vi "ActiView903-RealTime_CAS.vi"() -> ()   [LabVIEW 2022 SP3]
doc: "ActiView is based on a state machine (case structure inside while-loop) with six (orange) states:\n\nState 0: Wait for START, and read/write CFG files\nState 1: Start acquisition, determine speedmode and AD-box version, set panel controls accordingly, stop acquisition\nState 2: Reset panel indicators\nState 3: Initialize saving to BDF file\nState 4: Start acquisition, iterate while-loop to write data to screen and BDF flle (if selected) until STOP is pressed, or error occurs, stop acquisition\nState 5: Reset panel indicators, close BDF file\n\nThe while-loop in (orange) state 4 has five (green) cases.\n\nCase 0: Wait for new data\nCase 1: Read new data from ringbuffer, downsample data, write data to charts and in file array\nCase 2: Transfer block of 1 second of data from file array to BDF file\nCase 3: Close BDF file, and open new BDF file\nCase 4: Calculate average result, and write to ERP graphs \n\nAlso see the Light version of ActiView avalable from the www.biosemi.com"
uses:
  ActiView9-Subvi.llb/Data.glb
  ActiView9-Subvi.llb/CapsThread.glb
  ActiView9-Subvi.llb/PanelThread.glb
  <vilib>/Instr/_visa.llb/VISA Configure Serial Port (Instr).vi
  <vilib>/Utility/cursorutil.llb/Set Cursor (Icon Pict).vi
  <vilib>/Utility/config.llb/Read Key (String).vi
  <vilib>/Utility/config.llb/Write Key (String).vi
  ActiView9-Subvi.llb/StopJazzIni.glb
  ActiView9-Subvi.llb/TCPidentification.glb
  ActiView9-Subvi.llb/JazzLoBatWarning.glb
  ActiView9-Subvi.llb/LoBatWarning.glb
  ActiView9-Subvi.llb/StopThreads.glb
  <vilib>/httpClient/POSTBuffer.vi
  Instance          61 25Saved   ActiView606-Lores .vi
  <vilib>/Utility/config.llb/NI_LVConfig.lvlib
  <vilib>/httpClient/LabVIEWHTTPClient.lvlib
  <vilib>/Analysis/NI_AALBase.lvlib
panel:
  out "RemaingStim":i16
  in  "Task OFF/ON":bool
  in  "Condition":i8(ring) items=["Synch", "Asynch"]
  in  "Bloc":i8(ring) items=["1", "2", "3", "4"]
  in  "R-peak Threshold adjust":dbl=1.0 min=0.0 step=0.1 format="%#.6g"
  out "Trigger Bar":enum32{"Blank"}(tab)
  out "Dummy String":string
  out "Trigger Chart":i32[][](graph)
  out "Trigger Code":picture
  out "Battery":u8(slide) scale=0.0..100.0
  in  "Box":i32(ring) items=["AD-Box 1", "AD-Box 2", "AD-Box 3", "AD-Box 4"]
  out "Right Sidebar":enum32{"Blank"}(tab)
  out "Free HDD [sec]":i64=-1 caption="Free on Disc sec"
  out "Nr of Files":i32
  out "Total Saved [sec]":i32
  out "Current File [MB]":dbl format="%.1f"
  out "with Jazz or ABR":bool caption="with Jazz"
  out "Box4":bool caption="Box1"
  out "Box3":bool caption="Box1"
  out "Box2":bool caption="Box1"
  out "Box1":bool
  in  "FileAppend":bool=TRUE
  in  "RecTimeLimit":i32=9999999 caption="Time Limit [sec]" min=1 max=9999999 step=1
  out "Nr Chan Saved":string="0 + 0"
  out "with AIB":bool
  out "with Sens":bool
  out "with  8 EX":bool
  out "Bandwidth [Hz]":dbl
  in  "Decimation":i8(ring) items=["1", "1/2", "1/4", "1/8", "1/16", "1/32", "1/64"]
  out "Sample Rate [Hz]":dbl
  in  "FileLimit":i64=999999 caption="File Limit [MB]" min=1 max=999999 step=1
  out "Save Subset":string
  in  "Start Saving":bool
  in  "Pause Saving":bool
  out "Left Sidebar":T1(tab)
  in  "MonFree":i32[](listbox)=[0, 1, 2, 3, 4, 5, 6, 7, 8, 9, 10, 11, 12, 13, 14, 15, 16, 17, 18, 19, 20, 21, 22, 23, 24, 25, 26, 27, 28, 29, 30, 31, 32, 33, 34, 35, 36, 37, 38, 39, 40, 41, 42, 43, 44, 45, 46, 47, 48, 49, 50, 51, 52, 53, 54, 55, 56, 57, 58, 59, 60, 61, 62, 63, 64, 65, 66, 67, 68, 69, 70, 71, 72, 73, 74, 75, 76, 77, 78, 79, 80, 81, 82, 83, 84, 85, 86, 87, 88, 89, 90, 91, 92, 93, 94, 95, 96, 97, 98, 99, 100, 101, 102, 103, 104, 105, 106, 107, 108, 109, 110, 111, 112, 113, 114, 115, 116, 117, 118, 119, 120, 121, 122, 123, 124, 125, 126, 127, 128, 129, 130, 131, 132, 133, 134, 135, 136, 137, 138, 139, 140, 141, 142, 143, 144, 145, 146, 147, 148, 149, 150, 151, 152, 153, 154, 155, 156, 157, 158, 159, 160, 161, 162, 163, 164, 165, 166, 167, 168, 169, 170, 171, 172, 173, 174, 175, 176, 177, 178, 179, 180, 181, 182, 183, 184, 185, 186, 187, 188, 189, 190, 191, 192, 193, 194, 195, 196, 197, 198, 199, 200, 201, 202, 203, 204, 205, 206, 207, 208, 209, 210, 211, 212, 213, 214, 215, 216, 217, 218, 219, 220, 221, 222, 223, 224, 225, 226, 227, 228, 229, 230, 231, 232, 233, 234, 235, 236, 237, 238, 239, 240, 241, 242, 243, 244, 245, 246, 247, 248, 249, 250, 251, 252, 253, 254, 255]
  in  "Reference":i8(ring) items=["None (raw)", "Avg of 264", "Avg 1-256", "Avg 1-160", "Avg 1-128", "Avg 1-64", "Avg 1-32", "Avg of Displ", "Free Choice", "Ref (ABR)", "Mastoids (ABR)"]
  in  "Mon Filter Reset":bool
  in  "MonLP":bool=TRUE caption="Lowpass"
  in  "MonHP":bool=TRUE caption="Highpass"
  in  "RefFree":i32[](listbox)
  in  "Channels":i8(ring) items=["All 264 Chan ", "A-H (256)", "A-E (160)", "ABCD (128)", "A+B (64)", "A (32)", "B (32)", "C (32)", "D (32)", "E (32)", "F (32)", "G (32)", "H(32)", "EXG (8)", "Free Choice"]
  in  "MonHPfreq":dbl=0.16 caption="Cutoff Freq" min=0.01 max=9.99 step=0.1 format="%.2f"
  in  "MonScale":i8(ring)=4 caption="Y-scale V/div" items=["5 uV", "10 uV", "20 uV", "50 uV", "100 uV", "200 uV", "500 uV", "1 mV", "2 mV", "5 mV", "10 mV", "20 mV", "50 mV", "100 mV", "200 mV", "500 mV"]
  in  "MonLPfreq":dbl=100.0 caption="Cutoff Freq" min=1.0 max=8191.0 step=10.0
  out "NoRef Blinker":bool
  in  "AddTP":bool caption="Add  8 EXG"
  in  "BipFree":i32[](listbox)=[0, 2, 4, 6] caption="Bipolar\nLeads"
  in  "BipLP":bool=TRUE caption="Lowpass"
  in  "BipHP":bool=TRUE caption="Highpass"
  in  "BipHPfreq":dbl=0.16 caption="Cutoff Freq" min=0.01 max=99.9 step=1.0 format="%.2f"
  in  "BipScale":i8(ring)=7 caption="Y-scale V/div" items=["5 uV", "10 uV", "20 uV", "50 uV", "100 uV", "200 uV", "500 uV", "1 mV", "2 mV", "5 mV", "10 mV", "20 mV", "50 mV", "100 mV", "200 mV", "500 mV"]
  in  "BipLPfreq":dbl=100.0 caption="Cutoff Freq" min=1.0 max=8191.0 step=10.0
  in  "Bip Filter Reset":bool
  out "TP Offset Graph 2":dbl[](graph) caption="EX5 - EX8"
  out "TP Offset Graph 1":dbl[](graph) caption="EX1 - EX4"
  in  "Offset":i8(ring) caption="Channels" items=["All 256 Chan ", "A + B", "C + D", "E + F", "G + H"]
  out "Full Range":bool=TRUE
  in  "OffsetScale":i8(ring)=3 caption="Range" items=["20 mV", "50 mV", "100 mV", "262  mV", "1049 mV"]
  in  "HeadcapMaps":bool
  in  "UploadMaps":bool
  in  "ABR Filter Reset":bool
  in  "AbrLP":bool=TRUE caption="Lowpass"
  in  "AbrHP":bool=TRUE caption="Highpass"
  in  "AbrHPfreq":dbl=0.16 caption="Cutoff Freq" min=0.1 max=100.0 step=1.0 format="%.1f"
  in  "AbrScale":i8(ring)=4 caption="Y-scale V/div" items=["5 uV", "10 uV", "20 uV", "50 uV", "100 uV", "200 uV", "500 uV", "1 mV", "2 mV", "5 mV", "10 mV", "20 mV", "50 mV", "100 mV", "200 mV", "500 mV"]
  in  "AbrLPfreq":dbl=100.0 caption="Cutoff Freq" min=1.0 max=8191.0 step=10.0
  in  "AbrOn":bool caption="Enable ABR"
  in  "AbrChannels":i8(ring) caption="Channels" items=["Raw unreferenced", "LF referenced", "HF referenced"]
  out "ABR Offset Graph":dbl[](graph) caption="Offset"
  in  "AbrOffsetScale":i8(ring)=3 caption="Displayed \nRange" items=["20 mV", "50 mV", "100 mV", "262  mV"]
  out "ABR Full Range":bool=TRUE
  out "Rejected Sweeps":i32
  out "Valid Sweeps":i32
  in  "AvgLP":bool caption="Lowpass"
  in  "AvgLPfreq":dbl=100.0 caption="Cuttoff Freq" min=1.0 max=8191.0 step=10.0
  in  "AvgTrigLog":i8(ring) items=["AND trigs ", "OR trigs"]
  in  "AvgTrigSel":i32[](listbox)=[0]
  in  "AvgHP":bool=TRUE caption="Highpass"
  in  "AvgHPfreq":dbl=1.0 caption="Cutoff Freq" min=0.1 max=100.0 step=10.0 format="%.1f"
  out "RejDif":bool caption="Reject"
  out "RejAbs":bool caption="Reject"
  in  "AvgRelReject":dbl=50.0 caption="Difference with\navg more than:" min=0.0 step=1.0 format="%.1f"
  in  "AvgAbsReject":dbl=200.0 caption="All  sweeps\nlarger than:" min=0.0 step=10.0
  in  "AvgSweep":i32=500 caption="Sweep [msec]" min=1 max=9999 step=100
  in  "AvgAutoscale":bool=TRUE caption="Autoscale"
  in  "AvgScale":dbl=5.0 caption="Y-scale in uV" min=0.0 format="%.1f"
  in  "Averaging":bool
  in  "AuxReset":bool=TRUE caption="DC Reset at \nScreen Start"
  out "Unit":string="?"
  out "GSR2":dbl format="%_3f"
  out "GSR1":dbl format="%_3f"
  out "GSR2 pos":bool
  out "GSR2 neg":bool
  out "GSR1 pos":bool
  in  "GsrScale":i8(ring)=4 caption="GSR Y-scale" items=["1", "2", "5", "10", "20", "50", "100", "200", "500", "1k", "2k", "5k", "10k", "20k", "50k", "100k", "200k", "500k", "1M"]
  out "GSR1 neg":bool
  in  "ErgoLP":bool caption="Lowpass"
  in  "ErgoScale":i8(ring)=6 caption="Ergo Y-scale" items=["5 uV", "10 uV", "20 uV", "50 uV", "100 uV", "200 uV", "500 uV", "1 mV", "2 mV", "5 mV", "10 mV", "20 mV", "50 mV", "100 mV", "200 mV", "500 mV", "1V", "2V", "4V"]
  in  "AuxFree":i32[](listbox)=[0, 1, 2, 3, 4, 5, 6] caption="Sensors"
  in  "TempScale":i8(ring)=3 caption="Temp Y-scale" items=["0.01 C", "0.02 C", "0.05  C", "0.1 C", "0.2 C", "0.5 C", "1 C", "2 C", "5  C", "10 C"]
  in  "PletScale":i8(ring)=7 caption="Plet Y-scale" items=["5 uV", "10 uV", "20 uV", "50 uV", "100 uV", "200 uV", "500 uV", "1 mV", "2 mV", "5 mV", "10 mV", "20 mV", "50 mV", "100 mV", "200 mV", "500 mV"]
  in  "RespScale":i8(ring)=4 caption="Resp Y-scale" items=["0.1 mV", "0.2 mV", "0.5  mV", "1 mV", "2 mV", "5 mV", "10 mV", "20 mV", "50 mV", "100 mV", "200 mV", "500 mV"]
  out "Degrees Celcius":dbl caption="C" format="%.2f"
  in  "Aux DC Reset":bool
  in  "JazzOn":bool caption="Enable Jazz"
  in  "JazzReset":bool=TRUE caption="DC Reset at\nScreen Start"
  in  "JazzFree":i32[](listbox)=[0, 1, 2, 3, 4, 5, 6, 7, 8] caption="Jazz\nChannels"
  out "Jazz Batt Perc":string
  out "Jazz Batt Cap":u8(slide) caption="Jazz Batt" scale=0.0..100.0
  out "Jazz New\nFirmware":bool
  in  "Jazz Filter Reset":bool
  in  "AnaFree":i32[](listbox)=[0, 1, 2, 3, 4, 5, 6, 7, 8, 9, 10, 11, 12, 13, 14, 15] caption="Channels"
  in  "AnaReset":bool=TRUE caption="DC Reset at \nScreen Start"
  out "Ana Offset Graph":dbl[](graph)
  in  "AnaOffset":i32(ring) caption="AIB Channel" items=["Ana1", "Ana2", "Ana3", "Ana4", "Ana5", "Ana6", "Ana7", "Ana8", "Ana9", "Ana10", "Ana11", "Ana12", "Ana13", "Ana14", "Ana15", "Ana16", "Ana17", "Ana18", "Ana19", "Ana20", "Ana21", "Ana22", "Ana23", "Ana24", "Ana25", "Ana26", "Ana27", "Ana28", "Ana29", "Ana30", "Ana31", "Ana32"]
  in  "AnaLP":bool=TRUE caption="Lowpass"
  in  "AnaHP":bool=TRUE caption="Highpass"
  in  "AnaHPfreq":dbl=0.16 caption="Cutoff Freq" min=0.01 max=1023.0 step=1.0 format="%.2f"
  in  "AnaScale":i8(ring)=7 caption="Y-scale V/div" items=["5 uV", "10 uV", "20 uV", "50 uV", "100 uV", "200 uV", "500 uV", "1 mV", "2 mV", "5 mV", "10 mV", "20 mV", "50 mV", "100 mV", "200 mV", "500 mV", "1 V", "2 V", "4 V"]
  in  "AnaLPfreq":dbl=100.0 caption="Cutoff Freq" min=1.0 max=8191.0 step=10.0
  in  "Ana Filter Reset":bool
  in  "Buffer":i8(ring)=2 caption="Ringbuffer Size" items=["16 Mbyte", "32 Mbyte", "64 Mbyte", "128 Mbyte"]
  out "Pause Off/On":string="-1 / -1"
  out "Write CFG":bool
  in  "Save Configuration File":bool
  out "CFG Filepath":string
  in  "Load Configuration File":bool
  out "Errors:":i16
  in  "TrigCode":i8(ring) caption="Trigger Format" items=["Analog", "Decimal", "Hexa", "Binary", "Custom"]
  in  "ScreenLength":i32(ring)=3 caption="Screen Length" items=["1 sec", "2 sec", "4 sec", "8 sec", "16 sec", "32 sec", "64 sec"]
  out "Write BDF":bool
  out "BDF Filepath":string
  in  "Start":bool
  out "Low Batt":bool
  out "CM in Range":bool
  out "Ring Buffer":cluster{dbl, dbl}(knob)={0.0033134730043177896, 0.0033134730043177896} scale=0.0..64.0
  in  "Stop":bool
  in  "Charts/Graphs":T2(tab)
  out "MonLabels":picture
  out "Mon Chart":dbl[][](graph)
  out "BipLabels":picture
  out "Bip Chart":dbl[][](graph)
  out "DCLabels1 2":picture
  out "DCLabels1":picture
  out "Offset Graph First Half":dbl[](graph)
  out "Offset Graph  Second Half":dbl[](graph)
  out "ABR Labels":picture
  out "ABR Chart":dbl[][](graph)
  out "Avg2":dbl[][](graph) caption="Avg 2"
  out "Avg1":dbl[][](graph) caption="Avg 1"
  in  "RefFreeAvg2":i32[](listbox)=[3] caption="Versus"
  in  "MonFreeAvg2":i32(listbox)=2
  in  "RefFreeAvg1":i32[](listbox)=[1] caption="Versus"
  in  "MonFreeAvg1":i32(listbox)
  out "Sweeping":bool
  out "AuxLabels":picture
  out "Aux Chart":dbl[][](graph)
  out "JazzLabels":picture
  out "Jazz Chart":dbl[][](graph)
  out "AnaLabels":picture
  out "Ana Chart":dbl[][](graph)
  in  "TCPaddJazz":bool caption="Add 9 Jazz"
  in  "TCPaddTrig":bool caption="Add Trigger/Status Chan"
  out "Bytes in TCP Array":i32
  out "Bytes received by Client":i32
  out "TCP samples/channel":i32
  out "Channels sent by TCP":i32
  in  "TCPaddAnas":bool caption="Add 32 AIB Chan"
  in  "TCPaddSens":bool caption="Add 7 Sensors"
  in  "TCPaddTP":bool caption="Add  8 EX  electrodes"
  in  "TCPsubset":i8(ring)=7 caption="TCP subset:" items=["A1 - H32 (256)", "A1 - E32 (160)", "A1 - D32 (128)", "A1 - B32 (64)", "A1 - A32 (32)", "A1 - A16 (16)", "A1 -A8 (8)", "None (0) "]
  out "TCP Listening":bool
  out "TCP Connected":bool
  out "Remote Adress":string
  out "Receive Remote Port":u16
  out "Bytes sent by Server":i32
  in  "LocalPort":u16=778 caption="Sent Local Port"
  in  "Reset":bool
  out "Max RT Loop Block (ms)":i64
  in  "Set Stride in kByte\n(default 128 kByte)":i64=8
  out "USB-receiver firmware":string="?"
  out "USB-receiver model":string="?"
  out "Speed Mode":string="?"
  out "Server ID":string="?"
  out "Application:Kind":T3(ring)
  out "AD-box":string="?"
  in  "Edit":bool
  in  "Marker F8":bool
  in  "Marker F7":bool
  in  "Marker F6":bool
  in  "Marker F5":bool
  in  "Marker F4":bool
  in  "Marker F3":bool
  in  "Marker F2":bool
  in  "Marker F1":bool
  in  "Master Filter Reset":bool
  # "Trig 1-8"
  # "Trig 9-16"
  # "AD-Box"
  # "None = CMS"
  # "GSR\nIn Range"
  # "1"
  # "2"
  # "Range in mV"
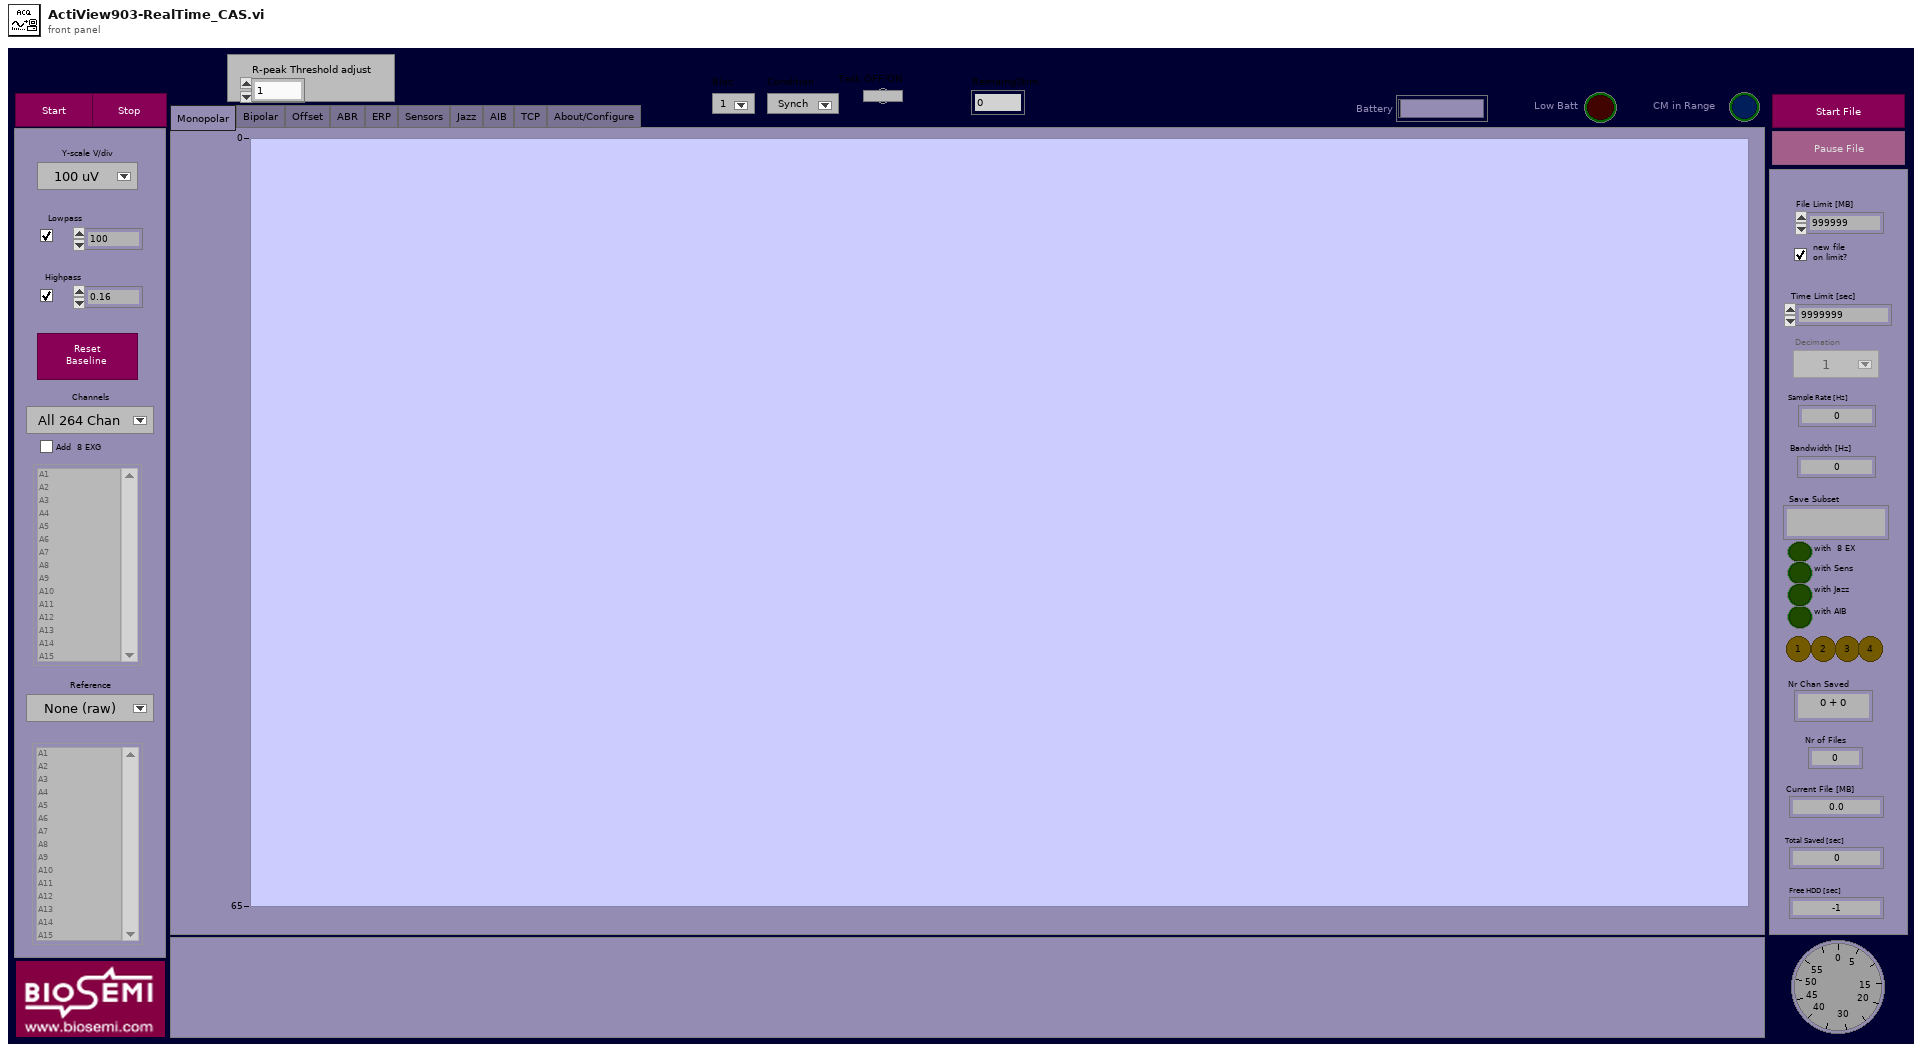
[diagram p1: front panel]
types:
  T1 = enum32{"Monopolar", "Bipolar", "Offset", "ABR", "Average", "Sensors", "Jazz", "Analog", "Initialization"}
  T2 = enum32{"Monopolar", "Bipolar", "Offset", "ABR", "ERP", "Sensors", "Jazz", "AIB", "TCP", "About/Configure"}
  T3 = enum32{"invalid app kind", "Development System", "Run Time System", "Student Edition", "Embedded LabVIEW", "Evaluation", "Custom"}
  T4 = cluster{"Font Name:":string, "Size":i16, "Strikeout?":bool, "Italic?":bool, "Underline?":bool, "Outline?":bool, "Shadow?":bool, "Bold?":bool}
  T5 = enum32{"Page Enabled", "Page Disabled", "Page Disabled & Grayed"}
  T6 = enum8{"Enabled", "Disabled", "Disabled and Grayed Out"}
  T7 = cluster{"AbrLP":bool, "AbrLPfreq":dbl, "AbrHP":bool, "AbrHPfreq":dbl}
  T8 = cluster{"Mark2":bool, "GSR16Hz":bool, "JazzRec":bool, "ABR Enabled":bool, "Speed Mode":i8, "ADC Rate":i32, "ADC Channels":i32, "Screen Ratio":i32, "Decimate Ratio":i32, "Mon Channels":i32, "Bip Channels":i32, "Aux Channels":i32, "Jazz Channels":i32, "Ana Channels":i32, "Save Subset":i8, "Add Touchproofs":bool, "Add Sensors":bool, "Add Jazz":bool, "Add Anas":bool, "Save Box":u32, "PauseOff":i32, "PauseOn":i32, "Save Path":path}
  T9 = cluster{"Warning":i8, "Motherboard":i8, "ElecGain":i8, "RespSwitch":i8, "LineWidth":u8, "Cursor":u16, "PopupKiller":i8, "BreathBelt":i8, "ABRlocation":i8, "SEMGswap":i8, "TrigLength":i32, "TrigLevel":i32, "TrigWindow":i8, "TrigPol":i8}
  T10 = cluster{"All Labels":string[], "Spec Labels":string[]}
  T11 = cluster{"connection ID":refnum<k5>, "remote address":string, "remote port":u16}
  T12 = enum16{"open", "replace", "create", "open or create", "replace or create", "replace or create with confirmation"}
  T13 = cluster{"Start Averaging":bool, "Busy Averaging":bool, "Sweep Lenght in Samples":i32, "Valid Sweeps":i32, "Rejected Sweeps":i32, "First Graph Update":bool}
  T14 = cluster{"Jazz No Data":bool, "Jazz Packet Loss":bool, "Jazz Batt":u8, "Jazz New Firmware":bool}
  T15 = cluster{"GSR1pos":bool, "GSR1neg":bool, "GSR2pos":bool, "GSR2neg":bool}
  T16 = cluster{"Sweeping":bool, "RejAbs":bool, "RejDif":bool}
  T17 = cluster{"ABR Enabled":bool, "Speed Mode":i8, "Save Subset":i8, "Initially Channel Selection":i32[], "Add Touchproofs":bool, "Mon Channels":i32, "Bip Channels":i32, "Add Sensors":bool, "Initially Channel Selection":i32[], "Add Jazz":bool, "Initially Channel Selection":i32[], "Add Anas":bool, "Initially Channel Selection":i32[], "Save Box":u32}
  T18 = typedef "LabVIEWHTTPClient.lvlib/ClientHandle.ctl" = refnum<k1>
  T19 = typedef "NI_LVConfig.lvlib/Config Data RefNum.ctl" = refnum<k1>
  T20 = cluster{"Save Subset":i8, "Add Touchproofs":bool, "Add Sensors":bool, "Add Jazz":bool, "Add Anas":bool, "Save Box":u32}
  T21 = cluster{"Local Patient Identification":string, "Local  Recording Identification":string}
  T22 = cluster{"Mark2":bool, "GSR16Hz":bool, bool, "Speed Mode":i8, "ABR Enabled":bool}
  T23 = cluster{"length":i32, "f":i32, "f":i32, "f":i32, "f":i32, "f":i32}
  T24 = cluster{bool, bool, bool, bool, bool, bool, bool, bool}
  T25 = cluster{"Clear Block":dbl, "Screen Ratio":dbl, "Y1":dbl, "Y2":dbl, "Y3":dbl, "Color":u32, "YT1":dbl, "YT2":dbl, "YT3":dbl}
  T26 = cluster{"Sync Errors":i16, "Recent Sync Error":bool}
  T27 = cluster{"LoBatChange":bool, "JazzLoBatChange":bool}
  T28 = typedef "LVRectTypeDef.ctl" = cluster{"Left":i16, "Top":i16, "Right":i16, "Bottom":i16}
  T29 = cluster{"GsrScale":i8, "ErgoScale":i8, "ErgoLP":bool, "RespScale":i8, "PletScale":i8, "TempScale":i8}
  T30 = cluster{"Mon Channels":i32, "Bip Channels":i32, "Aux Channels":i32, "Jazz Channels":i32}
  T31 = cluster{"End of Screen":bool, "Prop Screen Minimum":i64, "Screen Position":i32}
  T32 = cluster{"Ring Buffer Overflow":bool, "First Call":bool}
  T33 = cluster{"Xo":dbl, "Xmax":dbl, "Xmin":dbl, "Marker values":dbl[]}
  T34 = cluster{"AvgLP":bool, "AvgLPfreq ":dbl, "AvgHP":bool, "AvgHPfreq":dbl}
  T35 = cluster{"MonLP":bool, "MonLPfreq":dbl, "MonHP":bool, "MonHPfreq":dbl}
  T36 = cluster{"BipLP":bool, "BipLPfreq":dbl, "BipHP":bool, "BipHPfreq":dbl}
  T37 = cluster{"AnaLP":bool, "AnaLPfreq":dbl, "AnaHP":bool, "AnaHPfreq":dbl}
  T38 = cluster{"Marker F1":bool, "Marker F2":bool, "Marker F3":bool, "Marker F4":bool, "Marker F5":bool, "Marker F6":bool, "Marker F7":bool, "Marker F8":bool}
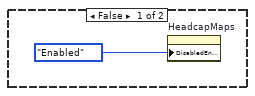
[diagram p2: hidden frame]
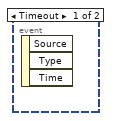
[diagram p3: hidden frame]
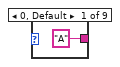
[diagram p6: hidden frame]
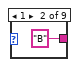
[diagram p7: hidden frame]
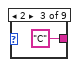
[diagram p8: hidden frame]
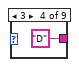
[diagram p9: hidden frame]
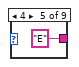
[diagram p10: hidden frame]
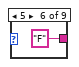
[diagram p11: hidden frame]
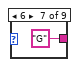
[diagram p12: hidden frame]
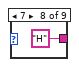
[diagram p13: hidden frame]
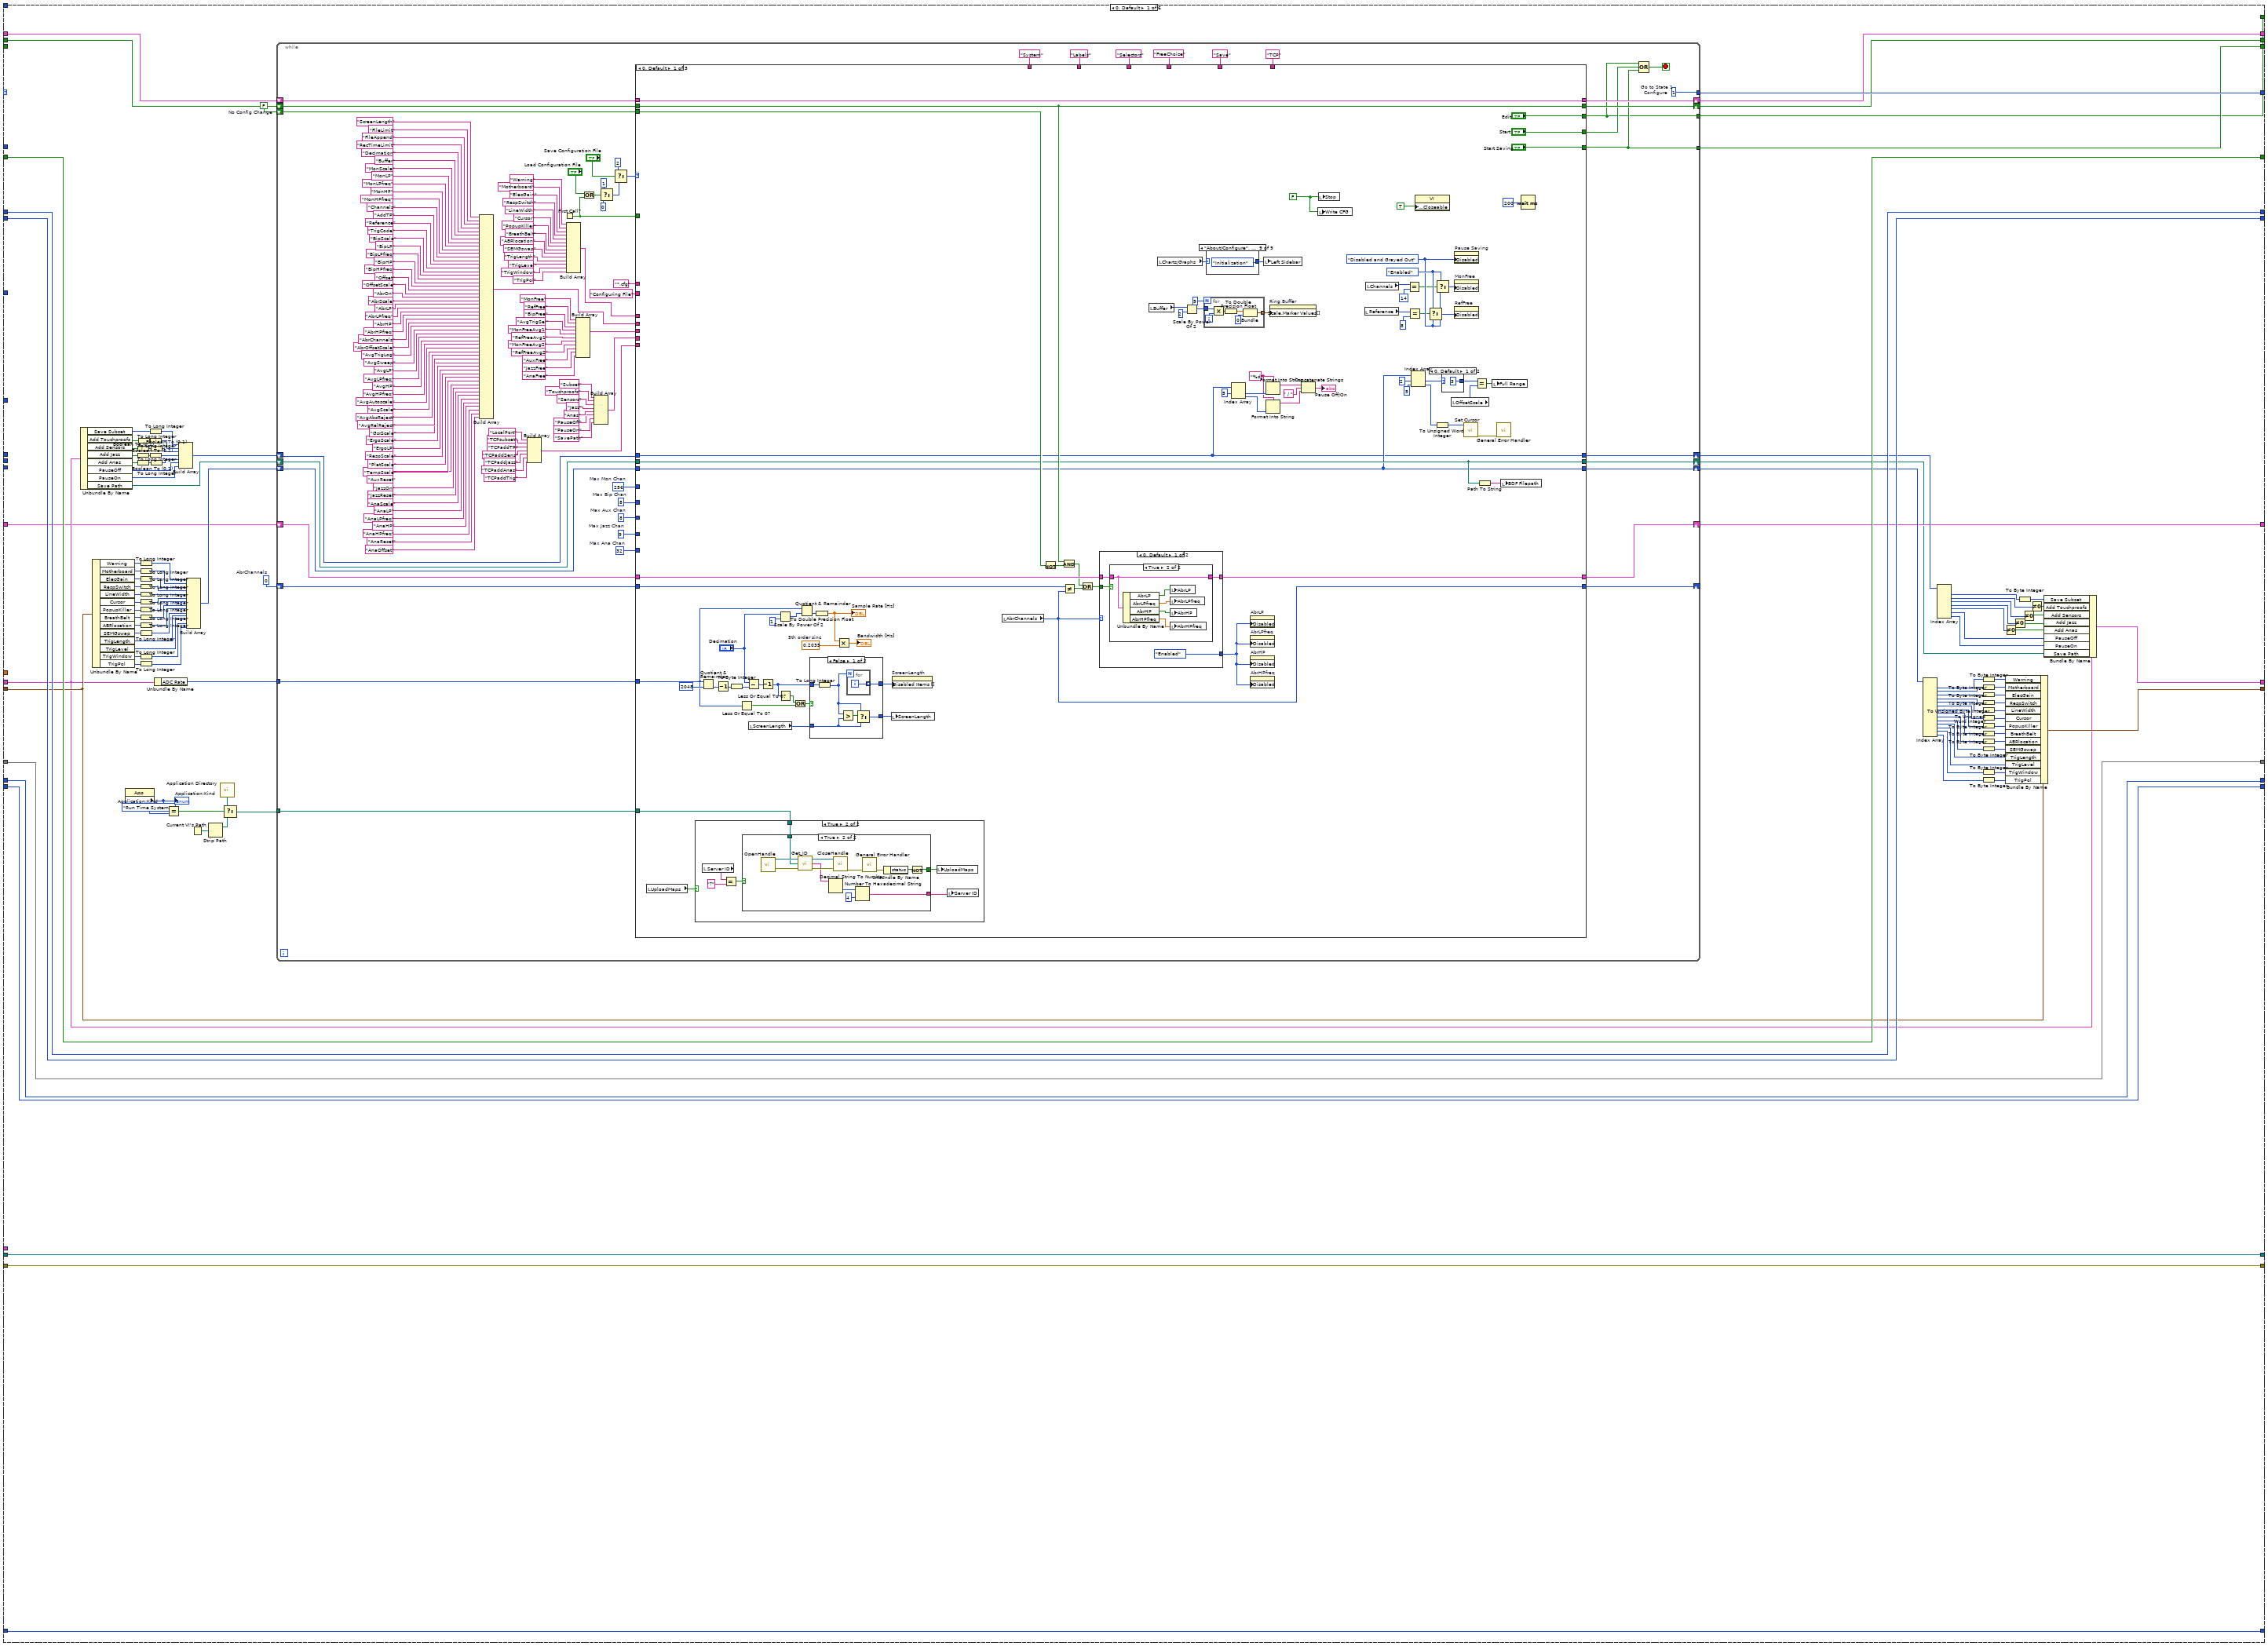
[diagram p14: hidden frame]
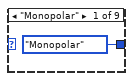
[diagram p15: hidden frame]
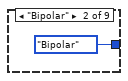
[diagram p16: hidden frame]
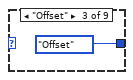
[diagram p17: hidden frame]
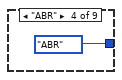
[diagram p18: hidden frame]
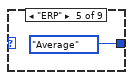
[diagram p19: hidden frame]
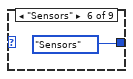
[diagram p20: hidden frame]
diagram:
  w20 = 44100.0
  w35 = i8 0  # TrigWindow
  w34 = i8 0  # TrigPol
  (unwired) i8 0  # TrigWindow
  w36 = 0  # TrigLevel
  w37 = 0  # TrigLength
  w38 = T4 {"Font Name:"="App Font", "Size"=12, "Strikeout?"=FALSE, "Italic?"=FALSE, "Underline?"=FALSE, "Outline?"=FALSE, "Shadow?"=FALSE, "Bold?"=FALSE}  # Channel and Trigger Font
  w39 = i8 0  # SEMGswap
  w42 = TRUE  # AbrHP
  w43 = 0.2  # AbrHPfreq
  w45 = 100.0  # AbrLPfreq
  w44 = TRUE  # AbrLP
  w46 = i8 0  # ABRlocation
  w51 = FALSE  # ABR Enabled
  w52 = i8 0  # BreathBelt
  w50 = FALSE  # JazzRec
  w54 = FALSE  # Add Anas
  w56 = 0  # Ana Channels
  w49 = FALSE  # GSR16Hz
  w61 = u32 0  # Save Box
  w48 = FALSE  # Mark2
  w64 = path ""  # Save Path
  w62 = 0  # PauseOff
  w63 = 0  # PauseOn
  w66 = 0  # ADC Rate
  w67 = 0  # ADC Channels
  w69 = 0  # Screen Ratio
  w55 = FALSE  # Add Jazz
  w57 = 0  # Jazz Channels
  w58 = FALSE  # Add Sensors
  w59 = FALSE  # Add Touchproofs
  w60 = i8 0  # Save Subset
  w65 = i8 -1  # Speed Mode
  w68 = 0  # Aux Channels
  w71 = 0  # Bip Channels
  w70 = 0  # Decimate Ratio
  w72 = 0  # Mon Channels
  w73 = i8 0  # PopupKiller
  w78 = FALSE  # Initially Not Start with Save
  w81 = refnum<file> refnum  # Dummy Refnum
  w74 = u16 0  # Cursor
  w75 = u8 0  # LineWidth
  w76 = i8 -1  # RespSwitch
  w83 = i8 -1  # Warning
  w85 = i8 -1  # Motherboard
  w84 = i8 -1  # ElecGain
  w86 = FALSE  # Initially Not Config Changed
  w87 = string[] []  # Spec Labels
  w88 = string[] []  # All Labels
  w77 = i32[] []  # Initially Channel Selection
  w79 = 0  # Initially  nothing saved
  w90 = FALSE  # Initially Not Busy Saving
  w89 = 0  # Initial State
  # "Load the CardiosynchExperimental generated by Matlab for experimental sucessions"
  # "Load the log file for r-peak threshold"
  # "Extract the R-peak threshold"
  # "loop start button"
  # "Initiate sound wave"
  # "Initiate trigger port"
  # "Initiate cooldown conter"
  # "Initialize Position_ECG_vector"
  # "Initialize ECG_vector"
  n1 = call "File Dialog2"("prompt"="Select CardioSynchExperimental of the participant" ("default name"), "pattern (all files)"="CardioSynchExperimental*.txt") -> ("selected path"=w6:path, "cancelled"=w7:bool)  [unwired: 10 in, 2 out]
  n2 = stacked-sequence {
    tunnel: [w129] -> w47
    frame #0 {
      w93 = FALSE ("PanelThread")
      w94 = T6."Enabled" ("Disabled")
      w103 = 0.5 ("X Scale.Range:Minimum")
      w104 = 128.5 ("X Scale.Range:Maximum")
      w99 = 8191.0 ("Data Range:Maximum")
      w129 = errorcluster {"status"=FALSE, "code"=0, "source"=""}  # Initially  No Error
      w130 = i32[] [] ("Disabled Items []")
      w127 = FALSE ("Visible")
      n3 = for {
        N: 264 -> [_]
        tunnel: [w147] -> w131 mode=indexing
        i -> [w152]
        n4 = Quotient & Remainder(x=w152, y=32) -> (x-y*floor(x/y)=w149:i32, floor(x/y)=w150:i32)
        n5 = case shown="8" w150 {
          tunnel: ["A" "B" "C" "D" "E" "F" "G" "H" "EX"] -> w148
          frame 0, Default {
          }
          frame 1 {
          }
          frame 2 {
          }
          frame 3 {
          }
          frame 4 {
          }
          frame 5 {
          }
          frame 6 {
          }
          frame 7 {
          }
          frame 8 {
          }
        }
        n6 = Increment(x=w149) -> (x+1=w146:i32)
        n7 = Format Into String(initial string=w148, w146) -> (resulting string=w147:string)  [unwired: 2 in, 1 out]
      }
      n8 = for {
        N: 128 -> [_]
        tunnel: [w136] -> w105 mode=indexing
        i -> [w138]
        n9 = Increment(x=w138) -> (x+1=w137:i32)
        n10 = To Double Precision Float(number=w137) -> (double precision float=w136:dbl)
      }
      n11 = Increment(x=3) -> (x+1=w95:i32)
      n12 = Increment(x=264) -> (x+1=w111:i32)
      n13 = Increment(x=8) -> (x+1=w110:i32)
      n14 = Increment(x=7) -> (x+1=w109:i32)
      n15 = Increment(x=9) -> (x+1=w108:i32)
      n16 = Increment(x=32) -> (x+1=w107:i32)
      n17 = property on="Charts/Graphs" class="TabCtl (strict)"() -> ("Pages"=w128:refnum<vi>[])  [unwired: 2 in, 2 out]
      n18 = property on="NoRef Blinker" class="Bool"("Visible"=w127) -> ()  [unwired: 2 in, 2 out]
      n19 = property on="Box" class="Ring (strict)"("Visible"=w127) -> ()  [unwired: 2 in, 2 out]
      n20 = for {
        N: w95 -> [_]
        tunnel: [w134] -> w97 mode=indexing
        i -> [w134]
      }
      n21 = for {
        N: w109 -> [_]
        tunnel: [w141] -> w119 mode=indexing
        i -> [w141]
      }
      n22 = for {
        N: w108 -> [_]
        tunnel: [w140] -> w116 mode=indexing
        i -> [w140]
      }
      n23 = for {
        N: w110 -> [_]
        tunnel: [w142] -> w122 mode=indexing
        i -> [w142]
      }
      n24 = for {
        N: w107 -> [_]
        tunnel: [w139] -> w113 mode=indexing
        i -> [w139]
      }
      n25 = for {
        N: w111 -> [_]
        tunnel: [w143] -> w125 mode=indexing
        i -> [w143]
      }
      n26 = for {
        N: 129 -> [_]
        tunnel: [0.0] -> w100 mode=indexing
      }
      n27 = for {
        tunnel: w128 -> [w145] mode=indexing
        n28 = property class="Page"(reference=w145, "Page Enabled State"=T5."Page Enabled") -> ()  [unwired: 1 in, 2 out]
      }
      n29 = global write "PanelThread.glb" "PanelThread"(w93) -> ()
      n30 = global write "CapsThread.glb" "CapsThread"(w93) -> ()
      n31 = local write "UploadMaps"(w93) -> ()
      n32 = property on="Ring Buffer" class="Knob (strict)"("Scale.Uniform Marker Spacing?"=FALSE) -> ()  [unwired: 2 in, 2 out]
      n33 = property on="AddTP" class="Bool (strict)"("Disabled"=w94) -> ()  [unwired: 2 in, 2 out]
      n34 = property on="TP Offset Graph 1" class="WFGraph (strict)"("Disabled"=w94) -> ()  [unwired: 2 in, 2 out]
      n35 = property on="TP Offset Graph 2" class="WFGraph (strict)"("Disabled"=w94) -> ()  [unwired: 2 in, 2 out]
      n36 = property on="AbrOn" class="Bool (strict)"("DisabledEnum"=w94) -> ()  [unwired: 2 in, 2 out]
      n37 = property on="AvgLP" class="Bool (strict)"("DisabledEnum"=w94) -> ()  [unwired: 2 in, 2 out]
      n38 = property on="AvgLPfreq" class="DigNum (strict)"("DisabledEnum"=w94) -> ()  [unwired: 2 in, 2 out]
      n39 = property on="AvgHP" class="Bool (strict)"("DisabledEnum"=w94) -> ()  [unwired: 2 in, 2 out]
      n40 = property on="AvgHPfreq" class="DigNum (strict)"("DisabledEnum"=w94) -> ()  [unwired: 2 in, 2 out]
      n41 = property on="MonFreeAvg1" class="LstBox (strict)"("DisabledEnum"=w94) -> ()  [unwired: 2 in, 2 out]
      n42 = property on="RefFreeAvg1" class="LstBox (strict)"("DisabledEnum"=w94) -> ()  [unwired: 2 in, 2 out]
      n43 = property on="MonFreeAvg2" class="LstBox (strict)"("DisabledEnum"=w94) -> ()  [unwired: 2 in, 2 out]
      n44 = property on="RefFreeAvg2" class="LstBox (strict)"("DisabledEnum"=w94) -> ()  [unwired: 2 in, 2 out]
      n45 = property on="GSR1 pos" class="Bool (strict)"("Disabled"=w94) -> ()  [unwired: 2 in, 2 out]
      n46 = property on="GSR1 neg" class="Bool (strict)"("Disabled"=w94) -> ()  [unwired: 2 in, 2 out]
      n47 = property on="GSR1" class="DigNum (strict)"("Disabled"=w94) -> ()  [unwired: 2 in, 2 out]
      n48 = property on="GSR2 neg" class="Bool (strict)"("Disabled"=w94) -> ()  [unwired: 2 in, 2 out]
      n49 = property on="GSR2 pos" class="Bool (strict)"("Disabled"=w94) -> ()  [unwired: 2 in, 2 out]
      n50 = property on="GsrScale" class="Ring (strict)"("Disabled"=w94) -> ()  [unwired: 2 in, 2 out]
      n51 = property on="Unit" class="Str"("Disabled"=w94) -> ()  [unwired: 2 in, 2 out]
      n52 = property on="ErgoScale" class="Ring (strict)"("Disabled"=w94) -> ()  [unwired: 2 in, 2 out]
      n53 = property on="ErgoLP" class="Bool (strict)"("Disabled"=w94) -> ()  [unwired: 2 in, 2 out]
      n54 = property on="RespScale" class="Ring (strict)"("Disabled"=w94) -> ()  [unwired: 2 in, 2 out]
      n55 = property on="PletScale" class="Ring (strict)"("Disabled"=w94) -> ()  [unwired: 2 in, 2 out]
      n56 = property on="TempScale" class="Ring (strict)"("Disabled"=w94) -> ()  [unwired: 2 in, 2 out]
      n57 = property on="Degrees Celcius" class="DigNum (strict)"("Disabled"=w94) -> ()  [unwired: 2 in, 2 out]
      n58 = property on="JazzOn" class="Bool (strict)"("Disabled"=w94) -> ()  [unwired: 2 in, 2 out]
      n59 = property on="HeadcapMaps" class="Bool (strict)"("DisabledEnum"=w94) -> ()  [unwired: 2 in, 2 out]
      n60 = property on="Decimation" class="Ring (strict)"("DisabledEnum"=w94) -> ()  [unwired: 2 in, 2 out]
      n61 = To Double Precision Float(number=w97) -> (double precision float=w96:dbl[])
      n62 = To Double Precision Float(number=w125) -> (double precision float=w124:dbl[])
      n63 = To Double Precision Float(number=w122) -> (double precision float=w121:dbl[])
      n64 = To Double Precision Float(number=w119) -> (double precision float=w118:dbl[])
      n65 = To Double Precision Float(number=w116) -> (double precision float=w115:dbl[])
      n66 = To Double Precision Float(number=w113) -> (double precision float=w112:dbl[])
      n67 = property on="Battery" class="Slide (strict)"("Visible"=TRUE) -> ()  [unwired: 2 in, 2 out]
      n68 = local write "Server ID"("?" ("Server ID")) -> ()
      n69 = property on="ScreenLength" class="Ring (strict)"("Disabled Items []"=w130) -> ()  [unwired: 2 in, 2 out]
      n70 = property on="Channels" class="Ring (strict)"("Disabled Items []"=w130) -> ()  [unwired: 2 in, 2 out]
      n71 = property on="Reference" class="Ring (strict)"("Disabled Items []"=w130) -> ()  [unwired: 2 in, 2 out]
      n72 = property on="Offset" class="Ring (strict)"("Disabled Items []"=w130) -> ()  [unwired: 2 in, 2 out]
      n73 = property on="TCPsubset" class="Ring (strict)"("Disabled Items []"=w130) -> ()  [unwired: 2 in, 2 out]
      n74 = global write "Data.glb" "Data"(w100) -> ()
      n75 = property on="Offset Graph First Half" class="WFGraph (strict)"("XScale.Maximum"=w104, "XScale.Minimum"=w103, "XScale.MarkerVals[]"=w105) -> ()  [unwired: 2 in, 2 out]
      n76 = property on="Offset Graph  Second Half" class="WFGraph (strict)"("XScale.Maximum"=w104, "XScale.Minimum"=w103, "XScale.MarkerVals[]"=w105) -> ()  [unwired: 2 in, 2 out]
      n77 = property on="ABR Chart" class="WFChart (strict)"("YScale.MarkerVals[]"=w96) -> ()  [unwired: 2 in, 2 out]
      n78 = property on="Mon Chart" class="WFChart (strict)"("YScale.MarkerVals[]"=w124, "YScale.Maximum"=65.0 ("Y Scale.Range:Maximum")) -> ()  [unwired: 2 in, 2 out]
      n79 = property on="Bip Chart" class="WFChart (strict)"("YScale.MarkerVals[]"=w121) -> ()  [unwired: 2 in, 2 out]
      n80 = property on="Aux Chart" class="WFChart (strict)"("YScale.MarkerVals[]"=w118) -> ()  [unwired: 2 in, 2 out]
      n81 = property on="Jazz Chart" class="WFChart (strict)"("YScale.MarkerVals[]"=w115) -> ()  [unwired: 2 in, 2 out]
      n82 = property on="Ana Chart" class="WFChart (strict)"("YScale.MarkerVals[]"=w112) -> ()  [unwired: 2 in, 2 out]
      n83 = property on="BipLPfreq" class="DigNum (strict)"("Data Range:Maximum"=w99) -> ()  [unwired: 2 in, 2 out]
      n84 = property on="AbrLPfreq" class="DigNum (strict)"("Data Range:Maximum"=w99) -> ()  [unwired: 2 in, 2 out]
      n85 = property on="AvgLPfreq" class="DigNum (strict)"("Data Range:Maximum"=w99) -> ()  [unwired: 2 in, 2 out]
      n86 = property on="AnaLPfreq" class="DigNum (strict)"("Data Range:Maximum"=w99) -> ()  [unwired: 2 in, 2 out]
      n87 = property on="MonLPfreq" class="DigNum (strict)"("Data Range:Maximum"=w99) -> ()  [unwired: 2 in, 2 out]
      n88 = property on="MonFree" class="LstBox (strict)"("Item Names"=w131) -> ()  [unwired: 2 in, 2 out]
      n89 = property on="RefFree" class="LstBox (strict)"("Item Names"=w131) -> ()  [unwired: 2 in, 2 out]
      n90 = property on="MonFreeAvg1" class="LstBox (strict)"("Item Names"=w131) -> ()  [unwired: 2 in, 2 out]
      n91 = property on="RefFreeAvg1" class="LstBox (strict)"("Item Names"=w131) -> ()  [unwired: 2 in, 2 out]
      n92 = property on="MonFreeAvg2" class="LstBox (strict)"("Item Names"=w131) -> ()  [unwired: 2 in, 2 out]
      n93 = property on="RefFreeAvg2" class="LstBox (strict)"("Item Names"=w131) -> ()  [unwired: 2 in, 2 out]
    }
  }
  n94 = call "File Dialog"("prompt"="Select logfile of the participant" ("default name"), "pattern (all files)"="logfile*.txt") -> ("selected path"=w14:path, "cancelled"=w11:bool)  [unwired: 10 in, 2 out]
  n95 = Stop(stop? (T)=w7) -> ()
  n96 = call "Read_text_file_mic.vi"("file path (dialog if empty)"=w6) -> ("Table"=w5:string[][])  [unwired: 10 in]
  n97 = Decimal String To Number(string=w5) -> (number=w4:i32[][])  [unwired: 2 in, 1 out]
  n98 = Stop(stop? (T)=w11) -> ()
  n99 = call "Read_text_file_mic.vi"("file path (dialog if empty)"=w14) -> ("Table"=w10:string[][])  [unwired: 10 in]
  n100 = Reciprocal(x=w20) -> (1/x=w23:dbl)
  n101 = Multiply(x=0.1, y=w20) -> (x*y=w26:dbl)
  n102 = Divide(x=1000.0, y=w20) -> (x/y=w24:dbl)
  n103 = call <vilib>:"Sine Wave.vi"("samples"=w26, "amplitude"=1.0, "frequency"=w24) -> ("sine wave"=w3:dbl[])  [unwired: 2 in, 2 out]
  n104 = Index Array(array=w10, index (row)=1, index (col)=1 ("disabled index (col)")) -> (element=w18:string)
  n105 = call "Normalized_sound.vi"("signal IN"=w3) -> ("signal OUT"=w2:dbl[])  [unwired: 10 in]
  n106 = Bundle By Name("Y"=w2, "dt"=w23) -> (w19:waveform(dbl))  [unwired: 1 in]
  n107 = Decimal String To Number(string=w18) -> (number=w15:i32)  [unwired: 2 in, 1 out]
  n108 = Bundle("AbrLP"=w44, "AbrLPfreq"=w45, "AbrHP"=w42, "AbrHPfreq"=w43) -> (w41:T7)  [unwired: 1 in]
  n109 = Bundle("Mark2"=w48, "GSR16Hz"=w49, "JazzRec"=w50, "ABR Enabled"=w51, "Speed Mode"=w65, "ADC Rate"=w66, "ADC Channels"=w67, "Screen Ratio"=w69, "Decimate Ratio"=w70, "Mon Channels"=w72, "Bip Channels"=w71, "Aux Channels"=w68, "Jazz Channels"=w57, "Ana Channels"=w56, "Save Subset"=w60, "Add Touchproofs"=w59, "Add Sensors"=w58, "Add Jazz"=w55, "Add Anas"=w54, "Save Box"=w61, "PauseOff"=w62, "PauseOn"=w63, "Save Path"=w64) -> (w53:T8)  [unwired: 1 out]
  n110 = Bundle("Warning"=w83, "Motherboard"=w85, "ElecGain"=w84, "RespSwitch"=w76, "LineWidth"=w75, "Cursor"=w74, "PopupKiller"=w73, "BreathBelt"=w52, "ABRlocation"=w46, "SEMGswap"=w39, "TrigLength"=w37, "TrigLevel"=w36, "TrigWindow"=w35, "TrigPol"=w34) -> (w82:T9)  [unwired: 1 out]
  n111 = Initialize Array(0.0 ("element"), 102 ("dimension size")) -> (w31:dbl[])
  n112 = Bundle("All Labels"=w88, "Spec Labels"=w87) -> (w40:T10)  [unwired: 1 out]
  n113 = To Quad Integer(1:w79) -> (0:w80:i64)
  n114 = call-poly "VISA Configure Serial Port"("VISA resource name"=refnum<visa-resource-name> "COM3", "baud rate (9600)"=u32 9600) -> ("VISA resource name out"=w27:refnum<visa-resource-name>)  [unwired: 12 in, 1 out]
  n115 = while {
    shift-left: w79 -> [w216]
    shift-right: [w215] -> _
    shift-left: w80 -> [w219]
    shift-right: [w220] -> _
    shift-left: w40 -> [w225]
    shift-right: [w226] -> _
    shift-left: w53 -> [w198]
    shift-right: [w227] -> _
    shift-left: w47 -> [w218]
    shift-right: [w228] -> _
    shift-left: w81 -> [w230]
    shift-right: [w229] -> _
    shift-left: w90 -> [w232]
    shift-right: [w231] -> _
    shift-left: w89 -> [w177]
    shift-right: [w233] -> _
    shift-right: [w212] -> _
    shift-left: w77 -> [w195]
    shift-right: [w207] -> _
    shift-left: w77 -> [w192]
    shift-right: [w205] -> _
    shift-left: w86 -> [w206]
    shift-right: [w204] -> _
    shift-left: w77 -> [w190]
    shift-right: [w200] -> _
    shift-left: w82 -> [w174]
    shift-right: [w188] -> _
    shift-left: w78 -> [w187]
    shift-right: [w186] -> _
    shift-left: w77 -> [w179]
    shift-right: [w171] -> _
    shift-left: w41 -> [w172]
    tunnel: w38 -> [w170]
    tunnel: w31 -> [w168]
    tunnel: 0 -> [w167]
    tunnel: i64 0 -> [w166]
    tunnel: w27 -> [w165]
    tunnel: w19 -> [w164]
    tunnel: w15 -> [w163]
    tunnel: w4 -> [w162]
    stop <- w169 stop-if-true
    w199 = 3  # Bytes per Word
    # "Sart with Save"
    # "Config Change"
    # "Current File in Byte"
    # "Header Lenght in Byte"
    # "Label Cluster"
    # "State machine with 6 states"
    # "Program runs continuously until\nEdit button is pressed in state 0"
    n116 = Unbundle By Name(w198) -> ("ABR Enabled"=w175:bool, "Speed Mode"=w176:i8, "Mon Channels"=w185:i32, "Bip Channels"=w184:i32, "Save Subset"=w183:i8, "Add Touchproofs"=w182:bool, "Add Sensors"=w181:bool, "Add Jazz"=w180:bool, "Add Anas"=w191:bool, "ADC Rate"=w194:i32, "Decimate Ratio"=w193:i32, "Save Box"=w189:u32)
    n117 = Unbundle By Name(w174) -> ("ABRlocation"=w173:i8)
    n118 = Wait (ms)(milliseconds to wait=u32 0) -> ()  [unwired: 1 out]
    n119 = Bundle("ABR Enabled"=w175, "Speed Mode"=w176, "Save Subset"=w183, "Initially Channel Selection"=w195, "Add Touchproofs"=w182, "Mon Channels"=w185, "Bip Channels"=w184, "Add Sensors"=w181, "Initially Channel Selection"=w192, "Add Jazz"=w180, "Initially Channel Selection"=w179, "Add Anas"=w191, "Initially Channel Selection"=w190, "Save Box"=w189) -> (w196:T17)  [unwired: 1 out]
    n120 = call "SaveSelect-ABR-EEG.vi"("Save Selection Cluster"=w196, "ABRlocation"=w173) -> ("ChanSelection"=w178:i32[], "Number of Save Channels"=w197:i32)
    n121 = Add(x="Buffer", y=i8 24) -> (x+y=w223:i8)
    n122 = Quotient & Remainder(x=w194, y=w193) -> (floor(x/y)=w211:i32)  [unwired: 1 out]
    n123 = Scale By Power Of 2(n="ScreenLength", x=1 ("X Scale.Range:Maximum")) -> (x*2^n=w201:i32)
    n124 = Scale By Power Of 2(n=w223, x=i64 1) -> (x*2^n=w221:i64)
    n125 = Scale By Power Of 2(n="Buffer", x=2) -> (x*2^n=w208:i32)
    n126 = To Double Precision Float(number=w211) -> (double precision float=w217:dbl)
    n127 = Compound Arithmetic op=MULTIPLY(w199, w197, w211) -> (w213:i32)
    n128 = case shown="4" w177 {
      tunnel: [w351 w1964 w2599 w2739 w3000 w5178] -> w233
      tunnel: w221 -> [_ w1776 _ _ w2860 _]
      tunnel: w217 -> [_ _ w2585 _ w2943 _]
      tunnel: w232 -> [w350 w1946 w2571 _ w2878 w5172]
      tunnel: [w350 w1946 w2571 w2730 w2877 w5151] -> w231
      tunnel: w230 -> [w349 w1961 w2613 _ w2996 w5176]
      tunnel: [w349 w1961 w2613 w2691 w2994 w5175] -> w229
      tunnel: [w348 w1779 w2573 w2736 w2926 w5162] -> w228
      tunnel: w213 -> [_ _ _ _ w2891 w5165]
      tunnel: [w343 w1711 w2576 w2725 w2982 w5146] -> w227
      tunnel: w198 -> [w297 w1812 w2576 w2724 w2931 w5146]
      tunnel: [w344 w1924 w2608 w2749 w2979 w5180] -> w226
      tunnel: w225 -> [w345 w1928 w2608 w2749 w2979 w5180]
      tunnel: [w347 w1962 w2612 w2693 w2998 w5150] -> w220
      tunnel: w219 -> [w347 w1962 w2612 _ w2993 w5177]
      tunnel: [w282 w1959 w2611 w2750 w2995 w5179] -> w169
      tunnel: w218 -> [w348 w1780 w2603 _ w2997 w5174]
      tunnel: w208 -> [_ _ w2605 _ _ _]
      tunnel: w216 -> [w346 w1963 w2610 _ w2992 w5173]
      tunnel: [w346 w1963 w2610 w2717 w2991 w5166] -> w215
      tunnel: w211 -> [_ _ _ _ w2945 _]
      tunnel: w195 -> [w309 w1960 w2609 w2714 w2984 w5171]
      tunnel: [w309 w1960 w2609 w2714 w2983 w5171] -> w212
      tunnel: w192 -> [w308 w1951 w2604 w2707 w2976 w5168]
      tunnel: [w308 w1951 w2604 w2707 w2975 w5168] -> w207
      tunnel: w206 -> [w329 w1950 w2588 w2734 w2974 w5170]
      tunnel: [w328 w1949 w2588 w2734 w2974 w5170] -> w205
      tunnel: w190 -> [w307 w1921 w2587 w2706 w2973 w5169]
      tunnel: [w307 w1921 w2587 w2706 w2972 w5169] -> w204
      tunnel: w201 -> [_ _ w2579 _ w2949 _]
      tunnel: w174 -> [w318 w1698 w2583 w2664 w2946 w5167]
      tunnel: [w317 w1698 w2583 w2664 w2948 w5167] -> w200
      tunnel: [w295 w1820 w2574 w2692 w2888 w5161] -> w188
      tunnel: w187 -> [_ w1820 w2574 w2692 w2887 w5161]
      tunnel: w179 -> [w288 w1796 w2572 w2684 w2885 w5152]
      tunnel: [w288 w1796 w2572 w2684 w2883 w5152] -> w186
      tunnel: w178 -> [_ _ _ _ w2857 _]
      tunnel: w172 -> [w271 w1682 w2566 w2662 w2842 w5119]
      tunnel: [w272 w1682 w2566 w2662 w2843 w5119] -> w171
      tunnel: w170 -> [_ _ _ _ w2841 _]
      tunnel: w168 -> [_ _ _ _ w2829 _]
      tunnel: w167 -> [_ _ _ _ w2828 _]
      tunnel: w166 -> [_ _ _ _ w2827 _]
      tunnel: w165 -> [_ _ _ _ w2826 _]
      tunnel: w164 -> [_ _ _ _ w2825 _]
      tunnel: w163 -> [_ _ _ _ w2824 _]
      tunnel: w162 -> [_ _ _ _ w2821 _]
      frame 0, Default {
        w269 = FALSE  # No Config Change
        w270 = i8 0  # AbrChannels
        n129 = Unbundle By Name(w297) -> ("Save Subset"=w333:i8, "Add Touchproofs"=w338:bool, "Add Sensors"=w337:bool, "Add Jazz"=w323:bool, "Add Anas"=w292:bool, "PauseOff"=w235:i32, "PauseOn"=w234:i32, "Save Path"=w236:path)
        n130 = Unbundle By Name(w318) -> ("Warning"=w322:i8, "Motherboard"=w321:i8, "ElecGain"=w320:i8, "RespSwitch"=w313:i8, "LineWidth"=w304:u8, "Cursor"=w306:u16, "PopupKiller"=w286:i8, "BreathBelt"=w283:i8, "ABRlocation"=w274:i8, "SEMGswap"=w268:i8, "TrigLength"=w240:i32, "TrigLevel"=w239:i32, "TrigWindow"=w246:i8, "TrigPol"=w245:i8)
        n131 = property class="App"() -> ("Application:Kind"=w277:T3)  [unwired: 2 in, 2 out]
        "Application:Kind" <- w277
        n132 = Boolean To (0,1)(Boolean=w323) -> (0, 1=w325:i16)
        n133 = Boolean To (0,1)(Boolean=w337) -> (0, 1=w336:i16)
        n134 = Boolean To (0,1)(Boolean=w292) -> (0, 1=w293:i16)
        n135 = Boolean To (0,1)(Boolean=w338) -> (0, 1=w335:i16)
        n136 = To Long Integer(number=w322) -> (32bit integer=w266:i32)
        n137 = To Long Integer(number=w321) -> (32bit integer=w265:i32)
        n138 = To Long Integer(number=w320) -> (32bit integer=w262:i32)
        n139 = To Long Integer(number=w313) -> (32bit integer=w261:i32)
        n140 = To Long Integer(number=w304) -> (32bit integer=w303:i32)
        n141 = To Long Integer(number=w306) -> (32bit integer=w305:i32)
        n142 = To Long Integer(number=w286) -> (32bit integer=w260:i32)
        n143 = To Long Integer(number=w283) -> (32bit integer=w259:i32)
        n144 = To Long Integer(number=w274) -> (32bit integer=w258:i32)
        n145 = To Long Integer(number=w268) -> (32bit integer=w257:i32)
        n146 = To Long Integer(number=w246) -> (32bit integer=w264:i32)
        n147 = To Long Integer(number=w245) -> (32bit integer=w263:i32)
        n148 = To Long Integer(number=w333) -> (32bit integer=w294:i32)
        n149 = To Long Integer(number=w335) -> (32bit integer=w332:i32)
        n150 = To Long Integer(number=w325) -> (32bit integer=w324:i32)
        n151 = To Long Integer(number=w336) -> (32bit integer=w331:i32)
        n152 = To Long Integer(number=w293) -> (32bit integer=w291:i32)
        n153 = Unbundle By Name(w297) -> ("ADC Rate"=w296:i32)
        n154 = Equal?(x=w277, y=T3."Run Time System") -> (x = y?=w281:bool)
        n155 = Build Array(w294, w332, w331, w324, w291, w235, w234) -> (w334:i32[])
        n156 = Build Array(w266, w265, w262, w261, w303, w305, w260, w259, w258, w257, w240, w239, w264, w263) -> (w319:i32[])
        n157 = Current VI's Path() -> (path=w280:path)
        n158 = Strip Path(path=w280) -> (stripped path=w278:path)  [unwired: 1 out]
        n159 = call <vilib>:"Application Directory.vi"() -> ("Application Directory"=w279:path)
        n160 = Select(t=w279, s=w281, f=w278) -> (s? t:f=w275:path)
        n161 = while {
          tunnel: [w359] -> w282
          tunnel: [w496] -> w351
          shift-right: [w493] -> w344
          shift-left: w345 -> [w494]
          shift-right: [w469] -> w311
          shift-left: w334 -> [w447]
          shift-right: [w491] -> w328
          shift-left: w329 -> [w492]
          shift-right: [w442] -> w310
          shift-left: w319 -> [w445]
          shift-right: [w466] -> w237
          shift-left: w236 -> [w446]
          tunnel: w296 -> [w362]
          tunnel: [w361] -> w295
          tunnel: w275 -> [w370]
          shift-right: [w367] -> w272
          shift-left: w271 -> [w368]
          shift-right: [w365] -> _
          shift-left: w270 -> [w366]
          shift-left: w269 -> [w364]
          stop <- w495 stop-if-true
          w427 = 9  # Max Jazz Chan
          w475 = 32  # Max Ana Chan
          w476 = 8  # Max Aux Chan
          w477 = 8  # Max Bip Chan
          w478 = 256  # Max Mon Chan
          w496 = 1  # Go to State 1   Configure
          n162 = Build Array("ScreenLength" ("key"), "FileLimit" ("key"), "FileAppend" ("key"), "RecTimeLimit" ("key"), "Decimation" ("key"), "Buffer" ("key"), "MonScale" ("key"), "MonLP" ("key"), "MonLPfreq" ("key"), "MonHP" ("key"), "MonHPfreq" ("key"), "Channels" ("key"), "AddTP" ("key"), "Reference" ("key"), "TrigCode" ("key"), "BipScale" ("key"), "BipLP" ("key"), "BipLPfreq" ("key"), "BipHP" ("key"), "BipHPfreq" ("key"), "Offset" ("key"), "OffsetScale" ("key"), "AbrOn" ("key"), "AbrScale" ("key"), "AbrLP" ("key"), "AbrLPfreq" ("key"), "AbrHP" ("key"), "AbrHPfreq" ("key"), "AbrChannels" ("key"), "AbrOffsetScale" ("key"), "AvgTrigLog" ("key"), "AvgSweep" ("key"), "AvgLP" ("key"), "AvgLPfreq" ("key"), "AvgHP" ("key"), "AvgHPfreq" ("key"), "AvgAutoscale" ("key"), "AvgScale" ("key"), "AvgAbsReject" ("key"), "AvgRelReject" ("key"), "GsrScale" ("key"), "ErgoScale" ("key"), "ErgoLP" ("key"), "RespScale" ("key"), "PletScale" ("key"), "TempScale" ("key"), "AuxReset" ("key"), "JazzOn" ("key"), "JazzReset" ("key"), "AnaScale" ("key"), "AnaLP" ("key"), "AnaLPfreq" ("key"), "AnaHP" ("key"), "AnaHPfreq" ("key"), "AnaReset" ("key"), "AnaOffset" ("key")) -> (w403:string[])
          n163 = Build Array("LocalPort" ("key"), "TCPsubset" ("key"), "TCPaddTP" ("key"), "TCPaddSens" ("key"), "TCPaddJazz" ("key"), "TCPaddAnas" ("key"), "TCPaddTrig" ("key")) -> (w437:string[])
          n164 = First Call?() -> (First Call?: T/F=w467:bool)
          n165 = Build Array("Warning" ("key"), "Motherboard" ("key"), "ElecGain" ("key"), "RespSwitch" ("key"), "LineWidth" ("key"), "Cursor" ("key"), "PopupKiller" ("key"), "BreathBelt" ("key"), "ABRlocation" ("key"), "SEMGswap" ("key"), "TrigLength" ("key"), "TrigLevel" ("key"), "TrigWindow" ("key"), "TrigPol" ("key")) -> (w428:string[])
          n166 = Build Array("MonFree" ("key"), "RefFree" ("key"), "BipFree" ("key"), "AvgTrigSel" ("key"), "MonFreeAvg1" ("key"), "RefFreeAvg1" ("key"), "MonFreeAvg2" ("key"), "RefFreeAvg2" ("key"), "AuxFree" ("key"), "JazzFree" ("key"), "AnaFree" ("key")) -> (w464:string[])
          n167 = Or(x="Load Configuration File", y=w467) -> (x .or. y?=w487:bool)
          n168 = Build Array("Subset" ("key"), "Touchproofs" ("key"), "Sensors" ("key"), "Jazz" ("key"), "Anas" ("key"), "PauseOff" ("key"), "PauseOn" ("key"), "SavePath" ("key")) -> (w473:string[])
          n169 = Select(t=i8 1, s=w487, f=i8 0 ("t")) -> (s? t:f=w489:i8)
          n170 = Select(t=i8 2, s="Save Configuration File", f=w489) -> (s? t:f=w490:i8)
          n171 = case shown="0, Default" w490 {
            tunnel: w494 -> [w574 w690 w1330]
            tunnel: w467 -> [_ w650 _]
            tunnel: [w574 w689 w1330] -> w493
            tunnel: [w515 w688 w1327] -> w469
            tunnel: w447 -> [w515 w687 w1327]
            tunnel: w492 -> [w565 w685 w1340]
            tunnel: [w565 w686 w1340] -> w491
            tunnel: w403 -> [_ w684 w1336]
            tunnel: "Labels" -> [_ w683 w1334]
            tunnel: "Selectors" ("section") -> [_ w682 w1335]
            tunnel: "FreeChoice" ("section") -> [_ w681 w1329]
            tunnel: "Save" ("section") -> [_ w680 w1328]
            tunnel: w478 -> [_ w679 w1333]
            tunnel: w477 -> [_ w678 w1332]
            tunnel: w476 -> [_ w677 w1331]
            tunnel: w475 -> [_ w676 w1315]
            tunnel: w473 -> [_ w675 w1326]
            tunnel: "System" -> [_ w674 w1324]
            tunnel: [w524 w673 w1325] -> w442
            tunnel: w445 -> [w524 w671 w1325]
            tunnel: w428 -> [_ w672 w1323]
            tunnel: w446 -> [w534 w670 w1322]
            tunnel: w437 -> [_ w669 w1321]
            tunnel: [w534 w668 w1322] -> w466
            tunnel: w464 -> [_ w667 w1320]
            tunnel: "TCP" ("section") -> [_ w651 w1319]
            tunnel: "*.cfg" ("pattern") -> [_ w649 w1317]
            tunnel: "Configuring File" ("pattern label") -> [_ w648 w1316]
            tunnel: w427 -> [_ w647 w1314]
            tunnel: w370 -> [w561 w646 w1313]
            tunnel: w368 -> [w572 w644 w1312]
            tunnel: [w571 w645 w1311] -> w367
            tunnel: w366 -> [w570 w643 w1310]
            tunnel: [w569 w643 w1310] -> w365
            tunnel: w364 -> [w566 _ _]
            tunnel: w362 -> [w536 _ _]
            tunnel: ["Start Saving" w642 w1309] -> w361
            tunnel: ["Start" w642 w1309] -> w360
            tunnel: ["Edit" w642 w1309] -> w359
            frame 0, Default {
              w513 = T6."Enabled" ("Disabled")
              w512 = T6."Disabled and Grayed Out" ("Disabled")
              w511 = FALSE ("Stop")
              w518 = "%d" ("Format String")
              w554 = 0.2035  # 5th order sinc
              n172 = local read "UploadMaps"() -> (w562:bool)
              n173 = case shown="True" w562 {
                tunnel: w561 -> [_ w602]
                frame False {
                }
                frame True {
                  n174 = local read "Server ID"() -> (w604:string)
                  n175 = Equal?(x=w604, y="?") -> (x = y?=w605:bool)
                  n176 = case shown="True" w605 {
                    tunnel: [w608 w615] -> w603
                    tunnel: w602 -> [_ w613]
                    tunnel: [TRUE w609] -> w601
                    frame False {
                      n177 = local read "Server ID"() -> (w608:string)
                    }
                    frame True {
                      n178 = call <vilib>:"OpenHandle.vi"() -> ("client handle out"=w619:T18, "error out"=w614:errorcluster)  [unwired: 14 in]
                      n179 = call "Get_ID.vi"("error in (no error)"=w614, "Filepath"=w613, "client handle in"=w619) -> ("error out"=w620:errorcluster, "ID (decimal)"=w616:string, "client handle out"=w621:T18)
                      n180 = Decimal String To Number(string=w616) -> (number=w618:i32)  [unwired: 2 in, 1 out]
                      n181 = call <vilib>:"CloseHandle.vi"("client handle"=w621, "error in (no error)"=w620) -> ("error out"=w612:errorcluster)  [unwired: 13 in]
                      n182 = Number To Hexadecimal String(1:i16 4 ("width (-)"), 2:w618) -> (0:w615:string)
                      n183 = call <vilib>:"General Error Handler.vi"("error in (no error)"=w612) -> ("error out"=w611:errorcluster)  [unwired: 4 in, 10 out]
                      n184 = Unbundle By Name(w611) -> ("status"=w610:bool)
                      n185 = Not(x=w610) -> (.not. x?=w609:bool)
                    }
                  }
                  n186 = local write "UploadMaps"(w601) -> ()
                  n187 = local write "Server ID"(w603) -> ()
                }
              }
              n188 = Quotient & Remainder(x=w536, y=2048) -> (floor(x/y)=w544:i32)  [unwired: 1 out]
              n189 = Decrement(x=w544) -> (x-1=w545:i32)
              n190 = To Byte Integer(number=w545) -> (8bit integer=w546:i8)
              n191 = Less Or Equal To 0?(x=w536) -> (x <= 0?=w552:bool)
              n192 = Subtract(x="Decimation", y=w546) -> (x-y=w550:i8)
              n193 = local read "ScreenLength"() -> (w548:i32)
              n194 = Decrement(x=w550) -> (x-1=w555:i8)
              n195 = Scale By Power Of 2(n="Decimation", x=1) -> (x*2^n=w541:i32)
              n196 = Less Or Equal To 0?(x=w555) -> (x <= 0?=w551:bool)
              n197 = Or(x=w551, y=w552) -> (x .or. y?=w553:bool)
              n198 = Quotient & Remainder(x=w536, y=w541) -> (floor(x/y)=w537:i32)  [unwired: 1 out]
              n199 = case shown="False" w553 {
                tunnel: [w588 i32[] [] ("Disabled Items []")] -> w547
                tunnel: [w589 w593] -> w549
                tunnel: w548 -> [w590 w593]
                tunnel: w555 -> [w587 _]
                frame False {
                  n200 = To Long Integer(number=w587) -> (32bit integer=w586:i32)
                  n201 = Greater?(x=w586, y=w590) -> (0:w591:bool)
                  n202 = for {
                    N: w586 -> [_]
                    tunnel: [w592] -> w588 mode=indexing
                    i -> [w592]
                  }
                  n203 = Select(t=w586, s=w591, f=w590) -> (s? t:f=w589:i32)
                }
                frame True {
                }
              }
              n204 = To Double Precision Float(number=w537) -> (double precision float=w539:dbl)
              "Sample Rate [Hz]" <- w539
              n205 = Multiply(x=w539, y=w554) -> (x*y=→"Bandwidth [Hz]":dbl)
              n206 = local write "ScreenLength"(w549) -> ()
              n207 = property on="ScreenLength" class="Ring (strict)"("Disabled Items []"=w547) -> ()  [unwired: 2 in, 2 out]
              n208 = local read "AbrChannels"() -> (w569:i8)
              n209 = Not(x=w566) -> (.not. x?=w563:bool)
              n210 = And(x=w565, y=w563) -> (x .and. y?=w564:bool)
              n211 = Not Equal?(x=w570, y=w569) -> (x != y?=w567:bool)
              n212 = Or(x=w564, y=w567) -> (x .or. y?=w568:bool)
              n213 = case shown="0, Default" w569 {
                tunnel: [T6."Enabled" ("Disabled") T6."Disabled and Grayed Out" ("Disabled")] -> w573
                tunnel: w572 -> [w624 w640]
                tunnel: [w623 w640] -> w571
                tunnel: w568 -> [w622 _]
                frame 0, Default {
                  n214 = case shown="True" w622 {
                    tunnel: w624 -> [w627 w636]
                    tunnel: [w626 w636] -> w623
                    frame False {
                      n215 = local read "AbrHPfreq"() -> (w628:dbl)
                      n216 = local read "AbrLPfreq"() -> (w630:dbl)
                      n217 = local read "AbrHP"() -> (w629:bool)
                      n218 = local read "AbrLP"() -> (w631:bool)
                      n219 = Bundle By Name(cluster=w627, "AbrLP"=w631, "AbrLPfreq"=w630, "AbrHP"=w629, "AbrHPfreq"=w628) -> (w626:T7)
                    }
                    frame True {
                      n220 = Unbundle By Name(w636) -> ("AbrLP"=w635:bool, "AbrLPfreq"=w634:dbl, "AbrHP"=w633:bool, "AbrHPfreq"=w632:dbl)
                      n221 = local write "AbrLP"(w635) -> ()
                      n222 = local write "AbrLPfreq"(w634) -> ()
                      n223 = local write "AbrHP"(w633) -> ()
                      n224 = local write "AbrHPfreq"(w632) -> ()
                    }
                  }
                }
                frame 2 {
                  w637 = TRUE ("AbrLP")
                  n225 = local write "AbrLP"(w637) -> ()
                  n226 = local write "AbrLPfreq"(3334.0 ("AbrLPfreq")) -> ()
                  n227 = local write "AbrHP"(w637) -> ()
                  n228 = local write "AbrHPfreq"(100.0 ("AbrHPfreq")) -> ()
                }
              }
              n229 = local read "Buffer"() -> (w560:i8)
              n230 = local read "Charts/Graphs"() -> (w502:T2)
              n231 = Scale By Power Of 2(n=w560, x=2) -> (x*2^n=w559:i32)
              n232 = for {
                N: 9 -> [_]
                tunnel: w559 -> [w599]
                tunnel: [w595] -> w557 mode=indexing
                i -> [w600]
                n233 = Multiply(x=w599, y=w600) -> (x*y=w598:i32)
                n234 = To Double Precision Float(number=w598) -> (double precision float=w597:dbl)
                n235 = Bundle(w597, u32 0) -> (w595:cluster{dbl, u32})  [unwired: 1 out]
              }
              n236 = case shown="\"About/Configure\", Default" w502 {
                tunnel: [T1."Monopolar" ("Left Sidebar") T1."Bipolar" ("Left Sidebar") T1."Offset" ("Left Sidebar") T1."ABR" ("Left Sidebar") T1."Average" ("Left Sidebar") T1."Sensors" ("Left Sidebar") T1."Jazz" ("Left Sidebar") T1."Analog" ("Left Sidebar") T1."Initialization" ("Left Sidebar")] -> w514
                frame "Monopolar" {
                }
                frame "Bipolar" {
                }
                frame "Offset" {
                }
                frame "ABR" {
                }
                frame "ERP" {
                }
                frame "Sensors" {
                }
                frame "Jazz" {
                }
                frame "AIB" {
                }
                frame "About/Configure", Default {
                }
              }
              n237 = Index Array(array=w515, index #1=5 ("index")) -> (element #1=w522:i32, element #2=w523:i32)  [unwired: 1 in]
              n238 = property on="AbrLP" class="Bool (strict)"("Disabled"=w573) -> ()  [unwired: 2 in, 2 out]
              n239 = property on="AbrLPfreq" class="DigNum (strict)"("Disabled"=w573) -> ()  [unwired: 2 in, 2 out]
              n240 = property on="AbrHP" class="Bool (strict)"("Disabled"=w573) -> ()  [unwired: 2 in, 2 out]
              n241 = property on="AbrHPfreq" class="DigNum (strict)"("Disabled"=w573) -> ()  [unwired: 2 in, 2 out]
              n242 = local write "Left Sidebar"(w514) -> ()
              n243 = Format Into String(format string=w518, w522) -> (resulting string=w520:string)  [unwired: 2 in, 1 out]
              n244 = Format Into String(format string=w518, w523) -> (resulting string=w516:string)  [unwired: 2 in, 1 out]
              n245 = property on="Ring Buffer" class="Knob (strict)"("Scale.Marker Values[]"=w557) -> ()  [unwired: 2 in, 2 out]
              n246 = Concatenate Strings(w520, " / " ("Substring"), w516) -> (→"Pause Off/On":string)
              n247 = local write "Write CFG"(w511) -> ()
              n248 = local write "Stop"(w511) -> ()
              n249 = local read "Reference"() -> (w508:i8)
              n250 = local read "Channels"() -> (w510:i8)
              n251 = Equal?(x=w510, y=i8 14 ("x")) -> (x = y?=w506:bool)
              n252 = Equal?(x=w508, y=i8 8) -> (x = y?=w507:bool)
              n253 = Index Array(array=w524, index #1=2 ("index"), index #2=5 ("index")) -> (element #1=w532:i32, element #2=w531:i32)
              n254 = property class="VI"("Front Panel Window:Closeable"=TRUE) -> ()  [unwired: 2 in, 2 out]
              n255 = Select(t=w513, s=w507, f=w512) -> (s? t:f=w503:T6)
              n256 = To Unsigned Word Integer(number=w531) -> (unsigned 16bit integer=w529:u16)
              n257 = Select(t=w513, s=w506, f=w512) -> (s? t:f=w504:T6)
              n258 = case shown="0, Default" w532 {
                tunnel: [i8 3 ("x") i8 4 ("x")] -> w533
                frame 0, Default {
                }
                frame 1 {
                }
              }
              n259 = local read "OffsetScale"() -> (w526:i8)
              n260 = property on="Pause Saving" class="Bool (strict)"("Disabled"=w512) -> ()  [unwired: 2 in, 2 out]
              n261 = property on="MonFree" class="LstBox (strict)"("Disabled"=w504) -> ()  [unwired: 2 in, 2 out]
              n262 = property on="RefFree" class="LstBox (strict)"("Disabled"=w503) -> ()  [unwired: 2 in, 2 out]
              n263 = call-poly <vilib>:"Set Cursor.vi"("icon"=w529) -> ("error out"=w528:errorcluster)  [unwired: 2 in, 8 out]
              n264 = Equal?(x=w533, y=w526) -> (x = y?=w525:bool)
              n265 = Path To String(path=w534) -> (string=w535:string)
              n266 = local write "Full Range"(w525) -> ()
              n267 = call <vilib>:"General Error Handler.vi"("error in (no error)"=w528) -> ()  [unwired: 2 in, 13 out]
              n268 = local write "BDF Filepath"(w535) -> ()
              n269 = Wait (ms)(milliseconds to wait=u32 200 ("millisecond timer value")) -> ()  [unwired: 1 out]
            }
            frame 1 {
              w642 = FALSE
              w660 = "Default.cfg"  # Default Configuration File
              # "Does File Exist?"
              n270 = property class="App"() -> (reference out=w666:refnum<vi>, "Application:Command Line Arguments"=w665:string[])  [unwired: 2 in, 1 out]
              n271 = Index Array(array=w665, index=1) -> (element=w661:string)
              n272 = Close Reference(reference=w666) -> (error out=w659:errorcluster)  [unwired: 1 in]
              n273 = Not Equal?(x=w661, y="") -> (x != y?=w662:bool)
              n274 = Select(t=w661, s=w662, f=w660) -> (s? t:f=w656:string)
              n275 = Build Path(base path=w646, name or relative path=w656) -> (appended path=w694:path)
              n276 = File/Directory Info(path=w694, error in=w659) -> (path out=w658:path, error out=w655:errorcluster)  [unwired: 5 out]
              n277 = Unbundle By Name(w655) -> ("code"=w693:i32)
              n278 = Not Equal?(x=w693, y=7 ("code")) -> (x != y?=w691:bool)
              n279 = And(x=w691, y=w650) -> (x .and. y?=w657:bool)
              n280 = case shown="False" w657 {
                tunnel: w646 -> [w701 _]
                tunnel: [w700 w705] -> w653
                tunnel: w658 -> [_ w705]
                tunnel: w656 -> [w698 _]
                tunnel: [w699 w704] -> w652
                tunnel: w655 -> [_ w703]
                tunnel: [w697 w703] -> w654
                tunnel: w649 -> [w696 _]
                tunnel: w648 -> [w695 _]
                frame False {
                  n281 = File Dialog(4:w695, 6:w696, 7:"Enter filename:" ("prompt"), 9:w698, 11:w701) -> (0:w697:errorcluster, 1:w699:bool, 3:w700:path)  [unwired: 1 in, 2 out]
                }
                frame True {
                  w704 = FALSE  # Cancelled
                }
              }
              n282 = case shown="False" w652 {
                tunnel: w690 -> [w749 w1308]
                tunnel: [w743 w1308] -> w689
                tunnel: w653 -> [w712 _]
                tunnel: [w744 w1307] -> w688
                tunnel: w687 -> [_ w1307]
                tunnel: [w745 w1306] -> w686
                tunnel: w685 -> [_ w1306]
                tunnel: w684 -> [w737 _]
                tunnel: w683 -> [w736 _]
                tunnel: w682 -> [w735 _]
                tunnel: w681 -> [w734 _]
                tunnel: w680 -> [w733 _]
                tunnel: w679 -> [w732 _]
                tunnel: w678 -> [w731 _]
                tunnel: w677 -> [w730 _]
                tunnel: w676 -> [w729 _]
                tunnel: w675 -> [w726 _]
                tunnel: w674 -> [w725 _]
                tunnel: [w724 w1305] -> w673
                tunnel: w672 -> [w723 _]
                tunnel: w671 -> [_ w1305]
                tunnel: w670 -> [_ w1304]
                tunnel: w669 -> [w721 _]
                tunnel: [w720 w1304] -> w668
                tunnel: w667 -> [w719 _]
                tunnel: w654 -> [w711 _]
                tunnel: w651 -> [w717 _]
                tunnel: w647 -> [w713 _]
                tunnel: [w707 w1303] -> w645
                tunnel: w644 -> [w706 w1303]
                frame False {
                  w745 = TRUE  # Config Changed
                  n283 = Path To String(path=w712) -> (string=→"CFG Filepath":string)
                  n284 = call <vilib>:"Open Config Data.vi"("error in (no error)"=w711, "configuration file path"=w712) -> ("error out"=w710:errorcluster, "refnum"=w709:T19)  [unwired: 7 in, 1 out]
                  n285 = stacked-sequence {
                    seq-local: [_ w841 _ _ _ _] -> [_ _ w1038 _ _ _]
                    seq-local: [_ w840 _ _ _ _] -> [_ _ w1037 _ _ _]
                    seq-local: [_ _ w1036 _ _ _] -> [_ _ _ w1190 _ _]
                    seq-local: [_ _ w1035 _ _ _] -> [_ _ _ w1189 _ _]
                    seq-local: [_ _ _ w1187 _ _] -> [_ _ _ _ w1252 _]
                    seq-local: [_ _ _ w1186 _ _] -> [_ _ _ _ w1251 _]
                    seq-local: [w758 _ _ _ _ _] -> [_ w843 _ _ _ _]
                    seq-local: [w759 _ _ _ _ _] -> [_ w844 _ _ _ _]
                    seq-local: [_ _ _ _ w1230 _] -> [_ _ _ _ _ w1274]
                    seq-local: [_ _ _ _ w1229 _] -> [_ _ _ _ _ w1273]
                    seq-local: [w752 _ _ _ _ _] -> [_ w831 _ _ _ _]
                    seq-local: [w750 _ _ _ _ _] -> [_ _ w1029 _ _ _]
                    tunnel: w749 -> [_ w868 _ _ _ _]
                    tunnel: w709 -> [w763 _ _ _ _ _]
                    tunnel: w710 -> [w762 _ _ _ _ _]
                    tunnel: [_ _ _ _ _ w1270] -> w746
                    tunnel: [_ _ _ _ _ w1269] -> w741
                    tunnel: [_ _ _ _ w1250 _] -> w744
                    tunnel: [_ w854 _ _ _ _] -> w743
                    tunnel: [_ w850 _ _ _ _] -> w716
                    tunnel: [_ _ w1032 _ _ _] -> w714
                    tunnel: [_ _ _ w1185 _ _] -> w728
                    tunnel: [_ _ _ _ w1243 _] -> w738
                    tunnel: w737 -> [_ _ w1031 _ _ _]
                    tunnel: w736 -> [_ w845 _ _ _ _]
                    tunnel: w735 -> [_ _ w1030 _ _ _]
                    tunnel: w734 -> [_ _ _ w1188 _ _]
                    tunnel: w733 -> [_ _ _ _ w1246 _]
                    tunnel: w732 -> [_ w839 _ _ _ _]
                    tunnel: w731 -> [_ w848 _ _ _ _]
                    tunnel: w730 -> [_ w853 _ _ _ _]
                    tunnel: w729 -> [_ w846 _ _ _ _]
                    tunnel: w726 -> [_ _ _ _ w1232 _]
                    tunnel: w725 -> [w760 _ _ _ _ _]
                    tunnel: [w764 _ _ _ _ _] -> w715
                    tunnel: [w753 _ _ _ _ _] -> w724
                    tunnel: w723 -> [w761 _ _ _ _ _]
                    tunnel: w712 -> [w756 _ _ _ _ _]
                    tunnel: w721 -> [_ _ _ _ _ w1272]
                    tunnel: [_ _ _ _ w1238 _] -> w720
                    tunnel: w719 -> [_ _ _ w1191 _ _]
                    tunnel: [_ _ _ _ _ w1266] -> w718
                    tunnel: w717 -> [_ _ _ _ _ w1271]
                    tunnel: w713 -> [_ w833 _ _ _ _]
                    tunnel: [_ _ w1028 _ _ _] -> w707
                    tunnel: w706 -> [_ _ w1027 _ _ _]
                    frame #0 {
                      # "ElecGain"
                      # "LineWidth"
                      # "Not Found"
                      n286 = for {
                        shift-right: [w771] -> w759
                        shift-left: w763 -> [w785]
                        shift-right: [w768] -> w758
                        shift-left: w762 -> [w784]
                        tunnel: [w767] -> w753 mode=indexing
                        tunnel: [w778] -> w757 mode=indexing
                        tunnel: w760 -> [w774]
                        tunnel: w761 -> [w769] mode=indexing
                        tunnel: w756 -> [w770]
                        i -> [w766]
                        n287 = call-poly <vilib>:"Read Key.vi"("section"=w774, "error in (no error)"=w784, "key"=w769, "refnum"=w785) -> ("error out"=w772:errorcluster, "value"=w780:string, "found?"=w779:bool, "refnum out"=w773:T19)  [unwired: 2 in, 2 out]
                        n288 = Decimal String To Number(string=w780) -> (number=w765:i32)  [unwired: 3 out]
                        n289 = Not(x=w779) -> (.not. x?=w782:bool)
                        n290 = Equal?(x="", y=w780) -> (x = y?=w781:bool)
                        n291 = Equal To 0?(x=w766) -> (x = 0?=w776:bool)
                        n292 = Or(x=w782, y=w781) -> (x .or. y?=w778:bool)
                        n293 = Not Equal To 0?(x=w765) -> (x != 0?=w777:bool)
                        n294 = And(x=w777, y=w776) -> (x .and. y?=w775:bool)
                        n295 = case shown="True" w775 {
                          tunnel: w769 -> [_ w804]
                          tunnel: w774 -> [_ w803]
                          tunnel: w773 -> [w795 w802]
                          tunnel: w772 -> [w796 w801]
                          tunnel: w770 -> [_ w800]
                          tunnel: [w796 w799] -> w768
                          tunnel: [w795 w798] -> w771
                          frame False {
                          }
                          frame True {
                            n296 = call "Act_Warning.vi"() -> ("Warning?"=w797:bool)  [unwired: 1 out]
                            n297 = case shown="False" w797 {
                              tunnel: w804 -> [w810 _]
                              tunnel: w803 -> [w812 _]
                              tunnel: w802 -> [w811 w827]
                              tunnel: w801 -> [w805 w828]
                              tunnel: w800 -> [w809 _]
                              tunnel: [w807 w828] -> w799
                              tunnel: [w806 w827] -> w798
                              frame False {
                                n298 = flat-sequence {
                                tunnel: w812 -> [w822]
                                tunnel: w805 -> [w821]
                                tunnel: w811 -> [w820]
                                tunnel: w810 -> [w819]
                                tunnel: [w814] -> w808
                                tunnel: w809 -> [w826]
                                tunnel: w808 -> [w825]
                                tunnel: [w823] -> w807
                                tunnel: [w824] -> w806
                                frame #0 {
                                w813 = "0"  # No Warning
                                w817 = TRUE  # write configuration file? (T)
                                n299 = call-poly <vilib>:"Write Key.vi"("section"=w822, "error in (no error)"=w821, "value"=w813, "key"=w819, "refnum"=w820) -> ("error out"=w815:errorcluster, "refnum out"=w816:T19)  [unwired: 1 in, 4 out]
                                n300 = call <vilib>:"Close Config Data.vi"("error in (no error)"=w815, "write file if changed (T)"=w817, "refnum"=w816) -> ("error out"=w818:errorcluster)  [unwired: 8 out]
                                n301 = call <vilib>:"General Error Handler.vi"("error in (no error)"=w818) -> ("error out"=w814:errorcluster)  [unwired: 2 in, 12 out]
                                }
                                frame #1 {
                                n302 = call <vilib>:"Open Config Data.vi"("error in (no error)"=w825, "configuration file path"=w826) -> ("error out"=w823:errorcluster, "refnum"=w824:T19)  [unwired: 7 in, 1 out]
                                }
                                }
                              }
                              frame True {
                              }
                            }
                          }
                        }
                        n303 = case shown="4" w766 {
                          tunnel: w765 -> [w786 w790 w794]
                          tunnel: [w786 w787 w791] -> w767
                          frame 0, Default {
                          }
                          frame 4 {
                            # "LineWidth"
                            n304 = In Range and Coerce(upper limit=1, x=w790, lower limit=5) -> (coerced(x)=w787:i32)  [unwired: 1 out]
                          }
                          frame 5 {
                            # "Cursor"
                            n305 = In Range and Coerce(upper limit=0, x=w794, lower limit=1) -> (coerced(x)=w791:i32)  [unwired: 1 out]
                          }
                        }
                      }
                      n306 = Index Array(array=w753, index #1=2 ("index"), index #2=4 ("index")) -> (element #1=w750:i32, element #2=w754:i32)
                      n307 = To Unsigned Byte Integer(number=w754) -> (unsigned 8bit integer=w752:u8)
                      n308 = Or Array Elements(Boolean array=w757) -> (logical OR=w764:bool)
                    }
                    frame #1 {
                      w830 = 3
                      # "Not Found"
                      # "Vbat is not a trace"
                      n309 = Decrement(x=w853) -> (x-1=w832:i32)
                      n310 = Add(x=w848, y=w839) -> (x+y=w838:i32)
                      n311 = Add(x=w848, y=w839) -> (x+y=w849:i32)
                      n312 = Add(x=w838, y=w853) -> (x+y=w837:i32)
                      n313 = Add(x=w837, y=w833) -> (x+y=w836:i32)
                      n314 = Add(x=w836, y=w846) -> (x+y=w851:i32)
                      n315 = for {
                        N: w849 -> [_]
                        tunnel: w831 -> [w950]
                        i -> [w949]
                        n316 = To Unsigned Long Integer(number=w949) -> (unsigned 32bit integer=w948:u32)
                        n317 = property on="Mon Chart" class="WFChart (strict)"("Active Plot"=w948, "Plot.Line Width"=w950) -> ()  [unwired: 2 in, 2 out]
                      }
                      n318 = for {
                        N: w848 -> [_]
                        tunnel: w831 -> [w947]
                        i -> [w946]
                        n319 = To Unsigned Long Integer(number=w946) -> (unsigned 32bit integer=w945:u32)
                        n320 = property on="Bip Chart" class="WFChart (strict)"("Active Plot"=w945, "Plot.Line Width"=w947) -> ()  [unwired: 2 in, 2 out]
                      }
                      n321 = To Unsigned Long Integer(number=w849) -> (unsigned 32bit integer=w867:u32)
                      n322 = To Unsigned Long Integer(number=w848) -> (unsigned 32bit integer=w856:u32)
                      n323 = To Unsigned Long Integer(number=w832) -> (unsigned 32bit integer=w855:u32)
                      n324 = To Unsigned Long Integer(number=w833) -> (unsigned 32bit integer=w847:u32)
                      n325 = To Unsigned Long Integer(number=w846) -> (unsigned 32bit integer=w852:u32)
                      n326 = To Unsigned Long Integer(number=w830) -> (unsigned 32bit integer=w829:u32)
                      n327 = Increment(x=w851) -> (x+1=w842:i32)
                      n328 = for {
                        N: w842 -> [w883]
                        shift-right: [w904] -> w841
                        shift-left: w844 -> [w906]
                        shift-right: [w903] -> w840
                        shift-left: w843 -> [w905]
                        tunnel: [w880] -> w834 mode=indexing
                        tunnel: [w892] -> w835 mode=indexing
                        tunnel: w839 -> [w884]
                        tunnel: w838 -> [w895]
                        tunnel: w845 -> [w879]
                        tunnel: w837 -> [w885]
                        tunnel: w836 -> [w872]
                        i -> [w874]
                        n329 = Increment(x=w874) -> (x+1=w882:i32)
                        n330 = Greater Or Equal?(x=w874, y=w895) -> (x >= y?=w900:bool)
                        n331 = Greater Or Equal?(x=w874, y=w884) -> (x >= y?=w902:bool)
                        n332 = Greater Or Equal?(x=w874, y=w885) -> (x >= y?=w886:bool)
                        n333 = Greater Or Equal?(x=w874, y=w872) -> (x >= y?=w873:bool)
                        n334 = Select(t=i8 1, s=w902, f=i8 0) -> (s? t:f=w901:i8)
                        n335 = Equal?(x=w883, y=w882) -> (x = y?=w875:bool)
                        n336 = Select(t=i8 2, s=w900, f=w901) -> (s? t:f=w889:i8)
                        n337 = Select(t=i8 3, s=w886, f=w889) -> (s? t:f=w888:i8)
                        n338 = Select(t=i8 4, s=w873, f=w888) -> (s? t:f=w877:i8)
                        n339 = Select(t=i8 5, s=w875, f=w877) -> (s? t:f=w878:i8)
                        n340 = case shown="5" w878 {
                          tunnel: [w910 w916 w922 w928 w934 "Trig" ("string")] -> w881
                          tunnel: w882 -> [w907 w914 w921 w925 w931 _]
                          tunnel: w884 -> [_ w913 _ _ _ _]
                          tunnel: w895 -> [_ _ w919 _ _ _]
                          tunnel: w885 -> [_ _ _ w923 _ _]
                          tunnel: w872 -> [_ _ _ _ w929 _]
                          frame 0, Default {
                            n341 = Number To Decimal String(number=w907) -> (decimal integer string=w908:string)  [unwired: 1 out]
                            n342 = Concatenate Strings("Chan" ("string"), w908) -> (w910:string)
                          }
                          frame 1 {
                            n343 = Subtract(x=w914, y=w913) -> (x-y=w911:i32)
                            n344 = Number To Decimal String(number=w911) -> (decimal integer string=w912:string)  [unwired: 1 out]
                            n345 = Concatenate Strings("Tou" ("string"), w912) -> (w916:string)
                          }
                          frame 2 {
                            n346 = Subtract(x=w921, y=w919) -> (x-y=w917:i32)
                            n347 = Number To Decimal String(number=w917) -> (decimal integer string=w918:string)  [unwired: 1 out]
                            n348 = Concatenate Strings("Aux" ("string"), w918) -> (w922:string)
                          }
                          frame 3 {
                            n349 = Subtract(x=w925, y=w923) -> (x-y=w924:i32)
                            n350 = Number To Decimal String(number=w924) -> (decimal integer string=w926:string)  [unwired: 1 out]
                            n351 = Concatenate Strings("Jazz" ("string"), w926) -> (w928:string)
                          }
                          frame 4 {
                            n352 = Subtract(x=w931, y=w929) -> (x-y=w930:i32)
                            n353 = Number To Decimal String(number=w930) -> (decimal integer string=w932:string)  [unwired: 1 out]
                            n354 = Concatenate Strings("Box" ("string"), w932) -> (w934:string)
                          }
                          frame 5 {
                          }
                        }
                        n355 = call-poly <vilib>:"Read Key.vi"("section"=w879, "error in (no error)"=w905, "key"=w881, "refnum"=w906) -> ("error out"=w903:errorcluster, "value"=w880:string, "found?"=w894:bool, "refnum out"=w904:T19)  [unwired: 2 in, 2 out]
                        n356 = Equal?(x="", y=w880) -> (x = y?=w890:bool)
                        n357 = Not(x=w894) -> (.not. x?=w893:bool)
                        n358 = Or(x=w890, y=w893) -> (x .or. y?=w892:bool)
                      }
                      n359 = property on="Mon Chart" class="WFChart (strict)"("Legend:Plots Shown"=w867) -> ()  [unwired: 2 in, 2 out]
                      n360 = property on="Bip Chart" class="WFChart (strict)"("Legend:Plots Shown"=w856) -> ()  [unwired: 2 in, 2 out]
                      n361 = property on="Aux Chart" class="WFChart (strict)"("Legend:Plots Shown"=w855) -> ()  [unwired: 2 in, 2 out]
                      n362 = property on="Jazz Chart" class="WFChart (strict)"("LegPlots"=w847) -> ()  [unwired: 2 in, 2 out]
                      n363 = property on="Ana Chart" class="WFChart (strict)"("Legend:Plots Shown"=w852) -> ()  [unwired: 2 in, 2 out]
                      n364 = property on="ABR Chart" class="WFChart (strict)"("Legend:Plots Shown"=w829) -> ()  [unwired: 2 in, 2 out]
                      n365 = Or Array Elements(Boolean array=w835) -> (logical OR=w850:bool)
                      n366 = Quotient & Remainder(x=w839, y=2) -> (floor(x/y)=w857:i32)  [unwired: 1 out]
                      n367 = case shown="False" w850 {
                        tunnel: w838 -> [w962 _]
                        tunnel: w848 -> [w961 _]
                        tunnel: w832 -> [w960 _]
                        tunnel: w839 -> [w959 _]
                        tunnel: w836 -> [w958 _]
                        tunnel: w846 -> [w957 _]
                        tunnel: w834 -> [w953 _]
                        tunnel: w833 -> [w955 _]
                        tunnel: w837 -> [w952 _]
                        frame False {
                          n368 = for {
                            N: w960 -> [_]
                            tunnel: w953 -> [w979]
                            tunnel: w962 -> [w980]
                            tunnel: [w978] -> w951 mode=indexing
                            i -> [w982]
                            n369 = Add(x=w980, y=w982) -> (x+y=w983:i32)
                            n370 = Index Array(array=w979, index=w983) -> (element=w984:string)
                            n371 = String Subset(string=w984, length (rest)=4 ("length (rest)")) -> (substring=w978:string)  [unwired: 1 out]
                          }
                          n372 = for {
                            N: w955 -> [_]
                            tunnel: w953 -> [w965]
                            tunnel: w952 -> [w966]
                            tunnel: [w964] -> w954 mode=indexing
                            i -> [w968]
                            n373 = Add(x=w966, y=w968) -> (x+y=w969:i32)
                            n374 = Index Array(array=w965, index=w969) -> (element=w970:string)
                            n375 = String Subset(string=w970, length (rest)=4 ("length (rest)")) -> (substring=w964:string)  [unwired: 1 out]
                          }
                          n376 = for {
                            N: w957 -> [_]
                            tunnel: w953 -> [w972]
                            tunnel: w958 -> [w973]
                            tunnel: [w971] -> w956 mode=indexing
                            i -> [w975]
                            n377 = Add(x=w973, y=w975) -> (x+y=w976:i32)
                            n378 = Index Array(array=w972, index=w976) -> (element=w977:string)
                            n379 = String Subset(string=w977, length (rest)=8 ("length (rest)")) -> (substring=w971:string)  [unwired: 1 out]
                          }
                          n380 = for {
                            N: w961 -> [w992]
                            tunnel: w953 -> [w997]
                            tunnel: w959 -> [w990]
                            tunnel: [w993] -> w963 mode=indexing
                            i -> [w988]
                            w985 = 4 ("length (rest)")
                            n381 = Increment(x=w988) -> (x+1=w987:i32)
                            n382 = Quotient & Remainder(x=w987, y=w992) -> (x-y*floor(x/y)=w986:i32)  [unwired: 1 out]
                            n383 = Add(x=w990, y=w988) -> (x+y=w991:i32)
                            n384 = Add(x=w990, y=w986) -> (x+y=w989:i32)
                            n385 = Index Array(array=w997, index=w991) -> (element=w999:string)
                            n386 = Index Array(array=w997, index=w989) -> (element=w998:string)
                            n387 = String Subset(string=w998, length (rest)=w985) -> (substring=w995:string)  [unwired: 1 out]
                            n388 = String Subset(string=w999, length (rest)=w985) -> (substring=w996:string)  [unwired: 1 out]
                            n389 = Concatenate Strings(w996, "-" ("string"), w995) -> (w993:string)
                          }
                          n390 = property on="AuxFree" class="LstBox (strict)"("Item Names"=w951) -> ()  [unwired: 2 in, 2 out]
                          n391 = property on="JazzFree" class="LstBox (strict)"("Item Names"=w954) -> ()  [unwired: 2 in, 2 out]
                          n392 = property on="AnaFree" class="LstBox (strict)"("Item Names"=w956) -> ()  [unwired: 2 in, 2 out]
                          n393 = property on="AnaOffset" class="Ring (strict)"("Strings []"=w956) -> ()  [unwired: 2 in, 2 out]
                          n394 = property on="BipFree" class="LstBox (strict)"("Item Names"=w963) -> ()  [unwired: 2 in, 2 out]
                        }
                        frame True {
                        }
                      }
                      n395 = Increment(x=w857) -> (x+1=w865:i32)
                      n396 = Increment(x=w857) -> (x+1=w860:i32)
                      n397 = for {
                        N: w830 -> [_]
                        tunnel: w831 -> [w871]
                        i -> [w870]
                        n398 = To Unsigned Long Integer(number=w870) -> (unsigned 32bit integer=w869:u32)
                        n399 = property on="ABR Chart" class="WFChart (strict)"("Active Plot"=w869, "Plot.Line Width"=w871) -> ()  [unwired: 2 in, 2 out]
                      }
                      n400 = for {
                        N: w833 -> [_]
                        tunnel: w831 -> [w938]
                        i -> [w937]
                        n401 = To Unsigned Long Integer(number=w937) -> (unsigned 32bit integer=w936:u32)
                        n402 = property on="Jazz Chart" class="WFChart (strict)"("Active Plot"=w936, "Plot.Line Width"=w938) -> ()  [unwired: 2 in, 2 out]
                      }
                      n403 = Increment(x=w860) -> (x+1=w866:i32)
                      n404 = Increment(x=w865) -> (x+1=w862:i32)
                      n405 = for {
                        N: w866 -> [w1006]
                        tunnel: [w1002] -> w859 mode=indexing
                        tunnel: [w1000] -> w861
                        i -> [w1009]
                        w1000 = 1.0 ("X Scale.Offset and Multiplier:Offset")
                        w1010 = 0.5 ("f")
                        n406 = Decrement(x=w1006) -> (x-1=w1005:i32)
                        n407 = Equal To 0?(x=w1009) -> (x = 0?=w1012:bool)
                        n408 = Equal?(x=w1005, y=w1009) -> (x = y?=w1008:bool)
                        n409 = To Double Precision Float(number=w1009) -> (double precision float=w1011:dbl)
                        n410 = To Double Precision Float(number=w1005) -> (double precision float=w1004:dbl)
                        n411 = Select(t=w1010, s=w1012, f=w1011) -> (s? t:f=w1007:dbl)
                        n412 = Subtract(x=w1004, y=w1010) -> (x-y=w1003:dbl)
                        n413 = Select(t=w1003, s=w1008, f=w1007) -> (s? t:f=w1001:dbl)
                        n414 = Subtract(x=w1001, y=w1000) -> (x-y=w1002:dbl)
                      }
                      n415 = for {
                        N: w862 -> [w1020]
                        tunnel: [w1013] -> w863 mode=indexing
                        tunnel: [w1015] -> w864
                        tunnel: w865 -> [w1016]
                        i -> [w1023]
                        w1024 = 0.5 ("f")
                        n416 = Decrement(x=w1020) -> (x-1=w1019:i32)
                        n417 = Equal To 0?(x=w1023) -> (x = 0?=w1026:bool)
                        n418 = Equal?(x=w1019, y=w1023) -> (x = y?=w1022:bool)
                        n419 = To Double Precision Float(number=w1023) -> (double precision float=w1025:dbl)
                        n420 = To Double Precision Float(number=w1019) -> (double precision float=w1018:dbl)
                        n421 = Select(t=w1024, s=w1026, f=w1025) -> (s? t:f=w1021:dbl)
                        n422 = Subtract(x=w1018, y=w1024) -> (x-y=w1017:dbl)
                        n423 = To Double Precision Float(number=w1016) -> (double precision float=w1015:dbl)
                        n424 = Select(t=w1017, s=w1022, f=w1021) -> (s? t:f=w1014:dbl)
                        n425 = Decrement(x=w1014) -> (x-1=w1013:dbl)
                      }
                      n426 = for {
                        N: w846 -> [_]
                        tunnel: w831 -> [w941]
                        i -> [w940]
                        n427 = To Unsigned Long Integer(number=w940) -> (unsigned 32bit integer=w939:u32)
                        n428 = property on="Ana Chart" class="WFChart (strict)"("Active Plot"=w939, "Plot.Line Width"=w941) -> ()  [unwired: 2 in, 2 out]
                      }
                      n429 = for {
                        N: w832 -> [_]
                        tunnel: w831 -> [w944]
                        i -> [w943]
                        n430 = To Unsigned Long Integer(number=w943) -> (unsigned 32bit integer=w942:u32)
                        n431 = property on="Aux Chart" class="WFChart (strict)"("Active Plot"=w942, "Plot.Line Width"=w944) -> ()  [unwired: 2 in, 2 out]
                      }
                      n432 = property on="Offset Graph First Half" class="WFGraph (strict)"("X Scale.Marker Values[]"=w859) -> ()  [unwired: 2 in, 2 out]
                      n433 = property on="Offset Graph  Second Half" class="WFGraph (strict)"("X Scale.Marker Values[]"=w863) -> ()  [unwired: 2 in, 2 out]
                      n434 = Bundle By Name(cluster=w868, "All Labels"=w834) -> (w854:T10)
                      n435 = property on="Offset Graph First Half" class="WFGraph (strict)"("X Scale.Offset and Multiplier:Offset"=w861) -> ()  [unwired: 2 in, 2 out]
                      n436 = property on="Offset Graph  Second Half" class="WFGraph (strict)"("X Scale.Offset and Multiplier:Offset"=w864) -> ()  [unwired: 2 in, 2 out]
                    }
                    frame #2 {
                      # "not found"
                      n437 = for {
                        shift-right: [w1183] -> w1036
                        shift-left: w1038 -> [w1181]
                        shift-right: [w1182] -> w1035
                        shift-left: w1037 -> [w1180]
                        tunnel: [w1179] -> w1034 mode=indexing
                        tunnel: w1031 -> [w1178] mode=indexing
                        tunnel: [w1172] -> w1033 mode=indexing
                        tunnel: w1030 -> [w1171]
                        n438 = call-poly <vilib>:"Read Key.vi"("section"=w1171, "error in (no error)"=w1180, "key"=w1178, "refnum"=w1181) -> ("error out"=w1182:errorcluster, "value"=w1176:string, "found?"=w1177:bool, "refnum out"=w1183:T19)  [unwired: 2 in, 2 out]
                        n439 = Not(x=w1177) -> (.not. x?=w1174:bool)
                        n440 = Equal?(x="", y=w1176) -> (x = y?=w1173:bool)
                        n441 = Decimal String To Number(string=w1176) -> (number=w1179:i32)  [unwired: 3 out]
                        n442 = Or(x=w1174, y=w1173) -> (x .or. y?=w1172:bool)
                      }
                      n443 = Or Array Elements(Boolean array=w1033) -> (logical OR=w1032:bool)
                      n444 = case shown="False" w1032 {
                        tunnel: w1034 -> [w1167 _]
                        tunnel: w1029 -> [w1084 _]
                        tunnel: [w1040 w1170] -> w1028
                        tunnel: w1027 -> [w1039 w1170]
                        frame False {
                          n445 = Index Array(array=w1167) -> (element #1=w1064:i32, element #2=w1063:i32, element #3=w1062:i32, element #4=w1061:i32, element #5=w1060:i32, element #6=w1059:i32, element #7=w1058:i32, element #8=w1057:i32, element #9=w1056:i32, element #10=w1055:i32, element #11=w1054:i32, element #12=w1053:i32, element #13=w1045:i32, element #14=w1046:i32, element #15=w1047:i32, element #16=w1048:i32, element #17=w1049:i32, element #18=w1050:i32, element #19=w1051:i32, element #20=w1052:i32, element #21=w1065:i32, element #22=w1066:i32, element #23=w1068:i32, element #24=w1070:i32, element #25=w1071:i32, element #26=w1072:i32, element #27=w1073:i32, element #28=w1074:i32, element #29=w1076:i32, element #30=w1078:i32, element #31=w1079:i32, element #32=w1131:i32, element #33=w1130:i32, element #34=w1127:i32, element #35=w1125:i32, element #36=w1112:i32, element #37=w1123:i32, element #38=w1119:i32, element #39=w1118:i32, element #40=w1117:i32, element #41=w1116:i32, element #42=w1115:i32, element #43=w1109:i32, element #44=w1108:i32, element #45=w1107:i32, element #46=w1106:i32, element #47=w1105:i32, element #48=w1095:i32, element #49=w1094:i32, element #50=w1096:i32, element #51=w1097:i32, element #52=w1098:i32, element #53=w1099:i32, element #54=w1100:i32, element #55=w1101:i32, element #56=w1102:i32)  [unwired: 56 in]
                          n446 = case shown="0, Default" w1084 {
                            tunnel: [i32[] [4] ("Disabled Items []") i32[] [] ("Disabled Items []")] -> w1083
                            frame 0, Default {
                            }
                            frame 1 {
                            }
                          }
                          n447 = Not Equal To 0?(x=w1123) -> (x != 0?=w1124:bool)
                          n448 = To Double Precision Float(number=w1100) -> (double precision float=w1147:dbl)
                          n449 = Not Equal To 0?(x=w1105) -> (x != 0?=w1151:bool)
                          n450 = Not Equal To 0?(x=w1125) -> (x != 0?=w1126:bool)
                          n451 = To Double Precision Float(number=w1119) -> (double precision float=w1122:dbl)
                          n452 = To Double Precision Float(number=w1118) -> (double precision float=w1121:dbl)
                          n453 = To Double Precision Float(number=w1117) -> (double precision float=w1120:dbl)
                          n454 = To Double Precision Float(number=w1052) -> (double precision float=w1157:dbl)
                          n455 = Not Equal To 0?(x=w1095) -> (x != 0?=w1093:bool)
                          n456 = To Byte Integer(number=w1106) -> (8bit integer=w1149:i8)
                          n457 = To Double Precision Float(number=w1098) -> (double precision float=w1144:dbl)
                          n458 = To Byte Integer(number=w1107) -> (8bit integer=w1150:i8)
                          n459 = To Byte Integer(number=w1115) -> (8bit integer=w1137:i8)
                          n460 = Not Equal To 0?(x=w1094) -> (x != 0?=w1092:bool)
                          n461 = Not Equal To 0?(x=w1097) -> (x != 0?=w1145:bool)
                          n462 = To Double Precision Float(number=w1074) -> (double precision float=w1081:dbl)
                          n463 = To Byte Integer(number=w1066) -> (8bit integer=w1086:i8)
                          n464 = To Long Integer(number=w1131) -> (32bit integer=w1132:i32)
                          n465 = To Byte Integer(number=w1046) -> (8bit integer=w1139:i8)
                          n466 = To Byte Integer(number=w1048) -> (8bit integer=w1158:i8)
                          n467 = To Byte Integer(number=w1079) -> (8bit integer=w1133:i8)
                          n468 = To Byte Integer(number=w1116) -> (8bit integer=w1103:i8)
                          n469 = To Double Precision Float(number=w1112) -> (double precision float=w1114:dbl)
                          n470 = To Byte Integer(number=w1078) -> (8bit integer=w1077:i8)
                          n471 = Not Equal To 0?(x=w1099) -> (x != 0?=w1143:bool)
                          n472 = To Byte Integer(number=w1096) -> (8bit integer=w1142:i8)
                          n473 = To Byte Integer(number=w1108) -> (8bit integer=w1136:i8)
                          n474 = To Double Precision Float(number=w1072) -> (double precision float=w1043:dbl)
                          n475 = To Double Precision Float(number=w1054) -> (double precision float=w1162:dbl)
                          n476 = Not Equal To 0?(x=w1055) -> (x != 0?=w1163:bool)
                          n477 = To Byte Integer(number=w1059) -> (8bit integer=w1159:i8)
                          n478 = Not Equal To 0?(x=w1051) -> (x != 0?=w1153:bool)
                          n479 = Divide(x=w1147, y=100.0) -> (x/y=w1146:dbl)
                          n480 = To Byte Integer(number=w1070) -> (8bit integer=w1069:i8)
                          n481 = To Quad Integer(1:w1063) -> (0:w1104:i64)
                          n482 = To Double Precision Float(number=w1050) -> (double precision float=w1154:dbl)
                          n483 = To Double Precision Float(number=w1127) -> (double precision float=w1128:dbl)
                          n484 = Not Equal To 0?(x=w1109) -> (x != 0?=w1110:bool)
                          n485 = Not Equal To 0?(x=w1062) -> (x != 0?=w1134:bool)
                          n486 = Not Equal To 0?(x=w1101) -> (x != 0?=w1135:bool)
                          n487 = To Double Precision Float(number=w1056) -> (double precision float=w1164:dbl)
                          n488 = To Byte Integer(number=w1060) -> (8bit integer=w1141:i8)
                          n489 = Not Equal To 0?(x=w1130) -> (x != 0?=w1129:bool)
                          n490 = To Byte Integer(number=w1058) -> (8bit integer=w1166:i8)
                          n491 = Not Equal To 0?(x=w1049) -> (x != 0?=w1155:bool)
                          n492 = To Byte Integer(number=w1047) -> (8bit integer=w1091:i8)
                          n493 = Divide(x=w1157, y=100.0) -> (x/y=w1152:dbl)
                          n494 = Not Equal To 0?(x=w1057) -> (x != 0?=w1165:bool)
                          n495 = To Byte Integer(number=w1065) -> (8bit integer=w1138:i8)
                          n496 = Not Equal To 0?(x=w1045) -> (x != 0?=w1082:bool)
                          n497 = Not Equal To 0?(x=w1071) -> (x != 0?=w1044:bool)
                          n498 = To Byte Integer(number=w1076) -> (8bit integer=w1075:i8)
                          n499 = Not Equal To 0?(x=w1068) -> (x != 0?=w1067:bool)
                          n500 = Divide(x=w1081, y=100.0) -> (x/y=w1041:dbl)
                          n501 = Divide(x=w1162, y=100.0) -> (x/y=w1160:dbl)
                          n502 = To Byte Integer(number=w1053) -> (8bit integer=w1140:i8)
                          n503 = Divide(x=w1114, y=100.0) -> (x/y=w1111:dbl)
                          n504 = Not Equal To 0?(x=w1073) -> (x != 0?=w1042:bool)
                          n505 = To Byte Integer(number=w1083) -> (8bit integer=w1087:i8[])
                          n506 = property on="OffsetScale" class="Ring (strict)"("Disabled Items []"=w1083) -> ()  [unwired: 2 in, 2 out]
                          n507 = local write "ScreenLength"(w1064) -> ()
                          n508 = local write "FileLimit"(w1104) -> ()
                          n509 = local write "FileAppend"(w1134) -> ()
                          n510 = local write "RecTimeLimit"(w1061) -> ()
                          n511 = local write "Decimation"(w1141) -> ()
                          n512 = local write "Buffer"(w1159) -> ()
                          n513 = local write "MonScale"(w1166) -> ()
                          n514 = local write "MonLP"(w1165) -> ()
                          n515 = local write "MonLPfreq"(w1164) -> ()
                          n516 = local write "MonHP"(w1163) -> ()
                          n517 = local write "MonHPfreq"(w1160) -> ()
                          n518 = local write "Channels"(w1140) -> ()
                          n519 = local write "AddTP"(w1082) -> ()
                          n520 = local write "Reference"(w1139) -> ()
                          n521 = local write "TrigCode"(w1091) -> ()
                          n522 = local write "BipScale"(w1158) -> ()
                          n523 = local write "BipLP"(w1155) -> ()
                          n524 = local write "BipLPfreq"(w1154) -> ()
                          n525 = local write "BipHP"(w1153) -> ()
                          n526 = local write "BipHPfreq"(w1152) -> ()
                          n527 = local write "Offset"(w1138) -> ()
                          n528 = local write "AbrOn"(w1067) -> ()
                          n529 = local write "AbrScale"(w1069) -> ()
                          n530 = local write "AbrChannels"(w1075) -> ()
                          n531 = local write "AbrOffsetScale"(w1077) -> ()
                          n532 = local write "AvgTrigLog"(w1133) -> ()
                          n533 = local write "AvgSweep"(w1132) -> ()
                          n534 = local write "AvgLP"(w1129) -> ()
                          n535 = local write "AvgLPfreq"(w1128) -> ()
                          n536 = local write "AvgHP"(w1126) -> ()
                          n537 = local write "AvgHPfreq"(w1111) -> ()
                          n538 = local write "AvgAutoscale"(w1124) -> ()
                          n539 = local write "AvgScale"(w1122) -> ()
                          n540 = local write "AvgAbsReject"(w1121) -> ()
                          n541 = local write "AvgRelReject"(w1120) -> ()
                          n542 = local write "GsrScale"(w1103) -> ()
                          n543 = local write "ErgoScale"(w1137) -> ()
                          n544 = local write "ErgoLP"(w1110) -> ()
                          n545 = local write "RespScale"(w1136) -> ()
                          n546 = local write "PletScale"(w1150) -> ()
                          n547 = local write "TempScale"(w1149) -> ()
                          n548 = local write "AuxReset"(w1151) -> ()
                          n549 = local write "JazzOn"(w1093) -> ()
                          n550 = local write "JazzReset"(w1092) -> ()
                          n551 = local write "AnaScale"(w1142) -> ()
                          n552 = local write "AnaLP"(w1145) -> ()
                          n553 = local write "AnaLPfreq"(w1144) -> ()
                          n554 = local write "AnaHP"(w1143) -> ()
                          n555 = local write "AnaHPfreq"(w1146) -> ()
                          n556 = local write "AnaReset"(w1135) -> ()
                          n557 = local write "AnaOffset"(w1102) -> ()
                          n558 = Search 1D Array(1D array=w1087, element=w1086) -> (index of element=w1088:i32)  [unwired: 1 out]
                          n559 = Less Than 0?(x=w1088) -> (x < 0?=w1089:bool)
                          n560 = Bundle By Name(cluster=w1039, "AbrLP"=w1044, "AbrLPfreq"=w1043, "AbrHP"=w1042, "AbrHPfreq"=w1041) -> (w1040:T7)
                          n561 = Select(t=w1086, s=w1089, f=i8 3) -> (s? t:f=w1085:i8)
                          n562 = local write "OffsetScale"(w1085) -> ()
                        }
                        frame True {
                        }
                      }
                    }
                    frame #3 {
                      w1184 = FALSE  # Not found
                      # "not found"
                      n563 = for {
                        tunnel: w1191 -> [w1199] mode=indexing
                        shift-right: [w1203] -> w1186
                        shift-left: w1189 -> [w1206]
                        shift-right: [w1204] -> w1187
                        shift-left: w1190 -> [w1207]
                        tunnel: w1188 -> [w1205]
                        shift-right: [w1192] -> w1185
                        shift-left: w1184 -> [w1194]
                        i -> [w1198]
                        n564 = call-poly <vilib>:"Read Key.vi"("section"=w1205, "error in (no error)"=w1206, "key"=w1199, "refnum"=w1207) -> ("error out"=w1203:errorcluster, "value"=w1200:string, "found?"=w1201:bool, "refnum out"=w1204:T19)  [unwired: 2 in, 2 out]
                        n565 = Not(x=w1201) -> (.not. x?=w1195:bool)
                        n566 = Equal?(x="", y=w1200) -> (x = y?=w1196:bool)
                        n567 = call "CFGtoArray.vi"("Cofiguration String"=w1200) -> ("Selector Array"=w1197:i32[])
                        n568 = Or(x=w1195, y=w1196) -> (x .or. y?=w1193:bool)
                        n569 = case shown="False" w1193 {
                          tunnel: w1198 -> [w1209 _]
                          tunnel: w1197 -> [w1208 _]
                          frame False {
                            n570 = case shown="8" w1209 {
                              tunnel: w1208 -> [w1210 w1211 w1212 w1213 w1215 w1218 w1221 w1223 w1226 w1227 w1228]
                              frame 0, Default {
                                n571 = local write "MonFree"(w1210) -> ()
                              }
                              frame 1 {
                                n572 = local write "RefFree"(w1211) -> ()
                              }
                              frame 2 {
                                n573 = local write "BipFree"(w1212) -> ()
                              }
                              frame 3 {
                                n574 = local write "AvgTrigSel"(w1213) -> ()
                              }
                              frame 4 {
                                n575 = Index Array(array=w1215) -> (element=w1214:i32)  [unwired: 1 in]
                                n576 = local write "MonFreeAvg1"(w1214) -> ()
                              }
                              frame 5 {
                                n577 = Array Size(array=w1218) -> (size(s)=w1217:i32)
                                n578 = Not Equal To 0?(x=w1217) -> (x != 0?=w1216:bool)
                                n579 = case shown="True" w1216 {
                                tunnel: w1218 -> [_ w1219]
                                frame False {
                                }
                                frame True {
                                n580 = local write "RefFreeAvg1"(w1219) -> ()
                                }
                                }
                              }
                              frame 6 {
                                n581 = Index Array(array=w1221) -> (element=w1220:i32)  [unwired: 1 in]
                                n582 = local write "MonFreeAvg2"(w1220) -> ()
                              }
                              frame 7 {
                                n583 = Array Size(array=w1223) -> (size(s)=w1224:i32)
                                n584 = Not Equal To 0?(x=w1224) -> (x != 0?=w1222:bool)
                                n585 = case shown="True" w1222 {
                                tunnel: w1223 -> [_ w1225]
                                frame False {
                                }
                                frame True {
                                n586 = local write "RefFreeAvg2"(w1225) -> ()
                                }
                                }
                              }
                              frame 8 {
                                n587 = local write "AuxFree"(w1226) -> ()
                              }
                              frame 9 {
                                n588 = local write "JazzFree"(w1227) -> ()
                              }
                              frame 10 {
                                n589 = local write "AnaFree"(w1228) -> ()
                              }
                            }
                          }
                          frame True {
                          }
                        }
                        n590 = Or(x=w1194, y=w1193) -> (x .or. y?=w1192:bool)
                      }
                    }
                    frame #4 {
                      w1236 = TRUE  # read raw string? (F)
                      # "Not Found"
                      n591 = Array Size(array=w1232) -> (size(s)=w1235:i32)
                      n592 = Decrement(x=w1235) -> (x-1=w1233:i32)
                      n593 = Decrement(x=w1235) -> (x-1=w1234:i32)
                      n594 = Index Array(array=w1232, index=w1234) -> (element=w1231:string)
                      n595 = for {
                        N: w1233 -> [_]
                        shift-right: [w1264] -> w1240
                        shift-left: w1252 -> [w1263]
                        shift-right: [w1265] -> w1239
                        shift-left: w1251 -> [w1262]
                        tunnel: [w1253] -> w1250 mode=indexing
                        tunnel: [w1256] -> w1249 mode=indexing
                        tunnel: w1246 -> [w1255]
                        tunnel: w1232 -> [w1254] mode=indexing
                        n596 = call-poly <vilib>:"Read Key.vi"("section"=w1255, "error in (no error)"=w1262, "key"=w1254, "refnum"=w1263) -> ("error out"=w1265:errorcluster, "value"=w1258:string, "found?"=w1257:bool, "refnum out"=w1264:T19)  [unwired: 2 in, 2 out]
                        n597 = Not(x=w1257) -> (.not. x?=w1260:bool)
                        n598 = Equal?(x="", y=w1258) -> (x = y?=w1259:bool)
                        n599 = Decimal String To Number(string=w1258) -> (number=w1253:i32)  [unwired: 3 out]
                        n600 = Or(x=w1260, y=w1259) -> (x .or. y?=w1256:bool)
                      }
                      n601 = call-poly <vilib>:"Read Key.vi"("read raw string? (F)"=w1236, "section"=w1246, "error in (no error)"=w1239, "key"=w1231, "refnum"=w1240) -> ("error out"=w1229:errorcluster, "value"=w1237:string, "found?"=w1245:bool, "refnum out"=w1230:T19)  [unwired: 1 in, 2 out]
                      n602 = Not(x=w1245) -> (.not. x?=w1244:bool)
                      n603 = Equal?(x="", y=w1237) -> (x = y?=w1247:bool)
                      n604 = String To Path(string=w1237) -> (path=w1238:path)
                      n605 = Or(x=w1244, y=w1247) -> (x .or. y?=w1241:bool)
                      n606 = Or Array Elements(Boolean array=w1249) -> (logical OR=w1242:bool)
                      n607 = Or(x=w1242, y=w1241) -> (x .or. y?=w1243:bool)
                    }
                    frame #5 {
                      # "Not Found"
                      n608 = for {
                        shift-right: [w1301] -> w1270
                        shift-left: w1274 -> [w1300]
                        shift-right: [w1302] -> w1269
                        shift-left: w1273 -> [w1299]
                        tunnel: [w1290] -> w1267 mode=indexing
                        tunnel: [w1293] -> w1268 mode=indexing
                        tunnel: w1271 -> [w1292]
                        tunnel: w1272 -> [w1291] mode=indexing
                        n609 = call-poly <vilib>:"Read Key.vi"("section"=w1292, "error in (no error)"=w1299, "key"=w1291, "refnum"=w1300) -> ("error out"=w1302:errorcluster, "value"=w1295:string, "found?"=w1294:bool, "refnum out"=w1301:T19)  [unwired: 2 in, 2 out]
                        n610 = Not(x=w1294) -> (.not. x?=w1297:bool)
                        n611 = Equal?(x="", y=w1295) -> (x = y?=w1296:bool)
                        n612 = Decimal String To Number(string=w1295) -> (number=w1290:i32)  [unwired: 3 out]
                        n613 = Or(x=w1297, y=w1296) -> (x .or. y?=w1293:bool)
                      }
                      n614 = Or Array Elements(Boolean array=w1268) -> (logical OR=w1266:bool)
                      n615 = case shown="False" w1266 {
                        tunnel: w1267 -> [w1289 _]
                        frame False {
                          n616 = Index Array(array=w1289) -> (element #1=w1288:i32, element #2=w1287:i32, element #3=w1286:i32, element #4=w1285:i32, element #5=w1276:i32, element #6=w1277:i32, element #7=w1278:i32)  [unwired: 7 in]
                          n617 = Not Equal To 0?(x=w1286) -> (x != 0?=w1282:bool)
                          n618 = Not Equal To 0?(x=w1276) -> (x != 0?=w1275:bool)
                          n619 = Not Equal To 0?(x=w1278) -> (x != 0?=w1279:bool)
                          n620 = To Byte Integer(number=w1287) -> (8bit integer=w1281:i8)
                          n621 = Not Equal To 0?(x=w1285) -> (x != 0?=w1283:bool)
                          n622 = Not Equal To 0?(x=w1277) -> (x != 0?=w1284:bool)
                          n623 = To Unsigned Word Integer(number=w1288) -> (unsigned 16bit integer=w1280:u16)
                          n624 = local write "LocalPort"(w1280) -> ()
                          n625 = local write "TCPaddTP"(w1282) -> ()
                          n626 = local write "TCPaddAnas"(w1284) -> ()
                          n627 = local write "TCPaddTrig"(w1279) -> ()
                          n628 = local write "TCPsubset"(w1281) -> ()
                          n629 = local write "TCPaddSens"(w1283) -> ()
                          n630 = local write "TCPaddJazz"(w1275) -> ()
                        }
                        frame True {
                        }
                      }
                    }
                  }
                  n631 = Compound Arithmetic op=OR(w715, w716, w714, w728, w738, w718) -> (w727:bool)
                  n632 = Build Array(w727) -> (w708:bool[])
                  n633 = call "Act_Error_7000.vi"("Error Code In"=w708, "error in (no error)"=w741) -> ("[user-defined descriptions]"=w739:string[], "[user-defined codes]"=w740:i32[], "error out"=w742:errorcluster)
                  n634 = call <vilib>:"Close Config Data.vi"("error in (no error)"=w742, "write file if changed (T)"=FALSE ("write configuration file? (T)"), "refnum"=w746) -> ("error out"=w748:errorcluster)  [unwired: 8 out]
                  n635 = call <vilib>:"General Error Handler.vi"("[user-defined codes]"=w740, "[user-defined descriptions]"=w739, "error in (no error)"=w748) -> ()  [unwired: 2 in, 11 out]
                }
                frame True {
                }
              }
            }
            frame 2 {
              w1309 = FALSE
              n636 = File Dialog(4:w1316, 6:w1317, 7:"Enter filename:" ("prompt"), 9:w1317, 11:w1313) -> (0:w1318:errorcluster, 1:w1337:bool, 3:w1338:path)  [unwired: 1 in, 2 out]
              n637 = case shown="False" w1337 {
                tunnel: w1338 -> [w1387 _]
                tunnel: w1336 -> [w1526 _]
                tunnel: w1335 -> [w1419 _]
                tunnel: w1334 -> [w1420 _]
                tunnel: w1333 -> [w1411 _]
                tunnel: w1332 -> [w1533 _]
                tunnel: w1331 -> [w1532 _]
                tunnel: w1330 -> [w1531 _]
                tunnel: w1329 -> [w1490 _]
                tunnel: w1328 -> [w1487 _]
                tunnel: w1327 -> [w1530 _]
                tunnel: w1326 -> [w1441 _]
                tunnel: w1325 -> [w1506 _]
                tunnel: w1324 -> [w1508 _]
                tunnel: w1323 -> [w1507 _]
                tunnel: w1322 -> [w1501 _]
                tunnel: w1321 -> [w1444 _]
                tunnel: w1320 -> [w1493 _]
                tunnel: w1319 -> [w1445 _]
                tunnel: w1318 -> [w1390 _]
                tunnel: w1315 -> [w1416 _]
                tunnel: w1314 -> [w1417 _]
                tunnel: w1312 -> [w1341 w1673]
                tunnel: [w1341 w1673] -> w1311
                frame False {
                  w1499 = TRUE  # write raw string? (F)
                  w1504 = i8 1  # New CFG has warning
                  w1534 = TRUE  # write configuration file?
                  n638 = call <vilib>:"Open Config Data.vi"("error in (no error)"=w1390, "configuration file path"=w1387) -> ("error out"=w1388:errorcluster, "refnum"=w1389:T19)  [unwired: 7 in, 1 out]
                  n639 = Replace Array Subset(array=w1506, new element=w1504) -> (w1505:i32[])  [unwired: 1 in]
                  n640 = Add(x=w1411, y=w1533) -> (x+y=w1412:i32)
                  n641 = Unbundle By Name(w1531) -> ("All Labels"=w1423:string[])
                  n642 = Add(x=w1412, y=w1532) -> (x+y=w1413:i32)
                  n643 = for {
                    shift-right: [w1651] -> w1422
                    shift-left: w1389 -> [w1654]
                    shift-right: [w1652] -> w1424
                    shift-left: w1388 -> [w1653]
                    tunnel: w1508 -> [w1650]
                    tunnel: w1505 -> [w1649] mode=indexing
                    tunnel: w1507 -> [w1647] mode=indexing
                    n644 = Number To Decimal String(number=w1649) -> (decimal integer string=w1648:string)  [unwired: 1 out]
                    n645 = call-poly <vilib>:"Write Key.vi"("section"=w1650, "error in (no error)"=w1653, "value"=w1648, "key"=w1647, "refnum"=w1654) -> ("error out"=w1652:errorcluster, "refnum out"=w1651:T19)  [unwired: 1 in, 4 out]
                  }
                  n646 = Add(x=w1413, y=w1417) -> (x+y=w1414:i32)
                  n647 = Add(x=w1414, y=w1416) -> (x+y=w1415:i32)
                  n648 = Increment(x=w1415) -> (x+1=w1421:i32)
                  n649 = for {
                    N: w1421 -> [w1573]
                    shift-right: [w1560] -> w1418
                    shift-left: w1422 -> [w1562]
                    shift-right: [w1559] -> w1425
                    shift-left: w1424 -> [w1563]
                    tunnel: w1411 -> [w1574]
                    tunnel: w1412 -> [w1580]
                    tunnel: w1420 -> [w1561]
                    tunnel: w1413 -> [w1575]
                    tunnel: w1414 -> [w1565]
                    tunnel: w1423 -> [w1558] mode=indexing
                    i -> [w1567]
                    n650 = Increment(x=w1567) -> (x+1=w1572:i32)
                    n651 = Greater Or Equal?(x=w1567, y=w1580) -> (x >= y?=w1585:bool)
                    n652 = Greater Or Equal?(x=w1567, y=w1574) -> (x >= y?=w1587:bool)
                    n653 = Greater Or Equal?(x=w1567, y=w1575) -> (x >= y?=w1576:bool)
                    n654 = Greater Or Equal?(x=w1567, y=w1565) -> (x >= y?=w1566:bool)
                    n655 = Select(t=i8 1, s=w1587, f=i8 0) -> (s? t:f=w1586:i8)
                    n656 = Equal?(x=w1573, y=w1572) -> (x = y?=w1568:bool)
                    n657 = Select(t=i8 2, s=w1585, f=w1586) -> (s? t:f=w1579:i8)
                    n658 = Select(t=i8 3, s=w1576, f=w1579) -> (s? t:f=w1578:i8)
                    n659 = Select(t=i8 4, s=w1566, f=w1578) -> (s? t:f=w1570:i8)
                    n660 = Select(t=i8 5, s=w1568, f=w1570) -> (s? t:f=w1571:i8)
                    n661 = case shown="5" w1571 {
                      tunnel: [w1591 w1597 w1603 w1609 w1615 "Trig" ("string")] -> w1564
                      tunnel: w1572 -> [w1588 w1595 w1602 w1606 w1612 _]
                      tunnel: w1574 -> [_ w1594 _ _ _ _]
                      tunnel: w1580 -> [_ _ w1600 _ _ _]
                      tunnel: w1575 -> [_ _ _ w1604 _ _]
                      tunnel: w1565 -> [_ _ _ _ w1610 _]
                      frame 0, Default {
                        n662 = Number To Decimal String(number=w1588) -> (decimal integer string=w1589:string)  [unwired: 1 out]
                        n663 = Concatenate Strings("Chan" ("string"), w1589) -> (w1591:string)
                      }
                      frame 1 {
                        n664 = Subtract(x=w1595, y=w1594) -> (x-y=w1592:i32)
                        n665 = Number To Decimal String(number=w1592) -> (decimal integer string=w1593:string)  [unwired: 1 out]
                        n666 = Concatenate Strings("Tou" ("string"), w1593) -> (w1597:string)
                      }
                      frame 2 {
                        n667 = Subtract(x=w1602, y=w1600) -> (x-y=w1598:i32)
                        n668 = Number To Decimal String(number=w1598) -> (decimal integer string=w1599:string)  [unwired: 1 out]
                        n669 = Concatenate Strings("Aux" ("string"), w1599) -> (w1603:string)
                      }
                      frame 3 {
                        n670 = Subtract(x=w1606, y=w1604) -> (x-y=w1605:i32)
                        n671 = Number To Decimal String(number=w1605) -> (decimal integer string=w1607:string)  [unwired: 1 out]
                        n672 = Concatenate Strings("Jazz" ("string"), w1607) -> (w1609:string)
                      }
                      frame 4 {
                        n673 = Subtract(x=w1612, y=w1610) -> (x-y=w1611:i32)
                        n674 = Number To Decimal String(number=w1611) -> (decimal integer string=w1613:string)  [unwired: 1 out]
                        n675 = Concatenate Strings("Box" ("string"), w1613) -> (w1615:string)
                      }
                      frame 5 {
                      }
                    }
                    n676 = call-poly <vilib>:"Write Key.vi"("section"=w1561, "error in (no error)"=w1563, "value"=w1558, "key"=w1564, "refnum"=w1562) -> ("error out"=w1559:errorcluster, "refnum out"=w1560:T19)  [unwired: 2 in, 3 out]
                  }
                  n677 = local read "AbrOffsetScale"() -> (w1359:i8)
                  n678 = local read "AvgAutoscale"() -> (w1482:bool)
                  n679 = local read "AvgAbsReject"() -> (w1480:dbl)
                  n680 = local read "ScreenLength"() -> (w1383:i32)
                  n681 = local read "RecTimeLimit"() -> (w1379:i32)
                  n682 = local read "AvgRelReject"() -> (w1481:dbl)
                  n683 = local read "AbrChannels"() -> (w1357:i8)
                  n684 = local read "MonHPfreq"() -> (w1551:dbl)
                  n685 = local read "Decimation"() -> (w1536:i8)
                  n686 = local read "AvgTrigLog"() -> (w1486:i8)
                  n687 = local read "FileAppend"() -> (w1495:bool)
                  n688 = local read "MonLPfreq"() -> (w1554:dbl)
                  n689 = local read "OffsetScale"() -> (w1525:i8)
                  n690 = local read "AvgLPfreq"() -> (w1474:dbl)
                  n691 = local read "AvgHPfreq"() -> (w1462:dbl)
                  n692 = local read "AnaHPfreq"() -> (w1512:dbl)
                  n693 = local read "TempScale"() -> (w1523:i8)
                  n694 = Unbundle By Name(w1341) -> ("AbrLP"=w1345:bool, "AbrLPfreq"=w1344:dbl, "AbrHP"=w1343:bool, "AbrHPfreq"=w1342:dbl)
                  n695 = local read "AvgSweep"() -> (w1485:i32)
                  n696 = local read "AnaLPfreq"() -> (w1519:dbl)
                  n697 = local read "BipHPfreq"() -> (w1542:dbl)
                  n698 = local read "AnaOffset"() -> (w1408:i32)
                  n699 = local read "MonScale"() -> (w1376:i8)
                  n700 = local read "Reference"() -> (w1547:i8)
                  n701 = local read "RespScale"() -> (w1509:i8)
                  n702 = local read "BipLPfreq"() -> (w1541:dbl)
                  n703 = local read "ErgoScale"() -> (w1510:i8)
                  n704 = local read "Channels"() -> (w1548:i8)
                  n705 = local read "AuxReset"() -> (w1522:bool)
                  n706 = local read "AnaReset"() -> (w1497:bool)
                  n707 = local read "TrigCode"() -> (w1511:i8)
                  n708 = local read "AvgScale"() -> (w1479:dbl)
                  n709 = local read "JazzReset"() -> (w1397:bool)
                  n710 = local read "AnaScale"() -> (w1520:i8)
                  n711 = local read "PletScale"() -> (w1524:i8)
                  n712 = local read "AbrScale"() -> (w1355:i8)
                  n713 = local read "FileLimit"() -> (w1494:i64)
                  n714 = local read "BipScale"() -> (w1546:i8)
                  n715 = local read "GsrScale"() -> (w1426:i8)
                  n716 = local read "MonHP"() -> (w1552:bool)
                  n717 = local read "MonLP"() -> (w1556:bool)
                  n718 = local read "AvgHP"() -> (w1483:bool)
                  n719 = local read "ErgoLP"() -> (w1434:bool)
                  n720 = local read "AnaHP"() -> (w1516:bool)
                  n721 = local read "JazzOn"() -> (w1399:bool)
                  n722 = local read "AddTP"() -> (w1391:bool)
                  n723 = local read "AbrOn"() -> (w1385:bool)
                  n724 = local read "AvgLP"() -> (w1484:bool)
                  n725 = local read "AnaLP"() -> (w1517:bool)
                  n726 = local read "BipHP"() -> (w1539:bool)
                  n727 = local read "Buffer"() -> (w1535:i8)
                  n728 = local read "Offset"() -> (w1537:i8)
                  n729 = local read "BipLP"() -> (w1544:bool)
                  n730 = Boolean To (0,1)(Boolean=w1391) -> (0, 1=w1392:i16)
                  n731 = Boolean To (0,1)(Boolean=w1495) -> (0, 1=w1496:i16)
                  n732 = Boolean To (0,1)(Boolean=w1544) -> (0, 1=w1545:i16)
                  n733 = Boolean To (0,1)(Boolean=w1556) -> (0, 1=w1555:i16)
                  n734 = Boolean To (0,1)(Boolean=w1539) -> (0, 1=w1540:i16)
                  n735 = Boolean To (0,1)(Boolean=w1345) -> (0, 1=w1353:i16)
                  n736 = Boolean To (0,1)(Boolean=w1343) -> (0, 1=w1351:i16)
                  n737 = Boolean To (0,1)(Boolean=w1522) -> (0, 1=w1521:i16)
                  n738 = To Long Integer(number=w1494) -> (32bit integer=w1381:i32)
                  n739 = To Long Integer(number=w1546) -> (32bit integer=w1366:i32)
                  n740 = Boolean To (0,1)(Boolean=w1434) -> (0, 1=w1435:i16)
                  n741 = To Long Integer(number=w1541) -> (32bit integer=w1364:i32)
                  n742 = Boolean To (0,1)(Boolean=w1385) -> (0, 1=w1386:i16)
                  n743 = To Long Integer(number=w1536) -> (32bit integer=w1378:i32)
                  n744 = To Long Integer(number=w1535) -> (32bit integer=w1377:i32)
                  n745 = Boolean To (0,1)(Boolean=w1552) -> (0, 1=w1553:i16)
                  n746 = Boolean To (0,1)(Boolean=w1399) -> (0, 1=w1400:i16)
                  n747 = To Long Integer(number=w1376) -> (32bit integer=w1375:i32)
                  n748 = To Long Integer(number=w1344) -> (32bit integer=w1347:i32)
                  n749 = Boolean To (0,1)(Boolean=w1397) -> (0, 1=w1401:i16)
                  n750 = To Long Integer(number=w1520) -> (32bit integer=w1402:i32)
                  n751 = To Long Integer(number=w1554) -> (32bit integer=w1373:i32)
                  n752 = Multiply(x=w1551, y=100.0) -> (x*y=w1549:dbl)
                  n753 = To Long Integer(number=w1547) -> (32bit integer=w1368:i32)
                  n754 = Multiply(x=w1542, y=100.0) -> (x*y=w1543:dbl)
                  n755 = To Long Integer(number=w1479) -> (32bit integer=w1470:i32)
                  n756 = Boolean To (0,1)(Boolean=w1517) -> (0, 1=w1518:i16)
                  n757 = To Long Integer(number=w1481) -> (32bit integer=w1468:i32)
                  n758 = To Long Integer(number=w1426) -> (32bit integer=w1467:i32)
                  n759 = Boolean To (0,1)(Boolean=w1516) -> (0, 1=w1515:i16)
                  n760 = To Long Integer(number=w1355) -> (32bit integer=w1354:i32)
                  n761 = Multiply(x=w1342, y=100.0) -> (x*y=w1352:dbl)
                  n762 = To Long Integer(number=w1480) -> (32bit integer=w1469:i32)
                  n763 = To Long Integer(number=w1486) -> (32bit integer=w1478:i32)
                  n764 = To Long Integer(number=w1485) -> (32bit integer=w1477:i32)
                  n765 = Boolean To (0,1)(Boolean=w1483) -> (0, 1=w1473:i16)
                  n766 = To Long Integer(number=w1496) -> (32bit integer=w1380:i32)
                  n767 = To Long Integer(number=w1392) -> (32bit integer=w1369:i32)
                  n768 = To Long Integer(number=w1540) -> (32bit integer=w1363:i32)
                  n769 = To Long Integer(number=w1474) -> (32bit integer=w1475:i32)
                  n770 = To Long Integer(number=w1555) -> (32bit integer=w1374:i32)
                  n771 = To Long Integer(number=w1525) -> (32bit integer=w1360:i32)
                  n772 = Multiply(x=w1462, y=100.0) -> (x*y=w1461:dbl)
                  n773 = To Long Integer(number=w1359) -> (32bit integer=w1358:i32)
                  n774 = Boolean To (0,1)(Boolean=w1484) -> (0, 1=w1476:i16)
                  n775 = To Long Integer(number=w1545) -> (32bit integer=w1365:i32)
                  n776 = To Long Integer(number=w1351) -> (32bit integer=w1348:i32)
                  n777 = To Long Integer(number=w1353) -> (32bit integer=w1346:i32)
                  n778 = To Long Integer(number=w1537) -> (32bit integer=w1361:i32)
                  n779 = To Long Integer(number=w1548) -> (32bit integer=w1370:i32)
                  n780 = To Long Integer(number=w1357) -> (32bit integer=w1356:i32)
                  n781 = Multiply(x=w1512, y=100.0) -> (x*y=w1514:dbl)
                  n782 = To Long Integer(number=w1386) -> (32bit integer=w1384:i32)
                  n783 = To Long Integer(number=w1549) -> (32bit integer=w1371:i32)
                  n784 = To Long Integer(number=w1511) -> (32bit integer=w1367:i32)
                  n785 = Boolean To (0,1)(Boolean=w1482) -> (0, 1=w1471:i16)
                  n786 = To Long Integer(number=w1435) -> (32bit integer=w1433:i32)
                  n787 = To Long Integer(number=w1553) -> (32bit integer=w1372:i32)
                  n788 = To Long Integer(number=w1510) -> (32bit integer=w1466:i32)
                  n789 = To Long Integer(number=w1509) -> (32bit integer=w1432:i32)
                  n790 = To Long Integer(number=w1400) -> (32bit integer=w1398:i32)
                  n791 = To Long Integer(number=w1473) -> (32bit integer=w1464:i32)
                  n792 = To Long Integer(number=w1524) -> (32bit integer=w1431:i32)
                  n793 = To Long Integer(number=w1401) -> (32bit integer=w1396:i32)
                  n794 = To Long Integer(number=w1543) -> (32bit integer=w1362:i32)
                  n795 = To Long Integer(number=w1523) -> (32bit integer=w1430:i32)
                  n796 = To Long Integer(number=w1476) -> (32bit integer=w1465:i32)
                  n797 = To Long Integer(number=w1515) -> (32bit integer=w1405:i32)
                  n798 = To Long Integer(number=w1352) -> (32bit integer=w1349:i32)
                  n799 = To Long Integer(number=w1521) -> (32bit integer=w1429:i32)
                  n800 = To Long Integer(number=w1519) -> (32bit integer=w1404:i32)
                  n801 = To Long Integer(number=w1518) -> (32bit integer=w1403:i32)
                  n802 = Boolean To (0,1)(Boolean=w1497) -> (0, 1=w1498:i16)
                  n803 = To Long Integer(number=w1514) -> (32bit integer=w1406:i32)
                  n804 = To Long Integer(number=w1471) -> (32bit integer=w1463:i32)
                  n805 = To Long Integer(number=w1461) -> (32bit integer=w1472:i32)
                  n806 = To Long Integer(number=w1498) -> (32bit integer=w1407:i32)
                  n807 = Build Array(w1383, w1381, w1380, w1379, w1378, w1377, w1375, w1374, w1373, w1372, w1371, w1370, w1369, w1368, w1367, w1366, w1365, w1364, w1363, w1362, w1361, w1360, w1384, w1354, w1346, w1347, w1348, w1349, w1356, w1358, w1478, w1477, w1465, w1475, w1464, w1472, w1463, w1470, w1469, w1468, w1467, w1466, w1433, w1432, w1431, w1430, w1429, w1398, w1396, w1402, w1403, w1404, w1405, w1406, w1407, w1408) -> (w1382:i32[])
                  n808 = for {
                    shift-right: [w1669] -> w1491
                    shift-left: w1425 -> [w1671]
                    shift-right: [w1670] -> w1492
                    shift-left: w1418 -> [w1672]
                    tunnel: w1526 -> [w1668] mode=indexing
                    tunnel: w1419 -> [w1667]
                    tunnel: w1382 -> [w1665] mode=indexing
                    n809 = Number To Decimal String(number=w1665) -> (decimal integer string=w1666:string)  [unwired: 1 out]
                    n810 = call-poly <vilib>:"Write Key.vi"("section"=w1667, "error in (no error)"=w1671, "value"=w1666, "key"=w1668, "refnum"=w1672) -> ("error out"=w1669:errorcluster, "refnum out"=w1670:T19)  [unwired: 1 in, 4 out]
                  }
                  n811 = Array Size(array=w1441) -> (size(s)=w1447:i32)
                  n812 = Decrement(x=w1447) -> (x-1=w1443:i32)
                  n813 = for {
                    tunnel: w1493 -> [w1628] mode=indexing
                    shift-right: [w1631] -> w1488
                    shift-left: w1491 -> [w1632]
                    shift-right: [w1630] -> w1489
                    shift-left: w1492 -> [w1633]
                    tunnel: w1490 -> [w1629]
                    i -> [w1627]
                    n814 = case shown="8" w1627 {
                      tunnel: [w1634 w1635 w1636 w1637 w1638 w1640 w1641 w1643 w1644 w1645 w1646] -> w1626
                      frame 0, Default {
                        n815 = local read "MonFree"() -> (w1634:i32[])
                      }
                      frame 1 {
                        n816 = local read "RefFree"() -> (w1635:i32[])
                      }
                      frame 2 {
                        n817 = local read "BipFree"() -> (w1636:i32[])
                      }
                      frame 3 {
                        n818 = local read "AvgTrigSel"() -> (w1637:i32[])
                      }
                      frame 4 {
                        n819 = local read "MonFreeAvg1"() -> (w1639:i32)
                        n820 = Build Array(w1639) -> (w1638:i32[])
                      }
                      frame 5 {
                        n821 = local read "RefFreeAvg1"() -> (w1640:i32[])
                      }
                      frame 6 {
                        n822 = local read "MonFreeAvg2"() -> (w1642:i32)
                        n823 = Build Array(w1642) -> (w1641:i32[])
                      }
                      frame 7 {
                        n824 = local read "RefFreeAvg2"() -> (w1643:i32[])
                      }
                      frame 8 {
                        n825 = local read "AuxFree"() -> (w1644:i32[])
                      }
                      frame 9 {
                        n826 = local read "JazzFree"() -> (w1645:i32[])
                      }
                      frame 10 {
                        n827 = local read "AnaFree"() -> (w1646:i32[])
                      }
                    }
                    n828 = call "ArrayToCFG.vi"("Selector Array"=w1626) -> ("Cofiguration String"=w1625:string)
                    n829 = call-poly <vilib>:"Write Key.vi"("section"=w1629, "error in (no error)"=w1632, "value"=w1625, "key"=w1628, "refnum"=w1633) -> ("error out"=w1631:errorcluster, "refnum out"=w1630:T19)  [unwired: 1 in, 4 out]
                  }
                  n830 = for {
                    N: w1443 -> [_]
                    shift-right: [w1661] -> w1503
                    shift-left: w1489 -> [w1664]
                    shift-right: [w1662] -> w1502
                    shift-left: w1488 -> [w1663]
                    tunnel: w1487 -> [w1660]
                    tunnel: w1530 -> [w1659] mode=indexing
                    tunnel: w1441 -> [w1657] mode=indexing
                    n831 = Number To Decimal String(number=w1659) -> (decimal integer string=w1658:string)  [unwired: 1 out]
                    n832 = call-poly <vilib>:"Write Key.vi"("section"=w1660, "error in (no error)"=w1663, "value"=w1658, "key"=w1657, "refnum"=w1664) -> ("error out"=w1662:errorcluster, "refnum out"=w1661:T19)  [unwired: 1 in, 4 out]
                  }
                  n833 = local read "TCPaddAnas"() -> (w1440:bool)
                  n834 = Decrement(x=w1447) -> (x-1=w1446:i32)
                  n835 = local read "TCPaddSens"() -> (w1439:bool)
                  n836 = local read "TCPaddJazz"() -> (w1394:bool)
                  n837 = local read "TCPaddTrig"() -> (w1427:bool)
                  n838 = local read "TCPsubset"() -> (w1437:i8)
                  n839 = local read "TCPaddTP"() -> (w1438:bool)
                  n840 = local read "LocalPort"() -> (w1436:u16)
                  n841 = Path To String(path=w1501) -> (string=w1500:string)
                  n842 = Index Array(array=w1441, index=w1446) -> (element=w1442:string)
                  n843 = Boolean To (0,1)(Boolean=w1439) -> (0, 1=w1455:i16)
                  n844 = Boolean To (0,1)(Boolean=w1438) -> (0, 1=w1456:i16)
                  n845 = Boolean To (0,1)(Boolean=w1394) -> (0, 1=w1395:i16)
                  n846 = Boolean To (0,1)(Boolean=w1440) -> (0, 1=w1454:i16)
                  n847 = Boolean To (0,1)(Boolean=w1427) -> (0, 1=w1428:i16)
                  n848 = To Long Integer(number=w1437) -> (32bit integer=w1457:i32)
                  n849 = To Long Integer(number=w1436) -> (32bit integer=w1458:i32)
                  n850 = To Long Integer(number=w1456) -> (32bit integer=w1453:i32)
                  n851 = To Long Integer(number=w1455) -> (32bit integer=w1452:i32)
                  n852 = To Long Integer(number=w1395) -> (32bit integer=w1393:i32)
                  n853 = To Long Integer(number=w1454) -> (32bit integer=w1409:i32)
                  n854 = To Long Integer(number=w1428) -> (32bit integer=w1410:i32)
                  n855 = call-poly <vilib>:"Write Key.vi"("write raw string? (F)"=w1499, "section"=w1487, "error in (no error)"=w1502, "value"=w1500, "key"=w1442, "refnum"=w1503) -> ("error out"=w1450:errorcluster, "refnum out"=w1451:T19)  [unwired: 4 out]
                  n856 = Build Array(w1458, w1457, w1453, w1452, w1393, w1409, w1410) -> (w1459:i32[])
                  n857 = Wait (ms)(milliseconds to wait=u32 300) -> ()  [unwired: 1 out]
                  n858 = for {
                    shift-right: [w1621] -> w1449
                    shift-left: w1451 -> [w1624]
                    shift-right: [w1622] -> w1448
                    shift-left: w1450 -> [w1623]
                    tunnel: w1445 -> [w1620]
                    tunnel: w1459 -> [w1619] mode=indexing
                    tunnel: w1444 -> [w1617] mode=indexing
                    n859 = Number To Decimal String(number=w1619) -> (decimal integer string=w1618:string)  [unwired: 1 out]
                    n860 = call-poly <vilib>:"Write Key.vi"("section"=w1620, "error in (no error)"=w1623, "value"=w1618, "key"=w1617, "refnum"=w1624) -> ("error out"=w1622:errorcluster, "refnum out"=w1621:T19)  [unwired: 1 in, 4 out]
                  }
                  n861 = call <vilib>:"Close Config Data.vi"("error in (no error)"=w1448, "write file if changed (T)"=w1534, "refnum"=w1449) -> ("error out"=w1528:errorcluster)  [unwired: 8 out]
                  n862 = call <vilib>:"General Error Handler.vi"("error in (no error)"=w1528) -> ("error out"=w1529:errorcluster)  [unwired: 2 in, 12 out]
                  n863 = Unbundle By Name(w1529) -> ("status"=w1527:bool)
                  n864 = case shown="False" w1527 {
                    tunnel: w1387 -> [w1655 _]
                    frame False {
                      n865 = Path To String(path=w1655) -> (string=w1656:string)
                      n866 = local write "CFG Filepath"(w1656) -> ()
                    }
                    frame True {
                    }
                  }
                  "Write CFG" <- w1534
                }
                frame True {
                }
              }
            }
          }
          n867 = Compound Arithmetic op=OR(w359, w360, w361) -> (w495:bool)
        }
        n868 = Index Array(array=w310) -> (element #1=w315:i32, element #2=w287:i32, element #3=w314:i32, element #4=w312:i32, element #5=w300:i32, element #6=w299:i32, element #7=w285:i32, element #8=w284:i32, element #9=w273:i32, element #10=w267:i32, element #11=w248:i32, element #12=w247:i32, element #13=w244:i32, element #14=w243:i32)  [unwired: 14 in]
        n869 = Index Array(array=w311) -> (element #1=w330:i32, element #2=w342:i32, element #3=w341:i32, element #4=w327:i32, element #5=w290:i32, element #6=w238:i32, element #7=w298:i32)  [unwired: 7 in]
        n870 = To Byte Integer(number=w315) -> (8bit integer=w256:i8)
        n871 = To Byte Integer(number=w287) -> (8bit integer=w255:i8)
        n872 = To Byte Integer(number=w314) -> (8bit integer=w254:i8)
        n873 = To Byte Integer(number=w312) -> (8bit integer=w253:i8)
        n874 = To Unsigned Byte Integer(number=w300) -> (unsigned 8bit integer=w302:u8)
        n875 = To Unsigned Word Integer(number=w299) -> (unsigned 16bit integer=w301:u16)
        n876 = To Byte Integer(number=w285) -> (8bit integer=w252:i8)
        n877 = To Byte Integer(number=w284) -> (8bit integer=w251:i8)
        n878 = To Byte Integer(number=w273) -> (8bit integer=w250:i8)
        n879 = To Byte Integer(number=w267) -> (8bit integer=w249:i8)
        n880 = To Byte Integer(number=w244) -> (8bit integer=w242:i8)
        n881 = To Byte Integer(number=w243) -> (8bit integer=w241:i8)
        n882 = Not Equal To 0?(x=w290) -> (x != 0?=w289:bool)
        n883 = Bundle By Name(cluster=w318, "Warning"=w256, "Motherboard"=w255, "ElecGain"=w254, "RespSwitch"=w253, "LineWidth"=w302, "Cursor"=w301, "PopupKiller"=w252, "BreathBelt"=w251, "ABRlocation"=w250, "SEMGswap"=w249, "TrigLength"=w248, "TrigLevel"=w247, "TrigWindow"=w242, "TrigPol"=w241) -> (w317:T9)
        n884 = Not Equal To 0?(x=w327) -> (x != 0?=w326:bool)
        n885 = To Byte Integer(number=w330) -> (8bit integer=w316:i8)
        n886 = Not Equal To 0?(x=w341) -> (x != 0?=w340:bool)
        n887 = Not Equal To 0?(x=w342) -> (x != 0?=w339:bool)
        n888 = Bundle By Name(cluster=w297, "Save Subset"=w316, "Add Touchproofs"=w339, "Add Sensors"=w340, "Add Jazz"=w326, "Add Anas"=w289, "PauseOff"=w238, "PauseOn"=w298, "Save Path"=w237) -> (w343:T8)
      }
      frame 1 {
        w1677 = 10  # Mastoids
        w1679 = 9  # Ref (ABR)
        w1727 = i8 7 items=["A1 - H32 (256)", "A1 - E32 (160)", "A1 - D32 (128)", "A1 - B32 (64)", "A1 - A32 (32)", "A1 - A16 (16)", "A1 -A8 (8)", "None (0) "] ("TCPsubset")
        w1734 = i8 13  # SimuABR
        w1756 = i8 9  # ABR
        w1818 = 0.2035  # 5th order sinc
        w1790 = i8 0 items=["All 256 Chan ", "A + B", "C + D", "E + F", "G + H"] ("Offset")
        w1933 = i8 0 items=["None (raw)", "Avg of 256", "Avg 1-224", "Avg 1-160", "Avg 1-128", "Avg 1-64", "Avg 1-32", "Avg of Displ", "Free Choice"] ("Reference")
        w1810 = 0 ("f")
        w1813 = 4  # Jazz Chan
        w1949 = FALSE  # Config Changed
        w1959 = FALSE  # Stop Running
        w1964 = 2  # Go to State 2 Initialize
        # "Jazz ?"
        # "Multibox?"
        # "Anabox?"
        # "Config Changed"
        # "Sensors?"
        n889 = flat-sequence {
          tunnel: w1776 -> [w2469]
          tunnel: [w2469] -> w1775
          tunnel: [w2488] -> w1909
          tunnel: [w2487] -> w1868
          tunnel: [w2486] -> w1867
          tunnel: [w2485] -> w1866
          tunnel: [w2483] -> w1833
          tunnel: [w2482] -> w1832
          tunnel: [w2481] -> w1817
          tunnel: "JazzOn" -> [w2477]
          tunnel: w1775 -> [w2473]
          tunnel: [w2472] -> w1675
          tunnel: [w2471] -> w1674
          tunnel: w1909 -> [w2537]
          tunnel: [w2536] -> w1706
          tunnel: w1868 -> [w2536]
          tunnel: w1867 -> [w2543]
          tunnel: w1866 -> [w2542]
          tunnel: [w2542] -> w1778
          tunnel: w1833 -> [w2541]
          tunnel: [w2541] -> w1785
          tunnel: w1832 -> [w2540]
          tunnel: w1817 -> [w2539]
          tunnel: [w2539] -> w1781
          tunnel: w1675 -> [w2534]
          tunnel: w1674 -> [w2533]
          frame #0 {
            n890 = global write "StopJazzIni.glb" "JazzIniStop"(FALSE) -> ()
          }
          frame #1 {
            w2479 = i64 1900544  # Max Samples in 2 sec
            w2484 = i64 0  # Integer 64
            n891 = call "Act_Open.vi"("Buffer Size in Byte"=w2473, "JazzOn"=w2477) -> ("Handle Out"=w2474:i64, "Buffer Size in Words"=w2475:i64, "RingBuffer"=w2476:i32[])
            n892 = Select(t=w2479, s=w2477, f=i64 256 ("Display Blocksize In")) -> (s? t:f=w2478:i64)
            n893 = while {
              tunnel: w2476 -> [w2515]
              tunnel: [w2514] -> w2487
              tunnel: w2475 -> [w2513]
              shift-right: [w2512] -> _
              shift-left: w2484 -> [w2506]
              tunnel: w2484 -> [w2511]
              tunnel: [w2497] -> w2488
              tunnel: [w2505] -> w2486
              tunnel: [w2504] -> w2485
              tunnel: [w2502] -> w2483
              tunnel: [w2501] -> w2482
              tunnel: [w2500] -> w2481
              tunnel: w2478 -> [w2499]
              tunnel: w2474 -> [w2496]
              i -> [w2508]
              stop <- w2498 stop-if-true
              n894 = Equal To 0?(x=w2508) -> (x = 0?=w2507:bool)
              n895 = call "Act_Pointer.vi"("First Iteration"=w2507, "Handle In"=w2496, "Display Blocksize In"=w2499, "Buffer Size"=w2513, "Old Total Displayed"=w2511, "Old Total Buffered"=w2506) -> ("Data Ready"=w2509:bool, "No Incoming Data"=w2503:bool, "New Total Buffered"=w2512:i64, "Handle Out"=w2497:i64)  [unwired: 1 out]
              n896 = case shown="True" w2509 {
                tunnel: w2515 -> [_ w2528]
                tunnel: [i8 -1 ("t") w2527] -> w2514
                tunnel: [FALSE TRUE] -> w2510
                tunnel: [w2517 w2529] -> w2505
                tunnel: [w2516 w2521] -> w2504
                tunnel: [w2516 w2524] -> w2502
                tunnel: [w2517 w2523] -> w2501
                tunnel: [w2516 w2522] -> w2500
                frame False {
                  w2516 = TRUE
                  w2517 = "?" ("f")
                  n897 = Wait (ms)(milliseconds to wait=u32 10) -> ()  [unwired: 1 out]
                }
                frame True {
                  n898 = call "Act_Mode.vi"("Serial Data"=w2528) -> ("SpeedMode"=w2527:i8, "Mk2 ?"=w2521:bool, "GSR16Hz ?"=w2524:bool, "Jazz ?"=w2522:bool)
                  n899 = property on="Battery" class="Slide (strict)"("Visible"=w2521) -> ()  [unwired: 2 in, 2 out]
                  n900 = Select(t="nanoS", s=w2524, f="Ohm") -> (s? t:f=w2523:string)
                  n901 = Select(t="Mk2", s=w2521, f="Mk1") -> (s? t:f=w2529:string)
                }
              }
              n902 = Or(x=w2503, y=w2510) -> (x .or. y?=w2498:bool)
              n903 = global write "StopJazzIni.glb" "JazzIniStop"(w2498) -> ()
            }
            n904 = case shown="True" w2477 {
              frame False {
              }
              frame True {
                n905 = while {
                  shift-left: TRUE ("NoRefWarning") -> [w2491]
                  shift-right: [w2490] -> _
                  stop <- w2490 stop-if-true
                  n906 = Wait (ms)(milliseconds to wait=u32 10) -> ()  [unwired: 1 out]
                  n907 = case shown="True" w2491 {
                    tunnel: [w2493 w2495] -> w2490
                    frame False {
                      n908 = global read "StopJazzIni.glb" "JazzIniStop"() -> (w2493:bool)
                    }
                    frame True {
                      n909 = call "JazzIni.vi"() -> ("Ready"=w2494:bool)  [unwired: 1 out]
                      n910 = Not(x=w2494) -> (.not. x?=w2495:bool)
                    }
                  }
                }
              }
            }
            n911 = call "Act_Info.vi"() -> ("FPGA firmware"=w2471:string, "USB chip"=w2472:string)  [unwired: 1 out]
          }
          frame #2 {
            # "JazzRec ?"
            # "GSR16Hz ?"
            # "Version Mk?"
            n912 = Number To Decimal String(number=w2536) -> (decimal integer string=→"Speed Mode":string)  [unwired: 1 in]
            n913 = global write "StopJazzIni.glb" "JazzIniStop"(FALSE) -> ()
            n914 = call "Act_Close.vi"("Handle In"=w2537) -> ()
            "AD-box" <- w2543
            "Unit" <- w2540
            "USB-receiver model" <- w2534
            "USB-receiver firmware" <- w2533
          }
        }
        n915 = Unbundle By Name(w1698) -> ("ABRlocation"=w1695:i8)
        n916 = Equal To 0?(x=w1695) -> (x = 0?=w1691:bool)
        n917 = local read "TCPsubset"() -> (w1879:i8)
        n918 = local read "Reference"() -> (w1919:i8)
        n919 = And(x="AbrOn", y=w1691) -> (x .and. y?=w1692:bool)
        n920 = local read "Channels"() -> (w1920:i8)
        n921 = local read "MonFree"() -> (w1917:i32[])
        n922 = local read "JazzFree"() -> (w1794:i32[])
        n923 = local read "AuxFree"() -> (w1697:i32[])
        n924 = local read "AnaFree"() -> (w1849:i32[])
        n925 = local read "RefFree"() -> (w1916:i32[])
        n926 = local read "BipFree"() -> (w1871:i32[])
        n927 = local read "Offset"() -> (w1918:i8)
        n928 = case shown="True" w1778 {
          tunnel: [w2051 w2224] -> w1878
          tunnel: [w2052 w2223] -> w1876
          tunnel: [w2050 w2222] -> w1680
          tunnel: [w2049 w2221] -> w1877
          tunnel: [w2046 w2220] -> w1815
          tunnel: [w2045 w2219] -> w1872
          tunnel: [w2047 w2218] -> w1736
          tunnel: [w2043 w2217] -> w1709
          tunnel: [w2042 w2216] -> w1707
          tunnel: [w2037 w2215] -> w1704
          tunnel: [w2044 w2214] -> w1705
          tunnel: w1706 -> [w2048 w2213]
          tunnel: [w2041 w2211] -> w1873
          tunnel: [w2040 w2212] -> w1875
          tunnel: w1780 -> [w2039 w2210]
          tunnel: [w2038 w2210] -> w1779
          tunnel: w1692 -> [_ w2209]
          frame False {
            # "Old Mk1 version"
            n929 = case shown="9" w2048 {
              tunnel: [232 ("Mon Channels") 256 ("Mon Channels") 128 ("Mon Channels") 64 ("Mon Channels") 32 ("Mon Channels") 232 ("Mon Channels") 104 ("Mon Channels") 40 ("Mon Channels") 8 ("Mon Channels") 232 ("Mon Channels") 232 ("Mon Channels")] -> w2037
              tunnel: [8 ("Bip Channels") 0 ("Bip Channels") 0 ("Bip Channels") 0 ("Bip Channels") 0 ("Bip Channels") 8 ("Bip Channels") 8 ("Bip Channels") 8 ("Bip Channels") 8 ("Bip Channels") 8 ("Bip Channels") 8 ("Bip Channels")] -> w2044
              tunnel: [8 ("Aux Channels") 0 ("Aux Channels") 0 ("Aux Channels") 0 ("Aux Channels") 0 ("Aux Channels") 8 ("Aux Channels") 8 ("Aux Channels") 8 ("Aux Channels") 8 ("Aux Channels") 8 ("Aux Channels") 8 ("Aux Channels")] -> w2043
              tunnel: [w2066 w2070 w2084 w2098 w2112 w2126 w2140 w2154 w2168 w2183 w2208] -> w2052
              tunnel: [i32[] [] ("Disabled Items []") i32[] [0, 13] ("Disabled Items []") i32[] [0, 1, 2, 9, 10, 11, 12, 13] ("Disabled Items []") i32[] [0, 1, 2, 3, 7, 8, 9, 10, 11, 12, 13] ("Disabled Items []") i32[] [0, 1, 2, 3, 4, 6, 7, 8, 9, 10, 11, 12, 13] ("Disabled Items []") i32[] [0, 1, 12] ("Disabled Items []") i32[] [0, 1, 2, 3, 8, 9, 10, 11, 12] ("Disabled Items []") i32[] [0, 1, 2, 3, 4, 6, 7, 8, 9, 10, 11, 12] ("Disabled Items []") i32[] [0, 1, 2, 3, 4, 5, 6, 7, 8, 9, 10, 11, 12] ("Disabled Items []") i32[] [0, 1, 12] ("Disabled Items []") i32[] [] ("Disabled Items []")] -> w2051
              tunnel: [i32[] [] ("Disabled Items []") i32[] [1] ("Disabled Items []") i32[] [1, 2, 3] ("Disabled Items []") i32[] [1, 2, 3, 4] ("Disabled Items []") i32[] [1, 2, 3, 4, 5] ("Disabled Items []") i32[] [1, 2] ("Disabled Items []") i32[] [1, 2, 3, 4] ("Disabled Items []") i32[] [1, 2, 3, 4, 5] ("Disabled Items []") i32[] [1, 2, 3, 4, 5, 6] ("Disabled Items []") i32[] [1] ("Disabled Items []") i32[] [] ("Disabled Items []")] -> w2050
              tunnel: [i32[] [] ("Disabled Items []") i32[] [] ("Disabled Items []") i32[] [3, 4] ("Disabled Items []") i32[] [2, 3, 4] ("Disabled Items []") i32[] [2, 3, 4] ("Disabled Items []") i32[] [] ("Disabled Items []") i32[] [3, 4] ("Disabled Items []") i32[] [2, 3, 4] ("Disabled Items []") i32[] [2, 3, 4] ("Disabled Items []") i32[] [] ("Disabled Items []") i32[] [] ("Disabled Items []")] -> w2049
              tunnel: [32 ("Aux Channels") 0 ("Aux Channels") 0 ("Aux Channels") 0 ("Aux Channels") 0 ("Aux Channels") 0 ("Aux Channels") 0 ("Aux Channels") 0 ("Aux Channels") 0 ("Aux Channels") 32 ("Aux Channels") 32 ("Aux Channels")] -> w2042
              tunnel: [0 ("ADC Rate") 2048 ("ADC Rate") 4096 ("ADC Rate") 8192 ("ADC Rate") 16384 ("ADC Rate") 2048 ("ADC Rate") 4096 ("ADC Rate") 8192 ("ADC Rate") 16384 ("ADC Rate") 2048 ("ADC Rate") 0 ("ADC Rate")] -> w2047
              tunnel: [0 ("Nr of Chan") 258 ("Nr of Chan") 130 ("Nr of Chan") 66 ("Nr of Chan") 34 ("Nr of Chan") 258 ("Nr of Chan") 130 ("Nr of Chan") 66 ("Nr of Chan") 34 ("Nr of Chan") 290 ("Nr of Chan") 0 ("Nr of Chan")] -> w2046
              tunnel: [0 ("Nr of Chan") 2 ("Nr of Chan") 4 ("Nr of Chan") 8 ("Nr of Chan") 16 ("Nr of Chan") 2 ("Nr of Chan") 4 ("Nr of Chan") 8 ("Nr of Chan") 16 ("Nr of Chan") 2 ("Nr of Chan") 0 ("Nr of Chan")] -> w2045
              tunnel: [i32[] [] ("Disabled Items []") i32[] [] ("Disabled Items []") i32[] [0, 1] ("Disabled Items []") i32[] [0, 1, 2] ("Disabled Items []") i32[] [0, 1, 2, 3] ("Disabled Items []") i32[] [0] ("Disabled Items []") i32[] [0, 1, 2] ("Disabled Items []") i32[] [0, 1, 2, 3] ("Disabled Items []") i32[] [0, 1, 2, 3, 4, 5] ("Disabled Items []") i32[] [0] ("Disabled Items []") i32[] [] ("Disabled Items []")] -> w2041
              tunnel: [w2054 w2069 w2083 w2097 w2111 w2125 w2138 w2153 w2167 w2182 w2196] -> w2040
              tunnel: w2039 -> [w2053 w2067 w2081 w2095 w2109 w2123 w2137 w2151 w2165 w2179 w2194]
              tunnel: [w2053 w2067 w2081 w2095 w2109 w2123 w2137 w2151 w2165 w2179 w2195] -> w2038
              frame -1, Default {
                w2054 = i8 0 items=["A1 - H32 (256)", "A1 - E32 (160)", "A1 - D32 (128)", "A1 - B32 (64)", "A1 - A32 (32)", "A1 - A16 (16)", "A1 -A8 (8)", "None (0) "] ("TCP subset:")
                w2066 = i8 0 items=["All 256 Chan ", "A-G (224)", "A-E (160)", "ABCD (128)", "A+B (64)", "A (32)", "B (32)", "C (32)", "D (32)", "E (32)", "F (32)", "G (32)", "H(32)", "EXG (8)", "Free Choice"] ("Channels")
              }
              frame 0 {
                w2069 = i8 0 items=["A1 - H32 (256)", "A1 - E32 (160)", "A1 - D32 (128)", "A1 - B32 (64)", "A1 - A32 (32)", "A1 - A16 (16)", "A1 -A8 (8)", "None (0) "] ("TCP subset:")
                w2070 = i8 1 items=["All 264 Chan ", "A-H (256)", "A-E (160)", "ABCD (128)", "A+B (64)", "A (32)", "B (32)", "C (32)", "D (32)", "E (32)", "F (32)", "G (32)", "H(32)", "EXG (8)", "Free Choice"] ("Channels")
              }
              frame 1 {
                w2083 = i8 2 items=["A1 - H32 (256)", "A1 - E32 (160)", "A1 - D32 (128)", "A1 - B32 (64)", "A1 - A32 (32)", "A1 - A16 (16)", "A1 -A8 (8)", "None (0) "] ("TCP subset:")
                w2084 = i8 3 items=["All 264 Chan ", "A-H (256)", "A-E (160)", "ABCD (128)", "A+B (64)", "A (32)", "B (32)", "C (32)", "D (32)", "E (32)", "F (32)", "G (32)", "H(32)", "EXG (8)", "Free Choice"] ("Channels")
              }
              frame 2 {
                w2097 = i8 3 items=["A1 - H32 (256)", "A1 - E32 (160)", "A1 - D32 (128)", "A1 - B32 (64)", "A1 - A32 (32)", "A1 - A16 (16)", "A1 -A8 (8)", "None (0) "] ("TCP subset:")
                w2098 = i8 4 items=["All 264 Chan ", "A-H (256)", "A-E (160)", "ABCD (128)", "A+B (64)", "A (32)", "B (32)", "C (32)", "D (32)", "E (32)", "F (32)", "G (32)", "H(32)", "EXG (8)", "Free Choice"] ("Channels")
              }
              frame 3 {
                w2111 = i8 4 items=["A1 - H32 (256)", "A1 - E32 (160)", "A1 - D32 (128)", "A1 - B32 (64)", "A1 - A32 (32)", "A1 - A16 (16)", "A1 -A8 (8)", "None (0) "] ("TCP subset:")
                w2112 = i8 5 items=["All 264 Chan ", "A-H (256)", "A-E (160)", "ABCD (128)", "A+B (64)", "A (32)", "B (32)", "C (32)", "D (32)", "E (32)", "F (32)", "G (32)", "H(32)", "EXG (8)", "Free Choice"] ("Channels")
              }
              frame 4 {
                w2125 = i8 1 items=["A1 - H32 (256)", "A1 - E32 (160)", "A1 - D32 (128)", "A1 - B32 (64)", "A1 - A32 (32)", "A1 - A16 (16)", "A1 -A8 (8)", "None (0) "] ("TCP subset:")
                w2126 = i8 2 items=["All 264 Chan ", "A-H (256)", "A-E (160)", "ABCD (128)", "A+B (64)", "A (32)", "B (32)", "C (32)", "D (32)", "E (32)", "F (32)", "G (32)", "H(32)", "EXG (8)", "Free Choice"] ("Channels")
              }
              frame 5 {
                w2138 = i8 3 items=["A1 - H32 (256)", "A1 - E32 (160)", "A1 - D32 (128)", "A1 - B32 (64)", "A1 - A32 (32)", "A1 - A16 (16)", "A1 -A8 (8)", "None (0) "] ("TCP subset:")
                w2140 = i8 4 items=["All 264 Chan ", "A-H (256)", "A-E (160)", "ABCD (128)", "A+B (64)", "A (32)", "B (32)", "C (32)", "D (32)", "E (32)", "F (32)", "G (32)", "H(32)", "EXG (8)", "Free Choice"] ("Channels")
              }
              frame 6 {
                w2153 = i8 4 items=["A1 - H32 (256)", "A1 - E32 (160)", "A1 - D32 (128)", "A1 - B32 (64)", "A1 - A32 (32)", "A1 - A16 (16)", "A1 -A8 (8)", "None (0) "] ("TCP subset:")
                w2154 = i8 5 items=["All 264 Chan ", "A-H (256)", "A-E (160)", "ABCD (128)", "A+B (64)", "A (32)", "B (32)", "C (32)", "D (32)", "E (32)", "F (32)", "G (32)", "H(32)", "EXG (8)", "Free Choice"] ("Channels")
              }
              frame 7 {
                w2167 = i8 6 items=["A1 - H32 (256)", "A1 - E32 (160)", "A1 - D32 (128)", "A1 - B32 (64)", "A1 - A32 (32)", "A1 - A16 (16)", "A1 -A8 (8)", "None (0) "] ("TCP subset:")
                w2168 = i8 14 items=["All 264 Chan ", "A-H (256)", "A-E (160)", "ABCD (128)", "A+B (64)", "A (32)", "B (32)", "C (32)", "D (32)", "E (32)", "F (32)", "G (32)", "H(32)", "EXG (8)", "Free Choice"] ("Channels")
              }
              frame 8 {
                w2182 = i8 1 items=["A1 - H32 (256)", "A1 - E32 (160)", "A1 - D32 (128)", "A1 - B32 (64)", "A1 - A32 (32)", "A1 - A16 (16)", "A1 -A8 (8)", "None (0) "] ("TCP subset:")
                w2183 = i8 2 items=["All 264 Chan ", "A-H (256)", "A-E (160)", "ABCD (128)", "A+B (64)", "A (32)", "B (32)", "C (32)", "D (32)", "E (32)", "F (32)", "G (32)", "H(32)", "EXG (8)", "Free Choice"] ("Channels")
              }
              frame 9 {
                w2193 = bool[] [FALSE, FALSE, TRUE]  # Error Code In
                w2196 = i8 0 items=["A1 - H32 (256)", "A1 - E32 (160)", "A1 - D32 (128)", "A1 - B32 (64)", "A1 - A32 (32)", "A1 - A16 (16)", "A1 -A8 (8)", "None (0) "] ("TCP subset:")
                w2208 = i8 0 items=["All 256 Chan ", "A-G (224)", "A-E (160)", "ABCD (128)", "A+B (64)", "A (32)", "B (32)", "C (32)", "D (32)", "E (32)", "F (32)", "G (32)", "H(32)", "EXG (8)", "Free Choice"] ("Channels")
                n930 = call "Act_Error_5000.vi"("Error Code In"=w2193, "error in (no error)"=w2194) -> ("error out"=w2195:errorcluster)  [unwired: 2 out]
              }
            }
          }
          frame True {
            # "New Mk2 version"
            n931 = case shown="13" w2213 {
              tunnel: [256 ("Mon Channels") 128 ("Mon Channels") 128 ("Mon Channels") 128 ("Mon Channels") 128 ("Mon Channels") 256 ("Mon Channels") 128 ("Mon Channels") 64 ("Mon Channels") 32 ("Mon Channels") 256 ("Mon Channels") 256 ("Mon Channels") 256 ("Mon Channels") 128 ("Mon Channels") 256 ("Mon Channels") 128 ("Mon Channels") 256 ("Mon Channels") 256 ("Mon Channels")] -> w2215
              tunnel: [8 ("Bip Channels") 8 ("Bip Channels") 8 ("Bip Channels") 8 ("Bip Channels") 8 ("Bip Channels") 8 ("Bip Channels") 8 ("Bip Channels") 8 ("Bip Channels") 8 ("Bip Channels") 8 ("Bip Channels") 8 ("Bip Channels") 8 ("Bip Channels") 8 ("Bip Channels") 8 ("Bip Channels") 8 ("Bip Channels") 8 ("Bip Channels") 8 ("Bip Channels")] -> w2214
              tunnel: [8 ("Aux Channels") 8 ("Aux Channels") 8 ("Aux Channels") 8 ("Aux Channels") 8 ("Aux Channels") 8 ("Aux Channels") 8 ("Aux Channels") 8 ("Aux Channels") 8 ("Aux Channels") 8 ("Aux Channels") 8 ("Aux Channels") 8 ("Aux Channels") 8 ("Aux Channels") 8 ("Aux Channels") 8 ("Aux Channels") 8 ("Aux Channels") 8 ("Aux Channels")] -> w2217
              tunnel: [w2228 w2241 w2254 w2267 w2280 w2293 w2306 w2320 w2333 w2345 w2364 w2371 w2384 w2397 w2412 w2432 w2445] -> w2223
              tunnel: [i32[] [] ("Disabled Items []") i32[] [0, 1, 2, 9, 10, 11, 12] ("Disabled Items []") i32[] [0, 1, 2, 9, 10, 11, 12] ("Disabled Items []") i32[] [0, 1, 2, 9, 10, 11, 12] ("Disabled Items []") i32[] [0, 1, 2, 9, 10, 11, 12] ("Disabled Items []") i32[] [] ("Disabled Items []") i32[] [0, 1, 2, 9, 10, 11, 12] ("Disabled Items []") i32[] [0, 1, 2, 3, 7, 8, 9, 10, 11, 12] ("Disabled Items []") i32[] [0, 1, 2, 3, 4, 6, 7, 8, 9, 10, 11, 12] ("Disabled Items []") i32[] [] ("Disabled Items []") i32[] [] ("Disabled Items []") i32[] [] ("Disabled Items []") i32[] [0, 1, 2, 9, 10, 11, 12] ("Disabled Items []") i32[] [] ("Disabled Items []") w2420 i32[] [] ("Disabled Items []") i32[] [] ("Disabled Items []")] -> w2224
              tunnel: [i32[] [] ("Disabled Items []") i32[] [1, 2, 3] ("Disabled Items []") i32[] [1, 2, 3] ("Disabled Items []") i32[] [1, 2, 3] ("Disabled Items []") i32[] [1, 2, 3] ("Disabled Items []") i32[] [] ("Disabled Items []") i32[] [1, 2, 3] ("Disabled Items []") i32[] [1, 2, 3, 4] ("Disabled Items []") i32[] [1, 2, 3, 4, 5] ("Disabled Items []") i32[] [] ("Disabled Items []") i32[] [] ("Disabled Items []") i32[] [] ("Disabled Items []") i32[] [1, 2, 3] ("Disabled Items []") i32[] [] ("Disabled Items []") w2419 i32[] [] ("Disabled Items []") i32[] [] ("Disabled Items []")] -> w2222
              tunnel: [i32[] [] ("Disabled Items []") i32[] [3, 4] ("Disabled Items []") i32[] [3, 4] ("Disabled Items []") i32[] [3, 4] ("Disabled Items []") i32[] [3, 4] ("Disabled Items []") i32[] [] ("Disabled Items []") i32[] [3, 4] ("Disabled Items []") i32[] [2, 3, 4] ("Disabled Items []") i32[] [2, 3, 4] ("Disabled Items []") i32[] [] ("Disabled Items []") i32[] [] ("Disabled Items []") i32[] [] ("Disabled Items []") i32[] [3, 4] ("Disabled Items []") i32[] [] ("Disabled Items []") w2416 i32[] [] ("Disabled Items []") i32[] [] ("Disabled Items []")] -> w2221
              tunnel: [32 ("Aux Channels") 0 ("Aux Channels") 0 ("Aux Channels") 0 ("Aux Channels") 0 ("Aux Channels") 0 ("Aux Channels") 0 ("Aux Channels") 0 ("Aux Channels") 0 ("Aux Channels") 32 ("Aux Channels") 32 ("Aux Channels") 0 ("Aux Channels") 0 ("Aux Channels") 0 ("Aux Channels") 0 ("Aux Channels") 0 ("Aux Channels") 0 ("Aux Channels")] -> w2216
              tunnel: [0 ("ADC Rate") 2048 ("ADC Rate") 2048 ("ADC Rate") 2048 ("ADC Rate") 2048 ("ADC Rate") 2048 ("ADC Rate") 4096 ("ADC Rate") 8192 ("ADC Rate") 16384 ("ADC Rate") 2048 ("ADC Rate") 16384 ("ADC Rate") 4096 ("ADC Rate") 8192 ("ADC Rate") 8192 ("ADC Rate") 16384 ("ADC Rate") 2048 ("ADC Rate") 2048 ("ADC Rate")] -> w2218
              tunnel: [0 ("Nr of Chan") 610 ("Nr of Chan") 610 ("Nr of Chan") 610 ("Nr of Chan") 610 ("Nr of Chan") 282 ("Nr of Chan") 154 ("Nr of Chan") 90 ("Nr of Chan") 58 ("Nr of Chan") 314 ("Nr of Chan") 10 ("Nr of Chan") 282 ("Nr of Chan") 154 ("Nr of Chan") 282 ("Nr of Chan") 154 ("Nr of Chan") 562 ("Nr of Chan") 562 ("Nr of Chan")] -> w2220
              tunnel: [0 ("Nr of Chan") 2 ("Nr of Chan") 2 ("Nr of Chan") 2 ("Nr of Chan") 2 ("Nr of Chan") 2 ("Nr of Chan") 4 ("Nr of Chan") 8 ("Nr of Chan") 16 ("Nr of Chan") 2 ("Nr of Chan") 16 ("Nr of Chan") 4 ("Nr of Chan") 8 ("Nr of Chan") 8 ("Nr of Chan") 16 ("Nr of Chan") 2 ("Nr of Chan") 2 ("Nr of Chan")] -> w2219
              tunnel: [w2227 w2240 w2253 w2266 w2279 w2292 w2305 w2317 w2331 w2344 w2360 w2370 w2383 w2396 w2408 w2431 w2444] -> w2212
              tunnel: [i32[] [] ("Disabled Items []") i32[] [0, 1] ("Disabled Items []") i32[] [0, 1] ("Disabled Items []") i32[] [0, 1] ("Disabled Items []") i32[] [0, 1] ("Disabled Items []") i32[] [] ("Disabled Items []") i32[] [0, 1] ("Disabled Items []") i32[] [0, 1, 2] ("Disabled Items []") i32[] [0, 1, 2, 3] ("Disabled Items []") i32[] [] ("Disabled Items []") i32[] [] ("Disabled Items []") i32[] [] ("Disabled Items []") i32[] [0, 1] ("Disabled Items []") i32[] [] ("Disabled Items []") i32[] [0, 1] ("Disabled Items []") i32[] [] ("Disabled Items []") i32[] [] ("Disabled Items []")] -> w2211
              tunnel: w2209 -> [_ _ _ _ _ _ _ _ _ _ _ _ _ _ w2410 _ _]
              frame -1, Default {
                w2227 = i8 0 items=["A1 - H32 (256)", "A1 - E32 (160)", "A1 - D32 (128)", "A1 - B32 (64)", "A1 - A32 (32)", "A1 - A16 (16)", "A1 -A8 (8)", "None (0) "] ("TCP subset:")
                w2228 = i8 0 items=["All 264 Chan ", "A-H (256)", "A-E (160)", "ABCD (128)", "A+B (64)", "A (32)", "B (32)", "C (32)", "D (32)", "E (32)", "F (32)", "G (32)", "H(32)", "EXG (8)", "Free Choice"] ("Channels")
              }
              frame 0 {
                w2240 = i8 2 items=["A1 - H32 (256)", "A1 - E32 (160)", "A1 - D32 (128)", "A1 - B32 (64)", "A1 - A32 (32)", "A1 - A16 (16)", "A1 -A8 (8)", "None (0) "] ("TCP subset:")
                w2241 = i8 3 items=["All 264 Chan ", "A-H (256)", "A-E (160)", "ABCD (128)", "A+B (64)", "A (32)", "B (32)", "C (32)", "D (32)", "E (32)", "F (32)", "G (32)", "H(32)", "EXG (8)", "Free Choice"] ("Channels")
              }
              frame 1 {
                w2253 = i8 2 items=["A1 - H32 (256)", "A1 - E32 (160)", "A1 - D32 (128)", "A1 - B32 (64)", "A1 - A32 (32)", "A1 - A16 (16)", "A1 -A8 (8)", "None (0) "] ("TCP subset:")
                w2254 = i8 3 items=["All 264 Chan ", "A-H (256)", "A-E (160)", "ABCD (128)", "A+B (64)", "A (32)", "B (32)", "C (32)", "D (32)", "E (32)", "F (32)", "G (32)", "H(32)", "EXG (8)", "Free Choice"] ("Channels")
              }
              frame 2 {
                w2266 = i8 2 items=["A1 - H32 (256)", "A1 - E32 (160)", "A1 - D32 (128)", "A1 - B32 (64)", "A1 - A32 (32)", "A1 - A16 (16)", "A1 -A8 (8)", "None (0) "] ("TCP subset:")
                w2267 = i8 3 items=["All 264 Chan ", "A-H (256)", "A-E (160)", "ABCD (128)", "A+B (64)", "A (32)", "B (32)", "C (32)", "D (32)", "E (32)", "F (32)", "G (32)", "H(32)", "EXG (8)", "Free Choice"] ("Channels")
              }
              frame 3 {
                w2279 = i8 2 items=["A1 - H32 (256)", "A1 - E32 (160)", "A1 - D32 (128)", "A1 - B32 (64)", "A1 - A32 (32)", "A1 - A16 (16)", "A1 -A8 (8)", "None (0) "] ("TCP subset:")
                w2280 = i8 3 items=["All 264 Chan ", "A-H (256)", "A-E (160)", "ABCD (128)", "A+B (64)", "A (32)", "B (32)", "C (32)", "D (32)", "E (32)", "F (32)", "G (32)", "H(32)", "EXG (8)", "Free Choice"] ("Channels")
              }
              frame 4 {
                w2292 = i8 0 items=["A1 - H32 (256)", "A1 - E32 (160)", "A1 - D32 (128)", "A1 - B32 (64)", "A1 - A32 (32)", "A1 - A16 (16)", "A1 -A8 (8)", "None (0) "] ("TCP subset:")
                w2293 = i8 1 items=["All 264 Chan ", "A-H (256)", "A-E (160)", "ABCD (128)", "A+B (64)", "A (32)", "B (32)", "C (32)", "D (32)", "E (32)", "F (32)", "G (32)", "H(32)", "EXG (8)", "Free Choice"] ("Channels")
              }
              frame 5 {
                w2305 = i8 2 items=["A1 - H32 (256)", "A1 - E32 (160)", "A1 - D32 (128)", "A1 - B32 (64)", "A1 - A32 (32)", "A1 - A16 (16)", "A1 -A8 (8)", "None (0) "] ("TCP subset:")
                w2306 = i8 3 items=["All 264 Chan ", "A-H (256)", "A-E (160)", "ABCD (128)", "A+B (64)", "A (32)", "B (32)", "C (32)", "D (32)", "E (32)", "F (32)", "G (32)", "H(32)", "EXG (8)", "Free Choice"] ("Channels")
              }
              frame 6 {
                w2317 = i8 3 items=["A1 - H32 (256)", "A1 - E32 (160)", "A1 - D32 (128)", "A1 - B32 (64)", "A1 - A32 (32)", "A1 - A16 (16)", "A1 -A8 (8)", "None (0) "] ("TCP subset:")
                w2320 = i8 4 items=["All 264 Chan ", "A-H (256)", "A-E (160)", "ABCD (128)", "A+B (64)", "A (32)", "B (32)", "C (32)", "D (32)", "E (32)", "F (32)", "G (32)", "H(32)", "EXG (8)", "Free Choice"] ("Channels")
              }
              frame 7 {
                w2331 = i8 4 items=["A1 - H32 (256)", "A1 - E32 (160)", "A1 - D32 (128)", "A1 - B32 (64)", "A1 - A32 (32)", "A1 - A16 (16)", "A1 -A8 (8)", "None (0) "] ("TCP subset:")
                w2333 = i8 5 items=["All 264 Chan ", "A-H (256)", "A-E (160)", "ABCD (128)", "A+B (64)", "A (32)", "B (32)", "C (32)", "D (32)", "E (32)", "F (32)", "G (32)", "H(32)", "EXG (8)", "Free Choice"] ("Channels")
              }
              frame 8 {
                w2344 = i8 0 items=["A1 - H32 (256)", "A1 - E32 (160)", "A1 - D32 (128)", "A1 - B32 (64)", "A1 - A32 (32)", "A1 - A16 (16)", "A1 -A8 (8)", "None (0) "] ("TCP subset:")
                w2345 = i8 1 items=["All 264 Chan ", "A-H (256)", "A-E (160)", "ABCD (128)", "A+B (64)", "A (32)", "B (32)", "C (32)", "D (32)", "E (32)", "F (32)", "G (32)", "H(32)", "EXG (8)", "Free Choice"] ("Channels")
              }
              frame 9 {
                w2360 = i8 0 items=["A1 - H32 (256)", "A1 - E32 (160)", "A1 - D32 (128)", "A1 - B32 (64)", "A1 - A32 (32)", "A1 - A16 (16)", "A1 -A8 (8)", "None (0) "] ("TCP subset:")
                w2364 = i8 0 items=["All 256 Chan ", "A-G (224)", "A-E (160)", "ABCD (128)", "A+B (64)", "A (32)", "B (32)", "C (32)", "D (32)", "E (32)", "F (32)", "G (32)", "H(32)", "EXG (8)", "Free Choice"] ("Channels")
              }
              frame 10 {
                w2370 = i8 0 items=["A1 - H32 (256)", "A1 - E32 (160)", "A1 - D32 (128)", "A1 - B32 (64)", "A1 - A32 (32)", "A1 - A16 (16)", "A1 -A8 (8)", "None (0) "] ("TCP subset:")
                w2371 = i8 1 items=["All 264 Chan ", "A-H (256)", "A-E (160)", "ABCD (128)", "A+B (64)", "A (32)", "B (32)", "C (32)", "D (32)", "E (32)", "F (32)", "G (32)", "H(32)", "EXG (8)", "Free Choice"] ("Channels")
              }
              frame 11 {
                w2383 = i8 2 items=["A1 - H32 (256)", "A1 - E32 (160)", "A1 - D32 (128)", "A1 - B32 (64)", "A1 - A32 (32)", "A1 - A16 (16)", "A1 -A8 (8)", "None (0) "] ("TCP subset:")
                w2384 = i8 3 items=["All 264 Chan ", "A-H (256)", "A-E (160)", "ABCD (128)", "A+B (64)", "A (32)", "B (32)", "C (32)", "D (32)", "E (32)", "F (32)", "G (32)", "H(32)", "EXG (8)", "Free Choice"] ("Channels")
              }
              frame 12 {
                w2396 = i8 0 items=["A1 - H32 (256)", "A1 - E32 (160)", "A1 - D32 (128)", "A1 - B32 (64)", "A1 - A32 (32)", "A1 - A16 (16)", "A1 -A8 (8)", "None (0) "] ("TCP subset:")
                w2397 = i8 1 items=["All 264 Chan ", "A-H (256)", "A-E (160)", "ABCD (128)", "A+B (64)", "A (32)", "B (32)", "C (32)", "D (32)", "E (32)", "F (32)", "G (32)", "H(32)", "EXG (8)", "Free Choice"] ("Channels")
              }
              frame 13 {
                w2408 = i8 2 items=["A1 - H32 (256)", "A1 - E32 (160)", "A1 - D32 (128)", "A1 - B32 (64)", "A1 - A32 (32)", "A1 - A16 (16)", "A1 -A8 (8)", "None (0) "] ("TCP subset:")
                n932 = case shown="True" w2410 {
                  tunnel: [i32[] [0, 1, 2, 9, 10, 11, 12] ("Disabled Items []") i32[] [0, 1, 2, 3, 7, 8, 9, 10, 11, 12] ("Disabled Items []")] -> w2420
                  tunnel: [i32[] [1, 2, 3] ("Disabled Items []") i32[] [1, 2, 3, 4] ("Disabled Items []")] -> w2419
                  tunnel: [i32[] [3, 4] ("Disabled Items []") i32[] [2, 3, 4] ("Disabled Items []")] -> w2416
                  tunnel: [w2421 w2428] -> w2412
                  frame False {
                    w2421 = i8 3 items=["All 264 Chan ", "A-H (256)", "A-E (160)", "ABCD (128)", "A+B (64)", "A (32)", "B (32)", "C (32)", "D (32)", "E (32)", "F (32)", "G (32)", "H(32)", "EXG (8)", "Free Choice"] ("Channels")
                  }
                  frame True {
                    w2428 = i8 4 items=["All 264 Chan ", "A-H (256)", "A-E (160)", "ABCD (128)", "A+B (64)", "A (32)", "B (32)", "C (32)", "D (32)", "E (32)", "F (32)", "G (32)", "H(32)", "EXG (8)", "Free Choice"] ("Channels")
                  }
                }
              }
              frame 14 {
                w2431 = i8 0 items=["A1 - H32 (256)", "A1 - E32 (160)", "A1 - D32 (128)", "A1 - B32 (64)", "A1 - A32 (32)", "A1 - A16 (16)", "A1 -A8 (8)", "None (0) "] ("TCP subset:")
                w2432 = i8 1 items=["All 264 Chan ", "A-H (256)", "A-E (160)", "ABCD (128)", "A+B (64)", "A (32)", "B (32)", "C (32)", "D (32)", "E (32)", "F (32)", "G (32)", "H(32)", "EXG (8)", "Free Choice"] ("Channels")
              }
              frame 15 {
                w2444 = i8 0 items=["A1 - H32 (256)", "A1 - E32 (160)", "A1 - D32 (128)", "A1 - B32 (64)", "A1 - A32 (32)", "A1 - A16 (16)", "A1 -A8 (8)", "None (0) "] ("TCP subset:")
                w2445 = i8 1 items=["All 264 Chan ", "A-H (256)", "A-E (160)", "ABCD (128)", "A+B (64)", "A (32)", "B (32)", "C (32)", "D (32)", "E (32)", "F (32)", "G (32)", "H(32)", "EXG (8)", "Free Choice"] ("Channels")
              }
            }
          }
        }
        n933 = In Range and Coerce(upper limit=i8 13 ("y"), x=w1706, lower limit=i8 4 ("y")) -> (In Range?=w1770:bool)  [unwired: 1 out]
        n934 = Build Array (concatenate)(w1680, w1679, w1677) -> (w1678:i32[])
        n935 = Compound Arithmetic op=AND(w1770, w1781, "JazzOn") -> (w1769:bool)
        n936 = Select(t=w1813, s=w1769, f=w1810) -> (s? t:f=w1814:i32)
        n937 = Select(t=9 ("Nr of Chan"), s=w1769, f=w1810) -> (s? t:f=w1708:i32)
        n938 = Add(x=w1815, y=w1814) -> (x+y=w1816:i32)
        n939 = To Byte Integer(number=w1873) -> (8bit integer=w1882:i8[])
        n940 = To Byte Integer(number=w1877) -> (8bit integer=w1937:i8[])
        n941 = local read "Charts/Graphs"() -> (w1732:T2)
        n942 = Search 1D Array(1D array=w1882, element=w1879) -> (index of element=w1881:i32)  [unwired: 1 out]
        n943 = Unbundle By Name(w1812) -> ("Speed Mode"=w1865:i8)
        n944 = Search 1D Array(1D array=w1937, element=w1918) -> (index of element=w1936:i32)  [unwired: 1 out]
        n945 = Less Than 0?(x=w1881) -> (x < 0?=w1880:bool)
        n946 = Less Than 0?(x=w1936) -> (x < 0?=w1935:bool)
        n947 = To Byte Integer(number=w1878) -> (8bit integer=w1945:i8[])
        n948 = Select(t=w1879, s=w1880, f=w1875) -> (s? t:f=w1874:i8)
        n949 = Add(x=w1705, y=w1704) -> (x+y=w1703:i32)
        n950 = Select(t=w1918, s=w1935, f=w1790) -> (s? t:f=w1934:i8)
        n951 = Search 1D Array(1D array=w1945, element=w1920) -> (index of element=w1944:i32)  [unwired: 1 out]
        n952 = Not Equal?(x=w1865, y=w1706) -> (x != y?=w1947:bool)
        n953 = Less Than 0?(x=w1944) -> (x < 0?=w1943:bool)
        n954 = Equal?(x=w1706, y=i8 8) -> (x = y?=w1914:bool)
        n955 = Less Than 0?(x=w1706) -> (x < 0?=w1777:bool)
        n956 = Select(t=w1920, s=w1943, f=w1876) -> (s? t:f=w1942:i8)
        n957 = Not(x=w1777) -> (.not. x?=w1805:bool)
        n958 = Or(x=w1914, y=w1777) -> (x .or. y?=w1806:bool)
        n959 = Equal?(x=w1732, y=T2."Jazz" ("Charts/Graphs")) -> (x = y?=w1784:bool)
        n960 = Equal?(x=T2."ABR" ("Charts/Graphs"), y=w1732) -> (x = y?=w1733:bool)
        n961 = Not(x=w1769) -> (.not. x?=w1783:bool)
        n962 = Not(x="AbrOn") -> (.not. x?=w1728:bool)
        n963 = Not(x=w1770) -> (.not. x?=w1847:bool)
        n964 = Compound Arithmetic op=OR(w1770, w1777, w1778) -> (w1789:bool)
        n965 = And(x=w1784, y=w1783) -> (x .and. y?=w1731:bool)
        n966 = And(x=w1733, y=w1728) -> (x .and. y?=w1730:bool)
        n967 = Compound Arithmetic op=AND(w1847, w1805, w1778) -> (w1765:bool)
        n968 = Compound Arithmetic op=OR(w1950, w1947, w1730, w1731) -> (w1714:bool)
        n969 = local write "Channels"(w1942) -> ()
        n970 = local write "Offset"(w1934) -> ()
        n971 = for {
          N: w1703 -> [_]
          tunnel: [w2547] -> w1699 mode=indexing
          i -> [w2547]
        }
        n972 = Bundle By Name(cluster=w1812, "Mark2"=w1778, "GSR16Hz"=w1785, "JazzRec"=w1781, "Speed Mode"=w1706, "ADC Rate"=w1736, "ADC Channels"=w1816, "Screen Ratio"=w1872, "Mon Channels"=w1704, "Bip Channels"=w1705, "Aux Channels"=w1709, "Jazz Channels"=w1708, "Ana Channels"=w1707) -> (w1767:T8)
        n973 = property on="Channels" class="Ring (strict)"("Disabled Items []"=w1878) -> ()  [unwired: 2 in, 2 out]
        n974 = property on="Offset" class="Ring (strict)"("Disabled Items []"=w1877) -> ()  [unwired: 2 in, 2 out]
        n975 = property on="TCPsubset" class="Ring (strict)"("Disabled Items []"=w1873) -> ()  [unwired: 2 in, 2 out]
        n976 = Or(x=w1769, y=w1777) -> (x .or. y?=w1786:bool)
        n977 = case shown="False" w1777 {
          tunnel: w1769 -> [w2027 _]
          frame False {
            n978 = local write "JazzOn"(w2027) -> ()
          }
          frame True {
          }
        }
        n979 = Select(t=w1727, s=w1765, f=w1874) -> (s? t:f=w1726:i8)
        n980 = local write "TCPsubset"(w1726) -> ()
        n981 = case shown="2" w1706 {
          tunnel: [i32[] [1, 2, 3] ("Disabled Items []") i32[] [2, 3] ("Disabled Items []") i32[] [3] ("Disabled Items []") i32[] [] ("Disabled Items []") i32[] [1, 2, 3] ("Disabled Items []") i32[] [2, 3] ("Disabled Items []")] -> w1768
          tunnel: [u32 1 u32 3 u32 7 u32 15 u32 1 u32 3] -> w1764
          frame 0, Default {
          }
          frame 1 {
          }
          frame 2 {
          }
          frame 3 {
          }
          frame 14 {
          }
          frame 15 {
          }
        }
        n982 = Not Equal?(x=w1706, y=w1734) -> (x != y?=w1729:bool)
        n983 = Or(x=w1728, y=w1729) -> (x .or. y?=w1687:bool)
        n984 = Not Equal?(x=w1756, y=w1706) -> (x != y?=w1713:bool)
        n985 = case shown="True" w1714 {
          tunnel: w1713 -> [_ w1996]
          frame False {
          }
          frame True {
            n986 = Select(t=T2."Monopolar" ("Charts/Graphs"), s=w1996, f=T2."ABR" ("Charts/Graphs")) -> (s? t:f=w1995:T2)
            n987 = local write "Charts/Graphs"(w1995) -> ()
          }
        }
        n988 = Not And(1:w1713, 2:w1687) -> (0:w1676:bool)
        n989 = Select(t=w1680, s=w1676, f=w1678) -> (s? t:f=w1681:i32[])
        n990 = To Byte Integer(number=w1681) -> (8bit integer=w1941:i8[])
        n991 = Search 1D Array(1D array=w1941, element=w1919) -> (index of element=w1940:i32)  [unwired: 1 out]
        n992 = Less Than 0?(x=w1940) -> (x < 0?=w1939:bool)
        n993 = Select(t=w1919, s=w1939, f=w1933) -> (s? t:f=w1938:i8)
        n994 = And(x=w1691, y=w1676) -> (x .and. y?=w1690:bool)
        n995 = local write "Reference"(w1938) -> ()
        n996 = case shown="True" w1690 {
          tunnel: w1699 -> [w1985 w1989]
          tunnel: [w1985 w1988] -> w1686
          tunnel: [i32[] [] w1986] -> w1685
          frame False {
          }
          frame True {
            w1987 = 64 ("length")
            n997 = Delete From Array(array=w1989, length=w1987, index=w1987) -> (array with subset deleted=w1988:i32[])  [unwired: 1 out]
            n998 = for {
              N: w1987 -> [_]
              tunnel: w1987 -> [w1992]
              tunnel: [w1990] -> w1986 mode=indexing
              i -> [w1991]
              n999 = Add(x=w1992, y=w1991) -> (x+y=w1990:i32)
            }
          }
        }
        n1000 = property on="Reference" class="Ring (strict)"("Disabled Items []"=w1681) -> ()  [unwired: 2 in, 2 out]
        n1001 = for {
          tunnel: w1686 -> [w2564]
          shift-right: [w2560] -> w1910
          shift-left: i32[] [] -> [w2562]
          tunnel: w1917 -> [w2558] mode=indexing
          n1002 = Search 1D Array(1D array=w2564, element=w2558) -> (index of element=w2563:i32)  [unwired: 1 out]
          n1003 = Greater Or Equal To 0?(x=w2563) -> (x >= 0?=w2561:bool)
          n1004 = Build Array (concatenate)(w2562, w2558) -> (w2559:i32[])
          n1005 = Select(t=w2559, s=w2561, f=w2562) -> (s? t:f=w2560:i32[])
        }
        n1006 = for {
          tunnel: w1686 -> [w2554]
          shift-right: [w2550] -> w1931
          shift-left: i32[] [] -> [w2552]
          tunnel: w1916 -> [w2548] mode=indexing
          n1007 = Search 1D Array(1D array=w2554, element=w2548) -> (index of element=w2553:i32)  [unwired: 1 out]
          n1008 = Greater Or Equal To 0?(x=w2553) -> (x >= 0?=w2551:bool)
          n1009 = Build Array (concatenate)(w2552, w2548) -> (w2549:i32[])
          n1010 = Select(t=w2549, s=w2551, f=w2552) -> (s? t:f=w2550:i32[])
        }
        n1011 = property on="MonFree" class="LstBox (strict)"("Disabled Items"=w1685) -> ()  [unwired: 2 in, 2 out]
        n1012 = property on="RefFree" class="LstBox (strict)"("Disabled Items"=w1685) -> ()  [unwired: 2 in, 2 out]
        n1013 = Array Size(array=w1910) -> (size(s)=w1913:i32)
        n1014 = Equal To 0?(x=w1913) -> (x = 0?=w1912:bool)
        n1015 = Select(t=w1764, s=w1765, f=u32 1) -> (s? t:f=w1766:u32)
        n1016 = local write "RefFree"(w1931) -> ()
        n1017 = Select(t=i32[] [0], s=w1912, f=w1910) -> (s? t:f=w1700:i32[])
        n1018 = local write "MonFree"(w1700) -> ()
        n1019 = case shown="1" w1695 {
          tunnel: [w1966 w1970] -> w1696
          tunnel: w1697 -> [w1966 w1971]
          tunnel: [i32[] [] ("Disabled Items") w1968] -> w1694
          tunnel: w1676 -> [_ w1967]
          frame 0, Default {
          }
          frame 1 {
            n1020 = case shown="False" w1967 {
              tunnel: [i32[] [0, 1, 2, 3] i32[] [2, 3]] -> w1969
              tunnel: [i32[] [4, 5, 6] i32[] [0, 1, 4, 5, 6]] -> w1968
              frame False {
              }
              frame True {
              }
            }
            n1021 = for {
              tunnel: w1969 -> [w1983]
              shift-right: [w1979] -> w1970
              shift-left: i32[] [] -> [w1981]
              tunnel: w1971 -> [w1977] mode=indexing
              n1022 = Search 1D Array(1D array=w1983, element=w1977) -> (index of element=w1982:i32)  [unwired: 1 out]
              n1023 = Greater Or Equal To 0?(x=w1982) -> (x >= 0?=w1980:bool)
              n1024 = Build Array (concatenate)(w1981, w1977) -> (w1978:i32[])
              n1025 = Select(t=w1978, s=w1980, f=w1981) -> (s? t:f=w1979:i32[])
            }
          }
        }
        n1026 = property on="Box" class="Ring (strict)"("Visible"=w1765, "Disabled Items []"=w1768) -> ()  [unwired: 2 in, 2 out]
        n1027 = local read "RefFreeAvg1"() -> (w1906:i32[])
        n1028 = local read "MonFreeAvg2"() -> (w1900:i32)
        n1029 = local read "RefFreeAvg2"() -> (w1905:i32[])
        n1030 = local read "MonFreeAvg1"() -> (w1895:i32)
        n1031 = for {
          tunnel: w1686 -> [w2468]
          shift-right: [w2464] -> w1890
          shift-left: i32[] [] -> [w2466]
          tunnel: w1906 -> [w2462] mode=indexing
          n1032 = Search 1D Array(1D array=w2468, element=w2462) -> (index of element=w2467:i32)  [unwired: 1 out]
          n1033 = Greater Or Equal To 0?(x=w2467) -> (x >= 0?=w2465:bool)
          n1034 = Build Array (concatenate)(w2466, w2462) -> (w2463:i32[])
          n1035 = Select(t=w2463, s=w2465, f=w2466) -> (s? t:f=w2464:i32[])
        }
        n1036 = for {
          tunnel: w1686 -> [w2461]
          shift-right: [w2457] -> w1884
          shift-left: i32[] [] -> [w2459]
          tunnel: w1905 -> [w2455] mode=indexing
          n1037 = Search 1D Array(1D array=w2461, element=w2455) -> (index of element=w2460:i32)  [unwired: 1 out]
          n1038 = Greater Or Equal To 0?(x=w2460) -> (x >= 0?=w2458:bool)
          n1039 = Build Array (concatenate)(w2459, w2455) -> (w2456:i32[])
          n1040 = Select(t=w2456, s=w2458, f=w2459) -> (s? t:f=w2457:i32[])
        }
        n1041 = Search 1D Array(1D array=w1686, element=w1900) -> (index of element=w1902:i32)  [unwired: 1 out]
        n1042 = Search 1D Array(1D array=w1686, element=w1895) -> (index of element=w1898:i32)  [unwired: 1 out]
        n1043 = Greater Or Equal To 0?(x=w1902) -> (x >= 0?=w1901:bool)
        n1044 = Greater Or Equal To 0?(x=w1898) -> (x >= 0?=w1897:bool)
        n1045 = Quotient & Remainder(x=w1736, y=2048) -> (floor(x/y)=w1830:i32)  [unwired: 1 out]
        n1046 = Select(t=w1900, s=w1901, f=0) -> (s? t:f=w1893:i32)
        n1047 = Select(t=w1895, s=w1897, f=0) -> (s? t:f=w1894:i32)
        n1048 = Decrement(x=w1830) -> (x-1=w1829:i32)
        n1049 = property on="AuxFree" class="LstBox (strict)"("Disabled Items"=w1694) -> ()  [unwired: 2 in, 2 out]
        n1050 = local write "AuxFree"(w1696) -> ()
        n1051 = To Byte Integer(number=w1829) -> (8bit integer=w1828:i8)
        n1052 = Array Size(array=w1890) -> (size(s)=w1892:i32)
        n1053 = local read "TCPaddAnas"() -> (w1839:bool)
        n1054 = local read "TCPaddSens"() -> (w1841:bool)
        n1055 = Less Or Equal To 0?(x=w1736) -> (x <= 0?=w1825:bool)
        n1056 = local read "TCPaddJazz"() -> (w1788:bool)
        n1057 = local read "TCPaddTrig"() -> (w1835:bool)
        n1058 = Array Size(array=w1884) -> (size(s)=w1887:i32)
        n1059 = local read "TCPaddTP"() -> (w1843:bool)
        n1060 = local read "Averaging"() -> (w1837:bool)
        n1061 = local read "ScreenLength"() -> (w1823:i32)
        n1062 = Equal To 0?(x=w1892) -> (x = 0?=w1891:bool)
        n1063 = local read "AddTP"() -> (w1724:bool)
        n1064 = Equal To 0?(x=w1887) -> (x = 0?=w1886:bool)
        n1065 = Not(x=w1765) -> (.not. x?=w1738:bool)
        n1066 = Select(t=i32[] [0], s=w1891, f=w1890) -> (s? t:f=w1889:i32[])
        n1067 = Select(t=i32[] [0], s=w1886, f=w1884) -> (s? t:f=w1883:i32[])
        n1068 = case shown="True" w1676 {
          selector: w1676 -> [_ w2004]
          tunnel: w1894 -> [w2003 _]
          tunnel: w1889 -> [w2002 _]
          tunnel: w1893 -> [w2001 _]
          tunnel: w1883 -> [w2000 _]
          tunnel: [w2003 0 ("f")] -> w1723
          tunnel: [w2002 w2013] -> w1722
          tunnel: [w2001 2 ("f")] -> w1721
          tunnel: [w2000 w2013] -> w1720
          tunnel: [w1999 w2011] -> w1718
          tunnel: [w1999 w2011] -> w1715
          tunnel: [w1999 w2011] -> w1716
          tunnel: [w1999 w2011] -> w1717
          tunnel: ["with Jazz" ("Boolean Text.Text") "with ABR" ("Boolean Text.Text")] -> w1719
          tunnel: [w1997 w2006] -> w1712
          frame False {
            w1999 = T6."Enabled" ("Disabled")
            n1069 = local read "Decimation"() -> (w1997:i8)
          }
          frame True {
            w2006 = i8 0 items=["1", "1/2", "1/4", "1/8", "1/16", "1/32", "1/64"] ("Decimation")
            w2007 = TRUE
            w2011 = T6."Disabled and Grayed Out" ("Disabled")
            w2013 = i32[] [1] ("t")
            n1070 = local write "AbrOn"(w2004) -> ()
            n1071 = local write "Decimation"(w2006) -> ()
            n1072 = property on="AbrOn" class="Bool (strict)"("DisabledEnum"=T6."Disabled and Grayed Out" ("Disabled")) -> ()  [unwired: 2 in, 2 out]
            n1073 = local write "AvgLPfreq"(3334.0 ("AvgLPfreq")) -> ()
            n1074 = local write "AvgLP"(w2007) -> ()
            n1075 = local write "AvgHP"(w2007) -> ()
            n1076 = local write "AvgHPfreq"(100.0 ("AvgLPfreq")) -> ()
          }
        }
        n1077 = Scale By Power Of 2(n=w1712, x=1) -> (x*2^n=w1710:i32)
        n1078 = Bundle By Name(cluster=w1767, "ABR Enabled"=w1676, "Save Box"=w1766, "Decimate Ratio"=w1710) -> (w1711:T8)
        n1079 = Quotient & Remainder(x=w1736, y=w1710) -> (floor(x/y)=w1907:i32)  [unwired: 1 out]
        n1080 = To Double Precision Float(number=w1907) -> (double precision float=w1819:dbl)
        n1081 = Multiply(x=w1818, y=w1819) -> (x*y=w1908:dbl)
        n1082 = local write "MonFreeAvg1"(w1723) -> ()
        n1083 = local write "RefFreeAvg1"(w1722) -> ()
        n1084 = local write "MonFreeAvg2"(w1721) -> ()
        n1085 = local write "RefFreeAvg2"(w1720) -> ()
        n1086 = property on="MonFreeAvg1" class="LstBox (strict)"("DisabledEnum"=w1718) -> ()  [unwired: 2 in, 2 out]
        n1087 = property on="RefFreeAvg1" class="LstBox (strict)"("DisabledEnum"=w1715) -> ()  [unwired: 2 in, 2 out]
        n1088 = property on="MonFreeAvg2" class="LstBox (strict)"("DisabledEnum"=w1716) -> ()  [unwired: 2 in, 2 out]
        n1089 = property on="RefFreeAvg2" class="LstBox (strict)"("DisabledEnum"=w1717) -> ()  [unwired: 2 in, 2 out]
        n1090 = property on="with Jazz or ABR" class="Bool (strict)"("Caption.Text"=w1719) -> ()  [unwired: 2 in, 2 out]
        n1091 = local write "Bandwidth [Hz]"(w1908) -> ()
        n1092 = local write "Sample Rate [Hz]"(w1819) -> ()
        n1093 = Subtract(x=w1712, y=w1828) -> (x-y=w1827:i8)
        n1094 = Decrement(x=w1827) -> (x-1=w1791:i8)
        n1095 = Less Or Equal To 0?(x=w1791) -> (x <= 0?=w1826:bool)
        n1096 = Or(x=w1826, y=w1825) -> (x .or. y?=w1824:bool)
        n1097 = property on="AvgLP" class="Bool (strict)"("DisabledEnum"=w1718) -> ()  [unwired: 2 in, 2 out]
        n1098 = property on="AvgLPfreq" class="DigNum (strict)"("DisabledEnum"=w1715) -> ()  [unwired: 2 in, 2 out]
        n1099 = property on="AvgHP" class="Bool (strict)"("DisabledEnum"=w1716) -> ()  [unwired: 2 in, 2 out]
        n1100 = property on="AvgHPfreq" class="DigNum (strict)"("DisabledEnum"=w1717) -> ()  [unwired: 2 in, 2 out]
        n1101 = case shown="False" w1824 {
          tunnel: [w2030 i32[] [] ("Disabled Items []")] -> w1821
          tunnel: [w2031 w2035] -> w1822
          tunnel: w1823 -> [w2032 w2035]
          tunnel: w1791 -> [w2029 _]
          frame False {
            n1102 = To Long Integer(number=w2029) -> (32bit integer=w2028:i32)
            n1103 = Greater?(x=w2028, y=w2032) -> (0:w2033:bool)
            n1104 = for {
              N: w2028 -> [_]
              tunnel: [w2034] -> w2030 mode=indexing
              i -> [w2034]
            }
            n1105 = Select(t=w2028, s=w2033, f=w2032) -> (s? t:f=w2031:i32)
          }
          frame True {
          }
        }
        n1106 = And(x=w1738, y=w1837) -> (x .and. y?=w1836:bool)
        n1107 = And(x=w1724, y=w1789) -> (x .and. y?=w1725:bool)
        n1108 = And(x=w1835, y=w1738) -> (x .and. y?=w1834:bool)
        n1109 = Compound Arithmetic op=AND(w1843, w1789, w1738) -> (w1842:bool)
        n1110 = Compound Arithmetic op=AND(w1841, w1789, w1738) -> (w1840:bool)
        n1111 = Compound Arithmetic op=AND(w1839, w1806, w1738) -> (w1838:bool)
        n1112 = Compound Arithmetic op=AND(w1788, w1786, w1738) -> (w1787:bool)
        n1113 = local write "AddTP"(w1725) -> ()
        n1114 = local write "TCPaddTP"(w1842) -> ()
        n1115 = local write "TCPaddSens"(w1840) -> ()
        n1116 = local write "TCPaddAnas"(w1838) -> ()
        n1117 = local write "TCPaddJazz"(w1787) -> ()
        n1118 = local write "TCPaddTrig"(w1834) -> ()
        n1119 = local write "Averaging"(w1836) -> ()
        n1120 = property on="ScreenLength" class="Ring (strict)"("Disabled Items []"=w1821) -> ()  [unwired: 2 in, 2 out]
        n1121 = local write "ScreenLength"(w1822) -> ()
        n1122 = Array Size(array=w1696) -> (size(s)=w1863:i32)
        n1123 = property on="Charts/Graphs" class="TabCtl (strict)"() -> ("Pages"=w1861:refnum<vi>[])  [unwired: 2 in, 2 out]
        n1124 = Array Size(array=w1794) -> (size(s)=w1795:i32)
        n1125 = Array Size(array=w1849) -> (size(s)=w1864:i32)
        n1126 = Array Size(array=w1871) -> (size(s)=w1930:i32)
        n1127 = Not Equal To 0?(x=w1795) -> (x != 0?=w1792:bool)
        n1128 = Not Equal To 0?(x=w1864) -> (x != 0?=w1741:bool)
        n1129 = Not Equal To 0?(x=w1863) -> (x != 0?=w1862:bool)
        n1130 = Not Equal To 0?(x=w1930) -> (x != 0?=w1929:bool)
        n1131 = Index Array(array=w1861) -> (element #1=w1752:refnum<vi>, element #2=w1762:refnum<vi>, element #3=w1747:refnum<vi>, element #4=w1745:refnum<vi>, element #5=w1757:refnum<vi>, element #6=w1761:refnum<vi>, element #7=w1760:refnum<vi>, element #8=w1759:refnum<vi>, element #9=w1758:refnum<vi>)  [unwired: 10 in, 1 out]
        n1132 = Compound Arithmetic op=AND(w1862, w1789, w1713) -> (w1855:bool)
        n1133 = Compound Arithmetic op=AND(w1741, w1806, w1713) -> (w1851:bool)
        n1134 = Compound Arithmetic op=AND(w1792, w1786, w1713) -> (w1793:bool)
        n1135 = And(x=w1929, y=w1789) -> (x .and. y?=w1848:bool)
        n1136 = Unbundle By Name(w1928) -> ("All Labels"=w1800:string[])
        n1137 = Unbundle By Name(w1711) -> ("Mon Channels"=w1953:i32, "Bip Channels"=w1952:i32, "Aux Channels"=w1869:i32, "Jazz Channels"=w1799:i32, "Ana Channels"=w1804:i32)
        n1138 = Not(x=w1713) -> (.not. x?=w1740:bool)
        n1139 = And(x=w1848, y=w1713) -> (x .and. y?=w1751:bool)
        n1140 = And(x=w1713, y=w1738) -> (x .and. y?=w1737:bool)
        n1141 = Or(x=w1740, y=w1738) -> (x .or. y?=w1739:bool)
        n1142 = Select(t=T5."Page Enabled" ("Page Enabled State"), s=w1751, f=T5."Page Disabled & Grayed" ("Page Enabled State")) -> (s? t:f=w1859:T5)
        n1143 = Select(t=T5."Page Enabled" ("Page Enabled State"), s=w1793, f=T5."Page Disabled & Grayed" ("Page Enabled State")) -> (s? t:f=w1807:T5)
        n1144 = Array Size(array=w1800) -> (size(s)=w1927:i32)
        n1145 = Select(t=T5."Page Enabled" ("Page Enabled State"), s=w1851, f=T5."Page Disabled & Grayed" ("Page Enabled State")) -> (s? t:f=w1852:T5)
        n1146 = Select(t=T5."Page Enabled" ("Page Enabled State"), s=w1737, f=T5."Page Disabled & Grayed" ("Page Enabled State")) -> (s? t:f=w1844:T5)
        n1147 = Select(t=T5."Page Enabled" ("Page Enabled State"), s=w1855, f=T5."Page Disabled & Grayed" ("Page Enabled State")) -> (s? t:f=w1854:T5)
        n1148 = Select(t=T6."Enabled" ("Disabled"), s=w1848, f=T6."Disabled and Grayed Out" ("Disabled")) -> (s? t:f=w1870:T6)
        n1149 = Select(t=T5."Page Enabled" ("Page Enabled State"), s=w1739, f=T5."Page Disabled & Grayed" ("Page Enabled State")) -> (s? t:f=w1742:T5)
        n1150 = Decrement(x=w1927) -> (x-1=w1926:i32)
        n1151 = property on="Bipolar" class="Page"(reference=w1762, "Page Enabled State"=w1859) -> ()  [unwired: 1 in, 2 out]
        n1152 = property on="Sensors" class="Page"(reference=w1761, "Page Enabled State"=w1854) -> ()  [unwired: 1 in, 2 out]
        n1153 = property on="Jazz" class="Page"(reference=w1760, "Page Enabled State"=w1807) -> ()  [unwired: 1 in, 2 out]
        n1154 = property on="AIB" class="Page"(reference=w1759, "Page Enabled State"=w1852) -> ()  [unwired: 1 in, 2 out]
        n1155 = property on="TCP" class="Page"(reference=w1758, "Page Enabled State"=w1844) -> ()  [unwired: 1 in, 2 out]
        n1156 = property on="Average" class="Page"(reference=w1757, "Page Enabled State"=w1742) -> ()  [unwired: 1 in, 2 out]
        n1157 = property on="TP Offset Graph 1" class="WFGraph (strict)"("Disabled"=w1870) -> ()  [unwired: 2 in, 2 out]
        n1158 = property on="TP Offset Graph 2" class="WFGraph (strict)"("Disabled"=w1870) -> ()  [unwired: 2 in, 2 out]
        n1159 = Index Array(array=w1800, index=w1926) -> (element=w1803:string)
        n1160 = Array Subset(array=w1800, length=w1953) -> (w1958:string[])  [unwired: 1 in]
        n1161 = Array Subset(array=w1800, index=256, length=w1952) -> (w1957:string[])
        n1162 = Array Subset(array=w1800, index=264, length=w1869) -> (w1954:string[])
        n1163 = Array Subset(array=w1800, index=272, length=w1799) -> (w1801:string[])
        n1164 = Array Subset(array=w1800, index=281, length=w1804) -> (w1802:string[])
        n1165 = Build Array (concatenate)(w1958, w1957, w1954, w1801, w1802, w1803) -> (w1925:string[])
        n1166 = Select(t=T5."Page Enabled" ("Page Enabled State"), s=w1713, f=T5."Page Disabled & Grayed" ("Page Enabled State")) -> (s? t:f=w1754:T5)
        n1167 = Select(t=T5."Page Enabled" ("Page Enabled State"), s=w1713, f=T5."Page Disabled & Grayed" ("Page Enabled State")) -> (s? t:f=w1749:T5)
        n1168 = Select(t=T5."Page Enabled" ("Page Enabled State"), s=w1676, f=T5."Page Disabled & Grayed" ("Page Enabled State")) -> (s? t:f=w1746:T5)
        n1169 = property on="Monopolar" class="Page"(reference=w1752, "Page Enabled State"=w1754) -> ()  [unwired: 1 in, 2 out]
        n1170 = property on="Offset" class="Page"(reference=w1747, "Page Enabled State"=w1749) -> ()  [unwired: 1 in, 2 out]
        n1171 = property on="ABR" class="Page"(reference=w1745, "Page Enabled State"=w1746) -> ()  [unwired: 1 in, 2 out]
        n1172 = for {
          N: w1703 -> [_]
          tunnel: w1925 -> [w2556] mode=indexing
          tunnel: [w2555] -> w1702 mode=indexing
          n1173 = String Subset(string=w2556, length (rest)=5 ("length (rest)")) -> (substring=w2555:string)  [unwired: 1 out]
        }
        n1174 = for {
          tunnel: w1925 -> [w2545] mode=indexing
          tunnel: [w2544] -> w1923 mode=indexing
          n1175 = Format Into String(format string="%-16.16s", w2545) -> (resulting string=w2544:string)  [unwired: 2 in, 1 out]
        }
        n1176 = Bundle By Name(cluster=w1928, "Spec Labels"=w1923) -> (w1924:T10)
        n1177 = Select(t=string[] ["Left", "Ref", "Right"], s=w1676, f=w1702) -> (s? t:f=w1735:string[])
        n1178 = property on="MonFree" class="LstBox (strict)"("Item Names"=w1702) -> ()  [unwired: 2 in, 2 out]
        n1179 = property on="RefFree" class="LstBox (strict)"("Item Names"=w1702) -> ()  [unwired: 2 in, 2 out]
        n1180 = property on="RefFreeAvg1" class="LstBox (strict)"("Item Names"=w1735) -> ()  [unwired: 2 in, 2 out]
        n1181 = property on="MonFreeAvg1" class="LstBox (strict)"("Item Names"=w1735) -> ()  [unwired: 2 in, 2 out]
        n1182 = property on="RefFreeAvg2" class="LstBox (strict)"("Item Names"=w1735) -> ()  [unwired: 2 in, 2 out]
        n1183 = property on="MonFreeAvg2" class="LstBox (strict)"("Item Names"=w1735) -> ()  [unwired: 2 in, 2 out]
      }
      frame 2 {
        w2565 = T6."Disabled and Grayed Out" ("Disabled")
        w2600 = 5  # Go to State 5:    stop running
        w2575 = FALSE
        w2570 = FALSE
        w2586 = 0 ("Dimension Size")
        w2611 = FALSE  # Stop Running
        w2614 = 4  # Go to State 4    Displaying
        w2615 = 3  # Go to State 3     Saving
        # "Screen Duration"
        # "Sample Rate"
        # "Busy Saving"
        n1184 = flat-sequence {
          tunnel: w2581 -> [w2622]
          tunnel: w2579 -> [w2621]
          tunnel: w2580 -> [w2620]
          tunnel: w2579 -> [w2627]
          tunnel: w2579 -> [w2632]
          frame #0 {
            w2618 = 0 ("Dimension Size")
            # "Cear the Charts"
            n1185 = Initialize Array(w2618, w2618, w2618) -> (w2617:i32[][])
            n1186 = To Double Precision Float(number=w2617) -> (double precision float=w2616:dbl[][])
            n1187 = property on="Trigger Chart" class="WFChart (strict)"("History Data"=w2617) -> ()  [unwired: 2 in, 2 out]
            n1188 = property on="Mon Chart" class="WFChart (strict)"("History Data"=w2616) -> ()  [unwired: 2 in, 2 out]
            n1189 = property on="Bip Chart" class="WFChart (strict)"("History Data"=w2616) -> ()  [unwired: 2 in, 2 out]
            n1190 = property on="ABR Chart" class="WFChart (strict)"("History Data"=w2616) -> ()  [unwired: 2 in, 2 out]
            n1191 = property on="Aux Chart" class="WFChart (strict)"("History Data"=w2616) -> ()  [unwired: 2 in, 2 out]
            n1192 = property on="Jazz Chart" class="WFChart (strict)"("History Data"=w2616) -> ()  [unwired: 2 in, 2 out]
            n1193 = property on="Ana Chart" class="WFChart (strict)"("History Data"=w2616) -> ()  [unwired: 2 in, 2 out]
          }
          frame #1 {
            # "Scale the Charts"
            # "Set \"Chart History Lenght\" at:\n(x-scale lenghts in s) * (sample rate) + 1"
            # "Sample Rate on screen"
            n1194 = Multiply(x=w2620, y=w2621) -> (x*y=w2625:i32)
            n1195 = Quotient & Remainder(x=w2622, y=w2625) -> (floor(x/y)=w2624:i32)  [unwired: 1 out]
            n1196 = To Double Precision Float(number=w2624) -> (double precision float=w2623:dbl)
            n1197 = Reciprocal(x=w2623) -> (1/x=w2619:dbl)
            n1198 = property on="Mon Chart" class="WFChart (strict)"("X Scale.Offset and Multiplier:Multiplier"=w2619) -> ()  [unwired: 2 in, 2 out]
            n1199 = property on="Trigger Chart" class="WFChart (strict)"("X Scale.Offset and Multiplier:Multiplier"=w2619) -> ()  [unwired: 2 in, 2 out]
            n1200 = property on="Bip Chart" class="WFChart (strict)"("X Scale.Offset and Multiplier:Multiplier"=w2619) -> ()  [unwired: 2 in, 2 out]
            n1201 = property on="ABR Chart" class="WFChart (strict)"("X Scale.Offset and Multiplier:Multiplier"=w2619) -> ()  [unwired: 2 in, 2 out]
            n1202 = property on="Aux Chart" class="WFChart (strict)"("X Scale.Offset and Multiplier:Multiplier"=w2619) -> ()  [unwired: 2 in, 2 out]
            n1203 = property on="Jazz Chart" class="WFChart (strict)"("X Scale.Offset and Multiplier:Multiplier"=w2619) -> ()  [unwired: 2 in, 2 out]
            n1204 = property on="Ana Chart" class="WFChart (strict)"("X Scale.Offset and Multiplier:Multiplier"=w2619) -> ()  [unwired: 2 in, 2 out]
          }
          frame #2 {
            n1205 = To Double Precision Float(number=w2627) -> (double precision float=w2626:dbl)
            n1206 = property on="Mon Chart" class="WFChart (strict)"("X Scale.Range:Maximum"=w2626) -> ()  [unwired: 2 in, 2 out]
            n1207 = property on="Trigger Chart" class="WFChart (strict)"("X Scale.Range:Maximum"=w2626) -> ()  [unwired: 2 in, 2 out]
            n1208 = property on="Bip Chart" class="WFChart (strict)"("X Scale.Range:Maximum"=w2626) -> ()  [unwired: 2 in, 2 out]
            n1209 = property on="ABR Chart" class="WFChart (strict)"("X Scale.Range:Maximum"=w2626) -> ()  [unwired: 2 in, 2 out]
            n1210 = property on="Aux Chart" class="WFChart (strict)"("X Scale.Range:Maximum"=w2626) -> ()  [unwired: 2 in, 2 out]
            n1211 = property on="Jazz Chart" class="WFChart (strict)"("X Scale.Range:Maximum"=w2626) -> ()  [unwired: 2 in, 2 out]
            n1212 = property on="Ana Chart" class="WFChart (strict)"("X Scale.Range:Maximum"=w2626) -> ()  [unwired: 2 in, 2 out]
          }
          frame #3 {
            n1213 = Greater Or Equal?(x=1, y=w2632) -> (x >= y?=w2631:bool)
            n1214 = Select(t=u8 1, s=w2631, f=u8 0) -> (s? t:f=w2628:u8)
            n1215 = property on="Mon Chart" class="WFChart (strict)"("X Scale.Format & Precision:Precision"=w2628) -> ()  [unwired: 2 in, 2 out]
            n1216 = property on="Bip Chart" class="WFChart (strict)"("X Scale.Format & Precision:Precision"=w2628) -> ()  [unwired: 2 in, 2 out]
            n1217 = property on="ABR Chart" class="WFChart (strict)"("X Scale.Format & Precision:Precision"=w2628) -> ()  [unwired: 2 in, 2 out]
            n1218 = property on="Aux Chart" class="WFChart (strict)"("X Scale.Format & Precision:Precision"=w2628) -> ()  [unwired: 2 in, 2 out]
            n1219 = property on="Jazz Chart" class="WFChart (strict)"("X Scale.Format & Precision:Precision"=w2628) -> ()  [unwired: 2 in, 2 out]
            n1220 = property on="Ana Chart" class="WFChart (strict)"("X Scale.Format & Precision:Precision"=w2628) -> ()  [unwired: 2 in, 2 out]
          }
        }
        n1221 = Unbundle By Name(w2576) -> ("ADC Rate"=w2581:i32, "Screen Ratio"=w2580:i32)
        n1222 = for {
          N: 9 -> [_]
          tunnel: w2605 -> [w2660]
          tunnel: [w2656] -> w2606 mode=indexing
          i -> [w2661]
          n1223 = Multiply(x=w2660, y=w2661) -> (x*y=w2659:i32)
          n1224 = To Double Precision Float(number=w2659) -> (double precision float=w2658:dbl)
          n1225 = Bundle(w2658, u32 0) -> (w2656:cluster{dbl, u32})  [unwired: 1 out]
        }
        n1226 = property on="Ring Buffer" class="Knob (strict)"("Scale.Marker Values[]"=w2606) -> ()  [unwired: 2 in, 2 out]
        n1227 = property on="ScreenLength" class="Ring (strict)"("Disabled"=w2565) -> ()  [unwired: 2 in, 2 out]
        n1228 = property on="Decimation" class="Ring (strict)"("Disabled"=w2565) -> ()  [unwired: 2 in, 2 out]
        n1229 = property on="Buffer" class="Ring (strict)"("Disabled"=w2565) -> ()  [unwired: 2 in, 2 out]
        n1230 = property on="Load Configuration File" class="Bool"("Disabled"=w2565) -> ()  [unwired: 2 in, 2 out]
        n1231 = property on="Save Configuration File" class="Bool"("Disabled"=w2565) -> ()  [unwired: 2 in, 2 out]
        n1232 = property on="Edit" class="Bool"("Disabled"=w2565) -> ()  [unwired: 2 in, 2 out]
        n1233 = property on="LocalPort" class="DigNum (strict)"("Disabled"=w2565) -> ()  [unwired: 2 in, 2 out]
        n1234 = property on="TCPsubset" class="Ring (strict)"("Disabled"=w2565) -> ()  [unwired: 2 in, 2 out]
        n1235 = property on="TCPaddTP" class="Bool (strict)"("Disabled"=w2565) -> ()  [unwired: 2 in, 2 out]
        n1236 = property on="TCPaddSens" class="Bool (strict)"("Disabled"=w2565) -> ()  [unwired: 2 in, 2 out]
        n1237 = property on="TCPaddAnas" class="Bool (strict)"("Disabled"=w2565) -> ()  [unwired: 2 in, 2 out]
        n1238 = property on="TCPaddJazz" class="Bool (strict)"("Disabled"=w2565) -> ()  [unwired: 2 in, 2 out]
        n1239 = property on="TCPaddTrig" class="Bool (strict)"("Disabled"=w2565) -> ()  [unwired: 2 in, 2 out]
        n1240 = property on="JazzOn" class="Bool (strict)"("Disabled"=w2565) -> ()  [unwired: 2 in, 2 out]
        n1241 = property on="AbrOn" class="Bool (strict)"("DisabledEnum"=w2565) -> ()  [unwired: 2 in, 2 out]
        n1242 = global write "TCPidentification.glb" "TCP cluster"(T11 {"connection ID"=refnum, "remote address"="", "remote port"=0} ("TCP cluster")) -> ()
        n1243 = property on="Set Stride in kByte\n(default 128 kByte)" class="DigNum (strict)"("DisabledEnum"=w2565) -> ()  [unwired: 2 in, 2 out]
        n1244 = local write "Save Subset"("" ("Local Patient Identification")) -> ()
        n1245 = local write "with  8 EX"(w2575) -> ()
        n1246 = local write "with Sens"(w2575) -> ()
        n1247 = local write "with AIB"(w2575) -> ()
        n1248 = local write "RejAbs"(w2575) -> ()
        n1249 = local write "RejDif"(w2575) -> ()
        n1250 = local write "Box1"(w2575) -> ()
        n1251 = local write "Box2"(w2575) -> ()
        n1252 = local write "Box3"(w2575) -> ()
        n1253 = local write "Box4"(w2575) -> ()
        n1254 = Greater Than 0?(x=w2585) -> (x > 0?=w2584:bool)
        n1255 = To Double Precision Float(number=w2586) -> (double precision float=w2589:dbl)
        n1256 = case shown="True" w2584 {
          tunnel: w2585 -> [_ w2649]
          frame False {
          }
          frame True {
            n1257 = Divide(x=w2649, y=2.0) -> (x/y=w2651:dbl)
            n1258 = Decrement(x=w2651) -> (x-1=w2635:dbl)
            n1259 = property on="MonLPfreq" class="DigNum (strict)"("Data Range:Maximum"=w2635) -> ()  [unwired: 2 in, 2 out]
            n1260 = property on="BipLPfreq" class="DigNum (strict)"("Data Range:Maximum"=w2635) -> ()  [unwired: 2 in, 2 out]
            n1261 = property on="AbrLPfreq" class="DigNum (strict)"("Data Range:Maximum"=w2635) -> ()  [unwired: 2 in, 2 out]
            n1262 = property on="AvgLPfreq" class="DigNum (strict)"("Data Range:Maximum"=w2635) -> ()  [unwired: 2 in, 2 out]
            n1263 = property on="AnaHPfreq" class="DigNum (strict)"("Data Range:Maximum"=w2635) -> ()  [unwired: 2 in, 2 out]
            n1264 = local read "MonLPfreq"() -> (w2648:dbl)
            n1265 = local read "AvgLPfreq"() -> (w2642:dbl)
            n1266 = local read "AbrLPfreq"() -> (w2636:dbl)
            n1267 = local read "AnaLPfreq"() -> (w2639:dbl)
            n1268 = local read "BipLPfreq"() -> (w2645:dbl)
            n1269 = Less Or Equal?(x=w2645, y=w2635) -> (x <= y?=w2646:bool)
            n1270 = Less Or Equal?(x=w2648, y=w2635) -> (x <= y?=w2652:bool)
            n1271 = Less Or Equal?(x=w2642, y=w2635) -> (x <= y?=w2643:bool)
            n1272 = Less Or Equal?(x=w2639, y=w2635) -> (x <= y?=w2640:bool)
            n1273 = Less Or Equal?(x=w2636, y=w2635) -> (x <= y?=w2637:bool)
            n1274 = Select(t=w2645, s=w2646, f=w2635) -> (s? t:f=w2644:dbl)
            n1275 = Select(t=w2648, s=w2652, f=w2635) -> (s? t:f=w2647:dbl)
            n1276 = Select(t=w2642, s=w2643, f=w2635) -> (s? t:f=w2641:dbl)
            n1277 = Select(t=w2639, s=w2640, f=w2635) -> (s? t:f=w2638:dbl)
            n1278 = Select(t=w2636, s=w2637, f=w2635) -> (s? t:f=w2634:dbl)
            n1279 = local write "MonLPfreq"(w2647) -> ()
            n1280 = local write "BipLPfreq"(w2644) -> ()
            n1281 = local write "AbrLPfreq"(w2634) -> ()
            n1282 = local write "AnaLPfreq"(w2638) -> ()
            n1283 = local write "AvgLPfreq"(w2641) -> ()
          }
        }
        n1284 = global write "LoBatWarning.glb" "LoBatWarning"(w2570) -> ()
        n1285 = global write "JazzLoBatWarning.glb" "JazzLoBatWarning"(w2570) -> ()
        n1286 = global write "StopThreads.glb" "StopThreads"(w2570) -> ()
        n1287 = local write "Total Saved [sec]"(w2586) -> ()
        n1288 = property class="VI"("Front Panel Window:Closeable"=FALSE) -> ()  [unwired: 2 in, 2 out]
        n1289 = local write "Current File [MB]"(w2589) -> ()
        n1290 = property on="MonFree" class="LstBox (strict)"() -> ("Item Names"=w2590:string[])  [unwired: 2 in, 2 out]
        n1291 = Unbundle By Name(w2576) -> ("Mon Channels"=w2569:i32, "Bip Channels"=w2598:i32)
        n1292 = Format Into String(format string="%-4.4s", "" ("input 1")) -> (resulting string=w2592:string)  [unwired: 2 in, 1 out]
        n1293 = Build Array (concatenate)(w2590, w2592) -> (w2595:string[])
        n1294 = Add(x=w2569, y=w2598) -> (x+y=w2597:i32)
        n1295 = Match First String(2:w2595, 3:w2592) -> (0:w2596:i32)  [unwired: 1 out]
        n1296 = Not Equal?(x=w2596, y=w2597) -> (x != y?=w2591:bool)
        n1297 = Build Array(FALSE ("element"), w2591) -> (w2567:bool[])
        n1298 = case shown="True" w2571 {
          selector: w2571 -> [_ w2653]
          frame False {
          }
          frame True {
            n1299 = flat-sequence {
              tunnel: w2653 -> [w2654]
              frame #0 {
                n1300 = local write "Start Saving"(w2654) -> ()
              }
              frame #1 {
                n1301 = property on="Start Saving" class="Bool (strict)"("Boolean Text.Text"="Initializing") -> ()  [unwired: 2 in, 2 out]
              }
            }
          }
        }
        n1302 = call "Act_Error_7000.vi"("Error Code In"=w2567, "error in (no error)"=w2603) -> ("error out"=w2573:errorcluster)  [unwired: 2 out]
        n1303 = Unbundle By Name(w2573) -> ("status"=w2602:bool)
        n1304 = Select(t=w2615, s=w2571, f=w2614) -> (s? t:f=w2601:i32)
        n1305 = Select(t=w2600, s=w2602, f=w2601) -> (s? t:f=w2599:i32)
      }
      frame 3 {
        w2721 = 43 items=["No Error", "Manager Argument Error", "Memory Full", "Out of Zone", "End of File", "File Already Open", "Generic File IO Error", "File Not Found", "File Permission Error", "Disk Full", "Duplicate Path", "Too Many Files Open", "Not Enabled", "Resource File Not Found", "Cannot Add Resource", "Resource Not Found", "Image Not Found", "Image Memory Error", "Pen Does Not Exist", "Config Bad Type", "Config Token Not Found", "Config Parse Error", "Config Memory Error", "Bad External Code Format", "Bad External Code Offset", "External Code Not Present", "Null Window", "Destroy Window Mixup", "Null Menu", "Print Aborted", "Bad Print Record", "Print Driver Error", "Windows Error During Print", "Memory Error During Print", "Print Dialog Error", "Generic Print Error", "Invalid Device Refnum", "Device Not Found", "Device Parameter Error", "Device Unit Error", "Can't Open Device", "Device Call Aborted", "Generic Error", "Cancelled By User"]
        w2735 = 43 items=["No Error", "Manager Argument Error", "Memory Full", "Out of Zone", "End of File", "File Already Open", "Generic File IO Error", "File Not Found", "File Permission Error", "Disk Full", "Duplicate Path", "Too Many Files Open", "Not Enabled", "Resource File Not Found", "Cannot Add Resource", "Resource Not Found", "Image Not Found", "Image Memory Error", "Pen Does Not Exist", "Config Bad Type", "Config Token Not Found", "Config Parse Error", "Config Memory Error", "Bad External Code Format", "Bad External Code Offset", "External Code Not Present", "Null Window", "Destroy Window Mixup", "Null Menu", "Print Aborted", "Bad Print Record", "Print Driver Error", "Windows Error During Print", "Memory Error During Print", "Print Dialog Error", "Generic Print Error", "Invalid Device Refnum", "Device Not Found", "Device Parameter Error", "Device Unit Error", "Can't Open Device", "Device Call Aborted", "Generic Error", "Cancelled By User"]
        w2750 = FALSE  # Stop Running
        # "Jazz Chan Selection"
        # "Ana Chan Selection"
        # "Aux Chan Selection"
        # "Mon Chan Selection"
        # "path does exist"
        # "Current File in Byte"
        # "Header Lenght in Byte"
        n1306 = Unbundle By Name(w2724) -> ("Save Path"=w2673:path, "Mark2"=w2672:bool, "GSR16Hz"=w2671:bool, "ABR Enabled"=w2667:bool, "Jazz Channels"=w2683:i32, "Speed Mode"=w2675:i8, "ADC Rate"=w2727:i32, "Decimate Ratio"=w2728:i32, "Mon Channels"=w2712:i32, "Bip Channels"=w2711:i32, "Save Subset"=w2710:i8, "Add Touchproofs"=w2709:bool, "Add Sensors"=w2705:bool, "Add Jazz"=w2688:bool, "Add Anas"=w2689:bool, "Save Box"=w2690:u32)
        n1307 = Not Equal To 0?(x=w2683) -> (x != 0?=w2678:bool)
        n1308 = Unbundle By Name(w2664) -> ("ABRlocation"=w2663:i8)
        n1309 = Bundle("Save Subset"=w2710, "Add Touchproofs"=w2709, "Add Sensors"=w2705, "Add Jazz"=w2688, "Add Anas"=w2689, "Save Box"=w2690) -> (w2733:T20)  [unwired: 1 out]
        n1310 = call "BDFlocal-ABR-EEG.vi"("ABR Enabled"=w2667, "ABRlocation"=w2663, "Default Save Cluster"=w2733, "Speedmode"=w2675, "JazzOn"=w2678, "Mark2"=w2672) -> ("error out"=w2679:errorcluster, "Save Cluster"=w2723:T20, "Local ID"=w2746:T21, "Save Subset"=w2666:string)
        n1311 = Strip Path(path=w2673) -> (stripped path=w2681:path, name=w2697:string)
        n1312 = Bundle("Mark2"=w2672, "GSR16Hz"=w2671, w2678, "Speed Mode"=w2675, "ABR Enabled"=w2667) -> (w2716:T22)  [unwired: 1 out]
        n1313 = Unbundle By Name(w2679) -> ("code"=w2722:i32)
        n1314 = File/Directory Info(path=w2681, error in=w2679) -> (directory=w2680:bool)  [unwired: 6 out]
        n1315 = Unbundle By Name(w2723) -> ("Save Subset"=w2715:i8, "Add Touchproofs"=w2713:bool, "Add Sensors"=w2708:bool, "Add Jazz"=w2685:bool, "Add Anas"=w2686:bool, "Save Box"=w2687:u32)
        n1316 = Equal?(x=w2722, y=w2721) -> (x = y?=w2719:bool)
        n1317 = Or(x=w2680, y=w2719) -> (x .or. y?=w2720:bool)
        n1318 = case shown="False" w2720 {
          tunnel: [w2753 w2761] -> w2700
          tunnel: w2679 -> [w2755 w2760]
          tunnel: w2681 -> [_ w2761]
          tunnel: [w2757 w2760] -> w2698
          frame False {
            w2753 = path ""  # Empty Path
            w2757 = errorcluster {"status"=FALSE, "code"=0, "source"=""}  # No Error
            w2752 = FALSE ("element")
            n1319 = Build Array(w2752, w2752, w2752, TRUE ("element")) -> (w2751:bool[])
            n1320 = call "Act_Error_7000.vi"("Error Code In"=w2751, "error in (no error)"=w2755) -> ("[user-defined descriptions]"=w2758:string[], "[user-defined codes]"=w2759:i32[], "error out"=w2754:errorcluster)
            n1321 = call <vilib>:"General Error Handler.vi"("[user-defined codes]"=w2759, "[user-defined descriptions]"=w2758, "error in (no error)"=w2754) -> ()  [unwired: 2 in, 11 out]
          }
          frame True {
          }
        }
        n1322 = File Dialog(4:"BioSemi Data Format" ("pattern label"), 6:"*.bdf" ("pattern (all files)"), 7:"Enter filename:" ("prompt"), 8:w2698, 9:w2697, 11:w2700) -> (0:w2699:errorcluster, 3:w2701:path)  [unwired: 3 out]
        n1323 = Unbundle By Name(w2664) -> ("ElecGain"=w2682:i8, "BreathBelt"=w2677:i8, "ABRlocation"=w2665:i8)
        n1324 = Open/Create/Replace File(file path (use dialog)=w2701, error in=w2699, operation (0:open)=T12."replace or create with confirmation") -> (refnum out=w2703:refnum<file>, error out=w2702:errorcluster)  [unwired: 4 out]
        n1325 = Bundle("ABR Enabled"=w2667, "Speed Mode"=w2675, "Save Subset"=w2715, "Initially Channel Selection"=w2714, "Add Touchproofs"=w2713, "Mon Channels"=w2712, "Bip Channels"=w2711, "Add Sensors"=w2708, "Initially Channel Selection"=w2707, "Add Jazz"=w2685, "Initially Channel Selection"=w2684, "Add Anas"=w2686, "Initially Channel Selection"=w2706, "Save Box"=w2687) -> (w2670:T17)  [unwired: 1 out]
        n1326 = Initialize Array(u8 255, 1) -> (w2742:u8[])
        n1327 = call "Write File+ [U8].vi"("1D array"=w2742, "error in (no error)"=w2702, "refnum"=w2703) -> ("error out"=w2747:errorcluster, "dup refnum"=w2748:refnum<file>)  [unwired: 2 in, 2 out]
        n1328 = Unbundle By Name(w2749) -> ("Spec Labels"=w2745:string[])
        n1329 = call "SaveSelect-ABR-EEG.vi"("Save Selection Cluster"=w2670, "ABRlocation"=w2665) -> ("ChanSelection"=w2669:i32[])  [unwired: 1 out]
        n1330 = Array Size(array=w2742) -> (size(s)=w2732:i32)
        n1331 = call "BDFheader-ABR-EEG.vi"("ElecGain"=w2682, "BreathBelt"=w2677, "ABRlocation"=w2665, "ChanSelection"=w2669, "Configuration"=w2716, "BDF Label Array"=w2745, "Decimate Ratio"=w2728, "ADC Sample Rate"=w2727, "Local ID"=w2746, "PreHeader Lenght"=w2732) -> ("BDF header Out"=w2731:string, "Total Header Lenght Out"=w2718:i32)
        n1332 = call "Write File+ [String].vi"("String"=w2731, "error in (no error)"=w2747, "refnum"=w2748) -> ("error out"=w2737:errorcluster, "dup refnum"=w2726:refnum<file>)  [unwired: 2 in, 2 out]
        n1333 = Equal?(x=w2675, y=i8 9) -> (x = y?=w2674:bool)
        n1334 = Or(x=w2667, y=w2674) -> (x .or. y?=w2668:bool)
        n1335 = Unbundle By Name(w2737) -> ("status"=w2740:bool, "code"=w2741:i32)
        n1336 = Equal?(x=w2741, y=w2735) -> (x = y?=w2738:bool)
        n1337 = case shown="True" w2740 {
          tunnel: [w2785 w2795] -> w2730
          tunnel: [w2784 w2796] -> w2739
          tunnel: w2738 -> [_ w2797]
          tunnel: w2737 -> [w2783 w2794]
          tunnel: [w2783 w2793] -> w2736
          tunnel: w2718 -> [w2782 w2792]
          tunnel: [w2782 w2791] -> w2717
          tunnel: w2726 -> [w2779 w2790]
          tunnel: [w2779 w2789] -> w2691
          tunnel: w2666 -> [w2773 _]
          tunnel: w2713 -> [w2776 _]
          tunnel: w2708 -> [w2777 _]
          tunnel: w2735 -> [_ w2788]
          tunnel: [T6."Enabled" ("Disabled") T6."Disabled and Grayed Out" ("Disabled")] -> w2729
          tunnel: w2724 -> [w2781 w2787]
          tunnel: [w2780 w2787] -> w2725
          tunnel: w2715 -> [w2778 _]
          tunnel: w2687 -> [w2767 _]
          tunnel: w2686 -> [w2766 _]
          tunnel: w2685 -> [w2763 _]
          tunnel: w2668 -> [w2762 _]
          frame False {
            w2785 = TRUE  # Busy Saving
            w2784 = 4  # Go to State 4: Display with Save
            n1338 = Number To Boolean Array(number=w2767) -> (Boolean array=w2772:bool[])
            n1339 = Index Array(array=w2772) -> (element #1=→"Box1":bool, element #2=→"Box2":bool, element #3=→"Box3":bool, element #4=→"Box4":bool)  [unwired: 4 in]
            n1340 = Or(x=w2763, y=w2762) -> (x .or. y?=→"with Jazz or ABR":bool)
            n1341 = Refnum to Path(1:w2779) -> (0:w2774:path)
            n1342 = Bundle By Name(cluster=w2781, "Save Path"=w2774, "Save Subset"=w2778, "Add Touchproofs"=w2776, "Add Sensors"=w2777, "Add Jazz"=w2763, "Add Anas"=w2766, "Save Box"=w2767) -> (w2780:T8)
            n1343 = Path To String(path=w2774) -> (string=→"BDF Filepath":string)
            "with  8 EX" <- w2776
            "with Sens" <- w2777
            "with AIB" <- w2766
            "Save Subset" <- w2773
          }
          frame True {
            n1344 = case shown="True" w2797 {
              tunnel: [w2802 w2814] -> w2796
              tunnel: [w2801 w2805] -> w2795
              tunnel: w2794 -> [w2800 w2811]
              tunnel: [w2800 w2812] -> w2793
              tunnel: w2792 -> [w2799 _]
              tunnel: [w2799 0 ("Total Header Lenght Out")] -> w2791
              tunnel: w2790 -> [w2798 w2807]
              tunnel: [w2798 w2803] -> w2789
              tunnel: w2788 -> [_ w2810]
              frame False {
                w2801 = TRUE  # Busy Saving
                w2802 = 5  # Go to State 5: Stop
              }
              frame True {
                w2803 = refnum<file> refnum  # Dummy Refnum
                w2804 = FALSE  # Start Saving
                w2805 = FALSE  # Busy Saving
                n1345 = Close File(refnum=w2807, error in=w2811) -> (error out=w2813:errorcluster)  [unwired: 1 out]
                n1346 = Unbundle By Name(w2813) -> ("code"=w2809:i32)
                n1347 = Equal?(x=w2810, y=w2809) -> (x = y?=w2808:bool)
                n1348 = case shown="True" w2808 {
                  tunnel: [w2816 w2818] -> w2814
                  tunnel: w2813 -> [w2815 _]
                  tunnel: [w2815 w2817] -> w2812
                  frame False {
                    w2816 = 5  # Go to State 5: Stop
                  }
                  frame True {
                    w2817 = errorcluster {"status"=FALSE, "code"=0, "source"=""}  # no error
                    w2818 = 4  # Go to State 4: Display  without Save
                  }
                }
                n1349 = local write "Start Saving"(w2804) -> ()
              }
            }
          }
        }
        n1350 = property on="Pause Saving" class="Bool (strict)"("Disabled"=w2729) -> ()  [unwired: 2 in, 2 out]
        n1351 = To Quad Integer(1:w2717) -> (0:w2693:i64)
        n1352 = local write "Pause Saving"(w2730) -> ()
      }
      frame 4 {
        w2840 = TRUE  # Paused
        w2845 = i8 0 items=["Raw unreferenced", "LF referenced", "HF referenced"] ("AbrChannels")
        w2848 = i16 650  # MinPanelHeight
        w2852 = 23.0  # YT2
        w2853 = 9.0  # YT1
        w2851 = 32.0  # YT3
        w2858 = bool[] [FALSE, FALSE, FALSE, FALSE, FALSE, FALSE, FALSE, FALSE, FALSE, FALSE, FALSE, FALSE, FALSE, FALSE, FALSE]  # 15 Triggers Out
        w2936 = 0.3 ("y")
        w2950 = 1.089  # Screen Ratio
        w2977 = i32[] [] ("Initially Empty Save Array")
        w2866 = 512  # GSR/Jazz sample rate
        w2871 = FALSE  # JazzLoBatChange
        w2884 = TRUE  # Initially Filter Reset
        w2888 = FALSE  # Not Start with Save
        w2889 = FALSE  # Initialy Not Start Saving
        w2893 = 0  # Box
        w2897 = 0 ("f")
        w2919 = 3  # 3 Bytes per Sample
        w2933 = 16  # Nr of Displayed Triggers
        w2942 = FALSE
        w2968 = 24.0  # Y2
        w2967 = 22.0  # Y1
        w2969 = 45.0  # Y3
        w2876 = i16 0  # Sync Errors
        w2952 = 44.0  # Clear Block
        w2962 = FALSE  # Initialy Not Last Call
        w2965 = 0 ("dimension size")
        w2970 = u32 13421823  # Color
        w2981 = FALSE  # LoBatChange
        w2986 = FALSE  # Second Half
        w2846 = TRUE  # Initially Filter Reset
        w2990 = i8 2  # Intiallly Screen Reset
        w2947 = 0  # Index
        w2988 = u8 0  # U8
        w2833 = i64 0  # Integer 64
        w2995 = FALSE  # Stop Running
        w3001 = 2  # Go to State 2:  Start Saving
        w2875 = FALSE  # Recent Sync Error
        w2837 = 0
        w2999 = 5  # Go to State 5: Close
        # "AsynchTime"
        # "variable Coen"
        # "StimIndice"
        # "Close triggerPort"
        # "SaveChanSelect"
        # "JazzOn"
        # "Sart with Save"
        # "Ringbuffer"
        # "Screen Duration"
        # "Config Changed"
        # "Busy Saving"
        # "Save Buffer"
        # "Busy Saving"
        # "Samples per Record"
        # "Label Cluster"
        # "Save Blocksize in Bytes"
        # "Busy Saving"
        n1353 = Unbundle By Name(w2931) -> ("Jazz Channels"=w2862:i32, "GSR16Hz"=w2869:bool, "ADC Rate"=w2867:i32, "ADC Channels"=w2873:i32, "Screen Ratio"=w2863:i32, "Decimate Ratio"=w2882:i32)
        n1354 = To Double Precision Float(number=w2949) -> (double precision float=w2850:dbl)
        n1355 = To Quad Integer(1:w2949) -> (0:w2892:i64)
        n1356 = To Double Precision Float(number=w2863) -> (double precision float=w2951:dbl)
        n1357 = To Double Precision Float(number=w2863) -> (double precision float=w2849:dbl)
        n1358 = Select(t=8 ("length"), s="TCPaddTP", f=w2897) -> (s? t:f=w2907:i32)
        n1359 = To Double Precision Float(number=w2949) -> (double precision float=w2954:dbl)
        n1360 = case shown="0, Default" "TCPsubset" {
          tunnel: [256 ("length") 160 ("length") 128 ("length") 64 ("length") 32 ("length") 16 ("length") 8 ("length") 0 ("length")] -> w2908
          frame 0, Default {
          }
          frame 1 {
          }
          frame 2 {
          }
          frame 3 {
          }
          frame 4 {
          }
          frame 5 {
          }
          frame 6 {
          }
          frame 7 {
          }
        }
        n1361 = Select(t=7, s="TCPaddSens", f=w2897) -> (s? t:f=w2906:i32)
        n1362 = Compound Arithmetic op=MULTIPLY(w2952, w2850, w2849) -> (w2953:dbl)
        n1363 = Select(t=9, s="TCPaddJazz", f=w2897) -> (s? t:f=w2905:i32)
        n1364 = Not Equal To 0?(x=w2862) -> (x != 0?=w2859:bool)
        n1365 = property on="Charts/Graphs" class="TabCtl (strict)"() -> ("Pages"=w2901:refnum<vi>[])  [unwired: 2 in, 2 out]
        n1366 = Not(x=w2869) -> (.not. x?=w2864:bool)
        n1367 = Select(t=32, s="TCPaddAnas", f=w2897) -> (s? t:f=w2904:i32)
        n1368 = Select(t=1, s="TCPaddTrig", f=w2897) -> (s? t:f=w2895:i32)
        n1369 = Multiply(x=w2949, y=w2863) -> (x*y=w2932:i32)
        n1370 = Or(x=w2859, y=w2864) -> (x .or. y?=w2868:bool)
        n1371 = Quotient & Remainder(x=w2867, y=w2866) -> (floor(x/y)=w2865:i32)  [unwired: 1 out]
        n1372 = for {
          tunnel: w2901 -> [w3238] mode=indexing
          shift-right: [w3232] -> w2899
          shift-left: i32[] [] ("Disabled Items []") -> [w3234]
          i -> [w3233]
          n1373 = property class="Page"(reference=w3238) -> ("Page Enabled State"=w3237:T5)  [unwired: 1 in, 2 out]
          n1374 = Equal?(x=T5."Page Enabled" ("Page Enabled State"), y=w3237) -> (x = y?=w3235:bool)
          n1375 = case shown="False" w3235 {
            tunnel: w3234 -> [w3241 w3242]
            tunnel: w3233 -> [w3239 _]
            tunnel: [w3240 w3242] -> w3232
            frame False {
              n1376 = Build Array (concatenate)(w3241, w3239) -> (w3240:i32[])
            }
            frame True {
            }
          }
        }
        n1377 = Compound Arithmetic op=MULTIPLY(w2950, w2954, w2951) -> (w2856:dbl)
        n1378 = Select(t=w2865, s=w2868, f=w2863) -> (s? t:f=w2870:i32)
        n1379 = Quotient & Remainder(x=w2932, y=w2882) -> (floor(x/y)=w2894:i32)  [unwired: 1 out]
        n1380 = call "Act_Stride.vi"("JazzOn"=w2859, "Stride in kByte"="Set Stride in kByte\n(default 128 kByte)", "Buffer Size in Byte"=w2860) -> ("RingBuffer"=w2838:i32[], "Buffer Size in Words"=w2836:i64, "Handle Out"=w2835:i64)
        n1381 = Compound Arithmetic op=ADD(w2908, w2907, w2906, w2905, w2904, w2895) -> (w2909:i32)
        "Channels sent by TCP" <- w2909
        n1382 = Bundle("length"=w2908, "f"=w2907, "f"=w2906, "f"=w2905, "f"=w2904, "f"=w2895) -> (w2903:T23)  [unwired: 1 out]
        n1383 = Multiply(x=w2873, y=w2867) -> (x*y=w2881:i32)
        n1384 = Multiply(x=w2873, y=w2932) -> (x*y=w2922:i32)
        n1385 = Multiply(x=w2873, y=w2870) -> (x*y=w2921:i32)
        n1386 = Multiply(x=w2891, y=2) -> (x*y=w2987:i32)
        n1387 = Bundle(w2942, w2942, w2942, w2942, w2942, w2942, w2942, w2942) -> (w2941:T24)  [unwired: 1 out]
        n1388 = Bundle By Name(cluster=T13 {"Start Averaging"=FALSE, "Busy Averaging"=FALSE, "Sweep Lenght in Samples"=0, "Valid Sweeps"=0, "Rejected Sweeps"=0, "First Graph Update"=FALSE} ("Avg Cluster In"), "Sweep Lenght in Samples"=w2945) -> (w2963:T13)
        n1389 = Multiply(x=w2919, y=w2909) -> (x*y=w2918:i32)
        n1390 = Bundle("Clear Block"=w2952, "Screen Ratio"=w2950, "Y1"=w2967, "Y2"=w2968, "Y3"=w2969, "Color"=w2970, "YT1"=w2853, "YT2"=w2852, "YT3"=w2851) -> (w2955:T25)  [unwired: 1 out]
        n1391 = Bundle By Name(cluster=w2955, "Clear Block"=w2953, "Screen Ratio"=w2856) -> (w2855:T25)
        n1392 = Initialize Array(w2988, w2987) -> (w2985:u8[])
        n1393 = Greater?(x=w2922, y=w2921) -> (0:w2923:bool)
        n1394 = To Double Precision Float(number=w2933) -> (double precision float=w2934:dbl)
        n1395 = Decrement(x=w2936) -> (x-1=w2935:dbl)
        n1396 = Select(t=w2922, s=w2923, f=w2921) -> (s? t:f=w2920:i32)
        n1397 = Negate(x=w2935) -> (-x=w2938:dbl)
        n1398 = Add(x=w2934, y=w2936) -> (x+y=w2937:dbl)
        n1399 = Bundle("Sync Errors"=w2876, "Recent Sync Error"=w2875) -> (w2874:T26)  [unwired: 1 out]
        n1400 = Initialize Array(0.0 ("element"), w2965, w2965) -> (w2964:dbl[][])
        n1401 = To Quad Integer(1:w2881) -> (0:w2831:i64)
        n1402 = Bundle(w2831, "64bit integer"=i64 282) -> (w2832:cluster{i64, "64bit integer":i64})  [unwired: 1 in]
        n1403 = Quotient & Remainder(x=w2920, y=w2873) -> (floor(x/y)=w2930:i32)  [unwired: 1 out]
        n1404 = To Quad Integer(1:w2920) -> (0:w2834:i64)
        n1405 = property on="Trigger Chart" class="WFChart (strict)"("Y Scale.Range:Maximum"=w2937) -> ()  [unwired: 2 in, 2 out]
        n1406 = property on="Trigger Chart" class="WFChart (strict)"("Y Scale.Range:Minimum"=w2938) -> ()  [unwired: 2 in, 2 out]
        n1407 = call "Empty Picture"() -> ("empty picture"=w2854:picture)
        n1408 = Select(t=1, s=w2878, f=w2837) -> (s? t:f=w2940:i32)
        n1409 = Quotient & Remainder(x=w2930, y=w2882) -> (floor(x/y)=w2902:i32)  [unwired: 1 out]
        "TCP samples/channel" <- w2902
        n1410 = Multiply(x=w2902, y=w2918) -> (x*y=→"Bytes in TCP Array":i32)
        n1411 = Bundle("LoBatChange"=w2981, "JazzLoBatChange"=w2871) -> (w2944:T27)  [unwired: 1 out]
        n1412 = To Quad Integer(1:w2891) -> (0:w2890:i64)
        n1413 = Scale By Power Of 2(n=20, x=i64 1) -> (x*2^n=w2959:i64)
        n1414 = To Quad Integer(1:w2837) -> (0:w2847:i64)
        n1415 = while {
          tunnel: w2838 -> [w3027]
          shift-right: [w3032] -> _
          shift-left: w2833 -> [w3039]
          shift-right: [w3034] -> _
          shift-left: w2833 -> [w3035]
          tunnel: w2836 -> [w3033]
          shift-right: [w3030] -> _
          shift-left: _ -> [w3036]
          tunnel: w2835 -> [w3038]
          tunnel: w2832 -> [w3031]
          shift-right: [w3025] -> _
          shift-left: w2833 -> [w3026]
          shift-right: [w3017] -> _
          shift-left: i64 0 ("New Display Blocksize") -> [w3023]
          shift-right: [w3013] -> _
          shift-left: w2828 -> [w3016]
          shift-right: [w3014] -> _
          shift-left: w2829 -> [w3015]
          shift-right: [w3011] -> _
          shift-left: w2827 -> [w3012]
          tunnel: w2826 -> [w3010]
          tunnel: [w3009] -> w2822
          tunnel: w2825 -> [w3008]
          tunnel: w2824 -> [w3007]
          tunnel: w2821 -> [w3006]
          shift-right: [w3002] -> _
          shift-left: i16 0 ("StimIndice_Next") -> [w3005]
          shift-right: [w3003] -> _
          shift-left: 0 -> [w3004]
          i -> [w3024]
          stop <- w3040 stop-if-true
          n1416 = Equal To 0?(x=w3024) -> (x = 0?=w3028:bool)
          n1417 = Wait (ms)(milliseconds to wait=u32 0) -> ()  [unwired: 1 out]
          n1418 = call "Act_Pointer_RT.vi"("First Iteration"=w3028, "Handle In"=w3038, "Display Blocksize In"=w3036, "Buffer Size"=w3033, "Old Total Displayed"=w3035, "Old Total Buffered"=w3039) -> ("Data Ready"=w3037:bool, "New Total Buffered"=w3032:i64)  [unwired: 1 in, 2 out]
          n1419 = case shown="True" w3037 {
            tunnel: w3036 -> [w3049 w3084]
            tunnel: w3035 -> [w3050 w3104]
            tunnel: [w3050 w3103] -> w3034
            tunnel: w3033 -> [_ w3097]
            tunnel: w3032 -> [_ w3102]
            tunnel: w3031 -> [_ w3101]
            tunnel: [w3049 w3100] -> w3030
            tunnel: w3027 -> [_ w3099]
            tunnel: w3026 -> [w3048 w3098]
            tunnel: [w3048 w3083] -> w3025
            tunnel: w3023 -> [w3043 w3092]
            tunnel: [w3043 w3091] -> w3018
            tunnel: w3016 -> [w3046 w3082]
            tunnel: w3015 -> [w3047 w3081]
            tunnel: [w3047 w3078] -> w3014
            tunnel: [w3046 w3080] -> w3013
            tunnel: w3012 -> [w3045 w3076]
            tunnel: [w3045 w3075] -> w3011
            tunnel: w3010 -> [w3044 w3074]
            tunnel: [w3044 w3073] -> w3009
            tunnel: w3008 -> [_ w3069]
            tunnel: w3007 -> [_ w3070]
            tunnel: w3006 -> [_ w3065]
            tunnel: [w3041 w3064] -> w3002
            tunnel: w3005 -> [w3041 w3059]
            tunnel: w3004 -> [w3042 w3063]
            tunnel: [w3042 w3062] -> w3003
            frame False {
              n1420 = Wait (ms)(milliseconds to wait=u32 1) -> ()  [unwired: 1 out]
            }
            frame True {
              # "Reset switch"
              # "Max number of stim"
              # "EXG1-EXG2"
              # "R-peak detector"
              # "Generate ECG vector"
              # "Contert to uV"
              # "Only for MK2 Speedmode 4"
              n1421 = Greater?(x=w3084, y=w3092) -> (0:w3093:bool)
              n1422 = call "Act_Ring_RT.vi"("Old Display Index"=w3098, "Buffer Size"=w3097, "Display Blocksize"=w3084, "Nr of Channels"=282, "Serial Data"=w3099) -> ("New Display Index"=w3083:i64, "2D Chan Array"=w3096:i32[][])  [unwired: 1 in, 1 out]
              n1423 = Select(t=w3084, s=w3093, f=w3092) -> (s? t:f=w3091:i64)
              n1424 = Index Array(array=w3096, index (row) #1=256 ("index (row)"), index (row) #2=257 ("index (row)")) -> (element #1=w3090:i32[], element #2=w3089:i32[])  [unwired: 2 in]
              n1425 = To Double Precision Float(number=w3090) -> (double precision float=w3088:dbl[])
              n1426 = To Double Precision Float(number=w3089) -> (double precision float=w3087:dbl[])
              n1427 = Subtract(x=i16 300, y=w3059) -> (x-y=w3057:i16)
              "RemaingStim" <- w3057
              n1428 = Subtract(x=w3088, y=w3087) -> (x-y=w3086:dbl[])
              n1429 = Divide(x=w3086, y=8192.0) -> (x/y=w3061:dbl[])
              n1430 = call "Act_Screen_RT.vi"("Max/Min Display Blocksize"=w3101, "New Total Buffered"=w3102, "Old Display Blocksize"=w3084, "Old Total Displayed"=w3104) -> ("New Display Blocksize"=w3100:i64, "New Total Displayed"=w3103:i64)  [unwired: 3 in, 3 out]
              n1431 = Greater?(x=w3057, y=i16 0) -> (0:w3052:bool)
              n1432 = Not(x=w3052) -> (.not. x?=w3053:bool)
              n1433 = case shown="True" w3053 {
                frame False {
                }
                frame True {
                  n1434 = property on="Task OFF/ON" class="Bool (strict)"("Value"=FALSE ("Task OFF/ON")) -> ()  [unwired: 2 in, 2 out]
                }
              }
              n1435 = Array Size(array=w3061) -> (size(s)=w3060:i32)
              n1436 = call "GenerateECGvector_V2.vi"("Position_ECG_vector"=w3082, "ECG_vector"=w3081, "cooldown In"=w3076, "EXG1-EXG2 current block"=w3061) -> ("Position_ECG_vector_OUT"=w3080:i32, "ECG_vector_OUT"=w3078:dbl[], "cooldown out"=w3077:i64)  [unwired: 5 in]
              n1437 = Multiply(x=w3070, y="R-peak Threshold adjust") -> (x*y=w3072:dbl)
              n1438 = And(x="Task OFF/ON", y=w3052) -> (x .and. y?=w3054:bool)
              n1439 = call "R-peak_detection_V2.vi"("Cooldown in"=w3077, "Threshold"=w3072, "ECG_vector"=w3078) -> ("Cooldown out"=w3075:i64, "Rpeak_detected"=w3068:bool)  [unwired: 7 in]
              n1440 = case shown="True" w3054 {
                tunnel: w3068 -> [_ w3119]
                tunnel: w3074 -> [w3108 w3118]
                tunnel: [w3108 w3116] -> w3073
                tunnel: w3069 -> [_ w3115]
                tunnel: "Condition" -> [_ w3120]
                tunnel: "Bloc" -> [_ w3117]
                tunnel: w3065 -> [_ w3114]
                tunnel: [w3106 w3113] -> w3064
                tunnel: w3059 -> [w3106 w3112]
                tunnel: w3063 -> [w3107 w3111]
                tunnel: [w3107 w3110] -> w3062
                tunnel: w3060 -> [_ w3109]
                frame False {
                }
                frame True {
                  n1441 = case shown="0, Default" w3120 {
                    tunnel: w3119 -> [w3129 _]
                    tunnel: w3118 -> [w3128 w3139]
                    tunnel: w3117 -> [w3126 w3138]
                    tunnel: [w3123 w3137] -> w3116
                    tunnel: w3115 -> [w3125 w3136]
                    tunnel: w3114 -> [w3124 w3135]
                    tunnel: [w3122 w3134] -> w3113
                    tunnel: w3112 -> [w3127 w3133]
                    tunnel: w3111 -> [w3121 w3132]
                    tunnel: [w3121 w3130] -> w3110
                    tunnel: w3109 -> [_ w3131]
                    frame 0, Default {
                      # "Synch"
                      n1442 = call "Task_code_SYNCH.vi"("SoundWave"=w3125, "CardioSynchExperimentalMatrix"=w3124, "StimIndice"=w3127, "Bloc"=w3126, "TriggerPort"=w3128, "Rpeak_detected"=w3129) -> ("StimIndice_Next"=w3122:i16, "TriggerPort"=w3123:refnum<visa-resource-name>)  [unwired: 4 in]
                    }
                    frame 1 {
                      # "Asynch"
                      n1443 = call "Task_code_ASYNCH.vi"("CurrentBufferSize"=w3131, "SoundWave"=w3136, "CardioSynchExperimentalMatrix"=w3135, "StimIndice"=w3133, "Bloc"=w3138, "TriggerPort"=w3139, "AsynchTimeIN"=w3132) -> ("StimIndice_Next"=w3134:i16, "TriggerPort"=w3137:refnum<visa-resource-name>, "AsynchTimeOUT"=w3130:i32)  [unwired: 2 in]
                    }
                  }
                }
              }
            }
          }
          n1444 = Select(t=i64 0, s="Reset", f=w3018) -> (s? t:f=w3017:i64)
          n1445 = Quotient & Remainder(x=w3017, y=i64 577) -> (floor(x/y)=→"Max RT Loop Block (ms)":i64)  [unwired: 1 out]
          n1446 = global read "StopThreads.glb" "StopThreads"() -> (w3040:bool)
        }
        n1447 = while {
          shift-left: FALSE ("LoBatWarning") -> [w3269]
          shift-right: [w3268] -> _
          stop <- w3267 stop-if-true
          n1448 = Wait (ms)(milliseconds to wait=u32 300) -> ()  [unwired: 1 out]
          n1449 = case shown="True" w3269 {
            tunnel: [w3271 w3272] -> w3268
            frame False {
              n1450 = global read "LoBatWarning.glb" "LoBatWarning"() -> (w3271:bool)
            }
            frame True {
              n1451 = call "LoBatWarning.vi"() -> ("Ready"=w3273:bool)  [unwired: 1 out]
              n1452 = Not(x=w3273) -> (.not. x?=w3272:bool)
            }
          }
          n1453 = global read "StopThreads.glb" "StopThreads"() -> (w3267:bool)
        }
        n1454 = while {
          shift-left: FALSE ("LoBatWarning") -> [w3227]
          shift-right: [w3226] -> _
          stop <- w3225 stop-if-true
          n1455 = Wait (ms)(milliseconds to wait=u32 300) -> ()  [unwired: 1 out]
          n1456 = case shown="True" w3227 {
            tunnel: [w3229 w3230] -> w3226
            frame False {
              n1457 = global read "JazzLoBatWarning.glb" "JazzLoBatWarning"() -> (w3229:bool)
            }
            frame True {
              n1458 = call "JazzLoBatWarning.vi"() -> ("Ready"=w3231:bool)  [unwired: 1 out]
              n1459 = Not(x=w3231) -> (.not. x?=w3230:bool)
            }
          }
          n1460 = global read "StopThreads.glb" "StopThreads"() -> (w3225:bool)
        }
        n1461 = while {
          tunnel: "LocalPort" -> [w3249]
          stop <- w3247 stop-if-true
          n1462 = global read "TCPidentification.glb" "TCP cluster"() -> (w3252:T11)
          n1463 = Wait (ms)(milliseconds to wait=u32 100) -> ()  [unwired: 1 out]
          n1464 = Unbundle By Name(w3252) -> ("remote port"=w3251:u16)
          n1465 = Equal To 0?(x=w3251) -> (x = 0?=w3248:bool)
          "TCP Listening" <- w3248
          n1466 = case shown="True" w3248 {
            tunnel: w3249 -> [_ w3253]
            frame False {
            }
            frame True {
              w3254 = 1000  # timeout ms
              n1467 = call <vilib>:"TCP Listen.vi"("timeout ms (wait forever: -1)"=w3254, "port"=w3253) -> ("remote port"=w3255:u16, "remote address"=w3257:string, "connection ID"=w3258:refnum<k5>)  [unwired: 2 in, 5 out]
              n1468 = Bundle("connection ID"=w3258, "remote address"=w3257, "remote port"=w3255) -> (w3256:T11)  [unwired: 1 out]
              n1469 = global write "TCPidentification.glb" "TCP cluster"(w3256) -> ()
            }
          }
          n1470 = global read "StopThreads.glb" "StopThreads"() -> (w3247:bool)
        }
        n1471 = while {
          stop <- w3140 stop-if-true
          n1472 = case shown="True" "UploadMaps" {
            tunnel: [w3142 w3145] -> w3140
            frame False {
              n1473 = Wait (ms)(milliseconds to wait=u32 300) -> ()  [unwired: 1 out]
              n1474 = global read "StopThreads.glb" "StopThreads"() -> (w3142:bool)
            }
            frame True {
              n1475 = local read "Server ID"() -> (w3144:string)
              n1476 = Hexadecimal String To Number(string=w3144) -> (number=w3147:u32)  [unwired: 2 in, 1 out]
              n1477 = call <vilib>:"OpenHandle.vi"() -> ("client handle out"=w3151:T18, "error out"=w3150:errorcluster)  [unwired: 14 in]
              n1478 = Number To Decimal String(number=w3147) -> (decimal integer string=w3146:string)  [unwired: 1 in]
              n1479 = while {
                shift-right: [w3185] -> w3148
                shift-left: w3151 -> [w3187]
                shift-right: [w3154] -> w3149
                shift-left: w3150 -> [w3186]
                shift-right: [w3184] -> _
                shift-left: w3146 -> [w3183]
                tunnel: [w3156] -> w3145
                tunnel: w3144 -> [w3160]
                stop <- w3157 stop-if-true
                w3171 = FALSE ("element")
                w3176 = "https://biosemi.nl/offsetmonitor/input.php"  # url
                n1480 = Equal?(x=w3160, y="?") -> (x = y?=w3166:bool)
                n1481 = Wait (ms)(milliseconds to wait=u32 1000) -> ()  [unwired: 1 out]
                n1482 = case shown="True" w3166 {
                  tunnel: w3186 -> [w3200 w3211]
                  tunnel: [w3200 w3209] -> w3165
                  tunnel: [w3199 w3208] -> w3184
                  tunnel: w3183 -> [w3199 _]
                  tunnel: w3187 -> [w3198 w3207]
                  tunnel: [w3198 w3206] -> w3161
                  frame False {
                  }
                  frame True {
                    n1483 = property class="App"(error in=w3211) -> (error out=w3210:errorcluster, "Application:Kind"=w3212:T3)  [unwired: 1 in, 1 out]
                    n1484 = Current VI's Path() -> (path=w3204:path)
                    n1485 = Equal?(x=w3212, y=T3."Run Time System") -> (x = y?=w3202:bool)
                    n1486 = Strip Path(path=w3204) -> (stripped path=w3203:path)  [unwired: 1 out]
                    n1487 = call <vilib>:"Application Directory.vi"() -> ("Application Directory"=w3205:path)
                    n1488 = Select(t=w3205, s=w3202, f=w3203) -> (s? t:f=w3201:path)
                    n1489 = call "Get_ID.vi"("error in (no error)"=w3210, "Filepath"=w3201, "client handle in"=w3207) -> ("error out"=w3209:errorcluster, "ID (decimal)"=w3208:string, "client handle out"=w3206:T18)
                  }
                }
                n1490 = global read "Data.glb" "Data"() -> (w3177:dbl[])
                n1491 = for {
                  N: 129 -> [_]
                  shift-right: [w3222] -> w3182
                  shift-left: "" -> [w3214]
                  tunnel: w3177 -> [w3217] mode=indexing
                  i -> [w3218]
                  n1492 = Absolute Value(x=w3217) -> (abs(x)=w3215:dbl)
                  n1493 = To Unsigned Byte Integer(number=w3215) -> (unsigned 8bit integer=w3216:u8)
                  n1494 = Number To Decimal String(number=w3218) -> (decimal integer string=w3220:string)  [unwired: 1 in]
                  n1495 = Number To Decimal String(number=w3216) -> (decimal integer string=w3224:string)  [unwired: 1 in]
                  n1496 = Concatenate Strings(w3214, "c" ("string"), w3220, "=" ("string"), w3224, "&" ("string")) -> (w3222:string)
                }
                n1497 = Decimal String To Number(string=w3184) -> (number=w3164:i32)  [unwired: 2 in, 1 out]
                n1498 = Concatenate Strings("id=" ("string"), w3184, "&" ("string"), w3182) -> (w3175:string)
                n1499 = Number To Hexadecimal String(1:i16 4 ("width (-)"), 2:w3164) -> (0:→"Server ID":string)
                n1500 = call-poly <vilib>:"POST.vi"("client handle"=w3161, "url"=w3176, "buffer"=w3175, "error in (no error)"=w3165) -> ("client handle out"=w3185:T18, "body"=w3172:string, "error out"=w3170:errorcluster)  [unwired: 8 in, 1 out]
                n1501 = Match Pattern(string=w3172, regular expression="Database updated.") -> (offset past match=w3173:i32)  [unwired: 1 in, 3 out]
                n1502 = Less Than 0?(x=w3173) -> (x < 0?=w3169:bool)
                n1503 = Build Array(w3171, w3171, w3171, w3171, w3169) -> (w3168:bool[])
                n1504 = call "Act_Error_7000.vi"("Error Code In"=w3168, "error in (no error)"=w3170) -> ("[user-defined descriptions]"=w3152:string[], "[user-defined codes]"=w3153:i32[], "error out"=w3155:errorcluster)
                n1505 = Unbundle By Name(w3155) -> ("status"=w3159:bool)
                n1506 = case shown="True" w3159 {
                  selector: w3159 -> [_ w3196]
                  tunnel: [w3190 w3196] -> w3158
                  tunnel: w3155 -> [w3189 w3195]
                  tunnel: [w3189 w3194] -> w3154
                  tunnel: w3153 -> [_ w3193]
                  tunnel: w3152 -> [_ w3192]
                  frame False {
                    n1507 = local read "UploadMaps"() -> (w3191:bool)
                    n1508 = Not(x=w3191) -> (.not. x?=w3190:bool)
                  }
                  frame True {
                    n1509 = Not(x=w3196) -> (.not. x?=w3197:bool)
                    n1510 = local write "UploadMaps"(w3197) -> ()
                    n1511 = call <vilib>:"General Error Handler.vi"("[user-defined codes]"=w3193, "[user-defined descriptions]"=w3192, "error in (no error)"=w3195) -> ("error out"=w3194:errorcluster)  [unwired: 2 in, 10 out]
                  }
                }
                n1512 = global read "StopThreads.glb" "StopThreads"() -> (w3156:bool)
                n1513 = Or(x=w3158, y=w3156) -> (x .or. y?=w3157:bool)
              }
              n1514 = call <vilib>:"CloseHandle.vi"("client handle"=w3148, "error in (no error)"=w3149) -> ()  [unwired: 13 in, 1 out]
            }
          }
        }
        n1515 = VISA Close(VISA resource name=w2822) -> ()  [unwired: 1 in, 1 out]
        n1516 = Unbundle By Name(w2979) -> ("Spec Labels"=w2978:string[])
        n1517 = Scale By Power Of 2(n=i16 20, x=1.0) -> (x*2^n=w2956:dbl)
        n1518 = while {
          shift-left: w2846 -> [w3467]
          shift-right: [w3466] -> _
          shift-left: w2944 -> [w3470]
          shift-right: [w3469] -> _
          shift-left: w2992 -> [w3435]
          shift-right: [w3476] -> w2991
          shift-left: w2874 -> [w3482]
          shift-right: [w3481] -> _
          shift-left: w2977 -> [w3485]
          shift-right: [w3486] -> _
          tunnel: w2978 -> [w3487]
          tunnel: w2931 -> [w3289]
          tunnel: w2891 -> [w3342]
          shift-left: w2985 -> [w3458]
          shift-right: [w3488] -> _
          shift-left: w2990 -> [w3405]
          shift-right: [w3472] -> _
          tunnel: w2878 -> [w3287]
          shift-left: w2996 -> [w3480]
          shift-right: [w3489] -> w2994
          shift-left: w2997 -> [w3490]
          shift-right: [w3491] -> w2927
          shift-left: w2993 -> [w3434]
          shift-right: [w3477] -> w2998
          tunnel: w2943 -> [w3465]
          tunnel: w2831 -> [w3475]
          shift-left: w2831 -> [w3392]
          shift-right: [w3373] -> _
          shift-left: w2847 -> [w3377]
          shift-right: [w3382] -> _
          shift-left: w2833 -> [w3483]
          shift-right: [w3495] -> _
          shift-left: w2833 -> [w3484]
          shift-right: [w3381] -> _
          tunnel: w2836 -> [w3376]
          tunnel: w2838 -> [w3374]
          shift-right: [w3464] -> _
          shift-left: w2846 -> [w3463]
          shift-right: [w3461] -> w2983
          shift-left: w2984 -> [w3462]
          tunnel: w2945 -> [w3412]
          shift-right: [w3460] -> _
          shift-left: w2947 -> [w3457]
          shift-right: [w3459] -> _
          shift-left: w2986 -> [w3360]
          tunnel: [w3307] -> w2982
          shift-right: [w3455] -> _
          shift-left: w2977 -> [w3456]
          shift-right: [w3452] -> _
          shift-left: w2846 -> [w3453]
          shift-right: [w3450] -> w2975
          shift-left: w2976 -> [w3451]
          tunnel: w2831 -> [w3387]
          tunnel: w2834 -> [w3386]
          tunnel: w2878 -> [w3346]
          shift-right: [w3438] -> w2972
          shift-left: w2973 -> [w3439]
          shift-right: [w3436] -> _
          shift-left: w2846 -> [w3437]
          shift-right: [w3429] -> _
          shift-left: w2854 -> [w3431]
          shift-right: [w3428] -> _
          shift-left: w2854 -> [w3430]
          shift-right: [w3427] -> _
          shift-left: FALSE ("fill?(F)") -> [w3424]
          shift-right: [w3415] -> _
          shift-left: w2964 -> [w3410]
          shift-right: [w3414] -> _
          shift-left: w2964 -> [w3411]
          shift-right: [w3413] -> _
          shift-left: w2963 -> [w3404]
          shift-right: [w3408] -> _
          shift-left: w2962 -> [w3303]
          tunnel: w2959 -> [w3391]
          tunnel: w2956 -> [w3390]
          tunnel: w2892 -> [w3388]
          tunnel: w2946 -> [w3372]
          tunnel: [w3385] -> w2948
          shift-right: [w3370] -> _
          shift-left: w2941 -> [w3371]
          shift-right: [w3369] -> _
          shift-left: w2837 -> [w3368]
          shift-right: [w3366] -> _
          shift-left: w2940 -> [w3367]
          tunnel: w2933 -> [w3358]
          tunnel: w2918 -> [w3357]
          tunnel: w2902 -> [w3356]
          tunnel: [w3350] -> w2925
          tunnel: [w3352] -> w2924
          tunnel: w2903 -> [w3351]
          tunnel: w2899 -> [_]
          tunnel: w2894 -> [w3349]
          shift-right: [w3347] -> _
          shift-left: w2893 -> [w3348]
          tunnel: w2890 -> [w3341]
          shift-right: [w3345] -> w2879
          shift-left: w2889 -> [w3337]
          tunnel: w2887 -> [w3336]
          shift-right: [w3331] -> w2883
          shift-left: w2885 -> [w3332]
          shift-right: [w3329] -> _
          shift-left: w2884 -> [w3330]
          shift-right: [w3313] -> _
          shift-left: w2858 -> [w3278]
          tunnel: [w3314] -> w2861
          tunnel: w2835 -> [w3312]
          tunnel: w2857 -> [w3304]
          shift-right: [w3302] -> _
          shift-left: T2."Monopolar" ("Charts/Graphs") -> [w3282]
          shift-right: [w3300] -> _
          shift-left: w2855 -> [w3301]
          tunnel: w2855 -> [w3299]
          shift-right: [w3298] -> _
          shift-left: w2848 -> [w3297]
          shift-right: [w3293] -> _
          shift-left: w2846 -> [w3294]
          shift-right: [w3291] -> _
          shift-left: w2845 -> [w3292]
          shift-right: [w3285] -> w2843
          shift-left: w2842 -> [w3284]
          tunnel: w2841 -> [w3283]
          shift-right: [w3275] -> _
          shift-left: w2840 -> [w3276]
          i -> [w3274]
          stop <- w3303 stop-if-true
          w3286 = T2."ERP" ("Charts/Graphs")
          w3409 = i8 4  # Avg
          w3478 = i8 3  # EOF
          w3492 = i8 2  # Save
          w3493 = i8 1  # Display
          w3494 = i8 0  # Wait
          (unwired) 32
          # "Start Output Trigger 13"
          # "Do not overwrite output trigger 16\n(used to switch receiver to Jazz)"
          # "Charts/Graphs"
          # "ABR Filter Cluster"
          # "ABR Filter Cluster"
          # "ABR Channel Selection"
          # "ABR Channel Selection"
          # "ABR Filter Reset"
          # "ABR Filter Reset"
          # "Speed/Save Cluster"
          # "Average Total"
          # "Noise Total"
          # "Total ADC Sample/s"
          # "Jazz Channel Selection"
          # "Jazz Filter Reset"
          # "Jazz Channel Selection"
          # "Jazz Filter Reset"
          # "Box"
          # "Box"
          # "File Limit in Byte"
          # "Time Limit"
          # "Number of Files"
          # "Number of Files"
          # "Total Saved in Sec"
          # "Total Saved in Sec"
          # "Markers"
          # "Driver Handle"
          # "Handle"
          # "System Cluster"
          # "Extra Blocksize Check"
          # "Buffer pointer in Byte"
          # "in Mbyte"
          # "Average Cluster"
          # "Tab Control"
          # "Last Call"
          # "Stop next call"
          # "Update Avg"
          # "Average Cluster"
          # "Average Total"
          # "Noise Total"
          # "Decimation Factor"
          # "Ana Filter Reset"
          # "Ana Filter Reset"
          # "Ana Channel Selection"
          # "Charts/Graphs"
          # "Ana Channel Selection"
          # "Acquisition Error"
          # "Second Half"
          # "Aux Channel Selection"
          # "Aux Channel Selection"
          # "Aux DC Reset"
          # "Aux DC Reset"
          # "Save Index"
          # "Bip Channel Selection"
          # "Bip Channel Selection"
          # "Sample Rate"
          # "Mon Channel selection"
          # "Mon Ref Selection"
          # "Mon Channel selection"
          # "Mon Ref Selection"
          # "Bip Filter Reset"
          # "Bip Filter Reset"
          # "Mon Filter Reset"
          # "Mon Filter Reset"
          # "Max/Min Display Blocksize"
          # "Popup Change"
          # "Popups Change"
          # "Max/Min Display Blocksize"
          # "Screen Reset"
          # "Current File in Byte"
          # "Header Lenght in Byte"
          # "Header Lenght in Byte"
          # "Current File in Byte"
          # "Screen Reset"
          # "Sync Error Cluster"
          # "Sync Error Cluster"
          # "Display/Save data until an error occurs,\nor Stop or Start-File button is pressed"
          # "No Incoming Data"
          # "Buffer Pointer"
          # "Buffer pointer"
          # "Speed/Save Cluster"
          # "Start Saving"
          # "New Total Buffered"
          # "Save Array"
          # "Diplay Blocksize"
          # "Display Index"
          # "Display Blocksize"
          # "New Total Displayed"
          # "Total ADC Samples/s"
          # "New Total Buffered"
          # "Buffer Size in I32"
          # "Old Total Displayed"
          # "New Total Buffered"
          # "Display Index"
          # "Old total buffered"
          n1519 = global write "StopThreads.glb" "StopThreads"(w3303) -> ()
          n1520 = Wait (ms)(milliseconds to wait=u32 0) -> ()  [unwired: 1 out]
          n1521 = Less Or Equal?(x=w3392, y=w3387) -> (x <= y?=w3398:bool)
          n1522 = Select(t=w3392, s=w3398, f=w3387) -> (s? t:f=w3393:i64)
          n1523 = Unbundle By Name(w3404) -> ("Valid Sweeps"=w3327:i32, "Rejected Sweeps"=w3325:i32)
          n1524 = Greater Or Equal?(x=w3368, y="RecTimeLimit") -> (x >= y?=w3340:bool)
          n1525 = Multiply(x=w3391, y="FileLimit") -> (x*y=w3343:i64)
          n1526 = global read "TCPidentification.glb" "TCP cluster"() -> (w3355:T11)
          n1527 = Quotient & Remainder(x=w3393, y=w3386) -> (floor(x/y)=w3396:i64)  [unwired: 1 out]
          n1528 = Select(t=T6."Disabled and Grayed Out" ("Disabled"), s="Averaging", f=T6."Enabled" ("Disabled")) -> (s? t:f=w3290:T6)
          n1529 = Bundle(w3387, w3386) -> (w3335:cluster{i64, i64})  [unwired: 1 out]
          n1530 = Less Or Equal To 0?(x=w3396) -> (x <= 0?=w3397:bool)
          n1531 = Unbundle By Name(w3289) -> ("ABR Enabled"=w3288:bool)
          n1532 = Not(x="Pause Saving") -> (.not. x?=w3281:bool)
          n1533 = Select(t=i64 1, s=w3397, f=w3396) -> (s? t:f=w3394:i64)
          n1534 = property on="AvgTrigSel" class="LstBox (strict)"("Disabled"=w3290) -> ()  [unwired: 2 in, 2 out]
          n1535 = property on="AvgTrigLog" class="Ring (strict)"("Disabled"=w3290) -> ()  [unwired: 2 in, 2 out]
          n1536 = property on="AvgSweep" class="DigNum (strict)"("Disabled"=w3290) -> ()  [unwired: 2 in, 2 out]
          n1537 = Unbundle By Name(w3355) -> ("connection ID"=w3350:refnum<k5>, "remote address"=→"Remote Adress":string, "remote port"=w3353:u16)
          "Receive Remote Port" <- w3353
          n1538 = Multiply(x=w3394, y=w3386) -> (x*y=w3375:i64)
          n1539 = local read "Valid Sweeps"() -> (w3326:i32)
          n1540 = Replace Array Subset(array=w3278, new element=w3281, index=12) -> (w3277:bool[])
          n1541 = case shown="False" w3288 {
            tunnel: w3290 -> [w3496 _]
            frame False {
              n1542 = property on="AvgLP" class="Bool (strict)"("Disabled"=w3496) -> ()  [unwired: 2 in, 2 out]
              n1543 = property on="AvgLPfreq" class="DigNum (strict)"("Disabled"=w3496) -> ()  [unwired: 2 in, 2 out]
              n1544 = property on="AvgHP" class="Bool (strict)"("Disabled"=w3496) -> ()  [unwired: 2 in, 2 out]
              n1545 = property on="AvgHPfreq" class="DigNum (strict)"("Disabled"=w3496) -> ()  [unwired: 2 in, 2 out]
              n1546 = property on="MonFreeAvg1" class="LstBox (strict)"("Disabled"=w3496) -> ()  [unwired: 2 in, 2 out]
              n1547 = property on="RefFreeAvg1" class="LstBox (strict)"("Disabled"=w3496) -> ()  [unwired: 2 in, 2 out]
              n1548 = property on="MonFreeAvg2" class="LstBox (strict)"("Disabled"=w3496) -> ()  [unwired: 2 in, 2 out]
              n1549 = property on="RefFreeAvg2" class="LstBox (strict)"("Disabled"=w3496) -> ()  [unwired: 2 in, 2 out]
            }
            frame True {
            }
          }
          n1550 = Add(x=w3434, y=w3341) -> (x+y=w3379:i64)
          n1551 = Equal To 0?(x=w3274) -> (x = 0?=w3378:bool)
          n1552 = local read "Charts/Graphs"() -> (w3406:T2)
          n1553 = Greater?(x=w3327, y=w3326) -> (0:w3323:bool)
          n1554 = Not Equal To 0?(x=w3353) -> (x != 0?=w3352:bool)
          "TCP Connected" <- w3352
          n1555 = local read "Rejected Sweeps"() -> (w3324:i32)
          n1556 = call "Act_Pointer.vi"("First Iteration"=w3378, "Handle In"=w3312, "Display Blocksize In"=w3375, "Buffer Size"=w3376, "Old Total Displayed"=w3483, "Old Total Buffered"=w3484) -> ("Data Ready"=w3444:bool, "No Incoming Data"=w3380:bool, "Buffer Pointer"=w3310:i64, "New Total Buffered"=w3381:i64, "Handle Out"=w3311:i64)
          n1557 = Greater?(x=w3379, y=w3343) -> (0:w3339:bool)
          n1558 = Greater?(x=w3325, y=w3324) -> (0:w3322:bool)
          n1559 = Not Equal?(x=w3282, y=w3286) -> (x != y?=w3407:bool)
          n1560 = Greater Or Equal?(x=w3457, y=w3342) -> (x >= y?=w3361:bool)
          n1561 = case shown="True" w3287 {
            tunnel: "Pause Saving" -> [_ w3506]
            frame False {
            }
            frame True {
              n1562 = property on="Start Saving" class="Bool (strict)"() -> ("Colors [4]"=w3515:cluster{u32, u32}[])  [unwired: 2 in, 2 out]
              n1563 = Select(t=u32 16711680, s=w3506, f=u32 6618880) -> (s? t:f=w3510:u32)
              n1564 = Select(t="Not Saving" ("f"), s=w3506, f="Saving" ("Boolean Text.Text")) -> (s? t:f=w3518:string)
              n1565 = Select(t=u32 16777215, s=w3506, f=u32 0) -> (s? t:f=w3505:u32)
              n1566 = Index Array(array=w3515) -> (element #1=w3509:cluster{u32, u32}, element #2=w3512:cluster{u32, u32})  [unwired: 2 in]
              n1567 = Unbundle(w3512) -> (w3511:u32)  [unwired: 1 out]
              n1568 = Bundle(w3510, w3511) -> (w3513:cluster{u32, u32})  [unwired: 1 out]
              n1569 = Build Array(w3509, w3513) -> (w3514:cluster{u32, u32}[])
              n1570 = property on="Start Saving" class="Bool (strict)"("Boolean Text.Text"=w3518, "Colors [4]"=w3514, "Boolean Text.Text Colors:Text Color"=w3505) -> ()  [unwired: 2 in, 2 out]
            }
          }
          n1571 = Equal?(x=w3286, y=w3406) -> (x = y?=w3320:bool)
          n1572 = Or(x=w3323, y=w3322) -> (x .or. y?=w3321:bool)
          n1573 = Or(x=w3340, y=w3339) -> (x .or. y?=w3338:bool)
          n1574 = Exclusive Or(1:w3360, 2:w3361) -> (0:w3359:bool)
          n1575 = And(x=w3321, y=w3320) -> (x .and. y?=w3319:bool)
          n1576 = And(x=w3407, y=w3320) -> (x .and. y?=w3315:bool)
          n1577 = Not And(1:w3359, 2:w3287) -> (0:w3362:bool)
          n1578 = Not And(1:w3287, 2:w3338) -> (0:w3449:bool)
          n1579 = local write "Start"(TRUE ("Start")) -> ()
          n1580 = Select(t=w3493, s=w3444, f=w3494) -> (s? t:f=w3364:i8)
          n1581 = Compound Arithmetic op=OR(w3319, w3303, w3315) -> (w3318:bool)
          n1582 = Not Or(1:"Pause Saving", 2:w3362) -> (0:→"Write BDF":bool)
          n1583 = Not And(1:"Averaging", 2:w3318) -> (0:w3317:bool)
          n1584 = Select(t=w3364, s=w3317, f=w3409) -> (s? t:f=w3363:i8)
          n1585 = Select(t=w3363, s=w3362, f=w3492) -> (s? t:f=w3474:i8)
          n1586 = Select(t=w3474, s=w3449, f=w3478) -> (s? t:f=w3365:i8)
          n1587 = property on="Trigger Chart" class="WFChart (strict)"() -> ("X Scale.Range:Maximum"=w3416:dbl)  [unwired: 2 in, 2 out]
          n1588 = property on="Mon Chart" class="WFChart (strict)"() -> ("X Scale.Range:Maximum"=w3473:dbl)  [unwired: 2 in, 2 out]
          n1589 = property on="Bip Chart" class="WFChart (strict)"() -> ("X Scale.Range:Maximum"=w3471:dbl)  [unwired: 2 in, 2 out]
          n1590 = property on="ABR Chart" class="WFChart (strict)"() -> ("XScale.Maximum"=w3296:dbl)  [unwired: 2 in, 2 out]
          n1591 = property on="Aux Chart" class="WFChart (strict)"() -> ("X Scale.Range:Maximum"=w3454:dbl)  [unwired: 2 in, 2 out]
          n1592 = property on="Jazz Chart" class="WFChart (strict)"() -> ("XScale.Maximum"=w3334:dbl)  [unwired: 2 in, 2 out]
          n1593 = property on="Ana Chart" class="WFChart (strict)"() -> ("X Scale.Range:Maximum"=w3441:dbl)  [unwired: 2 in, 2 out]
          n1594 = case shown="1" w3365 {
            tunnel: [w3675 w4161 w4786 w4938 w5068] -> w3495
            tunnel: [w3641 w3764 w4754 w4911 w5031] -> w3382
            tunnel: w3376 -> [_ w4048 _ _ _]
            tunnel: w3483 -> [w3675 w4159 w4786 w4938 w5068]
            tunnel: w3375 -> [w3673 w4047 w4714 w4937 w5067]
            tunnel: w3381 -> [_ w4167 _ _ _]
            tunnel: [w3673 w3735 w4714 w4937 w5067] -> w3373
            tunnel: w3342 -> [_ _ w4728 w4888 _]
            tunnel: [w3653 w4099 w4782 w4904 w5035] -> w3491
            tunnel: w3490 -> [w3652 w4009 w4744 w4908 w5035]
            tunnel: [w3672 w4002 w4730 w4906 w5034] -> w3489
            tunnel: w3480 -> [w3672 w4002 w4747 w4907 w5034]
            tunnel: [w3671 w4163 w4785 w4936 w5066] -> w3472
            tunnel: w3405 -> [w3671 w3786 w4785 w4936 w5066]
            tunnel: "Pause Saving" -> [_ w3984 w4694 _ _]
            tunnel: [w3670 w4128 w4742 w4935 w5065] -> w3488
            tunnel: w3458 -> [w3670 w3943 w4742 w4935 w5065]
            tunnel: w3475 -> [_ w4160 _ _ _]
            tunnel: w3289 -> [w3654 w3986 w4712 w4926 w5054]
            tunnel: w3487 -> [_ w3766 _ _ _]
            tunnel: [w3669 w3684 w4784 w4934 w5064] -> w3486
            tunnel: w3485 -> [w3669 w4140 w4784 w4934 w5064]
            tunnel: w3482 -> [w3668 w3889 w4783 w4933 w5063]
            tunnel: [w3668 w3887 w4783 w4933 w5063] -> w3481
            tunnel: [w3642 w3939 w4749 w4905 FALSE] -> w3442
            tunnel: w3435 -> [w3666 w4166 w4760 w4892 w5061]
            tunnel: w3434 -> [w3667 w4165 w4775 w4902 w5062]
            tunnel: [w3667 w4165 w4761 w4901 w5062] -> w3477
            tunnel: [w3666 w4166 w4760 w4892 w5061] -> w3476
            tunnel: w3473 -> [_ w3789 _ _ _]
            tunnel: w3335 -> [_ w4158 _ _ _]
            tunnel: w3471 -> [_ w4102 _ _ _]
            tunnel: w3470 -> [w3665 w4061 w4774 w4932 w5060]
            tunnel: [w3665 w4136 w4774 w4932 w5060] -> w3469
            tunnel: w3467 -> [w3664 w4143 w4773 w4931 w5059]
            tunnel: [w3664 w4038 w4773 w4931 w5059] -> w3466
            tunnel: w3465 -> [_ w3681 _ _ w5038]
            tunnel: [w3663 w4034 w4772 w4930 w5058] -> w3464
            tunnel: w3463 -> [w3663 w4115 w4772 w4930 w5058]
            tunnel: w3462 -> [w3662 w4139 w4771 w4929 w5057]
            tunnel: [w3662 w3895 w4771 w4929 w5057] -> w3461
            tunnel: w3412 -> [_ w3944 w4707 _ _]
            tunnel: w3457 -> [w3660 w3942 w4770 w4927 w5055]
            tunnel: w3360 -> [w3661 w4138 w4741 w4928 w5056]
            tunnel: [w3660 w4129 w4770 w4927 w5055] -> w3460
            tunnel: [w3661 w4138 w4743 w4928 w5056] -> w3459
            tunnel: [w3654 w3986 w4712 w4926 w5054] -> w3307
            tunnel: w3287 -> [_ w3919 _ _ _]
            tunnel: w3456 -> [w3659 w4125 w4769 w4925 w5053]
            tunnel: [w3659 w3916 w4769 w4925 w5053] -> w3455
            tunnel: w3454 -> [_ w4103 _ _ _]
            tunnel: [w3658 w4032 w4768 w4924 w5052] -> w3452
            tunnel: w3453 -> [w3658 w4114 w4768 w4924 w5052]
            tunnel: w3451 -> [w3657 w4105 w4767 w4923 w5051]
            tunnel: [w3657 w3914 w4767 w4923 w5051] -> w3450
            tunnel: [w3630 w4103 w4721 w4880 w5007] -> w3448
            tunnel: [w3630 w4102 w4721 w4880 w5007] -> w3447
            tunnel: [w3630 w3789 w4721 w4880 w5007] -> w3446
            tunnel: [FALSE w3775 FALSE FALSE FALSE] -> w3432
            tunnel: [w3655 w4101 w4765 w4922 w5050] -> w3445
            tunnel: [w3655 w3868 w4765 w4922 w5050] -> w3389
            tunnel: w3380 -> [w3642 _ _ _ _]
            tunnel: w3441 -> [_ w4096 _ _ _]
            tunnel: [w3630 w4096 w4721 w4880 w5007] -> w3440
            tunnel: w3439 -> [w3651 w4091 w4764 w4920 w5048]
            tunnel: w3282 -> [w3650 _ w4763 w4919 _]
            tunnel: [w3651 w3816 w4764 w4920 w5048] -> w3438
            tunnel: [w3650 "Charts/Graphs" w4763 w4919 T2."ERP" ("Charts/Graphs")] -> w3302
            tunnel: w3437 -> [w3649 w4030 w4762 w4918 w5047]
            tunnel: [w3649 w4033 w4762 w4918 w5047] -> w3436
            tunnel: w3431 -> [w3648 w3913 w4759 w4917 w5046]
            tunnel: w3430 -> [w3647 w3912 w4758 w4916 w5045]
            tunnel: [w3648 w3977 w4759 w4917 w5046] -> w3425
            tunnel: [w3647 w3976 w4758 w4916 w5045] -> w3426
            tunnel: w3424 -> [_ w4013 _ _ _]
            tunnel: [w3630 w3790 w4721 w4880 w5007] -> w3417
            tunnel: w3416 -> [_ w3790 _ _ _]
            tunnel: w3410 -> [w3645 w4083 w4756 w4914 w5023]
            tunnel: w3411 -> [w3644 w4082 w4755 w4915 w5022]
            tunnel: [w3645 w4081 w4756 w4914 w5023] -> w3415
            tunnel: [w3644 w3906 w4755 w4915 w5022] -> w3414
            tunnel: [w3646 w4079 w4757 w4913 w5016] -> w3413
            tunnel: w3404 -> [w3646 w4075 w4757 w4913 w5017]
            tunnel: "Averaging" -> [_ w4074 _ _ _]
            tunnel: w3388 -> [_ w3868 _ _ _]
            tunnel: w3349 -> [_ w3686 _ _ _]
            tunnel: w3372 -> [w3643 w3707 w4717 w4912 w5032]
            tunnel: [w3643 w3707 w4717 w4912 w5032] -> w3385
            tunnel: w3377 -> [w3641 w4049 w4754 w4911 w5031]
            tunnel: w3374 -> [_ w4046 _ _ _]
            tunnel: w3371 -> [w3640 w4023 w4753 w4910 w5030]
            tunnel: [w3640 w4022 w4753 w4910 w5030] -> w3370
            tunnel: w3368 -> [w3639 w4021 w4746 w4909 w5029]
            tunnel: [w3639 w4021 w4750 w4909 w5029] -> w3369
            tunnel: w3367 -> [w3638 w4020 w4748 w4895 w5028]
            tunnel: [w3638 w4020 w4748 w4903 w5028] -> w3366
            tunnel: w3340 -> [_ _ _ w4900 _]
            tunnel: w3343 -> [_ _ _ w4890 _]
            tunnel: w3358 -> [_ w3980 _ _ _]
            tunnel: w3357 -> [_ w4004 _ _ _]
            tunnel: w3356 -> [_ w4003 _ _ _]
            tunnel: w3352 -> [_ w4006 _ _ _]
            tunnel: w3351 -> [_ w3804 _ _ _]
            tunnel: w3350 -> [_ w4005 _ _ _]
            tunnel: w3348 -> [w3637 w3969 w4734 w4889 w5027]
            tunnel: [w3637 "Box" w4734 w4889 w5027] -> w3347
            tunnel: w3346 -> [_ w3963 _ _ _]
            tunnel: [w3636 w3949 w4732 w4886 w5026] -> w3345
            tunnel: w3337 -> [w3636 _ w4732 w4886 w5026]
            tunnel: w3336 -> [_ w3950 _ _ _]
            tunnel: [w3630 w3947 w4721 w4880 w5007] -> w3333
            tunnel: w3334 -> [_ w3947 _ _ _]
            tunnel: w3332 -> [w3634 w3933 w4724 w4884 w5024]
            tunnel: [w3634 w3811 w4724 w4884 w5024] -> w3331
            tunnel: w3330 -> [w3635 w3922 w4725 w4885 w5025]
            tunnel: [w3635 w3930 w4725 w4885 w5025] -> w3329
            tunnel: [w3633 w3678 w4711 w4883 w5010] -> w3313
            tunnel: w3277 -> [w3633 w3867 w4711 w4883 w5010]
            tunnel: w3304 -> [_ w3854 w4695 _ _]
            tunnel: w3301 -> [w3632 w3849 w4723 w4882 w5009]
            tunnel: [w3632 w3846 w4723 w4882 w5009] -> w3300
            tunnel: w3299 -> [_ w3845 _ _ _]
            tunnel: [w3631 w3819 w4722 w4881 w5008] -> w3298
            tunnel: w3297 -> [w3631 w3820 w4722 w4881 w5008]
            tunnel: [w3629 w3791 w4720 w4879 w5006] -> w3293
            tunnel: w3296 -> [_ w3788 _ _ _]
            tunnel: [w3630 w3788 w4721 w4880 w5007] -> w3295
            tunnel: w3294 -> [w3629 w3784 w4720 w4879 w5006]
            tunnel: w3292 -> [w3628 w3782 w4719 w4878 w5005]
            tunnel: [w3628 "AbrChannels" w4719 w4878 w5005] -> w3291
            tunnel: [w3626 w3737 w4718 w4877 w5003] -> w3285
            tunnel: w3284 -> [w3626 w3695 w4718 w4877 w5003]
            tunnel: w3283 -> [_ w3708 _ _ _]
            tunnel: w3276 -> [w3625 w3677 w4706 w4876 w5002]
            tunnel: [w3625 w3677 w4694 w4876 w5002] -> w3275
            frame 0, Default {
              w3630 = 0.0 ("XScale.Maximum")
              w3655 = i64 0 ("Prop Screen Minimum")
              # "Wait"
              n1595 = Wait (ms)(milliseconds to wait=u32 10) -> ()  [unwired: 1 out]
              n1596 = Build Array(w3642) -> (w3627:bool[])
              n1597 = call "Act_Error_5000.vi"("Error Code In"=w3627, "error in (no error)"=w3652) -> ("error out"=w3653:errorcluster)  [unwired: 2 out]
            }
            frame 1 {
              w3742 = u32 16711718
              w3750 = i8 9  # ABR
              w3839 = 12.0  # FontSize
              w3859 = T6."Disabled and Grayed Out" ("Disabled")
              w3871 = TRUE  # Aquiring?
              w3941 = FALSE  # No Error
              w4162 = i8 1  # End of Screen
              # "Speedmode"
              # "Reset ABR Labels"
              # "ABR Filter Reset"
              # "Screen X-axis reset"
              # "Screen Duration"
              # "RespSwitch"
              # "Jazz LoBatt"
              # "Reset Jazz Labels"
              # "JazzOn"
              # "<-- Mark2"
              # "First Call"
              # "<-- ADC Rate"
              # "<-- ADC Channels"
              # "Markers"
              # "Reset Aux Labels"
              # "Reset Aux Labels"
              # "Screen Duration"
              # "Busy Averaging"
              # "Start Averaging"
              # "Downsample Correction"
              # "Ana Filter Reset"
              # "Reset Ana Labels"
              # "Error Code"
              # "<-- Speed Mode"
              # "8 Aux Channels"
              # "First Call"
              # "<-- Center Traces"
              # "<-- Charts Tab"
              # "Decimation Factor"
              # "First Call"
              # "Reset Bip Labels"
              # "Reset Bip Labels"
              # "Busy Saving"
              # "Low Batt"
              # "Second Half"
              # "New Save Buffer"
              # "New Index"
              # "<-- First Call"
              # "Bip Filter Reset"
              # "First Call"
              # "Reset Mon Labels"
              # "Reset Mon Filter"
              # "Sample Rate"
              # "Mon Filter Reset"
              # "Screen X-axis reset"
              # "Popup Change"
              # "Screen DC Reset"
              # "Display"
              # "Status Channel"
              # "Sync Errors"
              # "Buffer Size"
              # "Display Blocksize"
              # "New Display Index"
              # "Old Total Displayed"
              n1598 = property class="VI"() -> ("Front Panel.PanelBounds"=w3851:T28)  [unwired: 2 in, 2 out]
              n1599 = Unbundle By Name(w3707) -> ("ElecGain"=w3869:i8, "RespSwitch"=w3739:i8, "PopupKiller"=w3891:i8, "BreathBelt"=w3691:i8, "ABRlocation"=w3709:i8, "SEMGswap"=w3724:i8)
              n1600 = Unbundle By Name(w3986) -> ("PauseOff"=w3988:i32, "PauseOn"=w3987:i32)
              n1601 = Unbundle By Name(w3851) -> ("Left"=w3847:i16, "Top"=w3848:i16, "Right"=w3853:i16, "Bottom"=w3852:i16)
              n1602 = property on="GSR1 pos" class="Bool (strict)"() -> ("Disabled"=w3956:u8)  [unwired: 2 in, 2 out]
              n1603 = property on="GSR2 pos" class="Bool (strict)"() -> ("Disabled"=w3957:u8)  [unwired: 2 in, 2 out]
              n1604 = Bundle("PauseOff"=w3988, "PauseOn"=w3987) -> (w3985:cluster{"PauseOff":i32, "PauseOn":i32})  [unwired: 1 out]
              n1605 = Subtract(x=w3853, y=w3847) -> (x-y=w3850:i16)
              n1606 = Subtract(x=w3852, y=w3848) -> (x-y=w3819:i16)
              n1607 = Not Equal?(x=w3819, y=w3820) -> (x != y?=w3777:bool)
              n1608 = Unbundle By Name(w3845) -> ("Clear Block"=w3823:dbl, "Screen Ratio"=w3842:dbl, "Y1"=w3835:dbl, "Y2"=w3834:dbl, "Y3"=w3833:dbl, "YT1"=w3832:dbl, "YT2"=w3831:dbl, "YT3"=w3830:dbl)
              n1609 = Equal To 0?(x=w3956) -> (x = 0?=w3711:bool)
              n1610 = Equal To 0?(x=w3957) -> (x = 0?=w3710:bool)
              n1611 = To Double Precision Float(number=w3850) -> (double precision float=w3843:dbl)
              n1612 = To Double Precision Float(number=w3819) -> (double precision float=w3841:dbl)
              n1613 = Divide(x=1200.0 ("y"), y=w3843) -> (x/y=w3806:dbl)
              n1614 = Unbundle By Name(w4075) -> ("Busy Averaging"=w4071:bool)
              n1615 = Divide(x=w3841, y=650.0) -> (x/y=w3821:dbl)
              n1616 = Unbundle By Name(w3986) -> ("Mark2"=w3946:bool, "GSR16Hz"=w3945:bool, "Speed Mode"=w3706:i8, "ADC Rate"=w3937:i32, "ADC Channels"=w3763:i32, "Decimate Ratio"=w3774:i32, "Mon Channels"=w3722:i32, "Bip Channels"=w3698:i32, "Aux Channels"=w3923:i32, "Jazz Channels"=w3679:i32, "Ana Channels"=w3680:i32, "Save Subset"=w3997:i8, "Add Sensors"=w3769:bool, "Add Jazz"=w3768:bool, "Add Anas"=w3767:bool, "ABR Enabled"=w3728:bool)
              n1617 = call "Act_Ring_X.vi"("Old Display Index"=w4049, "Buffer Size"=w4048, "Display Blocksize"=w4047, "Nr of Channels"=w3763, "Serial Data"=w4046) -> ("New Display Index"=w3764:i64, "Sync Channnel"=w3761:i32[], "Status Channnel"=w3760:i32[], "2D Chan Array"=w3762:i32[][])
              n1618 = In Range and Coerce(upper limit=i8 13 ("y"), x=w3706, lower limit=i8 4 ("y")) -> (In Range?=w3855:bool)  [unwired: 1 out]
              n1619 = Equal?(x=w3706, y=i8 8) -> (x = y?=w4018:bool)
              n1620 = Not(x=w3855) -> (.not. x?=w3954:bool)
              n1621 = call "SyncCheck.vi"("Speedmode"=w3706, "Satus Chan In"=w3760, "Sync Chan In"=w3761) -> ("Number of Sync Errors"=w3765:i16)
              n1622 = And(x=w3946, y=w3954) -> (x .and. y?=w3953:bool)
              n1623 = Multiply(x=w3839, y=w3821) -> (x*y=w3837:dbl)
              n1624 = Bundle("GsrScale"="GsrScale", "ErgoScale"="ErgoScale", "ErgoLP"="ErgoLP", "RespScale"="RespScale", "PletScale"="PletScale", "TempScale"="TempScale") -> (w4086:T29)  [unwired: 1 out]
              n1625 = Multiply(x=w3806, y=w3842) -> (x*y=w3807:dbl)
              n1626 = Unbundle By Name(w3986) -> ("Mon Channels"=w4012:i32, "Bip Channels"=w4011:i32, "Aux Channels"=w4010:i32, "Jazz Channels"=w3936:i32)
              n1627 = To Word Integer(number=w3837) -> (16bit integer=w3836:i16)
              n1628 = Not Equal?(x=w3706, y=w3750) -> (x != y?=w3749:bool)
              n1629 = Multiply(x=w3823, y=w3821) -> (x*y=w3822:dbl)
              n1630 = Array Size(array=w4105) -> (size(s)=w4109:i32)
              n1631 = Not(x=w4071) -> (.not. x?=w4080:bool)
              n1632 = Not Equal To 0?(x=w3679) -> (x != 0?=w3773:bool)
              n1633 = Multiply(x=w3821, y=w3835) -> (x*y=w3829:dbl)
              n1634 = Multiply(x=w3821, y=w3834) -> (x*y=w3828:dbl)
              n1635 = Multiply(x=w3821, y=w3833) -> (x*y=w3827:dbl)
              n1636 = Multiply(x=w3821, y=w3832) -> (x*y=w3826:dbl)
              n1637 = Multiply(x=w3821, y=w3831) -> (x*y=w3825:dbl)
              n1638 = Multiply(x=w3821, y=w3830) -> (x*y=w3824:dbl)
              n1639 = And(x=w4074, y=w4080) -> (x .and. y?=w4077:bool)
              n1640 = Bundle("Mon Channels"=w4012, "Bip Channels"=w4011, "Aux Channels"=w4010, "Jazz Channels"=w3936) -> (w4007:T30)  [unwired: 1 out]
              n1641 = And(x=w3919, y=w3769) -> (x .and. y?=w3951:bool)
              n1642 = Select(t=T6."Disabled and Grayed Out" ("Disabled"), s=w3951, f=T6."Enabled" ("Disabled")) -> (s? t:f=w4100:T6)
              n1643 = And(x=w3919, y=w3768) -> (x .and. y?=w3910:bool)
              n1644 = And(x=w3919, y=w3767) -> (x .and. y?=w3952:bool)
              n1645 = Bundle By Name(cluster=w3849, "Clear Block"=w3822, "Screen Ratio"=w3807, "Y1"=w3829, "Y2"=w3828, "Y3"=w3827, "YT1"=w3826, "YT2"=w3825, "YT3"=w3824) -> (w3846:T25)
              n1646 = property on="AuxFree" class="LstBox (strict)"("Disabled"=w4100) -> ()  [unwired: 2 in, 2 out]
              n1647 = Add(x=w3722, y=w3698) -> (x+y=w3699:i32)
              n1648 = Add(x=w3699, y="AuxFree") -> (x+y=w3914:i32[])
              n1649 = Array Size(array=w3914) -> (size(s)=w4059:i32)
              n1650 = Not Equal?(x=w4059, y=w4109) -> (x != y?=w4106:bool)
              n1651 = Not Equal?(x=w3914, y=w4105) -> (x != y?=w4108:bool[])
              n1652 = Or Array Elements(Boolean array=w4108) -> (logical OR=w4107:bool)
              n1653 = Bundle By Name(cluster=w3708, "Size"=w3836) -> (w3838:T4)
              n1654 = call "Act_Screen.vi"("Screen Reset Interval"=w3868, "Max/Min Display Blocksize"=w4158, "Nr of Channels"=w3763, "New Total Buffered"=w4167, "Buffer Size"=w4048, "ADC samples/s"=w4160, "Old Display Blocksize"=w4047, "Old Total Displayed"=w4159) -> ("Screen Reset Parameters"=w4156:T31, "New Display Blocksize"=w3735:i64, "New Total Displayed"=w4161:i64, "Errors Out"=w4085:T32)
              n1655 = Unbundle By Name(w4085) -> ("Ring Buffer Overflow"=w3940:bool, "First Call"=w3723:bool)
              n1656 = case shown="False" w3855 {
                tunnel: [w4282 w4307] -> w4019
                tunnel: [w4280 w4314] -> w3716
                tunnel: [w4281 w4311] -> w3726
                tunnel: w4018 -> [_ w4305]
                tunnel: w3707 -> [w4278 w4313]
                tunnel: w3937 -> [w4276 w4312]
                tunnel: [w4279 w4309] -> w3971
                tunnel: w3946 -> [w4279 _]
                tunnel: "Box" -> [w4277 _]
                tunnel: w3945 -> [w4275 w4310]
                tunnel: [w4274 w4309] -> w3870
                tunnel: w3723 -> [w4273 w4308]
                tunnel: [T14 {"Jazz No Data"=FALSE, "Jazz Packet Loss"=FALSE, "Jazz Batt"=0, "Jazz New Firmware"=FALSE} ("Jazz Cluster") w4304] -> w3721
                tunnel: w3773 -> [_ w4306]
                tunnel: w3706 -> [w4272 w4303]
                tunnel: [u8 0 ("Battery Voltage") w4302] -> w3770
                tunnel: w3762 -> [w4269 w4300]
                tunnel: w3760 -> [w4270 w4301]
                tunnel: w3728 -> [_ w4299]
                frame False {
                  n1657 = case shown="True" w4279 {
                    tunnel: [w4284 w4289] -> w4282
                    tunnel: [w4285 w4288] -> w4281
                    tunnel: [T15 {"GSR1pos"=FALSE, "GSR1neg"=FALSE, "GSR2pos"=FALSE, "GSR2neg"=FALSE} ("GSR in Range") w4290] -> w4280
                    tunnel: w4278 -> [_ w4293]
                    tunnel: w4277 -> [_ w4295]
                    tunnel: w4276 -> [_ w4292]
                    tunnel: [FALSE ("CM in Range") w4287] -> w4274
                    tunnel: w4275 -> [_ w4291]
                    tunnel: w4273 -> [_ w4294]
                    tunnel: w4272 -> [_ w4296]
                    tunnel: w4270 -> [w4284 w4298]
                    tunnel: w4269 -> [w4285 w4297]
                    frame False {
                    }
                    frame True {
                      n1658 = call "Convert_Daisy_Tr.vi"("Status Channel  In"=w4298, "GSR16Hz"=w4291, "N Chan Array In"=w4297, "Speedmode"=w4296, "Box"=w4295, "First Call"=w4294, "Sytem Cluster"=w4293, "ADC Rate"=w4292) -> ("GSR in Range"=w4290:T15, "Status Channnel"=w4289:i32[], "576 or 544 Chan Array"=w4288:i32[][], "CM in Range"=w4287:bool)  [unwired: 1 in, 3 out]
                    }
                  }
                }
                frame True {
                  w4309 = FALSE
                  n1659 = case shown="0, Default" w4303 {
                    tunnel: [w4320 T15 {"GSR1pos"=FALSE, "GSR1neg"=FALSE, "GSR2pos"=FALSE, "GSR2neg"=FALSE} ("GSR in Range")] -> w4314
                    tunnel: w4313 -> [w4323 _]
                    tunnel: w4312 -> [w4322 w4331]
                    tunnel: [w4316 w4333] -> w4311
                    tunnel: w4310 -> [w4319 _]
                    tunnel: w4308 -> [w4324 w4334]
                    tunnel: [w4317 w4336] -> w4307
                    tunnel: w4306 -> [w4318 _]
                    tunnel: w4305 -> [w4325 _]
                    tunnel: [w4321 T14 {"Jazz No Data"=FALSE, "Jazz Packet Loss"=FALSE, "Jazz Batt"=0, "Jazz New Firmware"=FALSE} ("Jazz Cluster")] -> w4304
                    tunnel: [u8 0 ("Battery Voltage") w4332] -> w4302
                    tunnel: w4301 -> [w4327 w4336]
                    tunnel: w4300 -> [w4326 w4335]
                    tunnel: w4299 -> [w4315 _]
                    frame 0, Default {
                      n1660 = call "Convert_4-13_Tr.vi"("Status Channel  In"=w4327, "Jazz On"=w4318, "GSR16Hz"=w4319, "N Chan Array In"=w4326, "AIB"=w4325, "First Call"=w4324, "Sytem Cluster"=w4323, "ADC Rate"=w4322, "ABR Enabled"=w4315) -> ("GSR in Range"=w4320:T15, "Jazz Cluster"=w4321:T14, "Status Channnel"=w4317:i32[], "N Chan Array Out"=w4316:i32[][])  [unwired: 3 in]
                    }
                    frame 9 {
                      n1661 = call "Convert_9_X.vi"("Initialize Filters"=w4334, "ADC Rate"=w4331, "8 Chan Array In"=w4335) -> ("Battery Voltage"=w4332:u8, "8 Chan Array Out"=w4333:i32[][])
                    }
                  }
                }
              }
              n1662 = Unbundle By Name(w3716) -> ("GSR1pos"=w3715:bool, "GSR1neg"=w3714:bool, "GSR2pos"=w3713:bool, "GSR2neg"=w3712:bool)
              n1663 = And(x=w3711, y=w3715) -> (x .and. y?=→"GSR1 pos":bool)
              n1664 = And(x=w3711, y=w3714) -> (x .and. y?=→"GSR1 neg":bool)
              n1665 = And(x=w3710, y=w3713) -> (x .and. y?=→"GSR2 pos":bool)
              n1666 = And(x=w3710, y=w3712) -> (x .and. y?=→"GSR2 neg":bool)
              n1667 = call "sEMG-ChanSwap.vi"("First Call"=w3723, "MonChannels"=w3722, "SMEGswap"=w3724, "Array In"=w3726) -> ("Array Out"=w3725:i32[][])
              n1668 = call "Downsample.vi"("Status Channel  In"=w4019, "Acquiring?"=w3871, "N Channel Array In"=w3725, "First Call"=w3723, "Marker Cluster"=w4023, "Decimate Ratio"=w3774) -> ("N-1 Channel Array Out"=w3915:i32[][], "Status Channel Out"=w3911:i32[])
              n1669 = call "TrigProcess.vi"("PopupKiller"=w3891, "Pause Cluster"=w3985, "First Call"=w3723, "Pause Saving"=w3984, "Decimation Factor"=w3686, "Status Channel  In"=w3911, "Nr of Displayed Triggers"=w3980) -> ("Pause"=w3983:bool, "Lamps Cluster"=w3982:cluster{"CM in Range":bool, "Low Batt":bool}, "Triggers Boolean"=w3704:bool[][], "Triggers Chart Signals"=→"Trigger Chart":i32[][])
              n1670 = Exclusive Or(1:w3984, 2:w3983) -> (0:w4028:bool)
              n1671 = case shown="True" w4028 {
                tunnel: w3983 -> [_ w4337]
                frame False {
                }
                frame True {
                  n1672 = local write "Pause Saving"(w4337) -> ()
                }
              }
              n1673 = Unbundle By Name(w3982) -> ("CM in Range"=w3955:bool, "Low Batt"=w3981:bool)
              n1674 = Select(t=w3870, s=w3953, f=w3955) -> (s? t:f=w3803:bool)
              "CM in Range" <- w3803
              n1675 = Compound Arithmetic op=OR(w3723, w4107, w4106) -> (w3781:bool)
              n1676 = Unbundle By Name(w3721) -> ("Jazz No Data"=w3720:bool, "Jazz Packet Loss"=w3719:bool, "Jazz Batt"=w3718:u8, "Jazz New Firmware"=→"Jazz New\nFirmware":bool)
              "Jazz Batt Cap" <- w3718
              n1677 = Add(x=w3699, y=w3923) -> (x+y=w3917:i32)
              n1678 = case shown="True" w3971 {
                tunnel: w3917 -> [_ w4266]
                tunnel: w3915 -> [w4262 w4265]
                tunnel: [w4262 w4264] -> w3730
                tunnel: "Box" -> [_ w4263]
                frame False {
                }
                frame True {
                  n1679 = Multiply(x=w4263, y=w4266) -> (x*y=w4267:i32)
                  n1680 = Array Subset(array=w4265, index (row)=w4267, length (row)=w4266) -> (w4264:i32[][])  [unwired: 2 in]
                }
              }
              n1681 = Array Subset(array=w3730, index (row)=w3699, length (row)=w3923) -> (w4110:i32[][])  [unwired: 2 in]
              n1682 = call "TCP-Jazz.vi"("Status Channel  In"=w3911, "connection ID"=w4005, "TCP Connected"=w4006, "TCP Add Cluster"=w3804, "Chan Number Cluster"=w4007, "error in (no error)"=w4009, "TCP Samples/Chan"=w4003, "TCP total Bytes"=w4004, "N Channel Array In"=w3730) -> ("error out"=w4008:errorcluster, "Bytes Received by Client"=→"Bytes received by Client":i32, "Bytes Sent by Server"=→"Bytes sent by Server":i32)
              n1683 = Format Into String(format string="%d", w3718) -> (resulting string=w3884:string)  [unwired: 2 in, 1 out]
              n1684 = Equal?(x=w3997, y=i8 8) -> (x = y?=w3996:bool)
              n1685 = case shown="\"Offset\"" "Charts/Graphs" {
                tunnel: w3730 -> [w4523 w4548 _]
                tunnel: w3722 -> [w4507 _ _]
                tunnel: w3706 -> [w4506 w4547 _]
                tunnel: w3869 -> [w4519 _ _]
                tunnel: w3766 -> [w4504 _ _]
                tunnel: w3946 -> [w4508 _ _]
                tunnel: w3709 -> [_ w4542 _]
                tunnel: w3708 -> [w4493 _ _]
                frame "Offset" {
                  n1686 = case shown="0, Default" w4519 {
                    tunnel: [i8 3 ("x") i8 4 ("x")] -> w4527
                    frame 0, Default {
                    }
                    frame 1 {
                    }
                  }
                  n1687 = Equal?(x="OffsetScale", y=w4527) -> (x = y?=w4531:bool)
                  "Full Range" <- w4531
                  n1688 = call "DCviewer-Mon.vi"("N Chan In"=w4523, "Speedmode"=w4506, "Mark2"=w4508, "Channels"="Offset", "ElecGain"=w4519) -> ("First Trace"=w4500:i32, "First Half array out"=→"Offset Graph First Half":dbl[], "First Half Graph Scaling"=w4518:T33, "Second Half array out"=→"Offset Graph  Second Half":dbl[], "Second Half Graph Scaling"=w4524:T33)
                  n1689 = property on="Offset Graph First Half" class="WFGraph (strict)"() -> ("Width"=w4497:u32)  [unwired: 2 in, 2 out]
                  n1690 = case shown="0" "OffsetScale" {
                    tunnel: [20.0 50.0 100.0 262.0 1049.0] -> w4511
                    frame 0 {
                    }
                    frame 1 {
                    }
                    frame 2 {
                    }
                    frame 3, Default {
                    }
                    frame 4 {
                    }
                  }
                  n1691 = call "DCviewer-TP.vi"("ElecGain"=w4519, "Mark2"=w4508, "Speedmode"=w4506, "N Chan In"=w4523) -> ("Second Half array out"=→"TP Offset Graph 2":dbl[], "First Half array out"=→"TP Offset Graph 1":dbl[])
                  n1692 = Add(x=w4500, y=32) -> (x+y=w4499:i32)
                  n1693 = Select(t=u32 16711680, s=w4531, f=u32 255) -> (s? t:f=w4509:u32)
                  n1694 = To Double Precision Float(number=w4497) -> (double precision float=w4496:dbl)
                  n1695 = Unbundle(w4518) -> ("Xo"=w4526:dbl, "Xmax"=w4514:dbl, "Xmin"=w4513:dbl, "Marker values"=w4512:dbl[])
                  n1696 = Divide(x=w4496, y=932.0) -> (x/y=w4494:dbl)
                  n1697 = Negate(x=w4511) -> (-x=w4510:dbl)
                  n1698 = property on="Offset Graph First Half" class="WFGraph (strict)"("Plot.Fill/Pt. Color"=w4509, "X Scale.Offset and Multiplier:Offset"=w4526, "XScale.Maximum"=w4514, "XScale.Minimum"=w4513, "XScale.MarkerVals[]"=w4512) -> ()  [unwired: 2 in, 2 out]
                  n1699 = Unbundle(w4524) -> ("Xo"=w4525:dbl, "Xmax"=w4517:dbl, "Xmin"=w4516:dbl, "Marker values"=w4515:dbl[])
                  n1700 = property on="Offset Graph First Half" class="WFGraph (strict)"("Y Scale.Range:Maximum"=w4511, "YScale.Minimum"=w4510) -> ()  [unwired: 2 in, 2 out]
                  n1701 = property on="Offset Graph  Second Half" class="WFGraph (strict)"("Y Scale.Range:Maximum"=w4511, "YScale.Minimum"=w4510) -> ()  [unwired: 2 in, 2 out]
                  n1702 = call "DClabels.vi"("Offset"="Offset", "Mark2"=w4508, "Speedmode"=w4506, "Mon Channels"=w4507, "Spec Labels"=w4504) -> ("DC Labels"=w4502:string[])
                  n1703 = call "Write_Labels.vi"("[user-specified font]"=w4493, "Spec Labels"=w4502, "Ratio"=w4494, "First Trace"=w4499) -> ("DC Labels"=→"DCLabels1 2":picture)
                  n1704 = call "Write_Labels.vi"("[user-specified font]"=w4493, "Spec Labels"=w4502, "Ratio"=w4494, "First Trace"=w4500) -> ("DC Labels"=→"DCLabels1":picture)
                  n1705 = property on="Offset Graph  Second Half" class="WFGraph (strict)"("Plot.Fill/Pt. Color"=w4509, "X Scale.Offset and Multiplier:Offset"=w4525, "XScale.Maximum"=w4517, "XScale.Minimum"=w4516, "XScale.MarkerVals[]"=w4515) -> ()  [unwired: 2 in, 2 out]
                  n1706 = property on="TP Offset Graph 1" class="WFGraph (strict)"("YScale.Maximum"=w4511, "YScale.Minimum"=w4510, "Plot.Fill/Pt. Color"=w4509) -> ()  [unwired: 2 in, 2 out]
                  n1707 = property on="TP Offset Graph 2" class="WFGraph (strict)"("YScale.Maximum"=w4511, "YScale.Minimum"=w4510, "Plot.Fill/Pt. Color"=w4509) -> ()  [unwired: 2 in, 2 out]
                }
                frame "ABR" {
                  w4553 = 8192.0  # Convert to uV
                  w4556 = 1000.0  # uV/mV
                  n1708 = Not Equal?(x=w4547, y=i8 9) -> (x != y?=w4545:bool)
                  n1709 = case shown="1" w4542 {
                    tunnel: [120 ("f") 140 ("f")] -> w4540
                    frame 0, Default {
                    }
                    frame 1 {
                    }
                  }
                  n1710 = Select(t=w4540, s=w4545, f=0 ("t")) -> (s? t:f=w4543:i32)
                  n1711 = Equal?(x="AbrOffsetScale", y=i8 3 ("x")) -> (x = y?=w4549:bool)
                  "ABR Full Range" <- w4549
                  n1712 = Array Size(array=w4548) -> (size(s)=w4558:i32[])
                  n1713 = Array Subset(array=w4548, index (row)=w4543, length (row)=3 ("length")) -> (w4559:i32[][])  [unwired: 2 in]
                  n1714 = case shown="3, Default" "AbrOffsetScale" {
                    tunnel: [20.0 50.0 100.0 262.0] -> w4562
                    frame 0 {
                    }
                    frame 1 {
                    }
                    frame 2 {
                    }
                    frame 3, Default {
                    }
                  }
                  n1715 = Index Array(array=w4558) -> (element #2=w4555:i32)  [unwired: 2 in, 1 out]
                  n1716 = Select(t=u32 16711680, s=w4549, f=u32 255) -> (s? t:f=w4560:u32)
                  n1717 = To Double Precision Float(number=w4555) -> (double precision float=w4557:dbl)
                  n1718 = Negate(x=w4562) -> (-x=w4561:dbl)
                  n1719 = Multiply(x=w4557, y=w4556) -> (x*y=w4554:dbl)
                  n1720 = for {
                    tunnel: w4559 -> [w4573] mode=indexing
                    tunnel: [w4569] -> w4550 mode=indexing
                    tunnel: w4554 -> [w4568]
                    tunnel: w4553 -> [w4567]
                    n1721 = To Double Precision Float(number=w4573) -> (double precision float=w4570:dbl[])
                    n1722 = Divide(x=w4570, y=w4567) -> (x/y=w4571:dbl[])
                    n1723 = Add Array Elements(numeric array=w4571) -> (sum=w4572:dbl)
                    n1724 = Divide(x=w4572, y=w4568) -> (x/y=w4569:dbl)
                  }
                  "ABR Offset Graph" <- w4550
                  n1725 = property on="ABR Offset Graph" class="WFGraph (strict)"("YScale.Maximum"=w4562, "YScale.Minimum"=w4561, "Plot.Fill/Pt. Color"=w4560) -> ()  [unwired: 2 in, 2 out]
                }
                frame "About/Configure", Default {
                }
              }
              n1726 = call "Act_Save.vi"("ChanSelection"=w3854, "Status Channel  In"=w3911, "Data In"=w3915, "Samples per Record"=w3944, "BDF Buffer In"=w3943, "Index in Byte In"=w3942) -> ("Nr of Chan Saved"=w4063:i32, "BDF Buffer Out"=w4128:u8[], "Index in Byte Out"=w4129:i32)
              n1727 = Add(x=w3679, y=w3917) -> (x+y=w3925:i32)
              n1728 = Concatenate Strings(w3884, " %" ("string")) -> (→"Jazz Batt Perc":string)
              n1729 = case shown="1" w3786 {
                tunnel: [FALSE FALSE TRUE] -> w3779
                tunnel: [i8 0 i8 2 i8 0] -> w4120
                tunnel: [FALSE TRUE FALSE] -> w3775
                frame 0, Default {
                }
                frame 1 {
                }
                frame 2 {
                }
              }
              n1730 = Compound Arithmetic op=OR(w3775, w3781, w3777) -> (w3812:bool)
              n1731 = case shown="True" w3812 {
                tunnel: "AuxFree" -> [_ w4442]
                tunnel: w3766 -> [_ w4437]
                tunnel: w3914 -> [_ w4440]
                tunnel: w3708 -> [_ w4435]
                frame False {
                }
                frame True {
                  w4441 = 8  # Max Nr of Aux Labels
                  n1732 = stacked-sequence {
                    tunnel: w4442 -> [w4452 w4463 w4473 w4481 w4487]
                    frame #0 {
                      w4443 = T6."Disabled and Grayed Out" ("Disabled")
                      w4444 = T6."Enabled" ("Disabled")
                      w4449 = -1 ("y")
                      n1733 = Search 1D Array(1D array=w4452, element=0) -> (index of element=w4456:i32)  [unwired: 1 out]
                      n1734 = Search 1D Array(1D array=w4452, element=1) -> (index of element=w4455:i32)  [unwired: 1 out]
                      n1735 = Not Equal?(x=w4456, y=w4449) -> (x != y?=w4454:bool)
                      n1736 = Not Equal?(x=w4455, y=w4449) -> (x != y?=w4448:bool)
                      n1737 = Or(x=w4454, y=w4448) -> (x .or. y?=w4453:bool)
                      n1738 = Select(t=w4444, s=w4448, f=w4443) -> (s? t:f=w4445:T6)
                      n1739 = Select(t=w4444, s=w4454, f=w4443) -> (s? t:f=w4447:T6)
                      n1740 = Select(t=w4444, s=w4453, f=w4443) -> (s? t:f=w4446:T6)
                      n1741 = property on="GSR1 pos" class="Bool (strict)"("Disabled"=w4447) -> ()  [unwired: 2 in, 2 out]
                      n1742 = property on="GSR1 neg" class="Bool (strict)"("Disabled"=w4447) -> ()  [unwired: 2 in, 2 out]
                      n1743 = property on="GSR1" class="DigNum (strict)"("Disabled"=w4447) -> ()  [unwired: 2 in, 2 out]
                      n1744 = property on="GSR2 pos" class="Bool (strict)"("Disabled"=w4445) -> ()  [unwired: 2 in, 2 out]
                      n1745 = property on="GSR2 neg" class="Bool (strict)"("Disabled"=w4445) -> ()  [unwired: 2 in, 2 out]
                      n1746 = property on="GSR2" class="DigNum (strict)"("Disabled"=w4445) -> ()  [unwired: 2 in, 2 out]
                      n1747 = property on="GsrScale" class="Ring (strict)"("Disabled"=w4446) -> ()  [unwired: 2 in, 2 out]
                      n1748 = property on="Unit" class="Str"("Disabled"=w4446) -> ()  [unwired: 2 in, 2 out]
                    }
                    frame #1 {
                      w4459 = -1 ("y")
                      n1749 = Search 1D Array(1D array=w4463, element=2) -> (index of element=w4468:i32)  [unwired: 1 out]
                      n1750 = Search 1D Array(1D array=w4463, element=3) -> (index of element=w4467:i32)  [unwired: 1 out]
                      n1751 = Not Equal?(x=w4468, y=w4459) -> (x != y?=w4466:bool)
                      n1752 = Not Equal?(x=w4467, y=w4459) -> (x != y?=w4465:bool)
                      n1753 = Or(x=w4466, y=w4465) -> (x .or. y?=w4464:bool)
                      n1754 = Select(t=T6."Enabled" ("Disabled"), s=w4464, f=T6."Disabled and Grayed Out" ("Disabled")) -> (s? t:f=w4460:T6)
                      n1755 = property on="ErgoScale" class="Ring (strict)"("Disabled"=w4460) -> ()  [unwired: 2 in, 2 out]
                    }
                    frame #2 {
                      n1756 = Search 1D Array(1D array=w4473, element=4) -> (index of element=w4475:i32)  [unwired: 1 out]
                      n1757 = Not Equal?(x=w4475, y=-1) -> (x != y?=w4470:bool)
                      n1758 = Select(t=T6."Enabled" ("Disabled"), s=w4470, f=T6."Disabled and Grayed Out" ("Disabled")) -> (s? t:f=w4472:T6)
                      n1759 = property on="RespScale" class="Ring (strict)"("Disabled"=w4472) -> ()  [unwired: 2 in, 2 out]
                    }
                    frame #3 {
                      n1760 = Search 1D Array(1D array=w4481, element=5) -> (index of element=w4484:i32)  [unwired: 1 out]
                      n1761 = Not Equal?(x=w4484, y=-1) -> (x != y?=w4480:bool)
                      n1762 = Select(t=T6."Enabled" ("Disabled"), s=w4480, f=T6."Disabled and Grayed Out" ("Disabled")) -> (s? t:f=w4479:T6)
                      n1763 = property on="PletScale" class="Ring (strict)"("Disabled"=w4479) -> ()  [unwired: 2 in, 2 out]
                    }
                    frame #4 {
                      n1764 = Search 1D Array(1D array=w4487, element=6) -> (index of element=w4492:i32)  [unwired: 1 out]
                      n1765 = Not Equal?(x=w4492, y=-1) -> (x != y?=w4489:bool)
                      n1766 = Select(t=T6."Enabled" ("Disabled"), s=w4489, f=T6."Disabled and Grayed Out" ("Disabled")) -> (s? t:f=w4488:T6)
                      n1767 = property on="TempScale" class="Ring (strict)"("Disabled"=w4488) -> ()  [unwired: 2 in, 2 out]
                      n1768 = property on="Degrees Celcius" class="DigNum (strict)"("Disabled"=w4488) -> ()  [unwired: 2 in, 2 out]
                    }
                  }
                  n1769 = property on="Aux Chart" class="WFChart (strict)"() -> ("Height"=w4439:u32)  [unwired: 2 in, 2 out]
                  n1770 = call "LabelsMon.vi"("Max Nr of Labels"=w4441, "Spec Labels"=w4437, "Channel Selection"=w4440, "Height"=w4439, "[user-specified font]"=w4435) -> ("Mon Labels"=→"AuxLabels":picture, "Y-Max"=w4438:dbl)
                  n1771 = property on="Aux Chart" class="WFChart (strict)"("YScale.Maximum"=w4438) -> ()  [unwired: 2 in, 2 out]
                }
              }
              n1772 = And(x=w3779, y="AuxReset") -> (x .and. y?=w4111:bool)
              n1773 = Or(x=w4111, y=w4114) -> (x .or. y?=w4113:bool)
              n1774 = call "Ref-Sens-Deci.vi"("First Call"=w3723, "Decimating factor"=w3686, "BreathBelt"=w3691, "Gain Cluster"=w4086, "Reset Traces"=w4113, "Sample Rate"=w3681, "Sensor Selection"="AuxFree", "8 Channel Aux Array In"=w4110) -> ("Battery Voltage"=w3772:u8, "Temperature"=→"Degrees Celcius":dbl, "Chart Array"=→"Aux Chart":dbl[][], "GSR Cluster"=w3694:cluster{"GSR1":dbl, "GSR2":dbl})
              n1775 = Unbundle By Name(w3694) -> ("GSR1"=→"GSR1":dbl, "GSR1"=→"GSR2":dbl)
              n1776 = Select(t=w3772, s=w3749, f=w3770) -> (s? t:f=→"Battery":u8)
              n1777 = And(x=w3919, y=w3996) -> (x .and. y?=w4098:bool)
              n1778 = call "DCviewer-Maps.vi"("N Chan In"=w3730, "CM in Range"=w3803) -> ("129 Chan DC Out"=w3805:dbl[])
              n1779 = Unbundle By Name(w3889) -> ("Sync Errors"=w3890:i16, "Recent Sync Error"=w3886:bool)
              n1780 = Add(x="AnaFree", y=w3925) -> (x+y=w3816:i32[])
              n1781 = Add(x="BipFree", y=w3722) -> (x+y=w3916:i32[])
              n1782 = And(x="AnaReset", y=w3779) -> (x .and. y?=w4029:bool)
              n1783 = global write "Data.glb" "Data"(w3805) -> ()
              n1784 = Not(x=w3720) -> (.not. x?=w3874:bool)
              n1785 = Less Or Equal?(x=w3718, y=u8 5) -> (x <= y?=w3873:bool)
              n1786 = Bundle("AvgLP"="AvgLP", "AvgLPfreq"="AvgLPfreq", "AvgHP"="AvgHP", "AvgHPfreq"="AvgHPfreq") -> (w3755:T34)  [unwired: 1 out]
              n1787 = call "Ref-Avg-ABR.vi"("HP Cluster"=w3755, "ABR Enabled"=w3728, "Initialize Filters"=w3723, "ABRlocation"=w3709, "Speedmode"=w3706, "Sample Rate"=w3681, "N Channel Array In"=w3730, "RefFreeAvg2"="RefFreeAvg2", "MonFreeAvg2"="MonFreeAvg2", "RefFreeAvg1"="RefFreeAvg1", "MonFreeAvg1"="MonFreeAvg1") -> ("2 Avg Chan Out"=w4062:dbl[][])
              n1788 = Equal To 0?(x="TrigCode") -> (x = 0?=w3974:bool)
              n1789 = Compound Arithmetic op=AND(w3874, w3873, w3773) -> (w3872:bool)
              n1790 = Not Equal To 0?(x=w3679) -> (x != 0?=w3924:bool)
              n1791 = Decrement(x=w4063) -> (x-1=w4070:i32)
              n1792 = Add(x=w3890, y=w3765) -> (x+y=w3888:i16)
              "Errors:" <- w3888
              n1793 = Not Equal To 0?(x=w3765) -> (x != 0?=w3885:bool)
              n1794 = case shown="14" "Channels" {
                tunnel: [i32[] [0, 1, 2, 3, 4, 5, 6, 7, 8, 9, 10, 11, 12, 13, 14, 15, 16, 17, 18, 19, 20, 21, 22, 23, 24, 25, 26, 27, 28, 29, 30, 31, 32, 33, 34, 35, 36, 37, 38, 39, 40, 41, 42, 43, 44, 45, 46, 47, 48, 49, 50, 51, 52, 53, 54, 55, 56, 57, 58, 59, 60, 61, 62, 63, 64, 65, 66, 67, 68, 69, 70, 71, 72, 73, 74, 75, 76, 77, 78, 79, 80, 81, 82, 83, 84, 85, 86, 87, 88, 89, 90, 91, 92, 93, 94, 95, 96, 97, 98, 99, 100, 101, 102, 103, 104, 105, 106, 107, 108, 109, 110, 111, 112, 113, 114, 115, 116, 117, 118, 119, 120, 121, 122, 123, 124, 125, 126, 127, 128, 129, 130, 131, 132, 133, 134, 135, 136, 137, 138, 139, 140, 141, 142, 143, 144, 145, 146, 147, 148, 149, 150, 151, 152, 153, 154, 155, 156, 157, 158, 159, 160, 161, 162, 163, 164, 165, 166, 167, 168, 169, 170, 171, 172, 173, 174, 175, 176, 177, 178, 179, 180, 181, 182, 183, 184, 185, 186, 187, 188, 189, 190, 191, 192, 193, 194, 195, 196, 197, 198, 199, 200, 201, 202, 203, 204, 205, 206, 207, 208, 209, 210, 211, 212, 213, 214, 215, 216, 217, 218, 219, 220, 221, 222, 223, 224, 225, 226, 227, 228, 229, 230, 231, 232, 233, 234, 235, 236, 237, 238, 239, 240, 241, 242, 243, 244, 245, 246, 247, 248, 249, 250, 251, 252, 253, 254, 255, 256, 257, 258, 259, 260, 261, 262, 263] ("Array") i32[] [0, 1, 2, 3, 4, 5, 6, 7, 8, 9, 10, 11, 12, 13, 14, 15, 16, 17, 18, 19, 20, 21, 22, 23, 24, 25, 26, 27, 28, 29, 30, 31, 32, 33, 34, 35, 36, 37, 38, 39, 40, 41, 42, 43, 44, 45, 46, 47, 48, 49, 50, 51, 52, 53, 54, 55, 56, 57, 58, 59, 60, 61, 62, 63, 64, 65, 66, 67, 68, 69, 70, 71, 72, 73, 74, 75, 76, 77, 78, 79, 80, 81, 82, 83, 84, 85, 86, 87, 88, 89, 90, 91, 92, 93, 94, 95, 96, 97, 98, 99, 100, 101, 102, 103, 104, 105, 106, 107, 108, 109, 110, 111, 112, 113, 114, 115, 116, 117, 118, 119, 120, 121, 122, 123, 124, 125, 126, 127, 128, 129, 130, 131, 132, 133, 134, 135, 136, 137, 138, 139, 140, 141, 142, 143, 144, 145, 146, 147, 148, 149, 150, 151, 152, 153, 154, 155, 156, 157, 158, 159, 160, 161, 162, 163, 164, 165, 166, 167, 168, 169, 170, 171, 172, 173, 174, 175, 176, 177, 178, 179, 180, 181, 182, 183, 184, 185, 186, 187, 188, 189, 190, 191, 192, 193, 194, 195, 196, 197, 198, 199, 200, 201, 202, 203, 204, 205, 206, 207, 208, 209, 210, 211, 212, 213, 214, 215, 216, 217, 218, 219, 220, 221, 222, 223, 224, 225, 226, 227, 228, 229, 230, 231, 232, 233, 234, 235, 236, 237, 238, 239, 240, 241, 242, 243, 244, 245, 246, 247, 248, 249, 250, 251, 252, 253, 254, 255] ("All Channels") i32[] [0, 1, 2, 3, 4, 5, 6, 7, 8, 9, 10, 11, 12, 13, 14, 15, 16, 17, 18, 19, 20, 21, 22, 23, 24, 25, 26, 27, 28, 29, 30, 31, 32, 33, 34, 35, 36, 37, 38, 39, 40, 41, 42, 43, 44, 45, 46, 47, 48, 49, 50, 51, 52, 53, 54, 55, 56, 57, 58, 59, 60, 61, 62, 63, 64, 65, 66, 67, 68, 69, 70, 71, 72, 73, 74, 75, 76, 77, 78, 79, 80, 81, 82, 83, 84, 85, 86, 87, 88, 89, 90, 91, 92, 93, 94, 95, 96, 97, 98, 99, 100, 101, 102, 103, 104, 105, 106, 107, 108, 109, 110, 111, 112, 113, 114, 115, 116, 117, 118, 119, 120, 121, 122, 123, 124, 125, 126, 127, 128, 129, 130, 131, 132, 133, 134, 135, 136, 137, 138, 139, 140, 141, 142, 143, 144, 145, 146, 147, 148, 149, 150, 151, 152, 153, 154, 155, 156, 157, 158, 159] ("Array") i32[] [0, 1, 2, 3, 4, 5, 6, 7, 8, 9, 10, 11, 12, 13, 14, 15, 16, 17, 18, 19, 20, 21, 22, 23, 24, 25, 26, 27, 28, 29, 30, 31, 32, 33, 34, 35, 36, 37, 38, 39, 40, 41, 42, 43, 44, 45, 46, 47, 48, 49, 50, 51, 52, 53, 54, 55, 56, 57, 58, 59, 60, 61, 62, 63, 64, 65, 66, 67, 68, 69, 70, 71, 72, 73, 74, 75, 76, 77, 78, 79, 80, 81, 82, 83, 84, 85, 86, 87, 88, 89, 90, 91, 92, 93, 94, 95, 96, 97, 98, 99, 100, 101, 102, 103, 104, 105, 106, 107, 108, 109, 110, 111, 112, 113, 114, 115, 116, 117, 118, 119, 120, 121, 122, 123, 124, 125, 126, 127] ("Array") i32[] [0, 1, 2, 3, 4, 5, 6, 7, 8, 9, 10, 11, 12, 13, 14, 15, 16, 17, 18, 19, 20, 21, 22, 23, 24, 25, 26, 27, 28, 29, 30, 31, 32, 33, 34, 35, 36, 37, 38, 39, 40, 41, 42, 43, 44, 45, 46, 47, 48, 49, 50, 51, 52, 53, 54, 55, 56, 57, 58, 59, 60, 61, 62, 63] ("Array") i32[] [0, 1, 2, 3, 4, 5, 6, 7, 8, 9, 10, 11, 12, 13, 14, 15, 16, 17, 18, 19, 20, 21, 22, 23, 24, 25, 26, 27, 28, 29, 30, 31] ("Array") i32[] [32, 33, 34, 35, 36, 37, 38, 39, 40, 41, 42, 43, 44, 45, 46, 47, 48, 49, 50, 51, 52, 53, 54, 55, 56, 57, 58, 59, 60, 61, 62, 63] ("Array") i32[] [64, 65, 66, 67, 68, 69, 70, 71, 72, 73, 74, 75, 76, 77, 78, 79, 80, 81, 82, 83, 84, 85, 86, 87, 88, 89, 90, 91, 92, 93, 94, 95] ("Array") i32[] [96, 97, 98, 99, 100, 101, 102, 103, 104, 105, 106, 107, 108, 109, 110, 111, 112, 113, 114, 115, 116, 117, 118, 119, 120, 121, 122, 123, 124, 125, 126, 127] ("Array") i32[] [128, 129, 130, 131, 132, 133, 134, 135, 136, 137, 138, 139, 140, 141, 142, 143, 144, 145, 146, 147, 148, 149, 150, 151, 152, 153, 154, 155, 156, 157, 158, 159] ("Array") i32[] [160, 161, 162, 163, 164, 165, 166, 167, 168, 169, 170, 171, 172, 173, 174, 175, 176, 177, 178, 179, 180, 181, 182, 183, 184, 185, 186, 187, 188, 189, 190, 191] ("Array") i32[] [192, 193, 194, 195, 196, 197, 198, 199, 200, 201, 202, 203, 204, 205, 206, 207, 208, 209, 210, 211, 212, 213, 214, 215, 216, 217, 218, 219, 220, 221, 222, 223] ("Array") i32[] [224, 225, 226, 227, 228, 229, 230, 231, 232, 233, 234, 235, 236, 237, 238, 239, 240, 241, 242, 243, 244, 245, 246, 247, 248, 249, 250, 251, 252, 253, 254, 255] ("Array") w4657 w4660] -> w3897
                tunnel: [w4629 w4631 w4633 w4635 w4637 w4639 w4641 w4643 w4645 w4647 w4649 w4651 w4653 w4655 T6."Enabled" ("Disabled")] -> w3898
                tunnel: w3722 -> [_ _ _ _ _ _ _ _ _ _ _ _ _ w4656 _]
                tunnel: "MonFree" -> [_ _ _ _ _ _ _ _ _ _ _ _ _ _ w4660]
                tunnel: T6."Disabled and Grayed Out" ("Disabled") -> [w4629 w4631 w4633 w4635 w4637 w4639 w4641 w4643 w4645 w4647 w4649 w4651 w4653 w4655 _]
                frame 0, Default {
                }
                frame 1 {
                }
                frame 2 {
                }
                frame 3 {
                }
                frame 4 {
                }
                frame 5 {
                }
                frame 6 {
                }
                frame 7 {
                }
                frame 8 {
                }
                frame 9 {
                }
                frame 10 {
                }
                frame 11 {
                }
                frame 12 {
                }
                frame 13 {
                  n1795 = Add(x=i32[] [0, 1, 2, 3, 4, 5, 6, 7] ("Array"), y=w4656) -> (x+y=w4657:i32[])
                }
                frame 14 {
                }
              }
              n1796 = Not Equal To 0?(x=w3698) -> (x != 0?=w3778:bool)
              n1797 = Add(x="JazzFree", y=w3917) -> (x+y=w3909:i32[])
              n1798 = Not Equal To 0?(x=w3680) -> (x != 0?=w3991:bool)
              n1799 = Not(x=w3974) -> (.not. x?=w4084:bool)
              n1800 = Format Into String(format string="%d" ("Format String"), w4070) -> (resulting string=w4068:string)  [unwired: 2 in, 1 out]
              n1801 = And(x="JazzReset", y=w3779) -> (x .and. y?=w3921:bool)
              n1802 = Select(t=w3909, s=w3924, f=i32[] []) -> (s? t:f=w3811:i32[])
              n1803 = Select(t=w3916, s=w3778, f=i32[] []) -> (s? t:f=w3999:i32[])
              n1804 = Select(t=w3816, s=w3991, f=i32[] []) -> (s? t:f=w3992:i32[])
              n1805 = And(x=w3886, y=w3885) -> (x .and. y?=w3938:bool)
              n1806 = property on="Trigger Code" class="Pict"("Visible"=w4084) -> ()  [unwired: 2 in, 2 out]
              n1807 = Array Size(array=w4062) -> (size(s)=w4073:i32[])
              n1808 = Concatenate Strings(w4068, " + 1" ("Substring")) -> (w4066:string)
              n1809 = call "Ref-Jazz-Deci.vi"("Decimating factor"=w3686, "Max Nr of Traces"=w3679, "Initialize Filters"=w3922, "Center Traces"=w3921, "Channels"=w3811, "Channel Array In"=w3730) -> ("Screen signals Out"=→"Jazz Chart":dbl[][])  [unwired: 3 in]
              n1810 = property on="Trigger Chart" class="WFChart (strict)"("Visible"=w3974) -> ()  [unwired: 2 in, 2 out]
              n1811 = Select(t=T6."Disabled and Grayed Out" ("Disabled"), s=w3910, f=T6."Enabled" ("Disabled")) -> (s? t:f=w3918:T6)
              n1812 = Select(t=w4066, s=w3919, f="0 + 0") -> (s? t:f=→"Nr Chan Saved":string)
              n1813 = Index Array(array=w4073) -> (element=w4072:i32)  [unwired: 1 in]
              n1814 = case shown="True" w4077 {
                selector: w4077 -> [_ w4391]
                tunnel: w4082 -> [w4388 _]
                tunnel: w4083 -> [w4389 _]
                tunnel: [w4389 w4402] -> w3908
                tunnel: [w4388 w4402] -> w3907
                tunnel: w4072 -> [_ w4401]
                tunnel: w4075 -> [w4387 w4390]
                tunnel: [w4387 w4400] -> w4076
                tunnel: w3944 -> [_ w4395]
                frame False {
                }
                frame True {
                  w4392 = 0 ("Rejected Sweeps")
                  # "Initilaize Buffers"
                  n1815 = Multiply(x="AvgSweep", y=w4395) -> (x*y=w4399:i32)
                  n1816 = To Double Precision Float(number=w4399) -> (double precision float=w4398:dbl)
                  n1817 = Divide(x=w4398, y=1000.0) -> (x/y=w4396:dbl)
                  n1818 = To Long Integer(number=w4396) -> (32bit integer=w4393:i32)
                  n1819 = local write "Valid Sweeps"(w4392) -> ()
                  n1820 = Bundle By Name(cluster=w4390, "Start Averaging"=w4391, "Busy Averaging"=w4391, "Sweep Lenght in Samples"=w4393, "Valid Sweeps"=w4392, "Rejected Sweeps"=w4392, "First Graph Update"=w4391) -> (w4400:T13)
                  n1821 = Initialize Array(0.0 ("element"), w4401, w4393) -> (w4402:dbl[][])
                  n1822 = local write "Rejected Sweeps"(w4392) -> ()
                }
              }
              n1823 = Array Size(array=w3811) -> (size(s)=w3810:i32)
              n1824 = case shown="True" "AddTP" {
                tunnel: w3897 -> [w4253 w4255]
                tunnel: [w4253 w4254] -> w3896
                tunnel: w3722 -> [_ w4257]
                frame False {
                }
                frame True {
                  n1825 = Add(x=i32[] [0, 1, 2, 3, 4, 5, 6, 7] ("Array"), y=w4257) -> (x+y=w4256:i32[])
                  n1826 = Build Array (concatenate)(w4255, w4256) -> (w4254:i32[])
                }
              }
              n1827 = Array Size(array=w3933) -> (size(s)=w3935:i32)
              n1828 = property on="JazzFree" class="LstBox (strict)"("Disabled"=w3918) -> ()  [unwired: 2 in, 2 out]
              n1829 = Not Equal?(x="AbrChannels", y=w3782) -> (x != y?=w3783:bool)
              n1830 = Not Equal?(x=w3810, y=w3935) -> (x != y?=w3926:bool)
              n1831 = Not Equal?(x=w3811, y=w3933) -> (x != y?=w3934:bool[])
              n1832 = property on="Dummy String" class="Str"("Visible"=w3974) -> ()  [unwired: 2 in, 2 out]
              n1833 = Or(x=w3783, y=w3723) -> (x .or. y?=w3733:bool)
              n1834 = Bundle("MonLP"="MonLP", "MonLPfreq"="MonLPfreq", "MonHP"="MonHP", "MonHPfreq"="MonHPfreq") -> (w3685:T35)  [unwired: 1 out]
              n1835 = Or Array Elements(Boolean array=w3934) -> (logical OR=w3927:bool)
              n1836 = Bundle("BipLP"="BipLP", "BipLPfreq"="BipLPfreq", "BipHP"="BipHP", "BipHPfreq"="BipHPfreq") -> (w3683:T36)  [unwired: 1 out]
              n1837 = Bundle By Name(cluster=w3889, "Sync Errors"=w3888, "Recent Sync Error"=w3885) -> (w3887:T26)
              n1838 = Bundle("AnaLP"="AnaLP", "AnaLPfreq"="AnaLPfreq", "AnaHP"="AnaHP", "AnaHPfreq"="AnaHPfreq") -> (w3682:T37)  [unwired: 1 out]
              n1839 = Compound Arithmetic op=OR(w3927, w3926, w3723) -> (w3809:bool)
              n1840 = Array Subset(array=w3896, length=w3699) -> (w3895:i32[])  [unwired: 1 in]
              n1841 = Select(t=w3859, s=w4098, f=w3898) -> (s? t:f=w4137:T6)
              n1842 = Select(t=w3859, s=w4098, f=T6."Enabled" ("Disabled")) -> (s? t:f=w3893:T6)
              n1843 = Select(t=w3730, s=w3728, f=i32[][] []) -> (s? t:f=w3729:i32[][])
              n1844 = Select(t=w3893, s=w3778, f=w3859) -> (s? t:f=w3892:T6)
              n1845 = property on="MonFree" class="LstBox (strict)"("Disabled"=w4137) -> ()  [unwired: 2 in, 2 out]
              n1846 = Equal?(x=T2."AIB" ("Charts/Graphs"), y="Charts/Graphs") -> (x = y?=w4088:bool)
              n1847 = property on="Channels" class="Ring (strict)"("Disabled"=w3893) -> ()  [unwired: 2 in, 2 out]
              n1848 = property on="AddTP" class="Bool (strict)"("Disabled"=w3892) -> ()  [unwired: 2 in, 2 out]
              n1849 = case shown="True" w4088 {
                tunnel: w3730 -> [_ w4408]
                tunnel: w3925 -> [_ w4406]
                frame False {
                }
                frame True {
                  n1850 = Add(x=w4406, y="AnaOffset") -> (x+y=w4404:i32)
                  n1851 = call "DCviewer-Ana.vi"("Ana Channels"=w4404, "N Chan In"=w4408) -> ("1 Chan array out"=→"Ana Offset Graph":dbl[])
                }
              }
              n1852 = Unbundle By Name(w4156) -> ("End of Screen"=w4104:bool, "Prop Screen Minimum"=w4101:i64, "Screen Position"=w3978:i32)
              n1853 = call "TriggerScreenVari.vi"("Screen Position"=w3978, "Downsample Correction"=w3774, "Block Cluster"=w3846, "[user-specified font]"=w3838, "Old picture 2"=w3912, "Old picture 1"=w3913, "Status Channel  In"=w3911, "TrigCode"="TrigCode") -> ("New picture 2"=w3976:picture, "New picture 1"=w3977:picture)
              n1854 = case shown="18" "AnaScale" {
                tunnel: [5.0 10.0 20.0 50.0 100.0 200.0 500.0 1000.0 2000.0 5000.0 10000.0 20000.0 50000.0 100000.0 200000.0 500000.0 1000000.0 2000000.0 4000000.0] -> w3687
                frame 0, Default {
                }
                frame 1 {
                }
                frame 2 {
                }
                frame 3 {
                }
                frame 4 {
                }
                frame 5 {
                }
                frame 6 {
                }
                frame 7 {
                }
                frame 8 {
                }
                frame 9 {
                }
                frame 10 {
                }
                frame 11 {
                }
                frame 12 {
                }
                frame 13 {
                }
                frame 14 {
                }
                frame 15 {
                }
                frame 16 {
                }
                frame 17 {
                }
                frame 18 {
                }
              }
              n1855 = call "Ref-Ana-Deci.vi"("Filter Cluster"=w3682, "Decimating factor"=w3686, "uV/div"=w3687, "Max Nr of Traces"=w3680, "Sample Rate"=w3681, "Initialize Filters"=w4030, "Center Traces"=w4029, "Channels"=w3992, "Channel Array In"=w3730) -> ("Screen signals Out"=→"Ana Chart":dbl[][])  [unwired: 2 in]
              n1856 = case shown="\"Monopolar\"" "Charts/Graphs" {
                tunnel: [T1."Monopolar" ("Left Sidebar") T1."Bipolar" ("Left Sidebar") T1."Offset" ("Left Sidebar") T1."ABR" ("Left Sidebar") T1."Average" ("Left Sidebar") T1."Sensors" ("Left Sidebar") T1."Jazz" ("Left Sidebar") T1."Analog" ("Left Sidebar") T1."Initialization" ("Left Sidebar")] -> w3793
                frame "Monopolar" {
                }
                frame "Bipolar" {
                }
                frame "Offset" {
                }
                frame "ABR" {
                }
                frame "ERP" {
                }
                frame "Sensors" {
                }
                frame "Jazz" {
                }
                frame "AIB" {
                }
                frame "About/Configure", Default {
                }
              }
              "Left Sidebar" <- w3793
              n1857 = case shown="15" "AbrScale" {
                tunnel: [5.0 10.0 20.0 50.0 100.0 200.0 500.0 1000.0 2000.0 5000.0 10000.0 20000.0 50000.0 100000.0 200000.0 500000.0] -> w3696
                frame 0, Default {
                }
                frame 1 {
                }
                frame 2 {
                }
                frame 3 {
                }
                frame 4 {
                }
                frame 5 {
                }
                frame 6 {
                }
                frame 7 {
                }
                frame 8 {
                }
                frame 9 {
                }
                frame 10 {
                }
                frame 11 {
                }
                frame 12 {
                }
                frame 13 {
                }
                frame 14 {
                }
                frame 15 {
                }
              }
              n1858 = call "Ref-ABR-Deci.vi"("Speedmode"=w3706, "Filter Cluster"=w3695, "Decimating factor"=w3686, "uV/div"=w3696, "ABRlocation"=w3709, "Sample Rate"=w3681, "Initialize Filters"=w3784, "Center Traces"=w3779, "Channels"="AbrChannels", "N Channel Array In"=w3729) -> ("Screen signals Out"=→"ABR Chart":dbl[][])  [unwired: 1 in]
              n1859 = Select(t=w3977, s=w4013, f=w3976) -> (s? t:f=→"Trigger Code":picture)
              n1860 = case shown="15" "MonScale" {
                tunnel: [5.0 10.0 20.0 50.0 100.0 200.0 500.0 1000.0 2000.0 5000.0 10000.0 20000.0 50000.0 100000.0 200000.0 500000.0] -> w3702
                frame 0, Default {
                }
                frame 1 {
                }
                frame 2 {
                }
                frame 3 {
                }
                frame 4 {
                }
                frame 5 {
                }
                frame 6 {
                }
                frame 7 {
                }
                frame 8 {
                }
                frame 9 {
                }
                frame 10 {
                }
                frame 11 {
                }
                frame 12 {
                }
                frame 13 {
                }
                frame 14 {
                }
                frame 15 {
                }
              }
              n1861 = case shown="15" "BipScale" {
                tunnel: [5.0 10.0 20.0 50.0 100.0 200.0 500.0 1000.0 2000.0 5000.0 10000.0 20000.0 50000.0 100000.0 200000.0 500000.0] -> w3700
                frame 0, Default {
                }
                frame 1 {
                }
                frame 2 {
                }
                frame 3 {
                }
                frame 4 {
                }
                frame 5 {
                }
                frame 6 {
                }
                frame 7 {
                }
                frame 8 {
                }
                frame 9 {
                }
                frame 10 {
                }
                frame 11 {
                }
                frame 12 {
                }
                frame 13 {
                }
                frame 14 {
                }
                frame 15 {
                }
              }
              n1862 = call "Ref-Bip-Deci.vi"("ElecGain"=w3869, "Filter Cluster"=w3683, "Decimating factor"=w3686, "uV/div"=w3700, "Max Nr of Traces"=w3698, "Sample Rate"=w3681, "Initialize Filter"=w4115, "Center Traces"=w3779, "Channels"=w3999, "Channel Array In"=w3730) -> ("Screen signals Out"=→"Bip Chart":dbl[][])  [unwired: 1 in]
              n1863 = Build Array(w3941, w3940, w3938, w3941, w3720, w3719) -> (w3740:bool[])
              n1864 = Compound Arithmetic op=OR(w3940, w3938, w3720, w3719) -> (w3939:bool)
              n1865 = Compound Arithmetic op=OR(w3775, w3809, w3777) -> (w3808:bool)
              n1866 = Array Size(array=w3895) -> (size(s)=w3970:i32)
              n1867 = Array Size(array=w4139) -> (size(s)=w4153:i32)
              n1868 = Bundle("AvgAbsReject"="AvgAbsReject", "AvgRelReject"="AvgRelReject") -> (w3904:cluster{"AvgAbsReject":dbl, "AvgRelReject":dbl})  [unwired: 1 out]
              n1869 = case shown="True" w4074 {
                selector: w4074 -> [w4374 _]
                tunnel: w4076 -> [w4373 w4378]
                tunnel: w4062 -> [_ w4386]
                tunnel: [w4372 w4377] -> w4079
                tunnel: [w4371 w4381] -> w4081
                tunnel: "AvgTrigLog" -> [_ w4385]
                tunnel: "AvgTrigSel" -> [_ w4384]
                tunnel: w3908 -> [w4371 w4383]
                tunnel: w3907 -> [w4370 w4382]
                tunnel: [w4370 w4380] -> w3906
                tunnel: w3704 -> [_ w4379]
                tunnel: w3904 -> [_ w4376]
                tunnel: [T16 {"Sweeping"=FALSE, "RejAbs"=FALSE, "RejDif"=FALSE} ("Sweep/Reject Cluster Out") w4375] -> w3902
                frame False {
                  n1870 = Bundle By Name(cluster=w4373, "Busy Averaging"=w4374) -> (w4372:T13)
                }
                frame True {
                  n1871 = call "Avg-Sweep-Rev.vi"("Triggers Boolean"=w4379, "Reject Cluster In"=w4376, "AvgTrigLog"=w4385, "AvgTrigSel"=w4384, "Noise Total"=w4382, "Average Total"=w4383, "Processed signals In"=w4386, "Avg Cluster In"=w4378) -> ("Noise Total Out"=w4380:dbl[][], "Average Total Out"=w4381:dbl[][], "Avg Cluster Out"=w4377:T13, "Sweep/Reject Cluster Out"=w4375:T16)
                }
              }
              n1872 = case shown="True" w3808 {
                tunnel: w3766 -> [_ w4230]
                tunnel: w3811 -> [_ w4232]
                tunnel: w3708 -> [_ w4229]
                frame False {
                }
                frame True {
                  w4231 = 9  # Max Nr of Jazz Labels
                  n1873 = property on="Jazz Chart" class="WFChart (strict)"() -> ("Height"=w4233:u32)  [unwired: 2 in, 2 out]
                  n1874 = call "LabelsMon.vi"("Max Nr of Labels"=w4231, "Spec Labels"=w4230, "Channel Selection"=w4232, "Height"=w4233, "[user-specified font]"=w4229) -> ("Mon Labels"=→"JazzLabels":picture, "Y-Max"=w4234:dbl)
                  n1875 = property on="Jazz Chart" class="WFChart (strict)"("YScale.Maximum"=w4234) -> ()  [unwired: 2 in, 2 out]
                }
              }
              n1876 = Not Equal?(x=w3970, y=w4153) -> (x != y?=w4123:bool)
              n1877 = case shown="10" "Reference" {
                tunnel: [i32[] [] i32[] [0, 1, 2, 3, 4, 5, 6, 7, 8, 9, 10, 11, 12, 13, 14, 15, 16, 17, 18, 19, 20, 21, 22, 23, 24, 25, 26, 27, 28, 29, 30, 31, 32, 33, 34, 35, 36, 37, 38, 39, 40, 41, 42, 43, 44, 45, 46, 47, 48, 49, 50, 51, 52, 53, 54, 55, 56, 57, 58, 59, 60, 61, 62, 63, 64, 65, 66, 67, 68, 69, 70, 71, 72, 73, 74, 75, 76, 77, 78, 79, 80, 81, 82, 83, 84, 85, 86, 87, 88, 89, 90, 91, 92, 93, 94, 95, 96, 97, 98, 99, 100, 101, 102, 103, 104, 105, 106, 107, 108, 109, 110, 111, 112, 113, 114, 115, 116, 117, 118, 119, 120, 121, 122, 123, 124, 125, 126, 127, 128, 129, 130, 131, 132, 133, 134, 135, 136, 137, 138, 139, 140, 141, 142, 143, 144, 145, 146, 147, 148, 149, 150, 151, 152, 153, 154, 155, 156, 157, 158, 159, 160, 161, 162, 163, 164, 165, 166, 167, 168, 169, 170, 171, 172, 173, 174, 175, 176, 177, 178, 179, 180, 181, 182, 183, 184, 185, 186, 187, 188, 189, 190, 191, 192, 193, 194, 195, 196, 197, 198, 199, 200, 201, 202, 203, 204, 205, 206, 207, 208, 209, 210, 211, 212, 213, 214, 215, 216, 217, 218, 219, 220, 221, 222, 223, 224, 225, 226, 227, 228, 229, 230, 231, 232, 233, 234, 235, 236, 237, 238, 239, 240, 241, 242, 243, 244, 245, 246, 247, 248, 249, 250, 251, 252, 253, 254, 255, 256, 257, 258, 259, 260, 261, 262, 263] ("Array") i32[] [0, 1, 2, 3, 4, 5, 6, 7, 8, 9, 10, 11, 12, 13, 14, 15, 16, 17, 18, 19, 20, 21, 22, 23, 24, 25, 26, 27, 28, 29, 30, 31, 32, 33, 34, 35, 36, 37, 38, 39, 40, 41, 42, 43, 44, 45, 46, 47, 48, 49, 50, 51, 52, 53, 54, 55, 56, 57, 58, 59, 60, 61, 62, 63, 64, 65, 66, 67, 68, 69, 70, 71, 72, 73, 74, 75, 76, 77, 78, 79, 80, 81, 82, 83, 84, 85, 86, 87, 88, 89, 90, 91, 92, 93, 94, 95, 96, 97, 98, 99, 100, 101, 102, 103, 104, 105, 106, 107, 108, 109, 110, 111, 112, 113, 114, 115, 116, 117, 118, 119, 120, 121, 122, 123, 124, 125, 126, 127, 128, 129, 130, 131, 132, 133, 134, 135, 136, 137, 138, 139, 140, 141, 142, 143, 144, 145, 146, 147, 148, 149, 150, 151, 152, 153, 154, 155, 156, 157, 158, 159, 160, 161, 162, 163, 164, 165, 166, 167, 168, 169, 170, 171, 172, 173, 174, 175, 176, 177, 178, 179, 180, 181, 182, 183, 184, 185, 186, 187, 188, 189, 190, 191, 192, 193, 194, 195, 196, 197, 198, 199, 200, 201, 202, 203, 204, 205, 206, 207, 208, 209, 210, 211, 212, 213, 214, 215, 216, 217, 218, 219, 220, 221, 222, 223, 224, 225, 226, 227, 228, 229, 230, 231, 232, 233, 234, 235, 236, 237, 238, 239, 240, 241, 242, 243, 244, 245, 246, 247, 248, 249, 250, 251, 252, 253, 254, 255] ("All Channels") i32[] [0, 1, 2, 3, 4, 5, 6, 7, 8, 9, 10, 11, 12, 13, 14, 15, 16, 17, 18, 19, 20, 21, 22, 23, 24, 25, 26, 27, 28, 29, 30, 31, 32, 33, 34, 35, 36, 37, 38, 39, 40, 41, 42, 43, 44, 45, 46, 47, 48, 49, 50, 51, 52, 53, 54, 55, 56, 57, 58, 59, 60, 61, 62, 63, 64, 65, 66, 67, 68, 69, 70, 71, 72, 73, 74, 75, 76, 77, 78, 79, 80, 81, 82, 83, 84, 85, 86, 87, 88, 89, 90, 91, 92, 93, 94, 95, 96, 97, 98, 99, 100, 101, 102, 103, 104, 105, 106, 107, 108, 109, 110, 111, 112, 113, 114, 115, 116, 117, 118, 119, 120, 121, 122, 123, 124, 125, 126, 127, 128, 129, 130, 131, 132, 133, 134, 135, 136, 137, 138, 139, 140, 141, 142, 143, 144, 145, 146, 147, 148, 149, 150, 151, 152, 153, 154, 155, 156, 157, 158, 159] ("Array") i32[] [0, 1, 2, 3, 4, 5, 6, 7, 8, 9, 10, 11, 12, 13, 14, 15, 16, 17, 18, 19, 20, 21, 22, 23, 24, 25, 26, 27, 28, 29, 30, 31, 32, 33, 34, 35, 36, 37, 38, 39, 40, 41, 42, 43, 44, 45, 46, 47, 48, 49, 50, 51, 52, 53, 54, 55, 56, 57, 58, 59, 60, 61, 62, 63, 64, 65, 66, 67, 68, 69, 70, 71, 72, 73, 74, 75, 76, 77, 78, 79, 80, 81, 82, 83, 84, 85, 86, 87, 88, 89, 90, 91, 92, 93, 94, 95, 96, 97, 98, 99, 100, 101, 102, 103, 104, 105, 106, 107, 108, 109, 110, 111, 112, 113, 114, 115, 116, 117, 118, 119, 120, 121, 122, 123, 124, 125, 126, 127] ("Array") i32[] [0, 1, 2, 3, 4, 5, 6, 7, 8, 9, 10, 11, 12, 13, 14, 15, 16, 17, 18, 19, 20, 21, 22, 23, 24, 25, 26, 27, 28, 29, 30, 31, 32, 33, 34, 35, 36, 37, 38, 39, 40, 41, 42, 43, 44, 45, 46, 47, 48, 49, 50, 51, 52, 53, 54, 55, 56, 57, 58, 59, 60, 61, 62, 63] ("Array") i32[] [0, 1, 2, 3, 4, 5, 6, 7, 8, 9, 10, 11, 12, 13, 14, 15, 16, 17, 18, 19, 20, 21, 22, 23, 24, 25, 26, 27, 28, 29, 30, 31] ("Array") w4616 "RefFree" w4619 w4624] -> w3684
                tunnel: [w4601 w4603 w4605 w4607 w4609 w4611 w4613 w4615 T6."Enabled" ("Disabled") w4621 w4626] -> w4149
                tunnel: w3895 -> [_ _ _ _ _ _ _ w4616 _ _ _]
                tunnel: w3859 -> [w4601 w4603 w4605 w4607 w4609 w4611 w4613 w4615 _ w4621 w4626]
                tunnel: w3709 -> [_ _ _ _ _ _ _ _ _ w4620 w4625]
                frame 0, Default {
                }
                frame 1 {
                }
                frame 2 {
                }
                frame 3 {
                }
                frame 4 {
                }
                frame 5 {
                }
                frame 6 {
                }
                frame 7 {
                }
                frame 8 {
                }
                frame 9 {
                  n1878 = case shown="0, Default" w4620 {
                    tunnel: [i32[] [121] i32[] [141]] -> w4619
                    frame 0, Default {
                    }
                    frame 1 {
                    }
                  }
                }
                frame 10 {
                  n1879 = case shown="0, Default" w4625 {
                    tunnel: [i32[] [120, 122] i32[] [140, 142]] -> w4624
                    frame 0, Default {
                    }
                    frame 1 {
                    }
                  }
                }
              }
              n1880 = call "Ref-Mon-Deci.vi"("ElecGain"=w3869, "Filter Cluster"=w3685, "Reference"=w3684, "Decimating factor"=w3686, "uV/div"=w3702, "Max Nr of Traces"=w3699, "Sample Rate"=w3681, "Initialize Filters"=w4143, "Center Traces"=w3779, "Channel Selection"=w3895, "N Channel Array In"=w3730) -> ("Screen signals Out"=→"Mon Chart":dbl[][])
              n1881 = Unbundle By Name(w4061) -> ("LoBatChange"=w4132:bool, "JazzLoBatChange"=w3876:bool)
              n1882 = Not Equal?(x=w3895, y=w4139) -> (x != y?=w4152:bool[])
              n1883 = Select(t=T6."Disabled and Grayed Out" ("Disabled"), s=w3952, f=T6."Enabled" ("Disabled")) -> (s? t:f=w4087:T6)
              n1884 = Or Array Elements(Boolean array=w4152) -> (logical OR=w4124:bool)
              n1885 = property on="AnaFree" class="LstBox (strict)"("Disabled"=w4087) -> ()  [unwired: 2 in, 2 out]
              n1886 = Compound Arithmetic op=OR(w4124, w4123, w3723) -> (w3817:bool)
              n1887 = Compound Arithmetic op=OR(w3775, w3817, w3777) -> (w3818:bool)
              n1888 = case shown="True" w3818 {
                tunnel: w3766 -> [_ w4671]
                tunnel: w3895 -> [_ w4676]
                tunnel: w3708 -> [_ w4670]
                frame False {
                }
                frame True {
                  w4672 = 64  # Max Nr of Mon Labels
                  n1889 = property on="Mon Chart" class="WFChart (strict)"() -> ("Height"=w4675:u32)  [unwired: 2 in, 2 out]
                  n1890 = call "LabelsMon.vi"("Max Nr of Labels"=w4672, "Spec Labels"=w4671, "Channel Selection"=w4676, "Height"=w4675, "[user-specified font]"=w4670) -> ("Mon Labels"=→"MonLabels":picture, "Y-Max"=w4673:dbl)
                  n1891 = property on="Mon Chart" class="WFChart (strict)"("YScale.Maximum"=w4673) -> ()  [unwired: 2 in, 2 out]
                }
              }
              n1892 = Compound Arithmetic op=OR(w3733, w3775, w3777) -> (w3776:bool)
              n1893 = case shown="True" w3776 {
                tunnel: "AbrChannels" -> [_ w4196]
                tunnel: w3708 -> [_ w4193]
                frame False {
                }
                frame True {
                  w4198 = 3  # Max Nr of ABR Labels
                  n1894 = case shown="0, Default" w4196 {
                    tunnel: [i32[] [0, 1, 2] ("Disabled Items []") i32[] [0, 2] ("Disabled Items []") i32[] [3, 4] ("Disabled Items []")] -> w4195
                    frame 0, Default {
                    }
                    frame 1 {
                    }
                    frame 2 {
                    }
                  }
                  n1895 = property on="ABR Chart" class="WFChart (strict)"() -> ("Height"=w4199:u32)  [unwired: 2 in, 2 out]
                  n1896 = call "LabelsMon.vi"("Max Nr of Labels"=w4198, "Spec Labels"=string[] ["Lmon", "Ref", "Rmon", "Left", "Right"], "Channel Selection"=w4195, "Height"=w4199, "[user-specified font]"=w4193) -> ("Mon Labels"=→"ABR Labels":picture, "Y-Max"=w4200:dbl)
                  n1897 = property on="ABR Chart" class="WFChart (strict)"("YScale.Maximum"=w4200) -> ()  [unwired: 2 in, 2 out]
                }
              }
              n1898 = Array Size(array=w3684) -> (size(s)=w4148:i32)
              n1899 = Array Size(array=w3916) -> (size(s)=w4051:i32)
              n1900 = Array Size(array=w4140) -> (size(s)=w4147:i32)
              n1901 = Array Size(array=w4125) -> (size(s)=w4127:i32)
              n1902 = property on="RefFree" class="LstBox (strict)"("Disabled"=w4149) -> ()  [unwired: 2 in, 2 out]
              n1903 = Not Equal?(x=w4148, y=w4147) -> (x != y?=w4144:bool)
              n1904 = Not Equal?(x=w4051, y=w4127) -> (x != y?=w4121:bool)
              n1905 = Unbundle By Name(w3902) -> ("Sweeping"=→"Sweeping":bool, "RejAbs"=→"RejAbs":bool, "RejDif"=→"RejDif":bool)
              n1906 = Not Equal?(x=w3684, y=w4140) -> (x != y?=w4146:bool[])
              n1907 = Not Equal?(x=w3916, y=w4125) -> (x != y?=w4126:bool[])
              n1908 = Or Array Elements(Boolean array=w4146) -> (logical OR=w4145:bool)
              n1909 = Or Array Elements(Boolean array=w4126) -> (logical OR=w4122:bool)
              n1910 = Compound Arithmetic op=OR(w4122, w4121, w3723) -> (w3738:bool)
              n1911 = Compound Arithmetic op=OR(w3775, w3738, w3777) -> (w3815:bool)
              n1912 = case shown="True" w3815 {
                tunnel: w3766 -> [_ w4581]
                tunnel: w3916 -> [_ w4580]
                tunnel: w3699 -> [_ w4579]
                tunnel: w3708 -> [_ w4578]
                frame False {
                }
                frame True {
                  n1913 = property on="Bip Chart" class="WFChart (strict)"() -> ("Height"=w4584:u32)  [unwired: 2 in, 2 out]
                  n1914 = call "LabelsBip.vi"("Channel Selection"=w4580, "Spec Labels"=w4581, "MonBipChan"=w4579, "Height"=w4584, "[user-specified font]"=w4578) -> ("Bip Labels"=→"BipLabels":picture, "Y-Max"=w4582:dbl)
                  n1915 = property on="Bip Chart" class="WFChart (strict)"("YScale.Maximum"=w4582) -> ()  [unwired: 2 in, 2 out]
                }
              }
              n1916 = case shown="1" w3706 {
                tunnel: [1 ("t") 2 ("t") 3 ("t") 4 ("t") 2 ("t")] -> w3705
                frame 0, Default {
                }
                frame 1 {
                }
                frame 2 {
                }
                frame 3 {
                }
                frame 15 {
                }
              }
              n1917 = Compound Arithmetic op=OR(w4145, w4144, w3817) -> (w3676:bool)
              n1918 = Not(x=w3885) -> (.not. x?=w4117:bool)
              n1919 = Array Size(array=w3684) -> (size(s)=w4157:i32)
              n1920 = global read "JazzLoBatWarning.glb" "JazzLoBatWarning"() -> (w3877:bool)
              n1921 = And(x=w4117, y=w3981) -> (x .and. y?=w4119:bool)
              "Low Batt" <- w4119
              n1922 = global read "LoBatWarning.glb" "LoBatWarning"() -> (w4134:bool)
              n1923 = Equal?(x=T2."Monopolar", y="Charts/Graphs") -> (x = y?=w4118:bool)
              n1924 = Equal To 0?(x=w4157) -> (x = 0?=w4043:bool)
              n1925 = Compound Arithmetic op=AND(w4118, w4043, w4117) -> (w4040:bool)
              "NoRef Blinker" <- w4040
              n1926 = call "Blinker.vi"("Ratio (>0)"=u32 5, "Period (ms)"=u32 2000, "On/Off In"=w4040) -> ("Blinker Out"=w4041:bool)
              n1927 = Not(x=w3876) -> (.not. x?=w3879:bool)
              n1928 = Not(x=w4132) -> (.not. x?=w4131:bool)
              n1929 = case shown="1, Default" w3739 {
                tunnel: [w4236 w4239] -> w3678
                tunnel: w3867 -> [w4236 w4240]
                tunnel: w3705 -> [_ w4238]
                tunnel: w3704 -> [_ w4237]
                frame 0 {
                }
                frame 1, Default {
                  n1930 = for {
                    N: w4238 -> [_]
                    shift-right: [w4247] -> w4239
                    shift-left: w4240 -> [w4248]
                    tunnel: w4237 -> [w4241]
                    i -> [w4246]
                    # "Trig In 9-16"
                    # "Trig Out 1-8"
                    n1931 = Multiply(x=2, y=w4246) -> (x*y=w4244:i32)
                    n1932 = Add(x=8, y=w4244) -> (x+y=w4242:i32)
                    n1933 = Index Array(array=w4241, index (row) #1=w4242) -> (element #1=w4252:bool[], element #2=w4251:bool[])  [unwired: 3 in]
                    n1934 = Or Array Elements(Boolean array=w4251) -> (logical OR=w4249:bool)
                    n1935 = Or Array Elements(Boolean array=w4252) -> (logical OR=w4250:bool)
                    n1936 = Replace Array Subset(array=w4248, new element #1=w4250, index #1=w4244, new element #2=w4249) -> (w4247:bool[])  [unwired: 1 in]
                  }
                }
              }
              n1937 = And(x=w3872, y=w3879) -> (x .and. y?=w3880:bool)
              n1938 = property on="NoRef Blinker" class="Bool"("Visible"=w4041) -> ()  [unwired: 2 in, 2 out]
              n1939 = And(x=w4119, y=w4131) -> (x .and. y?=w4135:bool)
              n1940 = Select(t=w4162, s=w4104, f=w4120) -> (s? t:f=w4163:i8)
              n1941 = Or(x=w3880, y=w3877) -> (x .or. y?=w3878:bool)
              n1942 = global write "JazzLoBatWarning.glb" "JazzLoBatWarning"(w3878) -> ()
              n1943 = Or(x=w4135, y=w4134) -> (x .or. y?=w4133:bool)
              n1944 = global write "LoBatWarning.glb" "LoBatWarning"(w4133) -> ()
              n1945 = Bundle(w4119, w3872) -> (w4136:cluster{bool, bool})  [unwired: 1 out]
              n1946 = Array Size(array=w3816) -> (size(s)=w4050:i32)
              n1947 = Array Size(array=w4091) -> (size(s)=w4095:i32)
              n1948 = case shown="0, Default" "AbrChannels" {
                tunnel: [w4176 w4192] -> w3737
                tunnel: w3695 -> [w4174 w4192]
                tunnel: w3733 -> [w4175 _]
                tunnel: [T6."Enabled" ("Disabled") T6."Disabled and Grayed Out" ("Disabled")] -> w3734
                frame 0, Default {
                  n1949 = case shown="True" w4175 {
                    tunnel: [w4181 w4183] -> w4176
                    tunnel: w4174 -> [w4180 w4183]
                    frame False {
                      n1950 = Bundle By Name(cluster=w4180, "AbrLP"="AbrLP", "AbrLPfreq"="AbrLPfreq", "AbrHP"="AbrHP", "AbrHPfreq"="AbrHPfreq") -> (w4181:T7)
                    }
                    frame True {
                      n1951 = Unbundle By Name(w4183) -> ("AbrLP"=w4187:bool, "AbrLPfreq"=w4186:dbl, "AbrHP"=w4185:bool, "AbrHPfreq"=w4184:dbl)
                      n1952 = local write "AbrLP"(w4187) -> ()
                      n1953 = local write "AbrLPfreq"(w4186) -> ()
                      n1954 = local write "AbrHP"(w4185) -> ()
                      n1955 = local write "AbrHPfreq"(w4184) -> ()
                    }
                  }
                }
                frame 2 {
                  w4191 = TRUE ("AbrLP")
                  n1956 = local write "AbrLP"(w4191) -> ()
                  n1957 = local write "AbrLPfreq"(3334.0 ("AbrLPfreq")) -> ()
                  n1958 = local write "AbrHP"(w4191) -> ()
                  n1959 = local write "AbrHPfreq"(100.0 ("AbrHPfreq")) -> ()
                }
              }
              n1960 = Not Equal?(x=w4050, y=w4095) -> (x != y?=w4092:bool)
              n1961 = Equal To 0?(x="AbrChannels") -> (x = 0?=w3744:bool)
              n1962 = Not Equal?(x=w3816, y=w4091) -> (x != y?=w4094:bool[])
              n1963 = Or Array Elements(Boolean array=w4094) -> (logical OR=w4093:bool)
              n1964 = case shown="True" w3963 {
                selector: w3963 -> [_ w4261]
                tunnel: [w4259 FALSE ("Start Saving")] -> w3948
                frame False {
                  n1965 = local read "Start Saving"() -> (w4259:bool)
                }
                frame True {
                  n1966 = local write "Start Saving"(w4261) -> ()
                }
              }
              n1967 = Not(x=w3723) -> (.not. x?=w3780:bool)
              n1968 = Not Equal?(x="Box", y=w3969) -> (x != y?=w3965:bool)
              n1969 = Select(t=u32 65280, s=w3744, f=w3742) -> (s? t:f=w3743:u32)
              n1970 = Compound Arithmetic op=OR(w4093, w4092, w3723) -> (w3813:bool)
              n1971 = Compound Arithmetic op=OR(w3775, w3813, w3777) -> (w3814:bool)
              n1972 = case shown="True" w3814 {
                tunnel: w3766 -> [_ w4411]
                tunnel: w3816 -> [_ w4414]
                tunnel: w3708 -> [_ w4409]
                frame False {
                }
                frame True {
                  w4415 = 32  # Max Nr of Ana Labels
                  n1973 = property on="Ana Chart" class="WFChart (strict)"() -> ("Height"=w4413:u32)  [unwired: 2 in, 2 out]
                  n1974 = call "LabelsMon.vi"("Max Nr of Labels"=w4415, "Spec Labels"=w4411, "Channel Selection"=w4414, "Height"=w4413, "[user-specified font]"=w4409) -> ("Mon Labels"=→"AnaLabels":picture, "Y-Max"=w4412:dbl)
                  n1975 = property on="Ana Chart" class="WFChart (strict)"("YScale.Maximum"=w4412) -> ()  [unwired: 2 in, 2 out]
                }
              }
              n1976 = And(x=w3965, y=w3780) -> (x .and. y?=w3964:bool)
              n1977 = Or(x=w3964, y="Master Filter Reset") -> (x .or. y?=w3967:bool)
              n1978 = And(x=w3676, y=w3780) -> (x .and. y?=w4039:bool)
              n1979 = And(x=w3738, y=w3780) -> (x .and. y?=w4035:bool)
              n1980 = And(x=w3780, y=w3733) -> (x .and. y?=w3787:bool)
              n1981 = And(x=w3780, y=w3781) -> (x .and. y?=w4036:bool)
              n1982 = And(x=w3780, y=w3809) -> (x .and. y?=w3928:bool)
              n1983 = And(x=w3780, y=w3813) -> (x .and. y?=w4037:bool)
              n1984 = property on="AbrLP" class="Bool (strict)"("Disabled"=w3734) -> ()  [unwired: 2 in, 2 out]
              n1985 = property on="AbrLPfreq" class="DigNum (strict)"("Disabled"=w3734) -> ()  [unwired: 2 in, 2 out]
              n1986 = property on="AbrHP" class="Bool (strict)"("Disabled"=w3734) -> ()  [unwired: 2 in, 2 out]
              n1987 = property on="AbrHPfreq" class="DigNum (strict)"("Disabled"=w3734) -> ()  [unwired: 2 in, 2 out]
              n1988 = property on="ABR Chart" class="WFChart (strict)"("Active Plot"=u32 0, "Plot.Plot Color"=u32 255, "Active Plot"=u32 1, "Plot.Plot Color"=w3743, "Active Plot"=u32 2, "Plot.Plot Color"=w3742) -> ()  [unwired: 2 in, 2 out]
              n1989 = case shown="\"ABR\"" "Charts/Graphs" {
                tunnel: w4039 -> [w4339 _ _ _ _ _ _]
                tunnel: "Mon Filter Reset" -> [w4342 _ _ _ _ _ _]
                tunnel: [w4341 w4343 w4350 w4353 w4358 w4364 w4368] -> w4038
                tunnel: w4037 -> [_ _ _ _ _ w4363 _]
                tunnel: "Ana Filter Reset" -> [_ _ _ _ _ w4367 _]
                tunnel: w4036 -> [_ _ _ w4357 _ _ _]
                tunnel: "Aux DC Reset" -> [_ _ _ w4356 _ _ _]
                tunnel: w4035 -> [_ w4347 _ _ _ _ _]
                tunnel: "Bip Filter Reset" -> [_ w4346 _ _ _ _ _]
                tunnel: [w4338 w4345 w4350 w4353 w4358 w4364 w4368] -> w4034
                tunnel: [w4338 w4343 w4350 w4353 w4358 w4366 w4368] -> w4033
                tunnel: [w4338 w4343 w4350 w4355 w4358 w4364 w4368] -> w4032
                tunnel: w3967 -> [w4340 w4344 w4352 w4354 w4362 w4365 _]
                tunnel: [w4338 w4343 w4350 w4353 w4359 w4364 w4368] -> w3930
                tunnel: "Jazz Filter Reset" -> [_ _ _ _ w4360 _ _]
                tunnel: w3928 -> [_ _ _ _ w4361 _ _]
                tunnel: "ABR Filter Reset" -> [_ _ w4349 _ _ _ _]
                tunnel: [w4338 w4343 w4351 w4353 w4358 w4364 w4368] -> w3791
                tunnel: w3787 -> [_ _ w4348 _ _ _ _]
                frame "Monopolar" {
                  w4338 = FALSE
                  n1990 = Compound Arithmetic op=OR(w4340, w4342, w4339) -> (w4341:bool)
                }
                frame "Bipolar" {
                  w4343 = FALSE
                  n1991 = Compound Arithmetic op=OR(w4344, w4346, w4347) -> (w4345:bool)
                }
                frame "ABR" {
                  w4350 = FALSE
                  n1992 = Compound Arithmetic op=OR(w4352, w4349, w4348) -> (w4351:bool)
                }
                frame "Sensors" {
                  w4353 = FALSE
                  n1993 = Compound Arithmetic op=OR(w4354, w4356, w4357) -> (w4355:bool)
                }
                frame "Jazz" {
                  w4358 = FALSE
                  n1994 = Compound Arithmetic op=OR(w4362, w4360, w4361) -> (w4359:bool)
                }
                frame "AIB" {
                  w4364 = FALSE
                  n1995 = Compound Arithmetic op=OR(w4365, w4367, w4363) -> (w4366:bool)
                }
                frame "About/Configure", Default {
                  w4368 = FALSE
                }
              }
              n1996 = Bundle("Marker F1"="Marker F1", "Marker F2"="Marker F2", "Marker F3"="Marker F3", "Marker F4"="Marker F4", "Marker F5"="Marker F5", "Marker F6"="Marker F6", "Marker F7"="Marker F7", "Marker F8"="Marker F8") -> (w4022:T38)  [unwired: 1 out]
              n1997 = call "Act_Error_5000.vi"("Error Code In"=w3740, "error in (no error)"=w4008) -> ("error out"=w4099:errorcluster)  [unwired: 2 out]
              n1998 = Or(x=w3950, y=w3948) -> (x .or. y?=w3949:bool)
            }
            frame 2 {
              w4721 = 0.0 ("XScale.Maximum")
              w4765 = i64 0 ("Prop Screen Minimum")
              # "Start Epoch"
              # "Save Blocksize in Bytes"
              # "Nr of Saved Bytes"
              # "Write Error"
              # "New Total Saved in Sec"
              # "Old Total Saved in Sec"
              # "Index"
              # "Save Buffer"
              # "Second Half ?"
              # "Save Blocksize in Bytes"
              # "Pause Saving"
              # "Bytes, 3 per Channel"
              # "Save"
              # "Header Lenght in Byte"
              # "Nr of Byte Saved in this Scan"
              # "New Current File in Byte"
              # "Old Current File in Byte"
              n1999 = Array Size(array=w4695) -> (size(s)=w4710:i32)
              n2000 = Not(x=w4741) -> (.not. x?=w4743:bool)
              n2001 = Select(t=w4728, s=w4741, f=0) -> (s? t:f=w4740:i32)
              n2002 = Compound Arithmetic op=MULTIPLY(3 ("y"), w4710, w4707) -> (w4708:i32)
              n2003 = Select(t=0, s=w4694, f=w4728) -> (s? t:f=w4738:i32)
              n2004 = Increment(x=w4708) -> (x+1=w4693:i32)
              n2005 = Not(x=w4694) -> (.not. x?=w4705:bool)
              n2006 = Increment(x=w4693) -> (x+1=w4699:i32)
              n2007 = Array Subset(array=w4742, index=w4740, length=w4738) -> (w4702:u8[])
              n2008 = And(x=w4705, y=w4706) -> (x .and. y?=w4696:bool)
              n2009 = Index Array(array=w4702, index=w4699) -> (element=w4698:u8)
              n2010 = Number To Boolean Array(number=w4698) -> (Boolean array=w4704:bool[])
              n2011 = Replace Array Subset(array=w4704, new element=w4696) -> (w4703:bool[])  [unwired: 1 in]
              n2012 = Boolean Array To Number(Boolean array=w4703) -> (number=w4701:u32)
              n2013 = To Unsigned Byte Integer(number=w4701) -> (unsigned 8bit integer=w4697:u8)
              n2014 = Unbundle By Name(w4717) -> ("RespSwitch"=w4716:i8, "TrigLength"=w4715:i32)
              n2015 = Replace Array Subset(array=w4702, new element=w4697, index=w4699) -> (w4700:u8[])
              n2016 = Array Size(array=w4702) -> (size(s)=w4745:i32)
              n2017 = case shown="3" w4716 {
                tunnel: w4700 -> [w4787 w4796]
                tunnel: [w4787 w4800] -> w4713
                tunnel: w4707 -> [_ w4798]
                tunnel: w4715 -> [_ w4799]
                tunnel: w4712 -> [_ w4794]
                tunnel: w4693 -> [_ w4788]
                frame 0, Default {
                }
                frame 3 {
                  # "Start Epoch"
                  n2018 = Unbundle By Name(w4794) -> ("Speed Mode"=w4793:i8)
                  n2019 = Index Array(array=w4796, index #1=w4788) -> (element #1=w4790:u8, element #2=w4797:u8)  [unwired: 1 in]
                  n2020 = Number To Boolean Array(number=w4790) -> (Boolean array=w4789:bool[])
                  n2021 = Number To Boolean Array(number=w4797) -> (Boolean array=w4801:bool[])
                  n2022 = Index Array(array=w4801) -> (element=w4795:bool)  [unwired: 1 in]
                  n2023 = case shown="0, Default" w4793 {
                    tunnel: w4795 -> [w4807 w4816 w4824 w4830 w4836]
                    tunnel: [w4804 w4812 w4820 w4829 w4832] -> w4792
                    tunnel: [w4802 w4813 w4821 w4828 w4833] -> w4791
                    tunnel: w4789 -> [w4810 w4818 w4826 w4827 w4838]
                    frame 0, Default {
                      w4803 = TRUE
                      # "Trig 9+10"
                      n2024 = Index Array(array=w4810) -> (element #1=w4809:bool, element #2=w4808:bool)  [unwired: 2 in]
                      n2025 = Not And(1:w4809, 2:w4807) -> (0:w4806:bool)
                      n2026 = Not And(1:w4808, 2:w4807) -> (0:w4805:bool)
                      n2027 = And(x=w4806, y=w4805) -> (x .and. y?=w4804:bool)
                      n2028 = Build Array(w4806, w4805, w4803, w4803, w4803, w4803, w4803, w4803) -> (w4802:bool[])
                    }
                    frame 1 {
                      w4811 = TRUE
                      # "Trig 9-12"
                      n2029 = Array Subset(array=w4818, length=4) -> (w4817:bool[])  [unwired: 1 in]
                      n2030 = Not And(1:w4817, 2:w4816) -> (0:w4814:bool[])
                      n2031 = Build Array (concatenate)(w4814, w4811, w4811, w4811, w4811) -> (w4813:bool[])
                      n2032 = And Array Elements(Boolean array=w4814) -> (logical AND=w4812:bool)
                    }
                    frame 2 {
                      w4819 = TRUE
                      # "Trig 9-14"
                      n2033 = Array Subset(array=w4826, length=6) -> (w4825:bool[])  [unwired: 1 in]
                      n2034 = Not And(1:w4825, 2:w4824) -> (0:w4822:bool[])
                      n2035 = Build Array (concatenate)(w4822, w4819, w4819) -> (w4821:bool[])
                      n2036 = And Array Elements(Boolean array=w4822) -> (logical AND=w4820:bool)
                    }
                    frame 3 {
                      # "Trig 9-16"
                      n2037 = Not And(1:w4827, 2:w4830) -> (0:w4828:bool[])
                      n2038 = And Array Elements(Boolean array=w4828) -> (logical AND=w4829:bool)
                    }
                    frame 15 {
                      w4831 = TRUE
                      # "Trig 9-12"
                      n2039 = Array Subset(array=w4838, length=4) -> (w4837:bool[])  [unwired: 1 in]
                      n2040 = Not And(1:w4837, 2:w4836) -> (0:w4834:bool[])
                      n2041 = Build Array (concatenate)(w4834, w4831, w4831, w4831, w4831) -> (w4833:bool[])
                      n2042 = And Array Elements(Boolean array=w4834) -> (logical AND=w4832:bool)
                    }
                  }
                  n2043 = case shown="False" w4792 {
                    tunnel: w4796 -> [w4843 w4861]
                    tunnel: [w4842 w4861] -> w4800
                    tunnel: w4799 -> [w4845 _]
                    tunnel: w4798 -> [w4844 _]
                    tunnel: w4788 -> [w4841 _]
                    tunnel: w4791 -> [w4839 _]
                    frame False {
                      # "Tigger Length\nin Samples"
                      n2044 = Multiply(x=w4845, y=w4844) -> (x*y=w4847:i32)
                      n2045 = Quotient & Remainder(x=w4847, y=1000) -> (floor(x/y)=w4840:i32)  [unwired: 1 out]
                      n2046 = for {
                        N: w4840 -> [_]
                        shift-right: [w4860] -> w4842
                        shift-left: w4843 -> [w4859]
                        tunnel: w4841 -> [w4858]
                        tunnel: w4839 -> [w4856]
                        i -> [w4851]
                        n2047 = Multiply(x=3, y=w4851) -> (x*y=w4849:i32)
                        n2048 = Add(x=w4858, y=w4849) -> (x+y=w4852:i32)
                        n2049 = Index Array(array=w4859, index=w4852) -> (element=w4848:u8)
                        n2050 = Number To Boolean Array(number=w4848) -> (Boolean array=w4857:bool[])
                        n2051 = And(x=w4857, y=w4856) -> (x .and. y?=w4855:bool[])
                        n2052 = Boolean Array To Number(Boolean array=w4855) -> (number=w4854:u32)
                        n2053 = To Unsigned Byte Integer(number=w4854) -> (unsigned 8bit integer=w4853:u8)
                        n2054 = Replace Array Subset(array=w4859, new element=w4853, index=w4852) -> (w4860:u8[])
                      }
                    }
                    frame True {
                    }
                  }
                }
              }
              n2055 = case shown="0" w4746 {
                tunnel: w4747 -> [w4869 w4875]
                tunnel: w4744 -> [w4868 w4874]
                tunnel: [w4867 w4874] -> w4736
                tunnel: [w4866 w4875] -> w4735
                frame 0 {
                  n2056 = Get Date/Time In Seconds() -> (seconds since 1Jan1904=w4862:timestamp)
                  n2057 = Decrement(x=w4862) -> (x-1=w4864:timestamp)
                  n2058 = Format Date/Time String(time format string (%c)="%d.%m.%y%H.%M.%S", seconds (now)=w4864) -> (date/time string=w4863:string)  [unwired: 1 out]
                  n2059 = Format Into String(format string="%-16.16s", w4863) -> (resulting string=w4870:string)  [unwired: 2 in, 1 out]
                  n2060 = call "Write File+ [String].vi"("String"=w4870, "error in (no error)"=w4868, "pos offset (bytes:0)"=i64 168, "pos mode (rel. to end:1)"=enum16{"start", "end", "current"}."start", "refnum"=w4869) -> ("error out"=w4867:errorcluster, "dup refnum"=w4866:refnum<file>)  [unwired: 2 out]
                }
                frame 1, Default {
                }
              }
              n2061 = call "Write File+ [U8].vi"("1D array"=w4713, "error in (no error)"=w4736, "refnum"=w4735) -> ("error out"=w4782:errorcluster, "dup refnum"=w4730:refnum<file>)  [unwired: 2 in, 2 out]
              n2062 = Unbundle By Name(w4782) -> ("status"=w4749:bool)
              n2063 = Select(t=0, s=w4749, f=w4745) -> (s? t:f=w4752:i32)
              n2064 = To Quad Integer(1:w4752) -> (0:w4733:i64)
              n2065 = Refnum to Path(1:w4730) -> (0:w4731:path)
              n2066 = Add(x=w4775, y=w4733) -> (x+y=w4761:i64)
              n2067 = Get Volume Info(11:w4731) -> (1:w4729:i64)  [unwired: 1 in, 5 out]
              n2068 = To Quad Integer(1:w4728) -> (0:w4727:i64)
              n2069 = Quotient & Remainder(x=w4729, y=w4727) -> (floor(x/y)=→"Free HDD [sec]":i64)  [unwired: 1 out]
              n2070 = Quotient & Remainder(x=w4752, y=w4728) -> (floor(x/y)=w4751:i32)  [unwired: 1 out]
              n2071 = Add(x=w4746, y=w4751) -> (x+y=w4750:i32)
              n2072 = Scale By Power Of 2(n=i16 20, x=1.0) -> (x*2^n=w4779:dbl)
              n2073 = To Double Precision Float(number=w4761) -> (double precision float=w4777:dbl)
              n2074 = Divide(x=w4777, y=w4779) -> (x/y=→"Current File [MB]":dbl)
            }
            frame 3 {
              w4880 = 0.0 ("XScale.Maximum")
              w4896 = 1000  # Max Nr of Files
              w4922 = i64 0 ("Prop Screen Minimum")
              # "Start New File ?"
              # "File Error"
              # "Save Blocksize in Byte"
              # "Current File in Byte"
              # "Header Lenght in Byte"
              # "End of File"
              n2075 = Not(x=w4900) -> (.not. x?=w4897:bool)
              n2076 = Add(x=w4892, y=w4888) -> (x+y=w4891:i32)
              n2077 = To Quad Integer(1:w4891) -> (0:w4887:i64)
              n2078 = Greater Or Equal?(x=w4890, y=w4887) -> (x >= y?=w4893:bool)
              n2079 = Less?(x=w4895, y=w4896) -> (x < y?=w4894:bool)
              n2080 = Compound Arithmetic op=AND(w4893, w4894, "FileAppend", w4897) -> (w4898:bool)
              n2081 = case shown="True" w4898 {
                tunnel: w4907 -> [w4944 w4963]
                tunnel: w4908 -> [w4945 w4962]
                tunnel: [w4944 w4970] -> w4906
                tunnel: [w4940 w4990] -> w4905
                tunnel: [w4943 w4969] -> w4904
                tunnel: w4895 -> [w4942 w4972]
                tunnel: [w4942 w5001] -> w4903
                tunnel: w4902 -> [w4941 w4992]
                tunnel: w4892 -> [_ w4964]
                tunnel: w4888 -> [_ w4991]
                tunnel: [w4941 w4947] -> w4901
                frame False {
                  w4946 = FALSE
                  w4940 = TRUE  # File at Limit Error
                  n2082 = Build Array(w4946, w4946, w4946, w4940) -> (w4939:bool[])
                  n2083 = call "Act_Error_5000.vi"("Error Code In"=w4939, "error in (no error)"=w4945) -> ("error out"=w4943:errorcluster)  [unwired: 2 out]
                }
                frame True {
                  # "new date/time"
                  # "Old Header"
                  # "New Current File in Byte"
                  # "Old Number of Files"
                  # "Old Path"
                  # "number of data records"
                  n2084 = To Quad Integer(1:w4964) -> (0:w4947:i64)
                  n2085 = To Quad Integer(1:w4991) -> (0:w4948:i64)
                  n2086 = Subtract(x=w4992, y=w4947) -> (x-y=w5000:i64)
                  n2087 = Quotient & Remainder(x=w5000, y=w4948) -> (floor(x/y)=w4993:i64)  [unwired: 1 out]
                  n2088 = Format Into String(format string="%-8d", w4993) -> (resulting string=w4998:string)  [unwired: 2 in, 1 out]
                  n2089 = call "Read File+ [String].vi"("count"=w4964, "error in (no error)"=w4962, "pos mode (rel. to current:2)"=enum16{"start", "end", "current"}."start", "refnum"=w4963) -> ("error out"=w4960:errorcluster, "string"=w4957:string, "dup refnum"=w4959:refnum<file>)  [unwired: 1 in, 2 out]
                  n2090 = call "Write File+ [String].vi"("String"=w4998, "error in (no error)"=w4960, "pos offset (bytes:0)"=i64 236, "pos mode (rel. to end:1)"=enum16{"start", "end", "current"}."start", "refnum"=w4959) -> ("error out"=w4997:errorcluster, "dup refnum"=w4996:refnum<file>)  [unwired: 2 out]
                  n2091 = Close File(refnum=w4996, error in=w4997) -> (path=w4973:path, error out=w4949:errorcluster)
                  n2092 = Strip Path(path=w4973) -> (stripped path=w4984:path, name=w4987:string)
                  n2093 = Greater?(x=w4972, y=1) -> (0:w4982:bool)
                  n2094 = Select(t=8 ("y"), s=w4982, f=4) -> (s? t:f=w4980:i32)
                  n2095 = String Length(string=w4987) -> (length=w4989:i32)
                  n2096 = Format Into String(format string="%03d" ("Format String"), w4972) -> (resulting string=w4977:string)  [unwired: 2 in, 1 out]
                  n2097 = Subtract(x=w4989, y=w4980) -> (x-y=w4988:i32)
                  n2098 = String Subset(string=w4987, length (rest)=w4988) -> (substring=w4986:string)  [unwired: 1 out]
                  n2099 = Concatenate Strings("+", w4977, ".bdf") -> (w4974:string)
                  n2100 = Format Date/Time String(time format string (%c)="%d.%m.%y%H.%M.%S") -> (date/time string=w4966:string)  [unwired: 2 out]
                  n2101 = Format Into String(format string="%-16.16s", w4966) -> (resulting string=w4958:string)  [unwired: 2 in, 1 out]
                  n2102 = Concatenate Strings(w4986, w4974) -> (w4985:string)
                  n2103 = Build Path(base path=w4984, name or relative path=w4985) -> (appended path=w4953:path)
                  n2104 = Path To String(path=w4953) -> (string=w4965:string)
                  n2105 = local write "BDF Filepath"(w4965) -> ()
                  n2106 = Increment(x=w4972) -> (x+1=w5001:i32)
                  n2107 = Replace Substring(2:16 ("length (len. of substring)"), 3:i64 168 ("pos offset (bytes:0)"), 4:w4958, 5:w4957) -> (1:w4954:string)  [unwired: 1 out]
                  n2108 = Open/Create/Replace File(file path (use dialog)=w4953, error in=w4949, operation (0:open)=T12."replace or create") -> (refnum out=w4950:refnum<file>, error out=w4951:errorcluster)  [unwired: 4 out]
                  n2109 = call "Write File+ [String].vi"("String"=w4954, "error in (no error)"=w4951, "pos mode (rel. to end:1)"=enum16{"start", "end", "current"}."start", "refnum"=w4950) -> ("error out"=w4969:errorcluster, "dup refnum"=w4970:refnum<file>)  [unwired: 1 in, 2 out]
                  n2110 = Unbundle By Name(w4969) -> ("status"=w4990:bool)
                }
              }
            }
            frame 4 {
              w5042 = 1000.0 ("y")
              w5007 = 0.0 ("XScale.Maximum")
              w5039 = 2  # Nr of AVG Chan
              w5050 = i64 0 ("Prop Screen Minimum")
              # "Noise Total"
              # "Average Total"
              # "Average"
              n2111 = Unbundle By Name(w5017) -> ("Sweep Lenght in Samples"=w5019:i32, "Valid Sweeps"=→"Valid Sweeps":i32, "Rejected Sweeps"=→"Rejected Sweeps":i32, "First Graph Update"=w5018:bool)
              n2112 = To Double Precision Float(number=w5019) -> (double precision float=w5033:dbl)
              n2113 = Bundle By Name(cluster=w5017, "First Graph Update"=FALSE ("Start Averaging")) -> (w5016:T13)
              n2114 = Multiply(x=w5033, y=w5042) -> (x*y=w5043:dbl)
              n2115 = Divide(x=w5043, y=w5038) -> (x/y=w5040:dbl)
              n2116 = Divide(x=w5042, y=w5038) -> (x/y=w5041:dbl)
              n2117 = for {
                tunnel: w5023 -> [w5073] mode=indexing
                tunnel: w5022 -> [w5072] mode=indexing
                tunnel: [w5071] -> w5012 mode=indexing
                tunnel: w5033 -> [w5070]
                tunnel: [w5069] -> w5011 mode=indexing
                n2118 = Add Array Elements(numeric array=w5073) -> (sum=w5074:dbl)
                n2119 = Add Array Elements(numeric array=w5072) -> (sum=w5076:dbl)
                n2120 = Divide(x=w5074, y=w5070) -> (x/y=w5075:dbl)
                n2121 = Divide(x=w5076, y=w5070) -> (x/y=w5077:dbl)
                n2122 = Subtract(x=w5073, y=w5075) -> (x-y=w5069:dbl[])
                n2123 = Subtract(x=w5072, y=w5077) -> (x-y=w5071:dbl[])
              }
              n2124 = Array Max & Min(array=w5011) -> (max value=w5014:dbl, min value=w5013:dbl)  [unwired: 2 out]
              n2125 = for {
                N: w5039 -> [_]
                tunnel: "AvgAutoscale" -> [w5093]
                tunnel: "AvgScale" -> [w5092]
                tunnel: w5040 -> [w5090]
                tunnel: w5041 -> [w5089]
                tunnel: w5018 -> [w5086]
                tunnel: w5014 -> [w5083]
                tunnel: w5013 -> [w5082]
                tunnel: w5011 -> [w5081]
                tunnel: w5012 -> [w5080]
                i -> [w5084]
                n2126 = case shown="False" w5093 {
                  tunnel: w5083 -> [_ w5117]
                  tunnel: [w5114 w5117] -> w5088
                  tunnel: w5082 -> [_ w5116]
                  tunnel: [w5115 w5116] -> w5087
                  tunnel: w5092 -> [w5114 _]
                  frame False {
                    n2127 = Negate(x=w5114) -> (-x=w5115:dbl)
                  }
                  frame True {
                  }
                }
                n2128 = Index Array(array=w5080, index (row)=w5084) -> (element=w5078:dbl[])  [unwired: 1 in]
                n2129 = Index Array(array=w5081, index (row)=w5084) -> (element=w5079:dbl[])  [unwired: 1 in]
                n2130 = Increment(x=w5084) -> (x+1=w5091:i32)
                n2131 = Build Array(w5079, w5078) -> (w5085:dbl[][])
                n2132 = case shown="2" w5091 {
                  tunnel: w5085 -> [w5096 w5106]
                  tunnel: w5089 -> [w5098 w5108]
                  tunnel: w5090 -> [w5099 w5109]
                  tunnel: w5087 -> [w5094 w5104]
                  tunnel: w5088 -> [w5095 w5105]
                  tunnel: w5086 -> [w5097 w5107]
                  frame 1, Default {
                    n2133 = case shown="True" w5097 {
                      tunnel: w5099 -> [_ w5101]
                      tunnel: w5098 -> [_ w5100]
                      frame False {
                      }
                      frame True {
                        n2134 = stacked-sequence {
                          tunnel: w5101 -> [_ w5103]
                          tunnel: w5100 -> [w5102 _]
                          frame #0 {
                            n2135 = property on="Avg1" class="WFGraph (strict)"("X Scale.Offset and Multiplier:Multiplier"=w5102) -> ()  [unwired: 2 in, 2 out]
                          }
                          frame #1 {
                            n2136 = property on="Avg1" class="WFGraph (strict)"("X Scale.Range:Maximum"=w5103) -> ()  [unwired: 2 in, 2 out]
                          }
                        }
                      }
                    }
                    n2137 = property on="Avg1" class="WFGraph (strict)"("Y Scale.Range:Maximum"=w5095, "YScale.Minimum"=w5094) -> ()  [unwired: 2 in, 2 out]
                    "Avg1" <- w5096
                  }
                  frame 2 {
                    n2138 = case shown="True" w5107 {
                      tunnel: w5109 -> [_ w5111]
                      tunnel: w5108 -> [_ w5110]
                      frame False {
                      }
                      frame True {
                        n2139 = stacked-sequence {
                          tunnel: w5111 -> [_ w5113]
                          tunnel: w5110 -> [w5112 _]
                          frame #0 {
                            n2140 = property on="Avg2" class="WFGraph (strict)"("X Scale.Offset and Multiplier:Multiplier"=w5112) -> ()  [unwired: 2 in, 2 out]
                          }
                          frame #1 {
                            n2141 = property on="Avg2" class="WFGraph (strict)"("X Scale.Range:Maximum"=w5113) -> ()  [unwired: 2 in, 2 out]
                          }
                        }
                      }
                    }
                    n2142 = property on="Avg2" class="WFGraph (strict)"("Y Scale.Range:Maximum"=w5105, "YScale.Minimum"=w5104) -> ()  [unwired: 2 in, 2 out]
                    "Avg2" <- w5106
                  }
                }
              }
            }
          }
          "Nr of Files" <- w3366
          n2143 = Unbundle By Name(w3300) -> ("Clear Block"=w3423:dbl, "Screen Ratio"=w3422:dbl, "Y1"=w3420:dbl, "Y2"=w3418:dbl, "Y3"=w3419:dbl, "Color"=w3421:u32)
          n2144 = case shown="True" w3432 {
            tunnel: w3445 -> [_ w3526]
            tunnel: w3389 -> [_ w3562]
            tunnel: w3446 -> [_ w3561]
            tunnel: w3302 -> [_ w3559]
            tunnel: w3447 -> [_ w3560]
            tunnel: w3448 -> [_ w3558]
            tunnel: w3440 -> [_ w3557]
            tunnel: w3425 -> [w3523 w3549]
            tunnel: [w3523 w3545] -> w3429
            tunnel: w3422 -> [_ w3555]
            tunnel: w3423 -> [_ w3529]
            tunnel: w3426 -> [w3522 w3552]
            tunnel: [w3522 w3543] -> w3428
            tunnel: w3424 -> [w3521 w3553]
            tunnel: [w3521 w3554] -> w3427
            tunnel: w3420 -> [_ w3547]
            tunnel: w3421 -> [_ w3541]
            tunnel: w3419 -> [_ w3539]
            tunnel: w3418 -> [_ w3537]
            tunnel: w3417 -> [_ w3525]
            tunnel: w3333 -> [_ w3535]
            tunnel: w3295 -> [_ w3528]
            frame False {
            }
            frame True {
              w3540 = TRUE ("fill?(F)")
              w3536 = i16 0
              n2145 = To Double Precision Float(number=w3562) -> (double precision float=w3533:dbl)
              n2146 = To Double Precision Float(number=w3526) -> (double precision float=w3524:dbl)
              n2147 = Divide(x=w3529, y=w3555) -> (x/y=w3556:dbl)
              n2148 = To Word Integer(number=w3547) -> (16bit integer=w3532:i16)
              n2149 = To Word Integer(number=w3537) -> (16bit integer=w3531:i16)
              n2150 = To Word Integer(number=w3539) -> (16bit integer=w3530:i16)
              n2151 = To Word Integer(number=w3556) -> (16bit integer=w3538:i16)
              n2152 = case shown="\"Monopolar\"" w3559 {
                tunnel: w3533 -> [w3575 w3583 w3592 w3601 w3610 w3619 _]
                tunnel: w3524 -> [w3571 w3581 w3589 w3599 w3608 w3616 _]
                tunnel: w3561 -> [w3572 _ _ _ _ _ _]
                tunnel: w3560 -> [_ w3580 _ _ _ _ _]
                tunnel: w3558 -> [_ _ _ w3598 _ _ _]
                tunnel: w3557 -> [_ _ _ _ _ w3617 _]
                tunnel: w3535 -> [_ _ _ _ w3607 _ _]
                tunnel: w3528 -> [_ _ w3590 _ _ _ _]
                frame "Monopolar" {
                  n2153 = Add(x=w3571, y=w3575) -> (x+y=w3574:dbl)
                  n2154 = Not Equal?(x=w3571, y=w3572) -> (x != y?=w3573:bool)
                  n2155 = case shown="True" w3573 {
                    tunnel: w3571 -> [_ w3577]
                    tunnel: w3574 -> [_ w3576]
                    frame False {
                    }
                    frame True {
                      n2156 = stacked-sequence {
                        tunnel: w3577 -> [w3578 _]
                        tunnel: w3576 -> [_ w3579]
                        frame #0 {
                          n2157 = property on="Mon Chart" class="WFChart (strict)"("X Scale.Range:Minimum"=w3578) -> ()  [unwired: 2 in, 2 out]
                        }
                        frame #1 {
                          n2158 = property on="Mon Chart" class="WFChart (strict)"("X Scale.Range:Maximum"=w3579) -> ()  [unwired: 2 in, 2 out]
                        }
                      }
                    }
                  }
                }
                frame "Bipolar" {
                  n2159 = Add(x=w3581, y=w3583) -> (x+y=w3584:dbl)
                  n2160 = Not Equal?(x=w3581, y=w3580) -> (x != y?=w3582:bool)
                  n2161 = case shown="True" w3582 {
                    tunnel: w3581 -> [_ w3586]
                    tunnel: w3584 -> [_ w3585]
                    frame False {
                    }
                    frame True {
                      n2162 = stacked-sequence {
                        tunnel: w3586 -> [w3587 _]
                        tunnel: w3585 -> [_ w3588]
                        frame #0 {
                          n2163 = property on="Bip Chart" class="WFChart (strict)"("X Scale.Range:Minimum"=w3587) -> ()  [unwired: 2 in, 2 out]
                        }
                        frame #1 {
                          n2164 = property on="Bip Chart" class="WFChart (strict)"("X Scale.Range:Maximum"=w3588) -> ()  [unwired: 2 in, 2 out]
                        }
                      }
                    }
                  }
                }
                frame "ABR" {
                  n2165 = Add(x=w3589, y=w3592) -> (x+y=w3593:dbl)
                  n2166 = Not Equal?(x=w3589, y=w3590) -> (x != y?=w3591:bool)
                  n2167 = case shown="True" w3591 {
                    tunnel: w3589 -> [_ w3595]
                    tunnel: w3593 -> [_ w3594]
                    frame False {
                    }
                    frame True {
                      n2168 = stacked-sequence {
                        tunnel: w3595 -> [w3596 _]
                        tunnel: w3594 -> [_ w3597]
                        frame #0 {
                          n2169 = property on="ABR Chart" class="WFChart (strict)"("X Scale.Range:Minimum"=w3596) -> ()  [unwired: 2 in, 2 out]
                        }
                        frame #1 {
                          n2170 = property on="ABR Chart" class="WFChart (strict)"("X Scale.Range:Maximum"=w3597) -> ()  [unwired: 2 in, 2 out]
                        }
                      }
                    }
                  }
                }
                frame "Sensors" {
                  n2171 = Add(x=w3599, y=w3601) -> (x+y=w3602:dbl)
                  n2172 = Not Equal?(x=w3598, y=w3599) -> (x != y?=w3600:bool)
                  n2173 = case shown="True" w3600 {
                    tunnel: w3599 -> [_ w3603]
                    tunnel: w3602 -> [_ w3604]
                    frame False {
                    }
                    frame True {
                      n2174 = stacked-sequence {
                        tunnel: w3603 -> [w3605 _]
                        tunnel: w3604 -> [_ w3606]
                        frame #0 {
                          n2175 = property on="Aux Chart" class="WFChart (strict)"("X Scale.Range:Minimum"=w3605) -> ()  [unwired: 2 in, 2 out]
                        }
                        frame #1 {
                          n2176 = property on="Aux Chart" class="WFChart (strict)"("X Scale.Range:Maximum"=w3606) -> ()  [unwired: 2 in, 2 out]
                        }
                      }
                    }
                  }
                }
                frame "Jazz" {
                  n2177 = Add(x=w3608, y=w3610) -> (x+y=w3611:dbl)
                  n2178 = Not Equal?(x=w3607, y=w3608) -> (x != y?=w3609:bool)
                  n2179 = case shown="True" w3609 {
                    tunnel: w3608 -> [_ w3612]
                    tunnel: w3611 -> [_ w3613]
                    frame False {
                    }
                    frame True {
                      n2180 = stacked-sequence {
                        tunnel: w3612 -> [w3614 _]
                        tunnel: w3613 -> [_ w3615]
                        frame #0 {
                          n2181 = property on="Jazz Chart" class="WFChart (strict)"("XScale.Minimum"=w3614) -> ()  [unwired: 2 in, 2 out]
                        }
                        frame #1 {
                          n2182 = property on="Jazz Chart" class="WFChart (strict)"("XScale.Maximum"=w3615) -> ()  [unwired: 2 in, 2 out]
                        }
                      }
                    }
                  }
                }
                frame "AIB" {
                  n2183 = Add(x=w3616, y=w3619) -> (x+y=w3620:dbl)
                  n2184 = Not Equal?(x=w3617, y=w3616) -> (x != y?=w3618:bool)
                  n2185 = case shown="True" w3618 {
                    tunnel: w3616 -> [_ w3621]
                    tunnel: w3620 -> [_ w3622]
                    frame False {
                    }
                    frame True {
                      n2186 = stacked-sequence {
                        tunnel: w3621 -> [w3623 _]
                        tunnel: w3622 -> [_ w3624]
                        frame #0 {
                          n2187 = property on="Ana Chart" class="WFChart (strict)"("X Scale.Range:Minimum"=w3623) -> ()  [unwired: 2 in, 2 out]
                        }
                        frame #1 {
                          n2188 = property on="Ana Chart" class="WFChart (strict)"("X Scale.Range:Maximum"=w3624) -> ()  [unwired: 2 in, 2 out]
                        }
                      }
                    }
                  }
                }
                frame "About/Configure", Default {
                }
              }
              n2189 = case shown="False" w3553 {
                tunnel: w3552 -> [_ w3570]
                tunnel: [w3567 w3570] -> w3551
                tunnel: [w3568 w3569] -> w3550
                tunnel: w3549 -> [w3568 _]
                frame False {
                  n2190 = call "Empty Picture"() -> ("empty picture"=w3567:picture)
                }
                frame True {
                  n2191 = call "Empty Picture"() -> ("empty picture"=w3569:picture)
                }
              }
              n2192 = Bundle(w3536, w3536, w3538, w3532) -> (w3548:cluster{i16, i16, i16, i16})  [unwired: 1 out]
              n2193 = Bundle(w3536, w3531, w3538, w3530) -> (w3542:cluster{i16, i16, i16, i16})  [unwired: 1 out]
              n2194 = Add(x=w3524, y=w3533) -> (x+y=w3534:dbl)
              n2195 = Not Equal?(x=w3524, y=w3525) -> (x != y?=w3527:bool)
              n2196 = case shown="True" w3527 {
                tunnel: w3524 -> [_ w3564]
                tunnel: w3534 -> [_ w3563]
                frame False {
                }
                frame True {
                  n2197 = stacked-sequence {
                    tunnel: w3564 -> [w3565 _]
                    tunnel: w3563 -> [_ w3566]
                    frame #0 {
                      n2198 = property on="Trigger Chart" class="WFChart (strict)"("X Scale.Range:Minimum"=w3565) -> ()  [unwired: 2 in, 2 out]
                    }
                    frame #1 {
                      n2199 = property on="Trigger Chart" class="WFChart (strict)"("X Scale.Range:Maximum"=w3566) -> ()  [unwired: 2 in, 2 out]
                    }
                  }
                }
              }
              n2200 = call <vilib>:"Draw Rect.vi"("picture"=w3551, "rect"=w3548, "fill?(F)"=w3540, "color(black)"=w3541) -> ("new picture"=w3544:picture)  [unwired: 1 in, 4 out]
              n2201 = call <vilib>:"Draw Rect.vi"("picture"=w3550, "rect"=w3548, "fill?(F)"=w3540, "color(black)"=w3541) -> ("new picture"=w3546:picture)  [unwired: 1 in, 4 out]
              n2202 = call <vilib>:"Draw Rect.vi"("picture"=w3544, "rect"=w3542, "fill?(F)"=w3540, "color(black)"=w3541) -> ("new picture"=w3543:picture)  [unwired: 1 in, 4 out]
              n2203 = Not(x=w3553) -> (.not. x?=w3554:bool)
              n2204 = call <vilib>:"Draw Rect.vi"("picture"=w3546, "rect"=w3542, "fill?(F)"=w3540, "color(black)"=w3541) -> ("new picture"=w3545:picture)  [unwired: 1 in, 4 out]
            }
          }
          n2205 = Exclusive Or(1:w3313, 2:w3278) -> (0:w3309:bool[])
          n2206 = Or Array Elements(Boolean array=w3309) -> (logical OR=w3308:bool)
          n2207 = case shown="True" w3308 {
            tunnel: w3313 -> [_ w3499]
            tunnel: w3311 -> [w3497 w3504]
            tunnel: [w3497 w3503] -> w3314
            tunnel: w3307 -> [_ w3502]
            frame False {
              # "Driver Handle"
            }
            frame True {
              n2208 = Unbundle By Name(w3502) -> ("Jazz Channels"=w3501:i32)
              n2209 = Not Equal To 0?(x=w3501) -> (x != 0?=w3500:bool)
              n2210 = Build Array (concatenate)(w3499, w3500) -> (w3498:bool[])
              n2211 = call "Act_Write.vi"("Triggers"=w3498, "Handle In"=w3504) -> ("Handle Out"=w3503:i64)
            }
          }
          n2212 = Compound Arithmetic op=OR(w3345, w3442, "Stop") -> (w3408:bool)
          n2213 = Multiply(x=w3382, y=i64 4) -> (x*y=w3383:i64)
          n2214 = To Double Precision Float(number=w3383) -> (double precision float=w3401:dbl)
          n2215 = To Double Precision Float(number=w3310) -> (double precision float=w3400:dbl)
          n2216 = Divide(x=w3401, y=w3390) -> (x/y=w3403:dbl)
          n2217 = Divide(x=w3400, y=w3390) -> (x/y=w3402:dbl)
          n2218 = Bundle(w3403, w3402) -> (→"Ring Buffer":cluster{dbl, dbl})  [unwired: 1 out]
          "Total Saved [sec]" <- w3368
        }
        n2219 = case shown="True" w2924 {
          tunnel: w2927 -> [w3243 w3246]
          tunnel: [w3243 w3245] -> w2926
          tunnel: w2925 -> [_ w3244]
          frame False {
          }
          frame True {
            n2220 = TCP Close Connection(connection ID=w3244, error in (no error)=w3246) -> (error out=w3245:errorcluster)  [unwired: 2 out]
          }
        }
        n2221 = call "Act_Close.vi"("Handle In"=w2861) -> ()
        n2222 = Or(x=w2879, y=w2878) -> (x .or. y?=w2877:bool)
        n2223 = Select(t=w3001, s=w2879, f=w2999) -> (s? t:f=w3000:i32)
      }
      frame 5 {
        w5120 = T6."Disabled and Grayed Out" ("Disabled")
        w5130 = T5."Page Disabled & Grayed" ("Page Enabled State")
        w5131 = T5."Page Enabled" ("Page Enabled State")
        w5121 = T6."Enabled" ("Disabled")
        w5147 = i8 9  # ABR
        w5118 = T6."Enabled" ("Disabled")
        w5166 = 0  # Initially Nothing Saved
        w5178 = 0  # Stay in State 0:    stop running
        w5151 = FALSE
        w5179 = FALSE  # Sop Running
        # "Save Blocksize in Byte"
        # "Current File in Byte"
        # "Header Lenght in Byte"
        # "Busy Saving"
        # "Busy Saving"
        n2224 = property on="Buffer" class="Ring (strict)"("Disabled"=w5118) -> ()  [unwired: 2 in, 2 out]
        n2225 = property on="Load Configuration File" class="Bool"("Disabled"=w5118) -> ()  [unwired: 2 in, 2 out]
        n2226 = property on="Save Configuration File" class="Bool"("Disabled"=w5118) -> ()  [unwired: 2 in, 2 out]
        n2227 = property on="Edit" class="Bool"("Disabled"=w5118) -> ()  [unwired: 2 in, 2 out]
        n2228 = property on="Channels" class="Ring (strict)"("Disabled"=w5118) -> ()  [unwired: 2 in, 2 out]
        n2229 = property on="AuxFree" class="LstBox (strict)"("Disabled"=w5118) -> ()  [unwired: 2 in, 2 out]
        n2230 = property on="JazzFree" class="LstBox (strict)"("Disabled"=w5118) -> ()  [unwired: 2 in, 2 out]
        n2231 = property on="AnaFree" class="LstBox (strict)"("Disabled"=w5118) -> ()  [unwired: 2 in, 2 out]
        n2232 = property on="ScreenLength" class="Ring (strict)"("Disabled"=w5118) -> ()  [unwired: 2 in, 2 out]
        n2233 = property on="LocalPort" class="DigNum (strict)"("Disabled"=w5118) -> ()  [unwired: 2 in, 2 out]
        n2234 = property on="TCPsubset" class="Ring (strict)"("Disabled"=w5118) -> ()  [unwired: 2 in, 2 out]
        n2235 = property on="TCPaddTP" class="Bool (strict)"("Disabled"=w5118) -> ()  [unwired: 2 in, 2 out]
        n2236 = property on="TCPaddSens" class="Bool (strict)"("Disabled"=w5118) -> ()  [unwired: 2 in, 2 out]
        n2237 = property on="TCPaddAnas" class="Bool (strict)"("Disabled"=w5118) -> ()  [unwired: 2 in, 2 out]
        n2238 = property on="TCPaddJazz" class="Bool (strict)"("Disabled"=w5118) -> ()  [unwired: 2 in, 2 out]
        n2239 = property on="TCPaddTrig" class="Bool (strict)"("Disabled"=w5118) -> ()  [unwired: 2 in, 2 out]
        n2240 = property on="AvgTrigSel" class="LstBox (strict)"("Disabled"=w5118) -> ()  [unwired: 2 in, 2 out]
        n2241 = property on="AvgTrigLog" class="Ring (strict)"("Disabled"=w5118) -> ()  [unwired: 2 in, 2 out]
        n2242 = property on="AvgSweep" class="DigNum (strict)"("Disabled"=w5118) -> ()  [unwired: 2 in, 2 out]
        n2243 = property on="Set Stride in kByte\n(default 128 kByte)" class="DigNum (strict)"("DisabledEnum"=w5118) -> ()  [unwired: 2 in, 2 out]
        n2244 = case shown="True" w5172 {
          tunnel: w5176 -> [w5197 w5222]
          tunnel: w5174 -> [w5198 w5204]
          tunnel: [w5198 w5205] -> w5163
          tunnel: [w5197 w5201] -> w5175
          tunnel: w5173 -> [_ w5209]
          tunnel: w5177 -> [_ w5221]
          tunnel: w5165 -> [_ w5212]
          tunnel: w5151 -> [_ w5202]
          frame False {
            n2245 = local write "Start Saving"(FALSE ("Start Saving")) -> ()
          }
          frame True {
            w5201 = refnum<file> refnum  # Dummy Refnum
            w5207 = errorcluster {"status"=FALSE, "code"=0, "source"=""}  # No error
            # "number of data records"
            n2246 = To Quad Integer(1:w5209) -> (0:w5199:i64)
            n2247 = To Quad Integer(1:w5212) -> (0:w5200:i64)
            n2248 = Unbundle By Name(w5204) -> ("code"=w5211:i32)
            n2249 = Subtract(x=w5221, y=w5199) -> (x-y=w5220:i64)
            n2250 = Quotient & Remainder(x=w5220, y=w5200) -> (floor(x/y)=w5213:i64)  [unwired: 1 out]
            n2251 = Less?(x=w5211, y=5000) -> (x < y?=w5203:bool)
            n2252 = Format Into String(format string="%-8d", w5213) -> (resulting string=w5218:string)  [unwired: 2 in, 1 out]
            n2253 = Select(t=w5204, s=w5203, f=w5207) -> (s? t:f=w5208:errorcluster)
            n2254 = call "Write File+ [String].vi"("String"=w5218, "error in (no error)"=w5208, "pos offset (bytes:0)"=i64 236, "pos mode (rel. to end:1)"=enum16{"start", "end", "current"}."start", "refnum"=w5222) -> ("error out"=w5217:errorcluster, "dup refnum"=w5216:refnum<file>)  [unwired: 2 out]
            n2255 = flat-sequence {
              tunnel: w5202 -> [w5224]
              frame #0 {
                n2256 = property on="Start Saving" class="Bool (strict)"("Boolean Text.Text"="Initializing") -> ()  [unwired: 2 in, 2 out]
              }
              frame #1 {
                n2257 = local write "Start Saving"(w5224) -> ()
              }
              frame #2 {
                n2258 = property on="Start Saving" class="Bool (strict)"("Boolean Text.Text"="Start File") -> ()  [unwired: 2 in, 2 out]
              }
            }
            n2259 = Close File(refnum=w5216, error in=w5217) -> (error out=w5206:errorcluster)  [unwired: 1 out]
            n2260 = Select(t=w5206, s=w5203, f=w5204) -> (s? t:f=w5205:errorcluster)
            n2261 = local write "Pause Saving"(w5202) -> ()
          }
        }
        n2262 = Unbundle By Name(w5146) -> ("JazzRec"=w5125:bool, "ABR Enabled"=w5123:bool, "Speed Mode"=w5128:i8)
        n2263 = property on="JazzOn" class="Bool (strict)"("Disabled"=w5118) -> ()  [unwired: 2 in, 2 out]
        n2264 = Less Than 0?(x=w5128) -> (x < 0?=w5126:bool)
        n2265 = Equal?(x=w5128, y=w5147) -> (x = y?=w5124:bool)
        n2266 = In Range and Coerce(upper limit=i8 8, x=w5128, lower limit=i8 4) -> (In Range?=w5127:bool)  [unwired: 1 out]
        n2267 = Equal?(x=w5128, y=i8 13) -> (x = y?=w5133:bool)
        n2268 = for {
          N: 129 -> [_]
          tunnel: [0.0] -> w5148 mode=indexing
        }
        n2269 = Or(x=w5126, y=w5127) -> (x .or. y?=w5142:bool)
        n2270 = Compound Arithmetic op=OR(w5124, w5133, w5126) -> (w5132:bool)
        n2271 = property on="Charts/Graphs" class="TabCtl (strict)"() -> ("Pages"=w5144:refnum<vi>[])  [unwired: 2 in, 2 out]
        n2272 = Select(t=w5120, s=w5123, f=w5121) -> (s? t:f=w5122:T6)
        n2273 = And(x=w5125, y=w5142) -> (x .and. y?=w5143:bool)
        n2274 = Select(t=w5131, s=w5143, f=w5130) -> (s? t:f=w5145:T5)
        n2275 = global write "Data.glb" "Data"(w5148) -> ()
        n2276 = Select(t=w5120, s=w5124, f=w5121) -> (s? t:f=w5129:T6)
        n2277 = Select(t=w5131, s=w5132, f=w5130) -> (s? t:f=w5135:T5)
        n2278 = Index Array(array=w5144, index #1=3 ("index"), index #2=6 ("index")) -> (element #1=w5136:refnum<vi>, element #2=w5137:refnum<vi>)
        n2279 = property on="AbrOn" class="Bool (strict)"("DisabledEnum"=w5129) -> ()  [unwired: 2 in, 2 out]
        n2280 = property on="Downsample Ratio" class="Ring (strict)"("Disabled"=w5122) -> ()  [unwired: 2 in, 2 out]
        n2281 = property on="ABR" class="Page"(reference=w5136, "Page Enabled State"=w5135) -> ()  [unwired: 1 in, 2 out]
        n2282 = property on="Jazz" class="Page"(reference=w5137, "Page Enabled State"=w5145) -> ()  [unwired: 1 in, 2 out]
        n2283 = property on="AvgLPfreq" class="DigNum (strict)"("Disabled"=w5122) -> ()  [unwired: 2 in, 2 out]
        n2284 = property on="AvgLP" class="Bool (strict)"("Disabled"=w5122) -> ()  [unwired: 2 in, 2 out]
        n2285 = local write "Start"(w5151) -> ()
        n2286 = local write "Write BDF"(w5151) -> ()
        n2287 = property on="AvgHPfreq" class="DigNum (strict)"("Disabled"=w5122) -> ()  [unwired: 2 in, 2 out]
        n2288 = property on="AvgHP" class="Bool (strict)"("Disabled"=w5122) -> ()  [unwired: 2 in, 2 out]
        n2289 = local write "Averaging"(w5151) -> ()
        n2290 = local write "Sweeping"(w5151) -> ()
        n2291 = property on="RefFreeAvg1" class="LstBox (strict)"("Disabled"=w5122) -> ()  [unwired: 2 in, 2 out]
        n2292 = property on="MonFreeAvg1" class="LstBox (strict)"("Disabled"=w5122) -> ()  [unwired: 2 in, 2 out]
        n2293 = local write "TCP Connected"(w5151) -> ()
        n2294 = local write "TCP Listening"(w5151) -> ()
        n2295 = Unbundle By Name(w5163) -> ("code"=w5164:i32)
        n2296 = property on="RefFreeAvg2" class="LstBox (strict)"("Disabled"=w5122) -> ()  [unwired: 2 in, 2 out]
        n2297 = property on="MonFreeAvg2" class="LstBox (strict)"("Disabled"=w5122) -> ()  [unwired: 2 in, 2 out]
        n2298 = property on="Start Saving" class="Bool (strict)"() -> ("Colors [4]"=w5156:cluster{u32, u32}[])  [unwired: 2 in, 2 out]
        n2299 = case shown="5003" w5164 {
          tunnel: w5163 -> [w5182 w5191]
          tunnel: [w5189 w5195] -> w5162
          frame 0, Default {
            w5189 = errorcluster {"status"=FALSE, "code"=0, "source"=""}  # No Error
            n2300 = call "Act_Error_5000.vi"() -> ("[user-defined descriptions]"=w5183:string[], "[user-defined codes]"=w5186:i32[])  [unwired: 2 in, 1 out]
            n2301 = call "Act_Error_7000.vi"() -> ("[user-defined descriptions]"=w5184:string[], "[user-defined codes]"=w5188:i32[])  [unwired: 2 in, 1 out]
            n2302 = Build Array (concatenate)(w5183, w5184) -> (w5185:string[])
            n2303 = Build Array (concatenate)(w5186, w5188) -> (w5187:i32[])
            n2304 = call <vilib>:"General Error Handler.vi"("[user-defined codes]"=w5187, "[user-defined descriptions]"=w5185, "error in (no error)"=w5182) -> ()  [unwired: 2 in, 11 out]
          }
          frame 5003 {
            n2305 = Unbundle(w5191) -> ("code"=w5193:i32, "source"=w5192:string)  [unwired: 1 out]
            n2306 = Bundle(FALSE, "code"=w5193, "source"=w5192) -> (w5190:cluster{bool, "code":i32, "source":string})  [unwired: 1 in]
            n2307 = call "Display Message to User"("error in (no error)"=w5190) -> ("error out"=w5195:errorcluster)  [unwired: 2 in, 8 out]
          }
        }
        n2308 = Index Array(array=w5156) -> (element #1=w5158:cluster{u32, u32}, element #2=w5157:cluster{u32, u32})  [unwired: 2 in]
        n2309 = Unbundle(w5157) -> (w5159:u32)  [unwired: 1 out]
        n2310 = Bundle(u32 16724991, w5159) -> (w5160:cluster{u32, u32})  [unwired: 1 out]
        n2311 = Build Array(w5158, w5160) -> (w5154:cluster{u32, u32}[])
        n2312 = property on="Start Saving" class="Bool (strict)"("Colors [4]"=w5154, "Boolean Text.Text Colors:Text Color"=u32 16777215) -> ()  [unwired: 2 in, 2 out]
        n2313 = To Quad Integer(1:w5166) -> (0:w5150:i64)
      }
    }
    n2314 = global write "PanelThread.glb" "PanelThread"(w169) -> ()
  }
  n2315 = while {
    tunnel: w47 -> [w5228]
    stop <- w5273 stop-if-true
    w5255 = 263 ("Position:Top")
    w5256 = 811 ("Position:Left")
    w5257 = u32 64 ("y")
    n2316 = property class="VI"(error in=w5228) -> ("Front Panel.PanelBounds"=w5268:T28)  [unwired: 1 in, 2 out]
    n2317 = property on="Ring Buffer" class="Knob (strict)" props=["Height", "Width", "Left", "Top"]() -> ("Height"=w5258:u32, "Left"=w5246:i32, "Top"=w5245:i32)  [unwired: 2 in, 3 out]
    n2318 = Wait (ms)(milliseconds to wait=u32 200) -> ()  [unwired: 1 out]
    n2319 = Unbundle By Name(w5268) -> ("Left"=w5271:i16, "Top"=w5270:i16, "Right"=w5272:i16, "Bottom"=w5269:i16)
    n2320 = Subtract(x=w5269, y=w5270) -> (x-y=w5261:i16)
    n2321 = Subtract(x=w5272, y=w5271) -> (x-y=w5262:i16)
    n2322 = Less?(x=w5258, y=w5257) -> (x < y?=w5250:bool)
    n2323 = Not Equal?(x=w5246, y=w5256) -> (x != y?=w5254:bool)
    n2324 = Not Equal?(x=w5245, y=w5255) -> (x != y?=w5253:bool)
    n2325 = Equal?(x=w5262, y=i16 1200) -> (x = y?=w5252:bool)
    n2326 = Equal?(x=w5261, y=i16 650) -> (x = y?=w5251:bool)
    n2327 = Greater?(x=w5262, y=i16 1400) -> (0:w5265:bool)
    n2328 = Greater?(x=w5261, y=i16 850) -> (0:w5240:bool)
    n2329 = Or(x=w5254, y=w5253) -> (x .or. y?=w5247:bool)
    n2330 = And(x=w5252, y=w5251) -> (x .and. y?=w5237:bool)
    n2331 = And(x=w5265, y=w5240) -> (x .and. y?=w5231:bool)
    n2332 = Select(t=u8 6 ("Plot.Point Style"), s=w5240, f=u8 9) -> (s? t:f=w5243:u8)
    n2333 = And(x=w5237, y=w5250) -> (x .and. y?=w5249:bool)
    n2334 = And(x=w5237, y=w5247) -> (x .and. y?=w5248:bool)
    n2335 = for {
      N: 16 -> [_]
      tunnel: w5243 -> [w5277]
      i -> [w5279]
      n2336 = To Unsigned Long Integer(number=w5279) -> (unsigned 32bit integer=w5278:u32)
      n2337 = property on="Trigger Chart" class="WFChart (strict)"("Active Plot"=w5278, "Plot.Point Style"=w5277) -> ()  [unwired: 2 in, 2 out]
    }
    n2338 = case shown="True" w5249 {
      tunnel: w5257 -> [_ w5282]
      frame False {
      }
      frame True {
        n2339 = property on="Ring Buffer" class="Knob (strict)"("Height"=w5282, "Width"=w5282) -> ()  [unwired: 2 in, 2 out]
      }
    }
    n2340 = case shown="True" w5248 {
      tunnel: w5256 -> [_ w5281]
      tunnel: w5255 -> [_ w5280]
      frame False {
      }
      frame True {
        n2341 = property on="Ring Buffer" class="Knob (strict)"("Left"=w5281, "Top"=w5280) -> ()  [unwired: 2 in, 2 out]
      }
    }
    n2342 = Select(t=u32 18, s=w5231, f=u32 14 ("Boolean Text.Font:Size")) -> (s? t:f=w5227:u32)
    n2343 = Select(t=u32 14, s=w5231, f=u32 12 ("Boolean Text.Font:Size")) -> (s? t:f=w5226:u32)
    n2344 = Select(t=u32 24, s=w5231, f=u32 18 ("Boolean Text.Font:Size")) -> (s? t:f=w5234:u32)
    n2345 = Select(t=u32 18, s=w5231, f=u32 12 ("Boolean Text.Font:Size")) -> (s? t:f=w5230:u32)
    n2346 = property on="Start" class="Bool (strict)"("BoolText.FontSize"=w5227) -> ()  [unwired: 2 in, 2 out]
    n2347 = property on="Mon Filter Reset" class="Bool"("BoolText.FontSize"=w5226) -> ()  [unwired: 2 in, 2 out]
    n2348 = property on="Edit" class="Bool"("BoolText.FontSize"=w5234) -> ()  [unwired: 2 in, 2 out]
    n2349 = property on="Bip Filter Reset" class="Bool"("BoolText.FontSize"=w5226) -> ()  [unwired: 2 in, 2 out]
    n2350 = property on="Stop" class="Bool (strict)"("BoolText.FontSize"=w5227) -> ()  [unwired: 2 in, 2 out]
    n2351 = property on="Battery" class="Slide (strict)"("Label.FontSize"=w5230) -> ()  [unwired: 2 in, 2 out]
    n2352 = property on="Aux DC Reset" class="Bool"("BoolText.FontSize"=w5226) -> ()  [unwired: 2 in, 2 out]
    n2353 = property on="Ana Filter Reset" class="Bool"("BoolText.FontSize"=w5226) -> ()  [unwired: 2 in, 2 out]
    n2354 = property on="Sweeping" class="Bool (strict)"("BoolText.FontSize"=w5226) -> ()  [unwired: 2 in, 2 out]
    n2355 = property on="UploadMaps" class="Bool (strict)"("BoolText.FontSize"=w5226) -> ()  [unwired: 2 in, 2 out]
    n2356 = property on="Low Batt" class="Bool (strict)"("Label.FontSize"=w5230) -> ()  [unwired: 2 in, 2 out]
    n2357 = property on="Start Saving" class="Bool (strict)"("BoolText.FontSize"=w5227) -> ()  [unwired: 2 in, 2 out]
    n2358 = property on="Pause Saving" class="Bool (strict)"("BoolText.FontSize"=w5227) -> ()  [unwired: 2 in, 2 out]
    n2359 = property on="Jazz Filter Reset" class="Bool"("BoolText.FontSize"=w5226) -> ()  [unwired: 2 in, 2 out]
    n2360 = property on="Averaging" class="Bool (strict)"("BoolText.FontSize"=w5226) -> ()  [unwired: 2 in, 2 out]
    n2361 = property on="HeadcapMaps" class="Bool (strict)"("BoolText.FontSize"=w5226) -> ()  [unwired: 2 in, 2 out]
    n2362 = property on="Full Range" class="Bool (strict)"("BoolText.FontSize"=w5226) -> ()  [unwired: 2 in, 2 out]
    n2363 = property on="CM in Range" class="Bool (strict)"("Label.FontSize"=w5230) -> ()  [unwired: 2 in, 2 out]
    n2364 = property on="Load Configuration File" class="Bool"("BoolText.FontSize"=w5226) -> ()  [unwired: 2 in, 2 out]
    n2365 = property on="Save Configuration File" class="Bool"("BoolText.FontSize"=w5226) -> ()  [unwired: 2 in, 2 out]
    n2366 = property on="ABR Filter Reset" class="Bool"("BoolText.FontSize"=w5226) -> ()  [unwired: 2 in, 2 out]
    n2367 = property on="ABR Full Range" class="Bool (strict)"("BoolText.FontSize"=w5226) -> ()  [unwired: 2 in, 2 out]
    n2368 = property on="Decimation" class="Ring (strict)"("RingText.FontSize"=w5226) -> ()  [unwired: 2 in, 2 out]
    n2369 = property on="MonScale" class="Ring (strict)"("RingText.FontSize"=w5226) -> ()  [unwired: 2 in, 2 out]
    n2370 = property on="Channels" class="Ring (strict)"("RingText.FontSize"=w5226) -> ()  [unwired: 2 in, 2 out]
    n2371 = property on="Reference" class="Ring (strict)"("RingText.FontSize"=w5226) -> ()  [unwired: 2 in, 2 out]
    n2372 = property on="BipScale" class="Ring (strict)"("RingText.FontSize"=w5226) -> ()  [unwired: 2 in, 2 out]
    n2373 = property on="OffsetScale" class="Ring (strict)"("RingText.FontSize"=w5226) -> ()  [unwired: 2 in, 2 out]
    n2374 = property on="Offset" class="Ring (strict)"("RingText.FontSize"=w5226) -> ()  [unwired: 2 in, 2 out]
    n2375 = property on="AvgTrigLog" class="Ring (strict)"("RingText.FontSize"=w5226) -> ()  [unwired: 2 in, 2 out]
    n2376 = property on="GsrScale" class="Ring (strict)"("RingText.FontSize"=w5226) -> ()  [unwired: 2 in, 2 out]
    n2377 = property on="RespScale" class="Ring (strict)"("RingText.FontSize"=w5226) -> ()  [unwired: 2 in, 2 out]
    n2378 = property on="ErgoScale" class="Ring (strict)"("RingText.FontSize"=w5226) -> ()  [unwired: 2 in, 2 out]
    n2379 = property on="PletScale" class="Ring (strict)"("RingText.FontSize"=w5226) -> ()  [unwired: 2 in, 2 out]
    n2380 = property on="TempScale" class="Ring (strict)"("RingText.FontSize"=w5226) -> ()  [unwired: 2 in, 2 out]
    n2381 = property on="AnaScale" class="Ring (strict)"("RingText.FontSize"=w5226) -> ()  [unwired: 2 in, 2 out]
    n2382 = property on="Box" class="Ring (strict)"("RingText.FontSize"=w5226) -> ()  [unwired: 2 in, 2 out]
    n2383 = property on="Buffer" class="Ring (strict)"("RingText.FontSize"=w5226) -> ()  [unwired: 2 in, 2 out]
    n2384 = property on="TrigCode" class="Ring (strict)"("RingText.FontSize"=w5226) -> ()  [unwired: 2 in, 2 out]
    n2385 = property on="ScreenLength" class="Ring (strict)"("RingText.FontSize"=w5226) -> ()  [unwired: 2 in, 2 out]
    n2386 = property on="TCPsubset" class="Ring (strict)"("RingText.FontSize"=w5226) -> ()  [unwired: 2 in, 2 out]
    n2387 = property on="AbrScale" class="Ring (strict)"("RingText.FontSize"=w5226) -> ()  [unwired: 2 in, 2 out]
    n2388 = property on="AbrChannels" class="Ring (strict)"("RingText.FontSize"=w5226) -> ()  [unwired: 2 in, 2 out]
    n2389 = property on="AbrOffsetScale" class="Ring (strict)"("RingText.FontSize"=w5226) -> ()  [unwired: 2 in, 2 out]
    n2390 = event shown="[1] Panel Close?" {
      selector: _ -> [_ _]
      dyn-events: _ -> [_ _]
      timeout: 50 -> [_ _]
      event Timeout {
        n2391 = event-data() -> ()  [unwired: 1 in, 3 out]
      }
      event Panel Close? {
        n2392 = event-data() -> ()  [unwired: 1 in, 4 out]
        n2393 = global write "CapsThread.glb" "CapsThread"(TRUE ("CapsThread")) -> ()
        n2394 = Wait (ms)(milliseconds to wait=u32 500) -> ()  [unwired: 1 out]
        n2395 = event-data() -> ()  [unwired: 2 in, 1 out]
      }
    }
    n2396 = global read "PanelThread.glb" "PanelThread"() -> (w5273:bool)
  }
  n2397 = while {
    tunnel: w47 -> [w5283]
    stop <- w5285 stop-if-true
    n2398 = call <vilib>:"General Error Handler.vi"("error in (no error)"=w5283) -> ()  [unwired: 4 in, 11 out]
    n2399 = Wait (ms)(milliseconds to wait=u32 200) -> ()  [unwired: 1 out]
    n2400 = case shown="True" "HeadcapMaps" {
      frame False {
        n2401 = property on="HeadcapMaps" class="Bool (strict)"("DisabledEnum"=T6."Enabled" ("Disabled")) -> ()  [unwired: 2 in, 2 out]
      }
      frame True {
        n2402 = flat-sequence {
          frame #0 {
            n2403 = property on="HeadcapMaps" class="Bool (strict)"("DisabledEnum"=T6."Disabled" ("Disabled")) -> ()  [unwired: 2 in, 2 out]
          }
          frame #1 {
            n2404 = call "HeadcapMaps-Win.vi"() -> ()  [unwired: 2 in]
          }
          frame #2 {
            n2405 = local write "HeadcapMaps"(FALSE ("HeadcapMaps")) -> ()
          }
        }
      }
    }
    n2406 = global read "PanelThread.glb" "PanelThread"() -> (w5285:bool)
  }
